vi "Battery_Tester_Main.vi"() -> ()   [LabVIEW 2019]
uses:
  <vilib>/Analysis/baseanly.llb/Mean (DBL).vi
  <vilib>/Analysis/NI_AALBase.lvlib
panel:
  in  "CurrentRefArrayGraph":dbl[](array[numeric])
  in  "Reset Log":bool
  out "Voltage/Current by Time NUI":T1(graph)=[{"TimeGraph"=[0.0, 0.88, 1.924, 3.815, 4.953, 6.09, 7.236, 8.152, 9.288, 10.425, 11.564, 12.704, 13.844, 14.984, 16.032, 17.055, 18.199, 19.341, 20.48, 21.391, 22.528, 23.667, 24.804, 25.944, 27.082, 28.181, 29.167, 30.31, 31.445, 32.587, 33.721, 34.863, 35.997, 37.13, 38.264, 39.403, 40.547, 41.692, 42.838, 43.976, 45.121, 46.267, 47.404, 48.544, 49.684, 50.825, 51.952, 53.087, 54.227, 55.361, 56.502, 57.644, 58.78, 59.928, 61.067, 62.203, 63.348, 64.485, 65.629, 66.772, 67.915, 69.061, 70.022, 71.167, 72.302, 73.444, 74.578, 75.709, 76.845, 77.978, 79.128, 80.272, 81.412, 82.552, 83.693, 84.833, 85.971, 87.106, 88.246, 89.247, 90.387, 91.523, 92.658, 93.8, 94.936, 96.082, 97.22, 98.357, 99.491, 100.625, 101.764, 102.898, 104.035, 105.171, 106.317, 107.453, 108.597, 109.732, 110.872, 112.007, 113.153, 114.287, 115.319, 116.45, 117.588, 118.721, 119.861, 120.999, 122.139, 123.108, 124.248, 125.384, 126.521, 127.655, 128.797, 129.932, 131.067, 132.105, 133.242, 134.386, 135.531, 136.662, 137.795, 138.946, 140.08, 141.219, 142.357, 143.495, 144.633, 145.771, 146.824, 147.806, 148.95, 150.084, 151.22, 152.353, 153.487, 154.625, 155.761, 156.899, 158.045, 159.178, 160.317, 161.481, 162.612, 163.748, 164.881, 166.022, 167.158, 168.295, 169.21, 170.339, 171.473, 172.612, 173.746, 174.884, 176.016, 177.159, 178.11, 179.243, 180.374, 181.505, 182.639, 183.777, 184.914, 186.049, 187.188, 188.326, 189.465, 190.609, 191.74, 201.232, 202.369, 203.395, 204.535, 205.597, 206.735, 207.868, 209.009, 210.148, 211.285, 212.42, 213.563, 214.701, 215.84, 216.981, 218.121, 219.26, 220.402, 221.537, 222.673, 223.812, 224.946, 226.083, 227.221, 228.36, 229.504, 230.637, 231.78, 232.916, 234.051, 235.189, 236.321, 237.457, 238.593, 239.73, 240.871, 242.008, 243.147, 265.521, 266.543, 267.649, 268.599, 269.536], "CurrentArrayGraph"=[844.5, 844.5, 844.0, 837.3, 835.8, 833.5, 835.2, 829.9, 832.5, 828.9, 829.5, 831.6, 832.0, 831.6, 825.7, 830.4, 828.4, 830.0, 825.9, 827.8, 825.2, 825.2, 826.7, 827.8, 827.4, 821.6, 831.1, 822.6, 826.3, 822.9, 824.2, 819.1, 819.5, 824.8, 825.0, 817.7, 821.7, 823.7, 820.6, 820.2, 824.2, 823.3, 820.2, 824.8, 825.4, 821.7, 818.0, 820.0, 822.7, 818.0, 817.1, 822.2, 821.1, 818.6, 816.5, 816.6, 818.1, 818.0, 818.1, 816.6, 816.5, 815.0, 819.0, 814.5, 823.8, 814.0, 816.0, 818.5, 812.5, 821.6, 817.0, 815.6, 818.0, 818.6, 817.6, 815.6, 814.0, 812.0, 813.5, 812.5, 813.0, 812.5, 814.5, 813.0, 815.0, 810.5, 817.0, 815.6, 814.6, 812.0, 816.5, 815.0, 813.0, 816.6, 812.5, 808.5, 812.5, 807.0, 810.5, 814.0, 812.0, 818.5, 810.5, 817.5, 808.0, 820.0, 808.5, 816.0, 813.1, 813.0, 808.0, 814.5, 809.0, 814.0, 806.5, 815.5, 810.0, 806.5, 807.0, 812.5, 811.5, 816.1, 810.5, 813.6, 812.5, 806.0, 809.5, 816.5, 809.0, 806.5, 806.0, 808.5, 804.5, 811.5, 814.5, 816.0, 804.5, 804.5, 803.5, 808.5, 809.0, 804.5, 805.5, 805.5, 804.0, 805.5, 805.0, 803.0, 806.0, 806.5, 810.5, 807.0, 803.5, 803.0, 802.5, 803.0, 802.5, 802.5, 812.0, 811.0, 803.5, 806.1, 809.0, 818.1, 809.5, 804.0, 802.5, 804.5, 803.5, 809.5, 809.5, 81.2, 809.5, 803.5, 812.0, 801.5, 807.5, 804.5, 804.5, 807.0, 805.0, 808.0, 807.0, 802.5, 807.0, 803.5, 803.0, 806.0, 802.5, 805.5, 806.5, 804.0, 806.0, 804.0, 804.5, 807.5, 800.0, 805.0, 807.0, 803.5, 804.0, 802.0, 806.5, 802.0, 804.0, 800.5, 803.0, 803.0, 804.0, 80.2, 723.3, 803.0, 800.5, 798.5]}, {"TimeGraph"=[0.0, 0.88, 1.924, 3.815, 4.953, 6.09, 7.236, 8.152, 9.288, 10.425, 11.564, 12.704, 13.844, 14.984, 16.032, 17.055, 18.199, 19.341, 20.48, 21.391, 22.528, 23.667, 24.804, 25.944, 27.082, 28.181, 29.167, 30.31, 31.445, 32.587, 33.721, 34.863, 35.997, 37.13, 38.264, 39.403, 40.547, 41.692, 42.838, 43.976, 45.121, 46.267, 47.404, 48.544, 49.684, 50.825, 51.952, 53.087, 54.227, 55.361, 56.502, 57.644, 58.78, 59.928, 61.067, 62.203, 63.348, 64.485, 65.629, 66.772, 67.915, 69.061, 70.022, 71.167, 72.302, 73.444, 74.578, 75.709, 76.845, 77.978, 79.128, 80.272, 81.412, 82.552, 83.693, 84.833, 85.971, 87.106, 88.246, 89.247, 90.387, 91.523, 92.658, 93.8, 94.936, 96.082, 97.22, 98.357, 99.491, 100.625, 101.764, 102.898, 104.035, 105.171, 106.317, 107.453, 108.597, 109.732, 110.872, 112.007, 113.153, 114.287, 115.319, 116.45, 117.588, 118.721, 119.861, 120.999, 122.139, 123.108, 124.248, 125.384, 126.521, 127.655, 128.797, 129.932, 131.067, 132.105, 133.242, 134.386, 135.531, 136.662, 137.795, 138.946, 140.08, 141.219, 142.357, 143.495, 144.633, 145.771, 146.824, 147.806, 148.95, 150.084, 151.22, 152.353, 153.487, 154.625, 155.761, 156.899, 158.045, 159.178, 160.317, 161.481, 162.612, 163.748, 164.881, 166.022, 167.158, 168.295, 169.21, 170.339, 171.473, 172.612, 173.746, 174.884, 176.016, 177.159, 178.11, 179.243, 180.374, 181.505, 182.639, 183.777, 184.914, 186.049, 187.188, 188.326, 189.465, 190.609, 191.74, 201.232, 202.369, 203.395, 204.535, 205.597, 206.735, 207.868, 209.009, 210.148, 211.285, 212.42, 213.563, 214.701, 215.84, 216.981, 218.121, 219.26, 220.402, 221.537, 222.673, 223.812, 224.946, 226.083, 227.221, 228.36, 229.504, 230.637, 231.78, 232.916, 234.051, 235.189, 236.321, 237.457, 238.593, 239.73, 240.871, 242.008, 243.147, 265.521, 266.543, 267.649, 268.599, 269.536], "CurrentArrayGraph"=[48.35, 47.1, 48.6, 47.3, 49.35, 49.4, 50.05, 44.95, 51.65, 44.95, 44.7, 50.15, 51.4, 49.9, 49.45, 48.05, 49.1, 49.85, 46.75, 50.1, 50.65, 44.9, 44.7, 43.9, 44.45, 46.25, 45.9, 49.9, 50.1, 46.8, 48.75, 48.6, 49.65, 51.4, 49.6, 43.7, 43.7, 51.15, 49.35, 50.45, 49.9, 50.9, 48.85, 49.05, 51.65, 50.4, 41.35, 50.65, 49.4, 43.9, 50.9, 48.55, 48.85, 47.8, 39.0, 48.9, 47.05, 51.95, 48.8, 51.15, 50.95, 48.6, 46.5, 45.75, 52.6, 43.45, 48.85, 51.6, 50.4, 50.3, 50.45, 44.95, 49.6, 49.8, 50.1, 49.9, 51.25, 44.75, 51.15, 46.0, 45.45, 51.5, 52.0, 48.65, 54.45, 48.85, 46.0, 53.95, 42.1, 51.15, 41.35, 56.1, 46.75, 53.6, 47.3, 50.7, 48.6, 52.75, 35.45, 56.05, 45.25, 54.2, 50.45, 52.65, 48.9, 48.5, 50.4, 48.6, 51.45, 48.85, 45.25, 53.5, 44.0, 52.35, 49.35, 52.95, 56.1, 56.35, 46.8, 52.35, 46.8, 55.0, 56.6, 52.3, 56.9, 46.3, 44.5, 49.75, 50.9, 46.5, 43.75, 45.75, 39.1, 46.75, 47.25, 52.1, 56.35, 49.9, 30.05, 46.0, 55.3, 51.0, 49.8, 39.6, 33.95, 45.5, 40.85, 35.95, 39.1, 39.6, 45.75, 43.25, 30.8, 43.75, 38.6, 43.75, 49.55, 39.85, 45.1, 46.5, 39.1, 49.55, 56.35, 50.25, 45.5, 44.0, 38.6, 39.35, 43.0, 48.5, 43.6, 5.95, 52.2, 48.55, 48.6, 43.5, 52.7, 49.55, 48.05, 49.1, 50.15, 49.6, 52.95, 49.35, 47.85, 50.65, 44.95, 49.1, 47.8, 49.1, 46.2, 48.1, 49.8, 49.65, 49.85, 50.6, 38.8, 46.55, 47.8, 50.05, 51.15, 46.0, 49.1, 48.3, 51.4, 50.2, 33.3, 50.65, 48.1, 5.95, 42.9, 48.3, 40.6, 45.7]}, {"TimeGraph"=[0.0, 0.88, 1.924, 3.815, 4.953, 6.09, 7.236, 8.152, 9.288, 10.425, 11.564, 12.704, 13.844, 14.984, 16.032, 17.055, 18.199, 19.341, 20.48, 21.391, 22.528, 23.667, 24.804, 25.944, 27.082, 28.181, 29.167, 30.31, 31.445, 32.587, 33.721, 34.863, 35.997, 37.13, 38.264, 39.403, 40.547, 41.692, 42.838, 43.976, 45.121, 46.267, 47.404, 48.544, 49.684, 50.825, 51.952, 53.087, 54.227, 55.361, 56.502, 57.644, 58.78, 59.928, 61.067, 62.203, 63.348, 64.485, 65.629, 66.772, 67.915, 69.061, 70.022, 71.167, 72.302, 73.444, 74.578, 75.709, 76.845, 77.978, 79.128, 80.272, 81.412, 82.552, 83.693, 84.833, 85.971, 87.106, 88.246, 89.247, 90.387, 91.523, 92.658, 93.8, 94.936, 96.082, 97.22, 98.357, 99.491, 100.625, 101.764, 102.898, 104.035, 105.171, 106.317, 107.453, 108.597, 109.732, 110.872, 112.007, 113.153, 114.287, 115.319, 116.45, 117.588, 118.721, 119.861, 120.999, 122.139, 123.108, 124.248, 125.384, 126.521, 127.655, 128.797, 129.932, 131.067, 132.105, 133.242, 134.386, 135.531, 136.662, 137.795, 138.946, 140.08, 141.219, 142.357, 143.495, 144.633, 145.771, 146.824, 147.806, 148.95, 150.084, 151.22, 152.353, 153.487, 154.625, 155.761, 156.899, 158.045, 159.178, 160.317, 161.481, 162.612, 163.748, 164.881, 166.022, 167.158, 168.295, 169.21, 170.339, 171.473, 172.612, 173.746, 174.884, 176.016, 177.159, 178.11, 179.243, 180.374, 181.505, 182.639, 183.777, 184.914, 186.049, 187.188, 188.326, 189.465, 190.609, 191.74, 201.232, 202.369, 203.395, 204.535, 205.597, 206.735, 207.868, 209.009, 210.148, 211.285, 212.42, 213.563, 214.701, 215.84, 216.981, 218.121, 219.26, 220.402, 221.537, 222.673, 223.812, 224.946, 226.083, 227.221, 228.36, 229.504, 230.637, 231.78, 232.916, 234.051, 235.189, 236.321, 237.457, 238.593, 239.73, 240.871, 242.008, 243.147, 265.521, 266.543, 267.649, 268.599, 269.536], "CurrentArrayGraph"=[50.0, 50.0, 50.0, 50.0, 50.0, 50.0, 50.0, 50.0, 50.0, 50.0, 50.0, 50.0, 50.0, 50.0, 50.0, 50.0, 50.0, 50.0, 50.0, 50.0, 50.0, 50.0, 50.0, 50.0, 50.0, 50.0, 50.0, 50.0, 50.0, 50.0, 50.0, 50.0, 50.0, 50.0, 50.0, 50.0, 50.0, 50.0, 50.0, 50.0, 50.0, 50.0, 50.0, 50.0, 50.0, 50.0, 50.0, 50.0, 50.0, 50.0, 50.0, 50.0, 50.0, 50.0, 50.0, 50.0, 50.0, 50.0, 50.0, 50.0, 50.0, 50.0, 50.0, 50.0, 50.0, 50.0, 50.0, 50.0, 50.0, 50.0, 50.0, 50.0, 50.0, 50.0, 50.0, 50.0, 50.0, 50.0, 50.0, 50.0, 50.0, 50.0, 50.0, 50.0, 50.0, 50.0, 50.0, 50.0, 50.0, 50.0, 50.0, 50.0, 50.0, 50.0, 50.0, 50.0, 50.0, 50.0, 50.0, 50.0, 50.0, 50.0, 50.0, 50.0, 50.0, 50.0, 50.0, 50.0, 50.0, 50.0, 50.0, 50.0, 50.0, 50.0, 50.0, 50.0, 50.0, 50.0, 50.0, 50.0, 50.0, 50.0, 50.0, 50.0, 50.0, 50.0, 50.0, 50.0, 50.0, 50.0, 50.0, 50.0, 50.0, 50.0, 50.0, 50.0, 50.0, 50.0, 50.0, 50.0, 50.0, 50.0, 50.0, 50.0, 50.0, 50.0, 50.0, 50.0, 50.0, 50.0, 50.0, 50.0, 50.0, 50.0, 50.0, 50.0, 50.0, 50.0, 50.0, 50.0, 50.0, 50.0, 50.0, 50.0, 50.0, 50.0, 50.0, 50.0, 50.0, 50.0, 50.0, 50.0, 50.0, 50.0, 50.0, 50.0, 50.0, 50.0, 50.0, 50.0, 50.0, 50.0, 50.0, 50.0, 50.0, 50.0, 50.0, 50.0, 50.0, 50.0, 50.0, 50.0, 50.0, 50.0, 50.0, 50.0, 50.0, 50.0, 50.0, 50.0, 50.0, 50.0, 50.0, 50.0, 50.0, 50.0, 50.0, 50.0, 50.0, 50.0, 50.0, 50.0, 50.0, 50.0, 0.0]}]
  out "Watt by Time NUI":cluster{"TimeGraph":dbl[], dbl[]}(graph)
  out "Watt by Time":cluster{"TimeGraph":dbl[], dbl[]}(graph)
  out "Voltage/Current by Time":T1(graph)
  in  "RTB Enable":bool
  in  "TimeGraph":dbl[](array[numeric])
  in  "CurrentArrayGraph":dbl[](array[numeric])
  in  "VoltageArrayGraph":dbl[](array[numeric])
  in  "Update XY":bool
  out "CL Status":bool
  out "VL Status":bool
  in  "CL Active":bool
  in  "VL Active":bool
  in  "Current Limit":dbl
  in  "Voltage Limit":dbl
  in  "LogIndex":i32
  in  "RTB":string="26\t312457915\t1404,000000\t498,000000\t500,000000\r\n27\t312459060\t1399,500000\t498,500000\t500,000000\r\n28\t312460197\t1398,500000\t498,000000\t500,000000\r\n29\t312461332\t1400,500000\t497,250000\t500,000000\r\n30\t312462472\t1397,000000\t498,250000\t500,000000\r\n31\t312463608\t1399,000000\t498,250000\t500,000000\r\n32\t312464755\t1395,900000\t498,250000\t500,000000\r\n33\t312465899\t1394,700000\t498,250000\t500,000000\r\n34\t312467032\t1393,300000\t498,750000\t500,000000\r\n35\t312468162\t1395,800000\t497,750000\t500,000000\r\n36\t312469297\t1390,400000\t497,500000\t500,000000\r\n37\t312470436\t1393,100000\t498,750000\t500,000000\r\n38\t312471582\t1390,400000\t498,000000\t500,000000\r\n39\t312472717\t1389,300000\t498,750000\t500,000000\r\n40\t312473855\t1385,500000\t499,250000\t500,000000\r\n41\t312474986\t1386,100000\t498,000000\t500,000000\r\n42\t312476128\t1384,700000\t498,250000\t500,000000\r\n43\t312477264\t1384,000000\t498,250000\t500,000000\r\n44\t312478402\t1384,700000\t498,750000\t500,000000\r\n45\t312479539\t1381,500000\t497,250000\t500,000000\r\n46\t312480679\t1381,500000\t498,750000\t500,000000\r\n47\t312481826\t1381,600000\t498,750000\t500,000000\r\n48\t312482971\t1381,500000\t498,750000\t500,000000\r\n49\t312484111\t1378,500000\t497,750000\t500,000000\r\n50\t312485249\t1377,000000\t498,000000\t500,000000\r\n51\t312486384\t1379,000000\t498,750000\t500,000000\r\n52\t312487529\t1379,100000\t497,250000\t500,000000\r\n53\t312488669\t1375,000000\t498,500000\t500,000000\r\n54\t312489813\t1376,000000\t498,250000\t500,000000\r\n55\t312490955\t1375,500000\t498,250000\t500,000000\r\n56\t312492089\t1375,500000\t498,500000\t500,000000\r\n57\t312493222\t1375,500000\t497,750000\t500,000000\r\n58\t312494349\t1375,000000\t497,750000\t500,000000\r\n59\t312495483\t1373,000000\t498,500000\t500,000000\r\n60\t312496615\t1373,500000\t498,000000\t500,000000\r\n61\t312497754\t1373,000000\t497,750000\t500,000000\r\n62\t312498899\t1372,500000\t498,000000\t500,000000\r\n63\t312500040\t1374,500000\t498,500000\t500,000000\r\n64\t312501176\t1373,500000\t497,250000\t500,000000\r\n65\t312502315\t1374,000000\t496,950000\t500,000000\r\n66\t312503457\t1371,500000\t497,250000\t500,000000\r\n67\t312504594\t1370,500000\t498,250000\t500,000000\r\n68\t312505732\t1370,500000\t498,250000\t500,000000\r\n69\t312506866\t1371,000000\t497,250000\t500,000000\r\n70\t312508008\t1369,500000\t498,250000\t500,000000\r\n71\t312509151\t1369,500000\t498,250000\t500,000000\r\n72\t312510284\t1367,500000\t498,500000\t500,000000\r\n73\t312511422\t1366,500000\t498,000000\t500,000000\r\n74\t312512564\t1370,500000\t497,500000\t500,000000\r\n75\t312513704\t1368,000000\t499,000000\t500,000000\r\n76\t312514846\t1366,000000\t499,000000\t500,000000\r\n77\t312515981\t1365,500000\t497,750000\t500,000000\r\n78\t312517116\t1365,000000\t498,250000\t500,000000\r\n79\t312518260\t1364,500000\t498,500000\t500,000000\r\n80\t312519401\t1364,500000\t498,200000\t500,000000\r\n81\t312520533\t1364,000000\t497,750000\t500,000000\r\n82\t312521670\t1363,000000\t498,250000\t500,000000\r\n83\t312522809\t1364,000000\t498,750000\t500,000000\r\n84\t312523943\t1362,500000\t499,500000\t500,000000\r\n85\t312525082\t1360,000000\t498,000000\t500,000000\r\n86\t312526212\t1358,500000\t498,750000\t500,000000\r\n87\t312527353\t1362,000000\t497,750000\t500,000000\r\n88\t312528493\t1359,000000\t498,250000\t500,000000\r\n89\t312529631\t1358,500000\t497,500000\t500,000000\r\n90\t312530777\t1359,500000\t498,250000\t500,000000\r\n91\t312531911\t1358,000000\t498,250000\t500,000000\r\n92\t312533047\t1358,000000\t498,250000\t500,000000\r\n93\t312534189\t1358,000000\t498,250000\t500,000000\r\n94\t312535334\t1358,000000\t498,000000\t500,000000\r\n95\t312536465\t1355,000000\t498,750000\t500,000000\r\n96\t312537599\t1356,000000\t498,500000\t500,000000\r\n97\t312538738\t1355,000000\t498,250000\t500,000000\r\n98\t312539872\t1355,000000\t498,750000\t500,000000\r\n99\t312541018\t1355,000000\t497,500000\t500,000000\r\n100\t312542160\t1354,000000\t498,250000\t500,000000\r\n101\t312543297\t1354,000000\t497,750000\t500,000000\r\n102\t312544442\t1353,000000\t497,000000\t500,000000\r\n103\t312545578\t1357,000000\t498,500000\t500,000000\r\n104\t312546718\t1353,000000\t498,000000\t500,000000\r\n105\t312547854\t1355,000000\t498,250000\t500,000000\r\n106\t312548993\t1352,500000\t498,250000\t500,000000\r\n107\t312550133\t1354,000000\t497,750000\t500,000000\r\n108\t312551272\t1353,000000\t499,250000\t500,000000\r\n109\t312552415\t1353,000000\t497,750000\t500,000000\r\n110\t312553556\t1351,000000\t498,250000\t500,000000\r\n111\t312554694\t1351,000000\t498,500000\t500,000000\r\n112\t312555836\t1352,000000\t498,250000\t500,000000\r\n113\t312556984\t1352,000000\t499,000000\t500,000000\r\n114\t312558116\t1350,000000\t499,250000\t500,000000\r\n115\t312559256\t1350,000000\t497,500000\t500,000000\r\n116\t312560395\t1348,900000\t498,750000\t500,000000\r\n117\t312561536\t1349,500000\t499,000000\t500,000000\r\n118\t312562677\t1350,500000\t497,750000\t500,000000\r\n119\t312563815\t1348,000000\t498,250000\t500,000000\r\n120\t312564953\t1350,000000\t498,500000\t500,000000\r\n121\t312566091\t1348,500000\t498,500000\t500,000000\r\n122\t312567233\t1346,900000\t498,000000\t500,000000\r\n123\t312568373\t1347,500000\t498,500000\t500,000000\r\n124\t312569512\t1346,500000\t498,750000\t500,000000\r\n125\t312570653\t1344,900000\t498,000000\t500,000000\r\n126\t312571794\t1344,500000\t498,000000\t500,000000\r\n127\t312572934\t1345,500000\t498,000000\t500,000000\r\n128\t312574072\t1347,000000\t498,750000\t500,000000\r\n129\t312575212\t1345,400000\t498,250000\t500,000000\r\n130\t312576346\t1343,200000\t498,750000\t500,000000\r\n131\t312577489\t1343,300000\t498,250000\t500,000000\r\n132\t312578627\t1344,400000\t498,250000\t500,000000\r\n133\t312579768\t1344,500000\t498,750000\t500,000000\r\n134\t312580911\t1341,700000\t497,750000\t500,000000\r\n135\t312582052\t1338,900000\t498,250000\t500,000000\r\n136\t312583191\t1342,700000\t498,750000\t500,000000\r\n137\t312584327\t1341,000000\t498,750000\t500,000000\r\n138\t312585467\t1342,100000\t498,000000\t500,000000\r\n139\t312586607\t1341,300000\t496,700000\t500,000000\r\n140\t312587748\t1341,100000\t498,750000\t500,000000\r\n141\t312588888\t1338,800000\t498,000000\t500,000000\r\n142\t312590024\t1339,400000\t498,750000\t500,000000\r\n143\t312591168\t1344,300000\t498,000000\t500,000000\r\n144\t312592300\t1337,700000\t498,500000\t500,000000\r\n145\t312593437\t1340,500000\t498,000000\t500,000000\r\n146\t312594574\t1338,700000\t498,000000\t500,000000\r\n147\t312595543\t1338,300000\t498,500000\t500,000000\r\n148\t312596684\t1337,300000\t497,750000\t500,000000\r\n149\t312597814\t1337,800000\t498,750000\t500,000000\r\n150\t312598947\t1338,900000\t498,500000\t500,000000\r\n151\t312600084\t1336,200000\t497,500000\t500,000000\r\n152\t312601230\t1337,200000\t497,500000\t500,000000\r\n153\t312602361\t1337,200000\t498,750000\t500,000000\r\n154\t312603499\t1337,300000\t498,000000\t500,000000\r\n155\t312604636\t1334,600000\t498,500000\t500,000000\r\n156\t312605771\t1336,300000\t497,200000\t500,000000\r\n157\t312606906\t1334,100000\t497,750000\t500,000000\r\n158\t312608051\t1333,500000\t497,500000\t500,000000\r\n159\t312609190\t1336,700000\t498,250000\t500,000000\r\n160\t312610331\t1334,600000\t498,750000\t500,000000\r\n161\t312611466\t1336,300000\t497,750000\t500,000000\r\n162\t312612612\t1336,100000\t498,750000\t500,000000\r\n163\t312613744\t1337,200000\t498,000000\t500,000000\r\n164\t312614881\t1333,500000\t498,500000\t500,000000\r\n165\t312616021\t1335,700000\t497,750000\t500,000000\r\n166\t312617153\t1333,000000\t498,250000\t500,000000\r\n167\t312618290\t1332,000000\t498,500000\t500,000000\r\n168\t312619431\t1332,000000\t498,000000\t500,000000\r\n169\t312620571\t1333,600000\t498,250000\t500,000000\r\n170\t312621708\t1335,600000\t498,500000\t500,000000\r\n171\t312622844\t1333,000000\t498,000000\t500,000000\r\n172\t312623981\t1333,500000\t498,750000\t500,000000\r\n173\t312625119\t1331,000000\t498,500000\t500,000000\r\n174\t312626257\t1333,100000\t498,250000\t500,000000\r\n175\t312627391\t1331,000000\t498,500000\t500,000000\r\n176\t312628523\t1330,000000\t497,750000\t500,000000\r\n177\t312629658\t1330,500000\t498,250000\t500,000000\r\n178\t312630789\t1330,000000\t498,500000\t500,000000\r\n179\t312631849\t1327,000000\t498,200000\t500,000000\r\n180\t312632984\t1332,100000\t498,000000\t500,000000\r\n181\t312634121\t1333,200000\t498,250000\t500,000000\r\n182\t312635257\t1332,600000\t499,000000\t500,000000\r\n183\t312636390\t1332,600000\t497,750000\t500,000000\r\n184\t312637535\t1330,500000\t499,000000\t500,000000\r\n185\t312638669\t1329,000000\t498,250000\t500,000000\r\n186\t312639804\t1329,100000\t498,500000\t500,000000\r\n187\t312640943\t1327,500000\t497,250000\t500,000000\r\n188\t312642081\t1331,500000\t499,250000\t500,000000\r\n189\t312643218\t1328,000000\t498,750000\t500,000000\r\n190\t312644355\t1327,000000\t498,750000\t500,000000\r\n191\t312645501\t1328,000000\t499,000000\t500,000000\r\n192\t312646651\t1325,500000\t498,500000\t500,000000\r\n193\t312647792\t1326,000000\t498,000000\t500,000000\r\n194\t312648930\t1327,000000\t498,250000\t500,000000\r\n195\t312650061\t1327,000000\t498,250000\t500,000000\r\n196\t312651205\t1326,000000\t498,250000\t500,000000\r\n197\t312652352\t1325,500000\t498,500000\t500,000000\r\n198\t312653490\t1324,000000\t498,250000\t500,000000\r\n199\t312654626\t1325,000000\t499,000000\t500,000000\r\n200\t312655764\t1325,500000\t498,250000\t500,000000\r\n201\t312656897\t1324,500000\t499,250000\t500,000000\r\n202\t312658036\t1326,000000\t499,750000\t500,000000\r\n203\t312659174\t1326,000000\t497,750000\t500,000000\r\n204\t312660311\t1326,500000\t498,750000\t500,000000\r\n205\t312661453\t1323,500000\t498,000000\t500,000000\r\n206\t312662597\t1323,500000\t497,750000\t500,000000\r\n207\t312663734\t1321,500000\t498,250000\t500,000000\r\n208\t312664877\t1321,000000\t497,750000\t500,000000\r\n209\t312666022\t1324,500000\t498,750000\t500,000000\r\n210\t312667162\t1324,500000\t497,750000\t500,000000\r\n211\t312668302\t1321,500000\t497,500000\t500,000000\r\n212\t312669438\t1321,000000\t498,250000\t500,000000\r\n213\t312670572\t1322,000000\t498,750000\t500,000000\r\n214\t312671709\t1322,500000\t498,000000\t500,000000\r\n215\t312672844\t1320,500000\t497,500000\t500,000000\r\n216\t312673981\t1322,500000\t497,250000\t500,000000\r\n217\t312675118\t1320,500000\t498,500000\t500,000000\r\n218\t312676261\t1321,000000\t498,750000\t500,000000\r\n219\t312677399\t1319,500000\t498,500000\t500,000000\r\n220\t312678534\t1321,500000\t498,250000\t500,000000\r\n221\t312679673\t1322,000000\t497,750000\t500,000000\r\n222\t312680810\t1320,500000\t498,250000\t500,000000\r\n223\t312681944\t1320,000000\t498,750000\t500,000000\r\n224\t312683083\t1318,000000\t498,250000\t500,000000\r\n225\t312684230\t1323,000000\t499,000000\t500,000000\r\n226\t312685373\t1317,500000\t498,750000\t500,000000\r\n227\t312686510\t1319,500000\t499,000000\t500,000000\r\n228\t312687654\t1319,500000\t498,250000\t500,000000\r\n229\t312688795\t1317,000000\t498,750000\t500,000000\r\n230\t312689930\t1317,500000\t498,750000\t500,000000\r\n231\t312691072\t1317,000000\t498,000000\t500,000000\r\n232\t312692219\t1318,500000\t497,500000\t500,000000\r\n233\t312693356\t1317,500000\t498,500000\t500,000000\r\n234\t312694500\t1318,000000\t498,250000\t500,000000\r\n235\t312695636\t1316,000000\t498,750000\t500,000000\r\n236\t312696768\t1318,000000\t498,500000\t500,000000\r\n237\t312697913\t1317,500000\t498,750000\t500,000000\r\n238\t312699048\t1318,000000\t498,500000\t500,000000\r\n239\t312700187\t1317,000000\t498,000000\t500,000000\r\n240\t312701322\t1315,000000\t499,750000\t500,000000\r\n241\t312702469\t1319,000000\t498,750000\t500,000000\r\n242\t312703615\t1317,000000\t498,250000\t500,000000\r\n243\t312704748\t1314,500000\t498,750000\t500,000000\r\n244\t312705885\t1313,500000\t497,750000\t500,000000\r\n245\t312707020\t1314,000000\t498,750000\t500,000000\r\n246\t312708160\t1314,500000\t498,250000\t500,000000\r\n247\t312709304\t1313,500000\t498,500000\t500,000000\r\n248\t312710447\t1313,500000\t498,250000\t500,000000\r\n249\t312711592\t1313,000000\t499,000000\t500,000000\r\n250\t312712747\t1314,000000\t498,000000\t500,000000\r\n251\t312713889\t1312,000000\t498,250000\t500,000000\r\n252\t312715021\t1311,000000\t497,500000\t500,000000\r\n253\t312716159\t1311,500000\t499,250000\t500,000000\r\n254\t312717297\t1314,000000\t498,750000\t500,000000\r\n255\t312718434\t1310,500000\t498,500000\t500,000000\r\n256\t312719566\t1311,500000\t498,750000\t500,000000\r\n257\t312720703\t1313,500000\t499,000000\t500,000000\r\n258\t312721832\t1313,500000\t499,250000\t500,000000\r\n259\t312722971\t1310,000000\t497,750000\t500,000000\r\n260\t312724113\t1312,500000\t498,250000\t500,000000\r\n261\t312725252\t1312,000000\t499,000000\t500,000000\r\n262\t312726386\t1311,500000\t498,500000\t500,000000\r\n263\t312727524\t1309,500000\t499,000000\t500,000000\r\n264\t312728662\t1312,000000\t497,750000\t500,000000\r\n265\t312729798\t1310,500000\t498,750000\t500,000000\r\n266\t312730940\t1312,500000\t498,250000\t500,000000\r\n267\t312732076\t1310,500000\t499,000000\t500,000000\r\n268\t312733211\t1311,500000\t497,750000\t500,000000\r\n269\t312734350\t1311,000000\t497,750000\t500,000000\r\n270\t312735485\t1310,500000\t498,750000\t500,000000\r\n271\t312736619\t1310,000000\t498,500000\t500,000000\r\n272\t312737754\t1308,500000\t498,000000\t500,000000\r\n273\t312738886\t1310,000000\t498,750000\t500,000000\r\n274\t312740021\t1310,500000\t498,250000\t500,000000\r\n275\t312741150\t1308,500000\t498,750000\t500,000000\r\n276\t312742547\t1306,500000\t498,000000\t500,000000\r\n277\t312744254\t1310,500000\t499,000000\t500,000000\r\n278\t312745956\t1310,500000\t497,750000\t500,000000\r\n279\t312747655\t1307,500000\t498,750000\t500,000000\r\n280\t312749356\t1307,500000\t498,250000\t500,000000\r\n281\t312751064\t1307,000000\t498,000000\t500,000000\r\n282\t312752776\t1306,000000\t499,000000\t500,000000\r\n283\t312754482\t1306,500000\t498,250000\t500,000000\r\n284\t312756185\t1306,500000\t497,750000\t500,000000\r\n285\t312757873\t1304,000000\t498,500000\t500,000000\r\n286\t312759574\t1303,500000\t497,500000\t500,000000\r\n287\t312761274\t1306,000000\t499,500000\t500,000000\r\n288\t312762978\t1303,000000\t498,250000\t500,000000\r\n289\t312764676\t1305,000000\t498,250000\t500,000000\r\n290\t312766380\t1303,500000\t498,250000\t500,000000\r\n291\t312768080\t1303,500000\t498,000000\t500,000000\r\n292\t312769773\t1300,500000\t497,750000\t500,000000\r\n293\t312771468\t1302,500000\t498,000000\t500,000000\r\n294\t312773170\t1301,500000\t498,000000\t500,000000\r\n295\t312774864\t1302,000000\t499,250000\t500,000000\r\n296\t312776568\t1301,500000\t498,000000\t500,000000\r\n297\t312778269\t1303,500000\t497,750000\t500,000000\r\n298\t312779966\t1301,000000\t497,250000\t500,000000\r\n299\t312781670\t1302,500000\t497,750000\t500,000000\r\n300\t312783364\t1301,000000\t498,000000\t500,000000\r\n301\t312785065\t1301,500000\t498,500000\t500,000000\r\n302\t312786760\t1301,500000\t499,000000\t500,000000\r\n303\t312788466\t1302,000000\t498,000000\t500,000000\r\n304\t312790164\t1300,000000\t498,750000\t500,000000\r\n305\t312791875\t1299,000000\t498,250000\t500,000000\r\n306\t312793587\t1298,000000\t498,500000\t500,000000\r\n307\t312795294\t1297,500000\t497,750000\t500,000000\r\n308\t312796989\t1298,000000\t498,750000\t500,000000\r\n309\t312798692\t1297,500000\t498,000000\t500,000000\r\n310\t312800399\t1299,500000\t498,250000\t500,000000\r\n311\t312802104\t1297,000000\t498,250000\t500,000000\r\n312\t312803809\t1298,000000\t498,750000\t500,000000\r\n313\t312805513\t1298,500000\t498,250000\t500,000000\r\n314\t312807215\t1297,000000\t498,000000\t500,000000\r\n315\t312808926\t1297,500000\t499,000000\t500,000000\r\n316\t312810628\t1297,000000\t497,500000\t500,000000\r\n317\t312812325\t1295,400000\t499,000000\t500,000000\r\n318\t312814026\t1295,500000\t498,250000\t500,000000\r\n319\t312815735\t1297,000000\t497,500000\t500,000000\r\n320\t312817433\t1295,500000\t499,000000\t500,000000\r\n321\t312819131\t1294,000000\t498,250000\t500,000000\r\n322\t312820831\t1292,900000\t499,000000\t500,000000\r\n323\t312822526\t1296,000000\t499,000000\t500,000000\r\n324\t312824223\t1294,500000\t498,250000\t500,000000\r\n325\t312825923\t1292,400000\t497,950000\t500,000000\r\n326\t312827610\t1292,400000\t497,750000\t500,000000\r\n327\t312829306\t1293,400000\t498,750000\t500,000000\r\n328\t312831006\t1292,500000\t498,000000\t500,000000\r\n329\t312832697\t1292,900000\t498,750000\t500,000000\r\n330\t312834397\t1294,400000\t498,250000\t500,000000\r\n331\t312836100\t1296,500000\t498,750000\t500,000000\r\n332\t312837789\t1291,800000\t498,500000\t500,000000\r\n333\t312839475\t1291,900000\t498,500000\t500,000000\r\n334\t312841175\t1291,800000\t498,750000\t500,000000\r\n335\t312842866\t1293,900000\t497,750000\t500,000000\r\n336\t312844563\t1291,700000\t497,750000\t500,000000\r\n337\t312846256\t1291,700000\t497,750000\t500,000000\r\n338\t312847944\t1292,200000\t499,000000\t500,000000\r\n339\t312849643\t1291,800000\t499,000000\t500,000000\r\n340\t312851337\t1290,500000\t498,750000\t500,000000\r\n341\t312853051\t1290,600000\t499,000000\t500,000000\r\n342\t312854746\t1289,000000\t498,500000\t500,000000\r\n343\t312856164\t1291,300000\t498,500000\t500,000000\r\n344\t312857846\t1291,100000\t498,500000\t500,000000\r\n345\t312859191\t1289,500000\t498,250000\t500,000000\r\n346\t312860323\t1290,000000\t498,750000\t500,000000\r\n347\t312861455\t1290,500000\t497,750000\t500,000000\r\n348\t312862592\t1290,100000\t498,250000\t500,000000\r\n349\t312863726\t1288,600000\t497,000000\t500,000000\r\n350\t312864864\t1287,900000\t498,500000\t500,000000\r\n351\t312865999\t1288,400000\t498,000000\t500,000000\r\n352\t312867141\t1286,800000\t498,250000\t500,000000\r\n353\t312868279\t1287,200000\t496,700000\t500,000000\r\n354\t312869415\t1289,500000\t499,000000\t500,000000\r\n355\t312870549\t1286,200000\t498,500000\t500,000000\r\n356\t312871686\t1286,800000\t498,000000\t500,000000\r\n357\t312872819\t1288,500000\t499,500000\t500,000000\r\n358\t312873953\t1287,800000\t498,500000\t500,000000\r\n359\t312875089\t1286,800000\t498,250000\t500,000000\r\n360\t312876228\t1287,900000\t499,000000\t500,000000\r\n361\t312877364\t1285,800000\t498,500000\t500,000000\r\n362\t312878506\t1286,700000\t498,250000\t500,000000\r\n363\t312879648\t1286,800000\t498,250000\t500,000000\r\n364\t312880785\t1287,300000\t498,000000\t500,000000\r\n365\t312881927\t1284,700000\t498,500000\t500,000000\r\n366\t312883066\t1285,800000\t498,000000\t500,000000\r\n367\t312884202\t1284,600000\t497,250000\t500,000000\r\n368\t312885341\t1285,300000\t499,000000\t500,000000\r\n369\t312886481\t1284,700000\t498,750000\t500,000000\r\n370\t312887614\t1284,700000\t498,500000\t500,000000\r\n371\t312888748\t1284,100000\t497,500000\t500,000000\r\n372\t312889888\t1284,100000\t498,000000\t500,000000\r\n373\t312891023\t1283,600000\t497,500000\t500,000000\r\n374\t312892166\t1284,700000\t498,000000\t500,000000\r\n375\t312893302\t1285,200000\t498,500000\t500,000000\r\n376\t312894441\t1283,600000\t498,000000\t500,000000\r\n377\t312895573\t1282,100000\t496,200000\t500,000000\r\n378\t312896713\t1282,000000\t498,250000\t500,000000\r\n379\t312897851\t1281,500000\t498,500000\t500,000000\r\n380\t312898995\t1284,800000\t498,250000\t500,000000\r\n381\t312900134\t1284,100000\t498,000000\t500,000000\r\n382\t312901274\t1283,100000\t497,500000\t500,000000\r\n383\t312902407\t1282,100000\t498,000000\t500,000000\r\n384\t312903547\t1282,100000\t499,000000\t500,000000\r\n385\t312904686\t1280,600000\t498,750000\t500,000000\r\n386\t312905824\t1283,800000\t498,750000\t500,000000\r\n387\t312906959\t1281,000000\t499,500000\t500,000000\r\n388\t312908103\t1279,000000\t498,250000\t500,000000\r\n389\t312909236\t1282,700000\t498,250000\t500,000000\r\n390\t312910369\t1283,100000\t497,750000\t500,000000\r\n391\t312911501\t1281,700000\t498,250000\t500,000000\r\n392\t312912639\t1280,000000\t499,250000\t500,000000\r\n393\t312913776\t1281,000000\t499,000000\t500,000000\r\n394\t312914917\t1279,000000\t498,500000\t500,000000\r\n395\t312916057\t1280,500000\t498,750000\t500,000000\r\n396\t312917199\t1282,100000\t497,750000\t500,000000\r\n397\t312918337\t1270,500000\t497,250000\t500,000000\r\n398\t312919479\t1279,500000\t498,250000\t500,000000\r\n399\t312920614\t1277,500000\t497,750000\t500,000000\r\n400\t312921745\t1280,700000\t496,750000\t500,000000\r\n401\t312922887\t1282,100000\t498,250000\t500,000000\r\n402\t312924018\t1279,000000\t498,500000\t500,000000\r\n403\t312925165\t1278,000000\t498,000000\t500,000000\r\n404\t312926308\t1277,000000\t498,500000\t500,000000\r\n405\t312927443\t1277,500000\t497,750000\t500,000000\r\n406\t312928582\t1280,000000\t498,250000\t500,000000\r\n407\t312929719\t1277,000000\t498,500000\t500,000000\r\n408\t312930848\t1278,100000\t498,000000\t500,000000\r\n409\t312931983\t1280,600000\t498,250000\t500,000000\r\n410\t312933117\t1278,500000\t497,750000\t500,000000\r\n411\t312934260\t1278,100000\t498,000000\t500,000000\r\n412\t312935395\t1277,500000\t498,750000\t500,000000\r\n413\t312936528\t1278,500000\t498,000000\t500,000000\r\n414\t312937661\t1276,500000\t498,000000\t500,000000\r\n415\t312938798\t1276,500000\t498,000000\t500,000000\r\n416\t312939937\t1276,500000\t498,000000\t500,000000\r\n417\t312941076\t1278,000000\t498,500000\t500,000000\r\n418\t312942209\t1276,500000\t499,000000\t500,000000\r\n419\t312943348\t1276,100000\t498,750000\t500,000000\r\n420\t312944491\t1276,500000\t498,000000\t500,000000\r\n421\t312945629\t1276,000000\t497,500000\t500,000000\r\n422\t312946770\t1275,500000\t498,000000\t500,000000\r\n423\t312947832\t1276,000000\t498,250000\t500,000000\r\n424\t312948976\t1276,500000\t498,250000\t500,000000\r\n425\t312950113\t1275,500000\t498,500000\t500,000000\r\n426\t312951132\t1276,500000\t499,000000\t500,000000\r\n427\t312952267\t1274,500000\t497,750000\t500,000000\r\n428\t312953406\t1276,100000\t497,200000\t500,000000\r\n429\t312954544\t1274,500000\t497,750000\t500,000000\r\n430\t312955686\t1275,500000\t498,000000\t500,000000\r\n431\t312956825\t1276,100000\t498,250000\t500,000000\r\n432\t312957963\t1272,500000\t498,000000\t500,000000\r\n433\t312959105\t1274,500000\t498,000000\t500,000000\r\n434\t312960243\t1273,000000\t498,500000\t500,000000\r\n435\t312961388\t1273,000000\t498,000000\t500,000000\r\n436\t312962527\t1273,500000\t498,250000\t500,000000\r\n437\t312963662\t1272,500000\t499,000000\t500,000000\r\n438\t312964799\t1273,500000\t498,250000\t500,000000\r\n439\t312965937\t1277,500000\t498,250000\t500,000000\r\n440\t312967069\t1271,000000\t499,000000\t500,000000\r\n441\t312968209\t1272,000000\t498,500000\t500,000000\r\n442\t312969340\t1273,500000\t498,750000\t500,000000\r\n443\t312970479\t1273,000000\t497,750000\t500,000000\r\n444\t312971640\t1273,500000\t498,000000\t500,000000\r\n445\t312972780\t1273,000000\t498,500000\t500,000000\r\n446\t312973913\t1272,000000\t498,000000\t500,000000\r\n447\t312975052\t1271,000000\t498,750000\t500,000000\r\n448\t312976190\t1273,500000\t498,000000\t500,000000\r\n449\t312977331\t1272,500000\t498,250000\t500,000000\r\n450\t312978471\t1272,000000\t498,250000\t500,000000\r\n451\t312979613\t1272,500000\t497,750000\t500,000000\r\n452\t312980754\t1271,500000\t497,500000\t500,000000\r\n453\t312981889\t1270,500000\t498,000000\t500,000000\r\n454\t312983027\t1272,500000\t496,950000\t500,000000\r\n455\t312984168\t1269,500000\t499,000000\t500,000000\r\n456\t312985306\t1272,500000\t498,000000\t500,000000\r\n457\t312986448\t1270,500000\t499,000000\t500,000000\r\n458\t312987591\t1271,500000\t498,750000\t500,000000\r\n459\t312988725\t1271,500000\t498,000000\t500,000000\r\n460\t312989861\t1270,000000\t498,250000\t500,000000\r\n461\t312990994\t1270,000000\t497,750000\t500,000000\r\n462\t312992127\t1270,500000\t498,000000\t500,000000\r\n463\t312993257\t1269,500000\t498,500000\t500,000000\r\n464\t312994392\t1269,500000\t498,000000\t500,000000\r\n465\t312995525\t1272,500000\t496,950000\t500,000000\r\n466\t312996659\t1269,000000\t499,000000\t500,000000\r\n467\t312997793\t1268,500000\t498,500000\t500,000000\r\n468\t312998801\t1269,000000\t498,500000\t500,000000\r\n469\t312999935\t1269,000000\t497,750000\t500,000000\r\n470\t313001073\t1270,500000\t498,250000\t500,000000\r\n471\t313002205\t1270,000000\t498,750000\t500,000000\r\n472\t313003352\t1268,000000\t498,750000\t500,000000\r\n473\t313004487\t1265,000000\t498,250000\t500,000000\r\n474\t313005625\t1270,500000\t498,500000\t500,000000\r\n475\t313006757\t1269,500000\t497,750000\t500,000000\r\n476\t313007897\t1267,500000\t498,750000\t500,000000\r\n477\t313009037\t1268,500000\t499,000000\t500,000000\r\n478\t313010172\t1267,000000\t499,250000\t500,000000\r\n479\t313011308\t1269,000000\t498,750000\t500,000000\r\n480\t313012439\t1269,000000\t497,500000\t500,000000\r\n481\t313013578\t1268,000000\t498,250000\t500,000000\r\n482\t313014713\t1267,000000\t498,750000\t500,000000\r\n483\t313015852\t1266,000000\t498,250000\t500,000000\r\n484\t313016990\t1267,500000\t498,500000\t500,000000\r\n485\t313018137\t1267,500000\t498,500000\t500,000000\r\n486\t313019275\t1269,500000\t498,250000\t500,000000\r\n487\t313020409\t1267,000000\t497,750000\t500,000000\r\n488\t313021545\t1267,000000\t498,500000\t500,000000\r\n489\t313022680\t1267,000000\t498,250000\t500,000000\r\n490\t313023814\t1265,500000\t497,500000\t500,000000\r\n491\t313024943\t1266,500000\t497,250000\t500,000000\r\n492\t313026086\t1267,500000\t498,500000\t500,000000\r\n493\t313027217\t1265,000000\t498,250000\t500,000000\r\n494\t313028356\t1266,000000\t498,750000\t500,000000\r\n495\t313029491\t1267,000000\t498,500000\t500,000000\r\n496\t313030623\t1264,500000\t498,000000\t500,000000\r\n497\t313031757\t1266,000000\t497,750000\t500,000000\r\n498\t313032898\t1264,500000\t498,250000\t500,000000\r\n499\t313034034\t1267,000000\t498,000000\t500,000000\r\n500\t313035167\t1266,500000\t498,250000\t500,000000\r\n501\t313036305\t1262,500000\t498,750000\t500,000000\r\n502\t313037443\t1263,500000\t498,000000\t500,000000\r\n503\t313038580\t1262,500000\t498,250000\t500,000000\r\n504\t313039714\t1265,500000\t498,500000\t500,000000\r\n505\t313040850\t1265,000000\t498,250000\t500,000000\r\n506\t313041987\t1262,000000\t497,750000\t500,000000\r\n507\t313043128\t1263,500000\t499,000000\t500,000000\r\n508\t313044268\t1264,500000\t497,750000\t500,000000\r\n509\t313045411\t1264,500000\t498,750000\t500,000000\r\n510\t313046548\t1264,000000\t498,500000\t500,000000\r\n511\t313047683\t1261,000000\t499,250000\t500,000000\r\n512\t313048827\t1263,500000\t498,000000\t500,000000\r\n513\t313049959\t1262,500000\t498,250000\t500,000000\r\n514\t313051092\t1263,500000\t498,000000\t500,000000\r\n515\t313052228\t1263,000000\t497,750000\t500,000000\r\n516\t313053368\t1263,000000\t498,000000\t500,000000\r\n517\t313054503\t1264,500000\t498,500000\t500,000000\r\n518\t313055637\t1261,000000\t497,200000\t500,000000\r\n519\t313056771\t1263,000000\t498,250000\t500,000000\r\n520\t313057899\t1262,000000\t497,750000\t500,000000\r\n521\t313059036\t1262,000000\t498,250000\t500,000000\r\n522\t313060166\t1262,000000\t498,000000\t500,000000\r\n523\t313061304\t1263,500000\t497,200000\t500,000000\r\n524\t313062439\t1262,000000\t497,750000\t500,000000\r\n525\t313063573\t1261,000000\t499,000000\t500,000000\r\n526\t313064720\t1261,500000\t498,500000\t500,000000\r\n527\t313065861\t1262,500000\t497,500000\t500,000000\r\n528\t313066990\t1260,000000\t498,000000\t500,000000\r\n529\t313068124\t1262,000000\t497,750000\t500,000000\r\n530\t313069278\t1261,500000\t498,500000\t500,000000\r\n531\t313070412\t1261,500000\t498,500000\t500,000000\r\n532\t313071548\t1260,000000\t498,500000\t500,000000\r\n533\t313072682\t1261,000000\t498,750000\t500,000000\r\n534\t313073823\t1259,000000\t498,750000\t500,000000\r\n535\t313074961\t1260,000000\t497,450000\t500,000000\r\n536\t313076099\t1261,000000\t497,500000\t500,000000\r\n537\t313077237\t1257,500000\t497,250000\t500,000000\r\n538\t313078373\t1260,000000\t498,250000\t500,000000\r\n539\t313079513\t1263,000000\t498,000000\t500,000000\r\n540\t313080656\t1258,000000\t497,500000\t500,000000\r\n541\t313081793\t1262,000000\t498,500000\t500,000000\r\n542\t313082929\t1259,500000\t498,750000\t500,000000\r\n543\t313084066\t1259,500000\t497,450000\t500,000000\r\n544\t313085205\t1261,000000\t497,750000\t500,000000\r\n545\t313086349\t1259,000000\t498,000000\t500,000000\r\n546\t313087490\t1257,500000\t498,750000\t500,000000\r\n547\t313088623\t1257,000000\t499,000000\t500,000000\r\n548\t313089756\t1257,500000\t498,500000\t500,000000\r\n549\t313090893\t1258,000000\t499,250000\t500,000000\r\n550\t313092028\t1257,000000\t498,750000\t500,000000\r\n551\t313093181\t1260,500000\t498,000000\t500,000000\r\n552\t313094318\t1257,000000\t498,500000\t500,000000\r\n553\t313095458\t1256,000000\t499,000000\t500,000000\r\n554\t313096589\t1257,500000\t498,250000\t500,000000\r\n555\t313097727\t1258,000000\t497,750000\t500,000000\r\n556\t313098865\t1255,500000\t498,250000\t500,000000\r\n557\t313099997\t1259,000000\t497,750000\t500,000000\r\n558\t313101133\t1255,500000\t498,500000\t500,000000\r\n559\t313102275\t1257,000000\t498,500000\t500,000000\r\n560\t313103410\t1256,500000\t498,250000\t500,000000\r\n561\t313104550\t1256,000000\t498,750000\t500,000000\r\n562\t313105681\t1257,500000\t499,250000\t500,000000\r\n563\t313106821\t1256,500000\t498,000000\t500,000000\r\n564\t313107961\t1256,000000\t498,000000\t500,000000\r\n565\t313109095\t1255,000000\t498,500000\t500,000000\r\n566\t313110233\t1255,500000\t498,500000\t500,000000\r\n567\t313111381\t1256,000000\t498,250000\t500,000000\r\n568\t313112520\t1255,500000\t498,750000\t500,000000\r\n569\t313113655\t1254,400000\t498,250000\t500,000000\r\n570\t313114798\t1255,000000\t498,500000\t500,000000\r\n571\t313115928\t1257,000000\t498,000000\t500,000000\r\n572\t313117062\t1253,500000\t499,250000\t500,000000\r\n573\t313118197\t1256,500000\t498,250000\t500,000000\r\n574\t313119334\t1255,500000\t498,500000\t500,000000\r\n575\t313120477\t1254,500000\t497,250000\t500,000000\r\n576\t313121613\t1252,500000\t497,500000\t500,000000\r\n577\t313122746\t1254,000000\t498,750000\t500,000000\r\n578\t313123883\t1254,500000\t498,250000\t500,000000\r\n579\t313125029\t1252,500000\t499,250000\t500,000000\r\n580\t313126171\t1254,000000\t498,500000\t500,000000\r\n581\t313127311\t1252,500000\t498,250000\t500,000000\r\n582\t313128447\t1255,500000\t498,250000\t500,000000\r\n583\t313129581\t1252,500000\t498,250000\t500,000000\r\n584\t313130721\t1249,900000\t498,250000\t500,000000\r\n585\t313131856\t1254,500000\t498,250000\t500,000000\r\n586\t313133001\t1254,000000\t498,750000\t500,000000\r\n587\t313134140\t1253,500000\t497,750000\t500,000000\r\n588\t313135276\t1253,000000\t497,750000\t500,000000\r\n589\t313136413\t1253,500000\t498,500000\t500,000000\r\n590\t313137560\t1251,000000\t498,500000\t500,000000\r\n591\t313138694\t1251,000000\t498,000000\t500,000000\r\n592\t313139836\t1251,500000\t498,250000\t500,000000\r\n593\t313140979\t1251,500000\t498,000000\t500,000000\r\n594\t313142115\t1251,500000\t497,750000\t500,000000\r\n596\t313144239\t1254,000000\t498,250000\t500,000000\r\n597\t313145376\t1251,000000\t498,000000\t500,000000\r\n598\t313146505\t1250,500000\t497,500000\t500,000000\r\n599\t313147637\t1253,500000\t498,250000\t500,000000\r\n600\t313148765\t1251,000000\t498,250000\t500,000000\r\n601\t313149900\t1252,000000\t497,750000\t500,000000\r\n602\t313151037\t1251,000000\t498,500000\t500,000000\r\n603\t313152171\t1250,000000\t498,250000\t500,000000\r\n604\t313153316\t1252,500000\t498,500000\t500,000000\r\n605\t313154456\t1252,500000\t499,000000\t500,000000\r\n606\t313155591\t1252,000000\t497,750000\t500,000000\r\n607\t313156733\t1250,500000\t498,500000\t500,000000\r\n608\t313157872\t1249,500000\t498,250000\t500,000000\r\n609\t313159009\t1249,000000\t498,000000\t500,000000\r\n610\t313160145\t1249,500000\t499,250000\t500,000000\r\n611\t313161285\t1249,500000\t498,750000\t500,000000\r\n612\t313162426\t1252,000000\t498,250000\t500,000000\r\n613\t313163567\t1253,000000\t499,000000\t500,000000\r\n614\t313164709\t1251,500000\t497,750000\t500,000000\r\n615\t313165844\t1250,500000\t498,000000\t500,000000\r\n616\t313166986\t1249,500000\t498,250000\t500,000000\r\n617\t313168118\t1249,500000\t498,500000\t500,000000\r\n618\t313169255\t1249,500000\t497,200000\t500,000000\r\n619\t313170397\t1250,000000\t498,250000\t500,000000\r\n620\t313171526\t1249,000000\t498,500000\t500,000000\r\n621\t313172666\t1248,500000\t499,000000\t500,000000\r\n622\t313173797\t1249,500000\t498,000000\t500,000000\r\n623\t313174934\t1249,000000\t498,500000\t500,000000\r\n624\t313176075\t1249,000000\t497,500000\t500,000000\r\n625\t313177211\t1248,400000\t499,000000\t500,000000\r\n626\t313178348\t1248,000000\t497,500000\t500,000000\r\n627\t313179485\t1247,400000\t498,500000\t500,000000\r\n628\t313180621\t1247,400000\t497,750000\t500,000000\r\n629\t313181767\t1243,900000\t498,000000\t500,000000\r\n630\t313182901\t1247,500000\t498,000000\t500,000000\r\n631\t313184039\t1248,000000\t497,000000\t500,000000\r\n632\t313185173\t1245,400000\t497,750000\t500,000000\r\n633\t313186309\t1245,400000\t498,250000\t500,000000\r\n634\t313187441\t1244,900000\t497,500000\t500,000000\r\n635\t313188571\t1247,500000\t498,200000\t500,000000\r\n636\t313189711\t1246,500000\t498,250000\t500,000000\r\n637\t313190844\t1247,000000\t498,250000\t500,000000\r\n638\t313191976\t1247,500000\t499,000000\t500,000000\r\n639\t313193116\t1248,000000\t498,000000\t500,000000\r\n640\t313194253\t1245,500000\t498,000000\t500,000000\r\n641\t313195385\t1244,000000\t498,250000\t500,000000\r\n642\t313196519\t1245,500000\t498,500000\t500,000000\r\n643\t313197665\t1246,500000\t498,750000\t500,000000\r\n644\t313198803\t1247,500000\t497,250000\t500,000000\r\n645\t313199943\t1244,900000\t498,000000\t500,000000\r\n646\t313201080\t1246,000000\t497,250000\t500,000000\r\n647\t313202218\t1245,500000\t497,750000\t500,000000\r\n648\t313203358\t1244,400000\t498,500000\t500,000000\r\n649\t313204497\t1244,000000\t498,250000\t500,000000\r\n650\t313205638\t1246,000000\t498,750000\t500,000000\r\n651\t313206777\t1244,900000\t498,500000\t500,000000\r\n652\t313207914\t1244,900000\t499,250000\t500,000000\r\n653\t313209052\t1245,000000\t498,250000\t500,000000\r\n654\t313210189\t1242,900000\t498,250000\t500,000000\r\n655\t313211332\t1245,500000\t498,000000\t500,000000\r\n656\t313212470\t1247,000000\t499,250000\t500,000000\r\n657\t313213603\t1243,500000\t497,750000\t500,000000\r\n658\t313214741\t1242,500000\t498,250000\t500,000000\r\n659\t313215891\t1246,500000\t498,750000\t500,000000\r\n660\t313217022\t1242,500000\t497,750000\t500,000000\r\n661\t313218159\t1244,000000\t496,750000\t500,000000\r\n662\t313219299\t1242,400000\t498,250000\t500,000000\r\n663\t313220440\t1242,400000\t498,000000\t500,000000\r\n664\t313221584\t1243,500000\t498,250000\t500,000000\r\n665\t313222725\t1243,400000\t498,000000\t500,000000\r\n666\t313223864\t1242,400000\t498,000000\t500,000000\r\n667\t313225002\t1243,000000\t497,750000\t500,000000\r\n668\t313226143\t1243,000000\t499,000000\t500,000000\r\n669\t313227281\t1242,500000\t497,500000\t500,000000\r\n670\t313228425\t1240,800000\t498,250000\t500,000000\r\n671\t313229558\t1242,500000\t498,500000\t500,000000\r\n672\t313230696\t1244,000000\t498,250000\t500,000000\r\n673\t313231837\t1243,500000\t498,750000\t500,000000\r\n674\t313232981\t1240,900000\t497,500000\t500,000000\r\n675\t313234118\t1240,300000\t498,000000\t500,000000\r\n676\t313235249\t1242,700000\t497,250000\t500,000000\r\n677\t313236392\t1241,300000\t498,250000\t500,000000\r\n678\t313237525\t1243,000000\t497,750000\t500,000000\r\n679\t313238658\t1240,900000\t498,750000\t500,000000\r\n680\t313239806\t1240,200000\t499,000000\t500,000000\r\n681\t313240956\t1240,800000\t498,750000\t500,000000\r\n682\t313242097\t1243,300000\t497,700000\t500,000000\r\n683\t313243235\t1243,300000\t498,500000\t500,000000\r\n684\t313244378\t1238,000000\t498,000000\t500,000000\r\n685\t313245517\t1242,200000\t498,500000\t500,000000\r\n686\t313246650\t1239,100000\t498,250000\t500,000000\r\n687\t313247785\t1242,400000\t498,250000\t500,000000\r\n688\t313248925\t1239,600000\t498,250000\t500,000000\r\n689\t313250063\t1240,400000\t498,250000\t500,000000\r\n690\t313251201\t1239,800000\t498,250000\t500,000000\r\n691\t313252333\t1240,400000\t497,750000\t500,000000\r\n692\t313253470\t1242,800000\t497,500000\t500,000000\r\n693\t313254608\t1239,000000\t498,250000\t500,000000\r\n694\t313255749\t1238,500000\t498,500000\t500,000000\r\n695\t313256887\t1239,500000\t498,750000\t500,000000\r\n696\t313258029\t1238,500000\t498,750000\t500,000000\r\n697\t313259169\t1237,600000\t498,250000\t500,000000\r\n698\t313260305\t1240,700000\t498,250000\t500,000000\r\n699\t313261437\t1236,200000\t498,250000\t500,000000\r\n700\t313262579\t1238,100000\t498,250000\t500,000000\r\n701\t313263714\t1235,200000\t498,500000\t500,000000\r\n702\t313264848\t1236,800000\t498,750000\t500,000000\r\n703\t313265993\t1237,300000\t497,750000\t500,000000\r\n704\t313267125\t1239,500000\t498,500000\t500,000000\r\n705\t313268260\t1236,900000\t498,500000\t500,000000\r\n706\t313269396\t1238,000000\t497,500000\t500,000000\r\n707\t313270530\t1239,500000\t498,500000\t500,000000\r\n708\t313271667\t1236,300000\t498,000000\t500,000000\r\n709\t313272805\t1236,700000\t498,500000\t500,000000\r\n710\t313273946\t1235,800000\t499,250000\t500,000000\r\n711\t313275086\t1235,200000\t498,250000\t500,000000\r\n712\t313276227\t1236,200000\t498,000000\t500,000000\r\n713\t313277367\t1236,400000\t498,750000\t500,000000\r\n714\t313278501\t1237,800000\t497,000000\t500,000000\r\n715\t313279638\t1236,200000\t498,750000\t500,000000\r\n716\t313280774\t1236,300000\t498,500000\t500,000000\r\n717\t313281907\t1236,300000\t498,000000\t500,000000\r\n718\t313283044\t1232,500000\t496,750000\t500,000000\r\n719\t313284181\t1234,100000\t498,000000\t500,000000\r\n720\t313285326\t1233,200000\t497,700000\t500,000000\r\n721\t313286465\t1239,000000\t498,250000\t500,000000\r\n722\t313287594\t1235,700000\t497,750000\t500,000000\r\n723\t313288728\t1234,100000\t497,750000\t500,000000\r\n724\t313289867\t1233,000000\t497,750000\t500,000000\r\n725\t313291002\t1236,300000\t499,000000\t500,000000\r\n726\t313292143\t1233,100000\t498,500000\t500,000000\r\n727\t313293281\t1236,400000\t498,000000\t500,000000\r\n728\t313294418\t1233,500000\t497,000000\t500,000000\r\n729\t313295557\t1233,600000\t498,000000\t500,000000\r\n730\t313296696\t1233,200000\t498,750000\t500,000000\r\n731\t313297832\t1236,300000\t498,000000\t500,000000\r\n732\t313298967\t1234,100000\t498,250000\t500,000000\r\n733\t313300107\t1232,500000\t498,250000\t500,000000\r\n734\t313301249\t1235,100000\t498,750000\t500,000000\r\n735\t313302390\t1232,500000\t498,500000\t500,000000\r\n736\t313303527\t1234,100000\t498,000000\t500,000000\r\n737\t313304668\t1232,500000\t497,750000\t500,000000\r\n738\t313305811\t1233,600000\t498,000000\t500,000000\r\n739\t313306946\t1230,500000\t498,500000\t500,000000\r\n740\t313308086\t1232,100000\t499,000000\t500,000000\r\n741\t313309226\t1234,700000\t499,500000\t500,000000\r\n742\t313310366\t1233,100000\t497,750000\t500,000000\r\n743\t313311503\t1232,600000\t498,000000\t500,000000\r\n744\t313312646\t1231,600000\t498,250000\t500,000000\r\n745\t313313781\t1232,600000\t499,250000\t500,000000\r\n746\t313314920\t1230,500000\t498,000000\t500,000000\r\n747\t313316053\t1232,000000\t498,000000\t500,000000\r\n748\t313317190\t1230,000000\t499,000000\t500,000000\r\n749\t313318329\t1233,700000\t498,000000\t500,000000\r\n750\t313319373\t1232,000000\t498,500000\t500,000000\r\n751\t313320512\t1232,100000\t497,750000\t500,000000\r\n752\t313321649\t1230,500000\t498,250000\t500,000000\r\n753\t313322786\t1229,500000\t498,250000\t500,000000\r\n754\t313323922\t1232,100000\t498,000000\t500,000000\r\n755\t313325061\t1231,100000\t498,250000\t500,000000\r\n756\t313326199\t1231,500000\t499,250000\t500,000000\r\n757\t313327331\t1232,500000\t497,750000\t500,000000\r\n758\t313328296\t1232,000000\t498,250000\t500,000000\r\n759\t313329430\t1230,000000\t498,000000\t500,000000\r\n760\t313330567\t1233,600000\t497,500000\t500,000000\r\n761\t313331710\t1227,500000\t498,750000\t500,000000\r\n762\t313332847\t1231,000000\t497,500000\t500,000000\r\n763\t313333985\t1231,600000\t497,750000\t500,000000\r\n764\t313335129\t1229,500000\t498,500000\t500,000000\r\n765\t313336276\t1230,600000\t498,500000\t500,000000\r\n766\t313337419\t1231,600000\t498,500000\t500,000000\r\n767\t313338552\t1230,000000\t498,000000\t500,000000\r\n768\t313339694\t1231,500000\t498,500000\t500,000000\r\n769\t313340833\t1232,200000\t499,000000\t500,000000\r\n770\t313341974\t1232,700000\t497,750000\t500,000000\r\n771\t313343114\t1229,000000\t497,500000\t500,000000\r\n772\t313344254\t1229,100000\t498,000000\t500,000000\r\n773\t313345396\t1230,700000\t498,000000\t500,000000\r\n774\t313346534\t1230,600000\t497,750000\t500,000000\r\n775\t313347666\t1228,500000\t498,500000\t500,000000\r\n776\t313348808\t1229,000000\t497,750000\t500,000000\r\n777\t313349945\t1230,000000\t497,750000\t500,000000\r\n778\t313351084\t1231,600000\t498,500000\t500,000000\r\n779\t313352216\t1229,000000\t497,750000\t500,000000\r\n780\t313353358\t1231,100000\t499,000000\t500,000000\r\n781\t313354497\t1226,500000\t497,500000\t500,000000\r\n782\t313355637\t1231,100000\t498,000000\t500,000000\r\n783\t313356772\t1227,000000\t498,500000\t500,000000\r\n784\t313357906\t1230,000000\t498,000000\t500,000000\r\n785\t313359049\t1228,000000\t498,000000\t500,000000\r\n786\t313360192\t1228,000000\t498,000000\t500,000000\r\n787\t313361325\t1226,000000\t498,250000\t500,000000\r\n788\t313362460\t1228,600000\t498,000000\t500,000000\r\n789\t313363599\t1227,500000\t498,250000\t500,000000\r\n790\t313364741\t1227,000000\t498,000000\t500,000000\r\n791\t313365882\t1227,500000\t497,750000\t500,000000\r\n792\t313367028\t1227,000000\t498,250000\t500,000000\r\n793\t313368160\t1227,500000\t498,000000\t500,000000\r\n794\t313369292\t1226,000000\t498,750000\t500,000000\r\n795\t313370429\t1227,500000\t497,750000\t500,000000\r\n796\t313371570\t1229,000000\t498,250000\t500,000000\r\n797\t313372714\t1227,000000\t498,500000\t500,000000\r\n798\t313373852\t1226,000000\t498,250000\t500,000000\r\n799\t313374982\t1226,000000\t498,500000\t500,000000\r\n800\t313376115\t1226,500000\t497,200000\t500,000000\r\n801\t313377254\t1227,000000\t498,250000\t500,000000\r\n802\t313378390\t1226,500000\t498,500000\t500,000000\r\n803\t313379529\t1226,500000\t497,750000\t500,000000\r\n804\t313380665\t1224,500000\t498,000000\t500,000000\r\n805\t313381800\t1226,000000\t498,500000\t500,000000\r\n806\t313382935\t1225,500000\t498,000000\t500,000000\r\n807\t313384071\t1227,500000\t498,500000\t500,000000\r\n808\t313385211\t1224,000000\t498,250000\t500,000000\r\n809\t313386346\t1225,500000\t498,000000\t500,000000\r\n810\t313387488\t1225,000000\t498,750000\t500,000000\r\n811\t313388623\t1225,000000\t498,250000\t500,000000\r\n812\t313389753\t1224,500000\t498,500000\t500,000000\r\n813\t313390894\t1226,500000\t498,000000\t500,000000\r\n814\t313392028\t1225,500000\t498,250000\t500,000000\r\n815\t313393164\t1225,000000\t499,500000\t500,000000\r\n816\t313394303\t1224,000000\t498,500000\t500,000000\r\n817\t313395440\t1224,100000\t498,250000\t500,000000\r\n818\t313396578\t1225,500000\t497,750000\t500,000000\r\n819\t313397710\t1225,500000\t499,000000\t500,000000\r\n820\t313398842\t1224,000000\t498,250000\t500,000000\r\n821\t313399981\t1226,000000\t498,500000\t500,000000\r\n822\t313401126\t1222,500000\t498,750000\t500,000000\r\n823\t313402267\t1221,500000\t498,500000\t500,000000\r\n824\t313403406\t1221,500000\t498,500000\t500,000000\r\n825\t313404542\t1223,500000\t498,250000\t500,000000\r\n826\t313405685\t1224,000000\t498,500000\t500,000000\r\n827\t313406825\t1222,500000\t498,250000\t500,000000\r\n828\t313407958\t1223,500000\t498,250000\t500,000000\r\n829\t313409091\t1221,500000\t498,750000\t500,000000\r\n830\t313410225\t1222,000000\t497,500000\t500,000000\r\n831\t313411359\t1224,500000\t498,500000\t500,000000\r\n832\t313412499\t1222,500000\t498,250000\t500,000000\r\n833\t313413641\t1220,500000\t498,250000\t500,000000\r\n834\t313414780\t1222,000000\t498,250000\t500,000000\r\n835\t313415922\t1222,000000\t498,500000\t500,000000\r\n836\t313417057\t1223,000000\t498,750000\t500,000000\r\n837\t313418191\t1222,500000\t497,500000\t500,000000\r\n838\t313419325\t1221,500000\t498,000000\t500,000000\r\n839\t313420457\t1221,000000\t498,000000\t500,000000\r\n840\t313421592\t1220,500000\t499,000000\t500,000000\r\n841\t313422730\t1221,000000\t498,250000\t500,000000\r\n842\t313423866\t1223,500000\t498,250000\t500,000000\r\n843\t313425006\t1222,000000\t497,750000\t500,000000\r\n844\t313426144\t1220,500000\t498,000000\t500,000000\r\n845\t313427276\t1218,000000\t498,000000\t500,000000\r\n846\t313428411\t1221,000000\t497,200000\t500,000000\r\n847\t313429555\t1219,000000\t498,500000\t500,000000\r\n848\t313430697\t1220,500000\t497,750000\t500,000000\r\n849\t313431835\t1221,500000\t497,200000\t500,000000\r\n850\t313432972\t1221,000000\t498,000000\t500,000000\r\n851\t313434115\t1218,500000\t497,250000\t500,000000\r\n852\t313435258\t1218,000000\t498,750000\t500,000000\r\n853\t313436394\t1217,500000\t498,500000\t500,000000\r\n854\t313437535\t1218,000000\t498,000000\t500,000000\r\n855\t313438673\t1217,000000\t497,450000\t500,000000\r\n856\t313439807\t1217,000000\t498,750000\t500,000000\r\n857\t313440937\t1219,000000\t498,500000\t500,000000\r\n859\t313443138\t1217,500000\t497,750000\t500,000000\r\n860\t313444275\t1216,000000\t498,500000\t500,000000\r\n861\t313445411\t1217,500000\t498,000000\t500,000000\r\n862\t313446547\t1217,500000\t498,250000\t500,000000\r\n863\t313447676\t1220,000000\t498,500000\t500,000000\r\n864\t313448810\t1215,500000\t498,000000\t500,000000\r\n865\t313449948\t1220,000000\t497,750000\t500,000000\r\n866\t313451081\t1217,000000\t497,450000\t500,000000\r\n867\t313452212\t1218,500000\t497,750000\t500,000000\r\n868\t313453351\t1219,000000\t499,000000\t500,000000\r\n869\t313454486\t1216,500000\t498,500000\t500,000000\r\n870\t313455618\t1220,000000\t497,500000\t500,000000\r\n871\t313456756\t1218,500000\t498,250000\t500,000000\r\n872\t313457896\t1216,500000\t498,000000\t500,000000\r\n873\t313459039\t1216,500000\t498,500000\t500,000000\r\n874\t313460178\t1217,500000\t498,000000\t500,000000\r\n875\t313461318\t1217,000000\t498,250000\t500,000000\r\n876\t313462458\t1214,500000\t498,500000\t500,000000\r\n877\t313464102\t1216,500000\t499,250000\t500,000000\r\n878\t313465796\t1216,000000\t498,500000\t500,000000\r\n879\t313467495\t1216,500000\t498,500000\t500,000000\r\n880\t313469188\t1214,000000\t498,000000\t500,000000\r\n881\t313470893\t1216,500000\t498,750000\t500,000000\r\n882\t313472591\t1214,500000\t498,250000\t500,000000\r\n883\t313474287\t1216,500000\t498,750000\t500,000000\r\n884\t313475983\t1214,000000\t498,500000\t500,000000\r\n885\t313477687\t1214,500000\t498,250000\t500,000000\r\n886\t313479383\t1213,000000\t497,200000\t500,000000\r\n887\t313481078\t1217,000000\t498,750000\t500,000000\r\n888\t313482778\t1214,000000\t498,000000\t500,000000\r\n889\t313484478\t1213,500000\t498,000000\t500,000000\r\n890\t313486176\t1211,500000\t498,500000\t500,000000\r\n891\t313487874\t1213,500000\t498,250000\t500,000000\r\n892\t313489572\t1215,000000\t498,000000\t500,000000\r\n893\t313491277\t1214,500000\t498,250000\t500,000000\r\n894\t313492983\t1212,500000\t498,500000\t500,000000\r\n895\t313494688\t1213,000000\t497,200000\t500,000000\r\n896\t313496393\t1212,000000\t498,500000\t500,000000\r\n897\t313498090\t1213,000000\t498,750000\t500,000000\r\n898\t313499794\t1215,500000\t498,000000\t500,000000\r\n899\t313501496\t1210,500000\t498,250000\t500,000000\r\n900\t313503205\t1212,500000\t498,250000\t500,000000\r\n901\t313504908\t1210,000000\t498,250000\t500,000000\r\n902\t313506617\t1211,500000\t498,000000\t500,000000\r\n903\t313508326\t1211,500000\t498,000000\t500,000000\r\n904\t313510033\t1212,500000\t497,000000\t500,000000\r\n905\t313511741\t1210,500000\t498,500000\t500,000000\r\n906\t313513442\t1210,500000\t498,500000\t500,000000\r\n907\t313515145\t1212,000000\t497,750000\t500,000000\r\n908\t313516849\t1213,000000\t498,000000\t500,000000\r\n909\t313518559\t1213,000000\t499,250000\t500,000000\r\n910\t313520261\t1211,500000\t498,250000\t500,000000\r\n911\t313521952\t1210,500000\t498,250000\t500,000000\r\n912\t313523649\t1212,000000\t498,000000\t500,000000\r\n913\t313525353\t1213,500000\t498,500000\t500,000000\r\n914\t313527052\t1210,500000\t498,500000\t500,000000\r\n915\t313528753\t1213,500000\t498,250000\t500,000000\r\n916\t313530451\t1213,000000\t497,250000\t500,000000\r\n917\t313532156\t1210,500000\t498,500000\t500,000000\r\n918\t313533853\t1210,500000\t498,500000\t500,000000\r\n919\t313535559\t1209,500000\t498,000000\t500,000000\r\n920\t313537263\t1212,000000\t497,750000\t500,000000\r\n921\t313538951\t1211,500000\t498,250000\t500,000000\r\n922\t313540651\t1209,500000\t498,750000\t500,000000\r\n923\t313542359\t1209,000000\t497,750000\t500,000000\r\n924\t313544067\t1210,000000\t498,250000\t500,000000\r\n925\t313545769\t1210,000000\t498,750000\t500,000000\r\n926\t313547471\t1208,000000\t498,750000\t500,000000\r\n927\t313549178\t1210,000000\t497,750000\t500,000000\r\n928\t313550879\t1209,500000\t497,750000\t500,000000\r\n929\t313552586\t1207,500000\t498,750000\t500,000000\r\n930\t313554287\t1210,000000\t498,000000\t500,000000\r\n931\t313555983\t1209,000000\t498,250000\t500,000000\r\n932\t313557686\t1208,500000\t498,200000\t500,000000\r\n933\t313559387\t1208,000000\t498,000000\t500,000000\r\n934\t313561094\t1207,000000\t498,750000\t500,000000\r\n935\t313562798\t1210,000000\t498,500000\t500,000000\r\n936\t313564501\t1208,500000\t498,750000\t500,000000\r\n937\t313566207\t1208,000000\t498,500000\t500,000000\r\n938\t313567907\t1208,500000\t497,500000\t500,000000\r\n939\t313569612\t1208,000000\t499,000000\t500,000000\r\n940\t313571313\t1207,000000\t498,500000\t500,000000\r\n941\t313573009\t1209,000000\t497,750000\t500,000000\r\n942\t313574717\t1204,900000\t498,250000\t500,000000\r\n943\t313576422\t1206,000000\t499,000000\t500,000000\r\n944\t313578124\t1206,500000\t498,500000\t500,000000\r\n945\t313579828\t1209,000000\t497,750000\t500,000000\r\n946\t313581532\t1207,000000\t498,750000\t500,000000\r\n947\t313583241\t1208,500000\t499,000000\t500,000000\r\n948\t313584952\t1203,000000\t497,250000\t500,000000\r\n949\t313586647\t1206,000000\t498,000000\t500,000000\r\n950\t313588346\t1206,500000\t498,750000\t500,000000\r\n951\t313590047\t1205,000000\t498,250000\t500,000000\r\n952\t313591749\t1206,500000\t497,750000\t500,000000\r\n953\t313593427\t1204,000000\t498,750000\t500,000000\r\n954\t313595126\t1206,500000\t498,250000\t500,000000\r\n955\t313596828\t1206,500000\t498,500000\t500,000000\r\n956\t313598525\t1201,000000\t498,250000\t500,000000\r\n957\t313600224\t1204,500000\t498,250000\t500,000000\r\n958\t313601927\t1204,000000\t498,750000\t500,000000\r\n959\t313603627\t1203,000000\t498,250000\t500,000000\r\n960\t313605328\t1204,000000\t498,500000\t500,000000\r\n961\t313607034\t1204,500000\t497,450000\t500,000000\r\n962\t313608735\t1203,500000\t498,000000\t500,000000\r\n963\t313610429\t1202,500000\t498,250000\t500,000000\r\n964\t313612133\t1203,500000\t498,250000\t500,000000\r\n965\t313613831\t1202,500000\t499,250000\t500,000000\r\n966\t313615532\t1201,500000\t498,250000\t500,000000\r\n967\t313617229\t1204,000000\t498,000000\t500,000000\r\n968\t313618932\t1202,000000\t498,500000\t500,000000\r\n969\t313620069\t1202,500000\t497,750000\t500,000000\r\n970\t313621207\t1202,500000\t498,000000\t500,000000\r\n971\t313622339\t1201,500000\t497,500000\t500,000000\r\n972\t313623475\t1201,500000\t499,000000\t500,000000\r\n973\t313624616\t1201,000000\t498,250000\t500,000000\r\n974\t313625748\t1202,500000\t499,000000\t500,000000\r\n975\t313626883\t1202,000000\t498,500000\t500,000000\r\n976\t313628016\t1202,000000\t498,000000\t500,000000\r\n977\t313629035\t1200,500000\t498,250000\t500,000000\r\n978\t313630062\t1200,000000\t497,750000\t500,000000\r\n979\t313631191\t1202,000000\t498,250000\t500,000000\r\n980\t313632326\t1201,500000\t498,500000\t500,000000\r\n981\t313633463\t1202,000000\t499,000000\t500,000000\r\n982\t313634605\t1200,000000\t498,500000\t500,000000\r\n983\t313635740\t1202,000000\t498,000000\t500,000000\r\n984\t313636879\t1203,000000\t498,000000\t500,000000\r\n985\t313638017\t1201,000000\t498,000000\t500,000000\r\n986\t313639159\t1198,000000\t498,000000\t500,000000\r\n987\t313640296\t1201,500000\t498,000000\t500,000000\r\n988\t313641435\t1202,000000\t498,000000\t500,000000\r\n989\t313642574\t1199,500000\t499,250000\t500,000000\r\n990\t313643720\t1202,000000\t498,000000\t500,000000\r\n991\t313644862\t1200,500000\t499,000000\t500,000000\r\n992\t313645993\t1202,500000\t498,250000\t500,000000\r\n993\t313647136\t1201,500000\t498,750000\t500,000000\r\n994\t313648265\t1199,000000\t498,750000\t500,000000\r\n995\t313649404\t1198,000000\t498,000000\t500,000000\r\n996\t313650549\t1199,000000\t497,750000\t500,000000\r\n997\t313651685\t1199,500000\t499,250000\t500,000000\r\n998\t313652819\t1198,500000\t498,000000\t500,000000\r\n999\t313653956\t1198,500000\t499,000000\t500,000000\r\n1000\t313655087\t1201,500000\t497,450000\t500,000000\r\n1001\t313656226\t1199,000000\t498,500000\t500,000000\r\n1002\t313657356\t1198,500000\t497,250000\t500,000000\r\n1003\t313658487\t1201,000000\t498,250000\t500,000000\r\n1004\t313659619\t1199,000000\t499,000000\t500,000000\r\n1005\t313660757\t1199,500000\t498,250000\t500,000000\r\n1006\t313661897\t1198,500000\t498,000000\t500,000000\r\n1007\t313663031\t1198,000000\t499,000000\t500,000000\r\n1008\t313664174\t1199,000000\t498,250000\t500,000000\r\n1009\t313665324\t1200,000000\t497,500000\t500,000000\r\n1010\t313666463\t1199,500000\t498,500000\t500,000000\r\n1011\t313667595\t1198,000000\t497,750000\t500,000000\r\n1012\t313668729\t1198,000000\t498,250000\t500,000000\r\n1013\t313669867\t1196,500000\t498,000000\t500,000000\r\n1014\t313671007\t1197,000000\t498,250000\t500,000000\r\n1015\t313672148\t1198,500000\t498,250000\t500,000000\r\n1016\t313673293\t1197,000000\t498,750000\t500,000000\r\n1017\t313674436\t1195,000000\t498,500000\t500,000000\r\n1018\t313675574\t1197,500000\t498,250000\t500,000000\r\n1019\t313676708\t1197,000000\t497,750000\t500,000000\r\n1020\t313677840\t1194,500000\t498,500000\t500,000000\r\n1021\t313678980\t1198,000000\t498,500000\t500,000000\r\n1022\t313680118\t1199,000000\t499,000000\t500,000000\r\n1023\t313681254\t1195,500000\t498,500000\t500,000000\r\n1024\t313682393\t1196,500000\t498,000000\t500,000000\r\n1025\t313683537\t1196,500000\t498,500000\t500,000000\r\n1026\t313684670\t1195,000000\t497,250000\t500,000000\r\n1027\t313685802\t1196,000000\t497,500000\t500,000000\r\n1028\t313686937\t1196,000000\t498,750000\t500,000000\r\n1029\t313688075\t1195,500000\t499,000000\t500,000000\r\n1030\t313689209\t1195,500000\t498,250000\t500,000000\r\n1031\t313690347\t1197,000000\t497,750000\t500,000000\r\n1032\t313691478\t1194,500000\t498,250000\t500,000000\r\n1033\t313692617\t1196,000000\t498,000000\t500,000000\r\n1034\t313693755\t1195,500000\t497,750000\t500,000000\r\n1035\t313694897\t1196,500000\t498,250000\t500,000000\r\n1036\t313696034\t1194,500000\t497,750000\t500,000000\r\n1037\t313697175\t1194,000000\t498,000000\t500,000000\r\n1038\t313698311\t1194,500000\t497,750000\t500,000000\r\n1039\t313699453\t1194,500000\t497,750000\t500,000000\r\n1040\t313700593\t1194,500000\t498,250000\t500,000000\r\n1041\t313701723\t1195,000000\t498,000000\t500,000000\r\n1042\t313702863\t1194,000000\t497,500000\t500,000000\r\n1043\t313703995\t1197,000000\t498,000000\t500,000000\r\n1044\t313705136\t1194,500000\t497,750000\t500,000000\r\n1045\t313706274\t1194,500000\t498,250000\t500,000000\r\n1047\t313708445\t1196,000000\t497,500000\t500,000000\r\n1048\t313709580\t1194,000000\t498,750000\t500,000000\r\n1049\t313710711\t1194,500000\t498,250000\t500,000000\r\n1050\t313711847\t1192,500000\t498,000000\t500,000000\r\n1051\t313712991\t1191,500000\t498,500000\t500,000000\r\n1052\t313714125\t1194,000000\t498,500000\t500,000000\r\n1053\t313715253\t1195,000000\t498,250000\t500,000000\r\n1054\t313716406\t1192,000000\t498,000000\t500,000000\r\n1055\t313717542\t1190,900000\t497,500000\t500,000000\r\n1056\t313718677\t1191,900000\t499,250000\t500,000000\r\n1057\t313719815\t1192,500000\t498,500000\t500,000000\r\n1058\t313720955\t1194,000000\t498,500000\t500,000000\r\n1059\t313722095\t1194,500000\t498,500000\t500,000000\r\n1060\t313723238\t1195,500000\t497,250000\t500,000000\r\n1061\t313724368\t1193,000000\t498,250000\t500,000000\r\n1062\t313725501\t1192,500000\t498,250000\t500,000000\r\n1063\t313726641\t1193,500000\t498,250000\t500,000000\r\n1064\t313727780\t1192,500000\t497,500000\t500,000000\r\n1065\t313728910\t1192,400000\t499,000000\t500,000000\r\n1066\t313730047\t1191,500000\t498,000000\t500,000000\r\n1067\t313731185\t1191,400000\t498,500000\t500,000000\r\n1068\t313732317\t1193,500000\t498,250000\t500,000000\r\n1069\t313733473\t1193,500000\t498,250000\t500,000000\r\n1070\t313734625\t1191,500000\t498,000000\t500,000000\r\n1071\t313735757\t1194,000000\t497,500000\t500,000000\r\n1072\t313736892\t1192,500000\t498,000000\t500,000000\r\n1073\t313738032\t1189,800000\t497,250000\t500,000000\r\n1074\t313739167\t1190,400000\t498,000000\t500,000000\r\n1075\t313740267\t1190,400000\t498,000000\t500,000000\r\n1076\t313741409\t1189,200000\t498,250000\t500,000000\r\n1077\t313742547\t1189,800000\t498,250000\t500,000000\r\n1078\t313743690\t1190,300000\t498,250000\t500,000000\r\n1079\t313744831\t1190,900000\t498,250000\t500,000000\r\n1080\t313745970\t1189,900000\t497,250000\t500,000000\r\n1081\t313747106\t1191,000000\t498,250000\t500,000000\r\n1082\t313748239\t1191,900000\t498,750000\t500,000000\r\n1083\t313749380\t1190,900000\t498,250000\t500,000000\r\n1084\t313750516\t1192,500000\t497,750000\t500,000000\r\n1085\t313751657\t1190,900000\t498,000000\t500,000000\r\n1086\t313752794\t1190,200000\t498,750000\t500,000000\r\n1087\t313753938\t1190,300000\t497,750000\t500,000000\r\n1088\t313755077\t1189,200000\t498,250000\t500,000000\r\n1089\t313756210\t1187,300000\t498,500000\t500,000000\r\n1090\t313757347\t1191,500000\t498,500000\t500,000000\r\n1091\t313758487\t1189,100000\t499,500000\t500,000000\r\n1092\t313759627\t1189,200000\t497,750000\t500,000000\r\n1093\t313760760\t1189,300000\t498,000000\t500,000000\r\n1094\t313761899\t1190,200000\t498,500000\t500,000000\r\n1095\t313763042\t1189,800000\t498,500000\t500,000000\r\n1096\t313764183\t1190,900000\t497,500000\t500,000000\r\n1097\t313765316\t1190,300000\t497,750000\t500,000000\r\n1098\t313766450\t1188,700000\t497,500000\t500,000000\r\n1099\t313767592\t1186,500000\t497,950000\t500,000000\r\n1100\t313768739\t1188,100000\t499,000000\t500,000000\r\n1101\t313769873\t1188,600000\t497,250000\t500,000000\r\n1102\t313771009\t1187,600000\t498,250000\t500,000000\r\n1103\t313772149\t1189,100000\t499,250000\t500,000000\r\n1104\t313773283\t1189,100000\t498,000000\t500,000000\r\n1105\t313774425\t1188,200000\t497,750000\t500,000000\r\n1106\t313775563\t1188,700000\t498,000000\t500,000000\r\n1107\t313776697\t1188,700000\t498,250000\t500,000000\r\n1108\t313777842\t1188,700000\t497,500000\t500,000000\r\n1109\t313778995\t1185,200000\t498,000000\t500,000000\r\n1110\t313780133\t1186,400000\t498,000000\t500,000000\r\n1111\t313781274\t1188,100000\t497,750000\t500,000000\r\n1112\t313782412\t1186,400000\t499,000000\t500,000000\r\n1113\t313783548\t1188,600000\t498,000000\t500,000000\r\n1114\t313784688\t1189,100000\t499,250000\t500,000000\r\n1115\t313785820\t1186,800000\t498,250000\t500,000000\r\n1116\t313786957\t1187,500000\t498,000000\t500,000000\r\n1117\t313788088\t1185,800000\t498,250000\t500,000000\r\n1118\t313789225\t1188,000000\t499,250000\t500,000000\r\n1119\t313790360\t1186,300000\t499,750000\t500,000000\r\n1120\t313791506\t1187,500000\t498,000000\t500,000000\r\n1121\t313792644\t1186,400000\t497,250000\t500,000000\r\n1122\t313793777\t1187,000000\t498,500000\t500,000000\r\n1123\t313794911\t1189,100000\t497,750000\t500,000000\r\n1124\t313796051\t1185,400000\t498,000000\t500,000000\r\n1125\t313797184\t1185,800000\t499,000000\t500,000000\r\n1126\t313798321\t1185,700000\t498,750000\t500,000000\r\n1127\t313799460\t1187,000000\t498,750000\t500,000000\r\n1128\t313800602\t1186,000000\t498,500000\t500,000000\r\n1129\t313801742\t1185,900000\t497,750000\t500,000000\r\n1130\t313802875\t1184,800000\t498,500000\t500,000000\r\n1131\t313804011\t1184,200000\t498,750000\t500,000000\r\n1132\t313805142\t1185,200000\t498,250000\t500,000000\r\n1133\t313806281\t1184,700000\t498,250000\t500,000000\r\n1134\t313807412\t1185,800000\t498,000000\t500,000000\r\n1135\t313808552\t1183,700000\t498,500000\t500,000000\r\n1136\t313809697\t1182,700000\t498,000000\t500,000000\r\n1137\t313810842\t1183,100000\t498,250000\t500,000000\r\n1138\t313811978\t1184,300000\t497,500000\t500,000000\r\n1139\t313813120\t1184,100000\t498,000000\t500,000000\r\n1140\t313814259\t1184,300000\t496,950000\t500,000000\r\n1141\t313815391\t1184,100000\t498,500000\t500,000000\r\n1142\t313816525\t1185,300000\t497,950000\t500,000000\r\n1143\t313817657\t1186,300000\t498,500000\t500,000000\r\n1144\t313818789\t1183,100000\t498,750000\t500,000000\r\n1145\t313819921\t1181,000000\t498,000000\t500,000000\r\n1146\t313821054\t1183,700000\t497,500000\t500,000000\r\n1147\t313822195\t1181,000000\t498,500000\t500,000000\r\n1148\t313823335\t1183,700000\t498,000000\t500,000000\r\n1149\t313824466\t1184,200000\t498,500000\t500,000000\r\n1150\t313825602\t1184,800000\t498,250000\t500,000000\r\n1151\t313826738\t1182,000000\t498,500000\t500,000000\r\n1152\t313827881\t1182,100000\t497,750000\t500,000000\r\n1153\t313829015\t1181,500000\t497,500000\t500,000000\r\n1154\t313830152\t1183,700000\t498,000000\t500,000000\r\n1155\t313831291\t1181,500000\t498,000000\t500,000000\r\n1156\t313832426\t1182,600000\t497,500000\t500,000000\r\n1157\t313833565\t1181,500000\t498,250000\t500,000000\r\n1158\t313834697\t1181,000000\t498,750000\t500,000000\r\n1159\t313835831\t1182,100000\t498,250000\t500,000000\r\n1160\t313836969\t1183,700000\t498,250000\t500,000000\r\n1161\t313838108\t1181,500000\t498,500000\t500,000000\r\n1162\t313839245\t1180,000000\t498,250000\t500,000000\r\n1163\t313840387\t1181,000000\t497,500000\t500,000000\r\n1164\t313841526\t1181,700000\t496,950000\t500,000000\r\n1165\t313842667\t1181,100000\t499,250000\t500,000000\r\n1166\t313843800\t1181,100000\t498,000000\t500,000000\r\n1167\t313844940\t1181,100000\t498,250000\t500,000000\r\n1168\t313846080\t1179,000000\t497,750000\t500,000000\r\n1169\t313847216\t1178,000000\t497,750000\t500,000000\r\n1170\t313848347\t1179,000000\t497,750000\t500,000000\r\n1171\t313849486\t1182,700000\t497,750000\t500,000000\r\n1172\t313850627\t1182,200000\t497,750000\t500,000000\r\n1173\t313851765\t1178,500000\t497,450000\t500,000000\r\n1174\t313852899\t1180,500000\t498,500000\t500,000000\r\n1175\t313854044\t1179,500000\t497,000000\t500,000000\r\n1176\t313855180\t1179,600000\t498,250000\t500,000000\r\n1177\t313856316\t1182,300000\t498,750000\t500,000000\r\n1178\t313857459\t1181,600000\t498,000000\t500,000000\r\n1179\t313858605\t1181,200000\t498,000000\t500,000000\r\n1180\t313859741\t1180,100000\t497,000000\t500,000000\r\n1181\t313860875\t1181,600000\t498,250000\t500,000000\r\n1182\t313862008\t1178,000000\t498,750000\t500,000000\r\n1183\t313863145\t1183,200000\t498,750000\t500,000000\r\n1184\t313864283\t1176,000000\t495,950000\t500,000000\r\n1185\t313865415\t1179,000000\t497,750000\t500,000000\r\n1186\t313866553\t1180,600000\t498,250000\t500,000000\r\n1187\t313867685\t1179,500000\t498,500000\t500,000000\r\n1188\t313868822\t1179,600000\t497,750000\t500,000000\r\n1189\t313869960\t1179,000000\t498,750000\t500,000000\r\n1190\t313871094\t1178,000000\t498,750000\t500,000000\r\n1191\t313872230\t1180,600000\t498,750000\t500,000000\r\n1192\t313873376\t1179,600000\t498,750000\t500,000000\r\n1193\t313874522\t1179,100000\t498,250000\t500,000000\r\n1194\t313875656\t1179,600000\t497,700000\t500,000000\r\n1195\t313876784\t1178,000000\t498,250000\t500,000000\r\n1196\t313877926\t1179,600000\t497,750000\t500,000000\r\n1197\t313879060\t1180,200000\t498,500000\t500,000000\r\n1198\t313880202\t1176,500000\t498,250000\t500,000000\r\n1199\t313881342\t1176,500000\t497,700000\t500,000000\r\n1200\t313882478\t1178,000000\t498,750000\t500,000000\r\n1201\t313883616\t1174,500000\t498,750000\t500,000000\r\n1202\t313884750\t1178,600000\t498,000000\t500,000000\r\n1203\t313885890\t1174,500000\t497,000000\t500,000000\r\n1204\t313887028\t1175,500000\t499,250000\t500,000000\r\n1205\t313888174\t1177,000000\t498,250000\t500,000000\r\n1206\t313889316\t1175,500000\t497,750000\t500,000000\r\n1207\t313890456\t1177,000000\t498,500000\t500,000000\r\n1208\t313891595\t1177,500000\t498,500000\t500,000000\r\n1209\t313892730\t1176,000000\t498,000000\t500,000000\r\n1210\t313893859\t1177,100000\t498,750000\t500,000000\r\n1211\t313894997\t1177,000000\t498,250000\t500,000000\r\n1212\t313896140\t1176,000000\t497,750000\t500,000000\r\n1213\t313897280\t1178,500000\t498,500000\t500,000000\r\n1214\t313898422\t1176,600000\t498,000000\t500,000000\r\n1215\t313899553\t1175,500000\t499,000000\t500,000000\r\n1216\t313900692\t1175,000000\t498,000000\t500,000000\r\n1217\t313901831\t1175,500000\t498,250000\t500,000000\r\n1218\t313902975\t1177,600000\t498,250000\t500,000000\r\n1219\t313904109\t1177,000000\t497,000000\t500,000000\r\n1220\t313905250\t1175,000000\t497,000000\t500,000000\r\n1221\t313906393\t1174,500000\t498,250000\t500,000000\r\n1222\t313907534\t1177,000000\t498,500000\t500,000000\r\n1223\t313908668\t1177,100000\t499,250000\t500,000000\r\n1224\t313909810\t1176,000000\t498,250000\t500,000000\r\n1225\t313910949\t1177,100000\t497,750000\t500,000000\r\n1226\t313912087\t1175,000000\t498,500000\t500,000000\r\n1227\t313913220\t1173,500000\t498,750000\t500,000000\r\n1228\t313914352\t1177,500000\t498,750000\t500,000000\r\n1229\t313915494\t1173,000000\t498,250000\t500,000000\r\n1230\t313916632\t1174,000000\t496,500000\t500,000000\r\n1231\t313917767\t1173,500000\t498,500000\t500,000000\r\n1232\t313918906\t1176,000000\t498,250000\t500,000000\r\n1233\t313920048\t1174,000000\t497,750000\t500,000000\r\n1234\t313921184\t1174,000000\t498,000000\t500,000000\r\n1235\t313922316\t1174,500000\t498,250000\t500,000000\r\n1236\t313923451\t1174,000000\t497,750000\t500,000000\r\n1237\t313924593\t1176,000000\t498,750000\t500,000000\r\n1238\t313925736\t1174,000000\t496,950000\t500,000000\r\n1239\t313926871\t1173,000000\t499,000000\t500,000000\r\n1240\t313928013\t1174,500000\t498,000000\t500,000000\r\n1241\t313929150\t1174,500000\t498,750000\t500,000000\r\n1242\t313930280\t1174,000000\t498,500000\t500,000000\r\n1243\t313931419\t1172,000000\t498,250000\t500,000000\r\n1244\t313932557\t1172,500000\t498,500000\t500,000000\r\n1245\t313933695\t1173,000000\t498,750000\t500,000000\r\n1246\t313934836\t1175,000000\t499,000000\t500,000000\r\n1247\t313935969\t1173,000000\t497,250000\t500,000000\r\n1248\t313937100\t1173,500000\t498,500000\t500,000000\r\n1249\t313938245\t1174,000000\t498,500000\t500,000000\r\n1250\t313939376\t1174,500000\t498,250000\t500,000000\r\n1251\t313940518\t1173,500000\t498,000000\t500,000000\r\n1252\t313941652\t1173,000000\t497,750000\t500,000000\r\n1253\t313942790\t1174,000000\t498,000000\t500,000000\r\n1254\t313943935\t1173,000000\t499,000000\t500,000000\r\n1255\t313945075\t1172,500000\t498,250000\t500,000000\r\n1256\t313946210\t1173,500000\t497,750000\t500,000000\r\n1257\t313947350\t1170,000000\t497,750000\t500,000000\r\n1258\t313948485\t1170,500000\t498,500000\t500,000000\r\n1259\t313949621\t1171,000000\t498,750000\t500,000000\r\n1260\t313950759\t1173,000000\t498,000000\t500,000000\r\n1261\t313951899\t1172,000000\t498,250000\t500,000000\r\n1262\t313953039\t1174,000000\t498,750000\t500,000000\r\n1263\t313954180\t1174,000000\t498,250000\t500,000000\r\n1264\t313955315\t1172,000000\t498,500000\t500,000000\r\n1265\t313956454\t1171,500000\t499,000000\t500,000000\r\n1266\t313957588\t1172,500000\t498,000000\t500,000000\r\n1267\t313958732\t1170,500000\t498,500000\t500,000000\r\n1268\t313959871\t1173,600000\t498,250000\t500,000000\r\n1269\t313961011\t1172,500000\t498,250000\t500,000000\r\n1270\t313962155\t1172,500000\t498,000000\t500,000000\r\n1271\t313963293\t1170,500000\t498,500000\t500,000000\r\n1272\t313964433\t1170,500000\t498,500000\t500,000000\r\n1273\t313965579\t1172,000000\t498,750000\t500,000000\r\n1274\t313966722\t1171,000000\t498,250000\t500,000000\r\n1275\t313967861\t1169,500000\t498,250000\t500,000000\r\n1276\t313968993\t1170,500000\t497,750000\t500,000000\r\n1277\t313970136\t1171,500000\t497,500000\t500,000000\r\n1278\t313971277\t1173,000000\t497,500000\t500,000000\r\n1279\t313972413\t1171,500000\t498,250000\t500,000000\r\n1280\t313973548\t1170,500000\t498,500000\t500,000000\r\n1281\t313974685\t1170,500000\t498,750000\t500,000000\r\n1282\t313975824\t1170,500000\t499,000000\t500,000000\r\n1283\t313976957\t1169,500000\t499,000000\t500,000000\r\n1284\t313978095\t1169,500000\t498,500000\t500,000000\r\n1285\t313979232\t1170,000000\t497,250000\t500,000000\r\n1286\t313980369\t1171,500000\t498,500000\t500,000000\r\n1287\t313981507\t1170,500000\t498,250000\t500,000000\r\n1288\t313982645\t1170,500000\t498,250000\t500,000000\r\n1289\t313983776\t1168,500000\t498,500000\t500,000000\r\n1290\t313984917\t1170,000000\t497,750000\t500,000000\r\n1291\t313986064\t1169,500000\t498,000000\t500,000000\r\n1292\t313987202\t1170,500000\t498,250000\t500,000000\r\n1293\t313988336\t1171,500000\t498,500000\t500,000000\r\n1294\t313989470\t1170,500000\t498,500000\t500,000000\r\n1295\t313990618\t1172,000000\t497,750000\t500,000000\r\n1296\t313991752\t1171,000000\t496,450000\t500,000000\r\n1297\t313992897\t1169,000000\t498,250000\t500,000000\r\n1298\t313994031\t1169,500000\t498,500000\t500,000000\r\n1299\t313995175\t1171,000000\t498,000000\t500,000000\r\n1300\t313996314\t1168,500000\t498,250000\t500,000000\r\n1301\t313997450\t1169,000000\t498,500000\t500,000000\r\n1302\t313998590\t1168,500000\t498,500000\t500,000000\r\n1303\t313999729\t1170,500000\t498,750000\t500,000000\r\n1304\t314000869\t1170,000000\t498,750000\t500,000000\r\n1305\t314002006\t1169,500000\t497,250000\t500,000000\r\n1306\t314003144\t1169,000000\t497,750000\t500,000000\r\n1307\t314004280\t1167,500000\t498,500000\t500,000000\r\n1308\t314005414\t1169,500000\t499,000000\t500,000000\r\n1309\t314006552\t1168,000000\t497,750000\t500,000000\r\n1310\t314007686\t1167,000000\t497,500000\t500,000000\r\n1311\t314008827\t1168,500000\t498,750000\t500,000000\r\n1312\t314009959\t1168,000000\t498,000000\t500,000000\r\n1313\t314011096\t1171,000000\t498,250000\t500,000000\r\n1314\t314012233\t1168,000000\t497,750000\t500,000000\r\n1315\t314013197\t1166,500000\t498,500000\t500,000000\r\n1316\t314014333\t1172,000000\t498,750000\t500,000000\r\n1317\t314015466\t1169,000000\t498,750000\t500,000000\r\n1318\t314016604\t1168,000000\t498,750000\t500,000000\r\n1319\t314017736\t1168,000000\t497,750000\t500,000000\r\n1320\t314018878\t1169,000000\t497,750000\t500,000000\r\n1321\t314020518\t1168,000000\t498,500000\t500,000000\r\n1322\t314022220\t1166,500000\t498,500000\t500,000000\r\n1323\t314023919\t1167,000000\t498,000000\t500,000000\r\n1324\t314025621\t1170,500000\t498,500000\t500,000000\r\n1325\t314026993\t1166,500000\t498,500000\t500,000000\r\n1326\t314028131\t1169,000000\t497,750000\t500,000000\r\n1327\t314029267\t1167,500000\t498,250000\t500,000000\r\n1328\t314030401\t1169,500000\t498,250000\t500,000000\r\n1329\t314031530\t1168,500000\t498,000000\t500,000000\r\n1330\t314032660\t1167,000000\t498,500000\t500,000000\r\n1331\t314033792\t1167,000000\t498,250000\t500,000000\r\n1332\t314035241\t1166,500000\t498,750000\t500,000000\r\n1333\t314036941\t1166,500000\t498,250000\t500,000000\r\n1334\t314038635\t1167,000000\t498,750000\t500,000000\r\n1335\t314040336\t1167,500000\t498,000000\t500,000000\r\n1336\t314042034\t1165,500000\t498,250000\t500,000000\r\n1337\t314043728\t1166,000000\t498,750000\t500,000000\r\n1338\t314045431\t1164,000000\t498,000000\t500,000000\r\n1339\t314047126\t1166,500000\t498,500000\t500,000000\r\n1340\t314048818\t1164,500000\t498,000000\t500,000000\r\n1341\t314050511\t1165,000000\t498,000000\t500,000000\r\n1342\t314052201\t1168,000000\t497,500000\t500,000000\r\n1343\t314053896\t1164,000000\t498,500000\t500,000000\r\n1344\t314055593\t1165,000000\t498,250000\t500,000000\r\n1345\t314057291\t1166,500000\t498,500000\t500,000000\r\n1346\t314058981\t1165,000000\t498,250000\t500,000000\r\n1347\t314060680\t1165,000000\t498,000000\t500,000000\r\n1348\t314062370\t1163,000000\t498,250000\t500,000000\r\n1349\t314064066\t1164,500000\t499,250000\t500,000000\r\n1350\t314065759\t1164,000000\t498,250000\t500,000000\r\n1351\t314067443\t1164,500000\t498,500000\t500,000000\r\n1352\t314069142\t1162,500000\t498,500000\t500,000000\r\n1353\t314070835\t1166,500000\t498,250000\t500,000000\r\n1354\t314072528\t1164,500000\t498,750000\t500,000000\r\n1355\t314074228\t1164,500000\t500,000000\t500,000000\r\n1356\t314075924\t1165,500000\t498,500000\t500,000000\r\n1357\t314077617\t1164,500000\t498,750000\t500,000000\r\n1358\t314079308\t1160,500000\t497,750000\t500,000000\r\n1359\t314080999\t1165,500000\t498,000000\t500,000000\r\n1360\t314082689\t1162,000000\t497,500000\t500,000000\r\n1361\t314084386\t1162,500000\t498,000000\t500,000000\r\n1362\t314086089\t1162,500000\t498,000000\t500,000000\r\n1363\t314087781\t1163,000000\t497,500000\t500,000000\r\n1364\t314089475\t1163,000000\t497,500000\t500,000000\r\n1365\t314091172\t1163,000000\t497,500000\t500,000000\r\n1366\t314092861\t1165,500000\t497,750000\t500,000000\r\n1367\t314094564\t1163,500000\t497,750000\t500,000000\r\n1368\t314096266\t1161,500000\t497,500000\t500,000000\r\n1369\t314097668\t1162,000000\t498,750000\t500,000000\r\n1370\t314098807\t1162,000000\t498,000000\t500,000000\r\n1371\t314099936\t1161,500000\t499,500000\t500,000000\r\n1372\t314101069\t1163,000000\t497,500000\t500,000000\r\n1373\t314102204\t1162,000000\t498,250000\t500,000000\r\n1374\t314103348\t1162,500000\t498,500000\t500,000000\r\n1375\t314104485\t1161,000000\t498,000000\t500,000000\r\n1376\t314105621\t1161,000000\t498,750000\t500,000000\r\n1377\t314106758\t1161,500000\t498,500000\t500,000000\r\n1378\t314107890\t1163,500000\t498,750000\t500,000000\r\n1379\t314109035\t1162,000000\t498,250000\t500,000000\r\n1380\t314110171\t1160,000000\t497,500000\t500,000000\r\n1381\t314111312\t1161,500000\t498,500000\t500,000000\r\n1382\t314112449\t1161,500000\t499,250000\t500,000000\r\n1383\t314113592\t1161,000000\t499,250000\t500,000000\r\n1384\t314114725\t1159,500000\t497,750000\t500,000000\r\n1385\t314115866\t1160,000000\t498,500000\t500,000000\r\n1386\t314117001\t1158,500000\t498,250000\t500,000000\r\n1387\t314118136\t1160,500000\t498,250000\t500,000000\r\n1388\t314119271\t1160,500000\t498,500000\t500,000000\r\n1389\t314120406\t1160,000000\t498,750000\t500,000000\r\n1390\t314121540\t1161,500000\t498,000000\t500,000000\r\n1391\t314122675\t1160,500000\t497,250000\t500,000000\r\n1392\t314123811\t1160,500000\t497,750000\t500,000000\r\n1393\t314124949\t1159,000000\t498,250000\t500,000000\r\n1394\t314126086\t1159,500000\t498,000000\t500,000000\r\n1395\t314127218\t1161,500000\t498,500000\t500,000000\r\n1396\t314128354\t1159,000000\t499,000000\t500,000000\r\n1397\t314129488\t1158,000000\t498,000000\t500,000000\r\n1398\t314130630\t1158,000000\t499,000000\t500,000000\r\n1399\t314131766\t1162,000000\t498,000000\t500,000000\r\n1400\t314132897\t1158,500000\t497,750000\t500,000000\r\n1401\t314134036\t1159,500000\t498,250000\t500,000000\r\n1402\t314135171\t1161,500000\t498,500000\t500,000000\r\n1403\t314136305\t1156,500000\t498,500000\t500,000000\r\n1404\t314137444\t1160,000000\t499,000000\t500,000000\r\n1405\t314138583\t1158,500000\t499,000000\t500,000000\r\n1406\t314139726\t1158,000000\t497,750000\t500,000000\r\n1407\t314140866\t1157,000000\t498,500000\t500,000000\r\n1408\t314142010\t1158,500000\t498,250000\t500,000000\r\n1409\t314143155\t1158,000000\t498,500000\t500,000000\r\n1410\t314144288\t1157,500000\t498,250000\t500,000000\r\n1411\t314145435\t1159,500000\t498,750000\t500,000000\r\n1412\t314146573\t1158,000000\t498,000000\t500,000000\r\n1413\t314147703\t1157,500000\t497,500000\t500,000000\r\n1414\t314148834\t1158,000000\t498,000000\t500,000000\r\n1415\t314149973\t1157,500000\t498,000000\t500,000000\r\n1416\t314151111\t1157,000000\t498,750000\t500,000000\r\n1417\t314152118\t1157,000000\t498,250000\t500,000000\r\n1418\t314153144\t1158,000000\t498,250000\t500,000000\r\n1419\t314154279\t1159,500000\t498,250000\t500,000000\r\n1420\t314155421\t1157,500000\t498,000000\t500,000000\r\n1421\t314156563\t1156,000000\t498,750000\t500,000000\r\n1422\t314157692\t1156,000000\t498,000000\t500,000000\r\n1423\t314158828\t1156,500000\t498,250000\t500,000000\r\n1424\t314159959\t1158,500000\t498,500000\t500,000000\r\n1425\t314161101\t1157,000000\t497,750000\t500,000000\r\n1426\t314162243\t1157,000000\t498,250000\t500,000000\r\n1427\t314163384\t1155,500000\t498,250000\t500,000000\r\n1428\t314164523\t1157,000000\t498,000000\t500,000000\r\n1429\t314165660\t1156,500000\t498,000000\t500,000000\r\n1430\t314166796\t1156,000000\t498,000000\t500,000000\r\n1431\t314167934\t1155,000000\t497,750000\t500,000000\r\n1432\t314169075\t1159,500000\t498,250000\t500,000000\r\n1433\t314170210\t1157,500000\t498,500000\t500,000000\r\n1434\t314171348\t1156,000000\t498,500000\t500,000000\r\n1435\t314172490\t1156,000000\t498,000000\t500,000000\r\n1436\t314173624\t1156,500000\t498,000000\t500,000000\r\n1437\t314174768\t1154,500000\t498,500000\t500,000000\r\n1438\t314175911\t1157,000000\t497,750000\t500,000000\r\n1439\t314177051\t1154,500000\t498,700000\t500,000000\r\n1440\t314178186\t1155,500000\t498,250000\t500,000000\r\n1441\t314179321\t1156,500000\t498,000000\t500,000000\r\n1442\t314180458\t1155,000000\t497,500000\t500,000000\r\n1443\t314181594\t1156,500000\t497,950000\t500,000000\r\n1444\t314182732\t1157,000000\t499,250000\t500,000000\r\n1445\t314183862\t1155,000000\t498,500000\t500,000000\r\n1446\t314184999\t1157,000000\t497,750000\t500,000000\r\n1447\t314186132\t1155,000000\t497,750000\t500,000000\r\n1448\t314187276\t1155,500000\t498,250000\t500,000000\r\n1449\t314188410\t1154,500000\t498,000000\t500,000000\r\n1450\t314189546\t1156,000000\t498,500000\t500,000000\r\n1451\t314190685\t1155,000000\t499,000000\t500,000000\r\n1452\t314191819\t1153,500000\t498,000000\t500,000000\r\n1453\t314192952\t1154,500000\t498,000000\t500,000000\r\n1454\t314194088\t1152,000000\t497,500000\t500,000000\r\n1455\t314195221\t1156,000000\t499,000000\t500,000000\r\n1456\t314196278\t1152,500000\t497,750000\t500,000000\r\n1457\t314197417\t1155,000000\t497,750000\t500,000000\r\n1458\t314198551\t1153,500000\t498,750000\t500,000000\r\n1459\t314199690\t1153,000000\t497,500000\t500,000000\r\n1460\t314200829\t1153,500000\t498,000000\t500,000000\r\n1461\t314201966\t1154,500000\t498,250000\t500,000000\r\n1462\t314203108\t1153,000000\t497,500000\t500,000000\r\n1464\t314205255\t1153,000000\t499,000000\t500,000000\r\n1465\t314206389\t1153,500000\t498,250000\t500,000000\r\n1466\t314207538\t1153,500000\t498,750000\t500,000000\r\n1467\t314208676\t1154,000000\t497,750000\t500,000000\r\n1468\t314209808\t1154,500000\t498,250000\t500,000000\r\n1469\t314210947\t1153,000000\t497,750000\t500,000000\r\n1470\t314212083\t1153,500000\t497,500000\t500,000000\r\n1471\t314213219\t1153,500000\t498,250000\t500,000000\r\n1472\t314214349\t1153,500000\t498,750000\t500,000000\r\n1473\t314215484\t1154,000000\t498,250000\t500,000000\r\n1474\t314216618\t1153,000000\t498,250000\t500,000000\r\n1475\t314217755\t1155,000000\t498,250000\t500,000000\r\n1476\t314218889\t1152,500000\t497,500000\t500,000000\r\n1477\t314220026\t1152,500000\t497,500000\t500,000000\r\n1478\t314221155\t1152,500000\t497,500000\t500,000000\r\n1479\t314222288\t1152,500000\t498,500000\t500,000000\r\n1480\t314223431\t1155,500000\t498,250000\t500,000000\r\n1481\t314224570\t1152,000000\t498,250000\t500,000000\r\n1482\t314225709\t1152,000000\t498,500000\t500,000000\r\n1483\t314226851\t1152,500000\t498,750000\t500,000000\r\n1484\t314227984\t1153,000000\t498,000000\t500,000000\r\n1485\t314229121\t1151,500000\t498,750000\t500,000000\r\n1486\t314230257\t1152,000000\t497,500000\t500,000000\r\n1487\t314231391\t1150,000000\t498,000000\t500,000000\r\n1488\t314232521\t1153,000000\t497,500000\t500,000000\r\n1489\t314233662\t1151,500000\t498,500000\t500,000000\r\n1490\t314234801\t1152,000000\t497,750000\t500,000000\r\n1491\t314235938\t1153,000000\t497,250000\t500,000000\r\n1492\t314237083\t1150,500000\t498,750000\t500,000000\r\n1493\t314238223\t1151,000000\t498,250000\t500,000000\r\n1494\t314239361\t1151,000000\t498,500000\t500,000000\r\n1495\t314240494\t1152,500000\t498,750000\t500,000000\r\n1496\t314241628\t1151,500000\t498,500000\t500,000000\r\n1497\t314242768\t1153,000000\t498,500000\t500,000000\r\n1498\t314243907\t1152,000000\t498,500000\t500,000000\r\n1499\t314245041\t1150,500000\t498,000000\t500,000000\r\n1500\t314246180\t1154,000000\t497,750000\t500,000000\r\n1501\t314247339\t1151,500000\t498,750000\t500,000000\r\n1502\t314248475\t1152,000000\t498,750000\t500,000000\r\n1503\t314249609\t1152,000000\t498,250000\t500,000000\r\n1504\t314250737\t1151,500000\t498,000000\t500,000000\r\n1505\t314251871\t1150,500000\t498,500000\t500,000000\r\n1506\t314253016\t1148,400000\t498,750000\t500,000000\r\n1507\t314254163\t1149,500000\t499,000000\t500,000000\r\n1508\t314255307\t1150,500000\t498,250000\t500,000000\r\n1509\t314256443\t1152,000000\t498,500000\t500,000000\r\n1510\t314257581\t1150,000000\t498,250000\t500,000000\r\n1511\t314258717\t1150,000000\t498,500000\t500,000000\r\n1512\t314259851\t1151,000000\t499,750000\t500,000000\r\n1513\t314260991\t1149,500000\t497,750000\t500,000000\r\n1514\t314262131\t1149,500000\t498,250000\t500,000000\r\n1515\t314263272\t1152,000000\t498,500000\t500,000000\r\n1516\t314264409\t1149,500000\t498,750000\t500,000000\r\n1517\t314265549\t1152,000000\t498,750000\t500,000000\r\n1518\t314266681\t1150,500000\t497,750000\t500,000000\r\n1519\t314267821\t1149,500000\t497,750000\t500,000000\r\n1520\t314268959\t1152,500000\t498,000000\t500,000000\r\n1521\t314270102\t1150,000000\t498,750000\t500,000000\r\n1522\t314271239\t1150,500000\t498,250000\t500,000000\r\n1523\t314272381\t1148,500000\t498,250000\t500,000000\r\n1524\t314273514\t1150,000000\t498,250000\t500,000000\r\n1525\t314274650\t1151,000000\t497,750000\t500,000000\r\n1526\t314275788\t1150,000000\t498,000000\t500,000000\r\n1527\t314276934\t1150,000000\t498,000000\t500,000000\r\n1528\t314278068\t1150,000000\t498,750000\t500,000000\r\n1529\t314279205\t1148,500000\t498,000000\t500,000000\r\n1530\t314280341\t1149,000000\t498,250000\t500,000000\r\n1531\t314281475\t1148,500000\t498,250000\t500,000000\r\n1532\t314282619\t1149,000000\t498,000000\t500,000000\r\n1533\t314283755\t1150,500000\t498,000000\t500,000000\r\n1534\t314284896\t1151,000000\t497,700000\t500,000000\r\n1535\t314286031\t1150,000000\t499,250000\t500,000000\r\n1536\t314287169\t1149,000000\t498,750000\t500,000000\r\n1537\t314288309\t1147,500000\t498,750000\t500,000000\r\n1538\t314289440\t1149,000000\t498,750000\t500,000000\r\n1539\t314290579\t1150,500000\t499,250000\t500,000000\r\n1540\t314291712\t1149,000000\t498,250000\t500,000000\r\n1541\t314292848\t1149,000000\t497,500000\t500,000000\r\n1542\t314293982\t1146,500000\t498,000000\t500,000000\r\n1543\t314295119\t1147,500000\t498,000000\t500,000000\r\n1544\t314296256\t1150,000000\t498,250000\t500,000000\r\n1545\t314297398\t1146,500000\t497,750000\t500,000000\r\n1546\t314298529\t1149,000000\t498,500000\t500,000000\r\n1547\t314299668\t1148,500000\t498,000000\t500,000000\r\n1548\t314300807\t1148,000000\t498,500000\t500,000000\r\n1549\t314301944\t1147,500000\t498,000000\t500,000000\r\n1550\t314303085\t1150,000000\t498,250000\t500,000000\r\n1551\t314304222\t1150,500000\t497,750000\t500,000000\r\n1552\t314305354\t1149,000000\t497,750000\t500,000000\r\n1553\t314306483\t1149,500000\t497,000000\t500,000000\r\n1554\t314307627\t1147,500000\t498,250000\t500,000000\r\n1555\t314308768\t1150,000000\t498,000000\t500,000000\r\n1556\t314309907\t1148,500000\t498,250000\t500,000000\r\n1557\t314311044\t1147,500000\t498,750000\t500,000000\r\n1558\t314312179\t1148,000000\t498,250000\t500,000000\r\n1559\t314313316\t1146,000000\t497,750000\t500,000000\r\n1560\t314314455\t1147,000000\t498,000000\t500,000000\r\n1561\t314315587\t1147,500000\t498,250000\t500,000000\r\n1562\t314316728\t1148,000000\t498,000000\t500,000000\r\n1563\t314317859\t1146,500000\t497,750000\t500,000000\r\n1564\t314318995\t1147,500000\t498,000000\t500,000000\r\n1565\t314320128\t1147,500000\t497,750000\t500,000000\r\n1566\t314321261\t1149,500000\t499,000000\t500,000000\r\n1567\t314322399\t1147,500000\t498,500000\t500,000000\r\n1568\t314323530\t1148,000000\t498,000000\t500,000000\r\n1569\t314324658\t1149,000000\t498,750000\t500,000000\r\n1570\t314325789\t1149,000000\t497,750000\t500,000000\r\n1571\t314326926\t1147,000000\t499,500000\t500,000000\r\n1572\t314328062\t1147,000000\t498,500000\t500,000000\r\n1573\t314329194\t1149,000000\t497,750000\t500,000000\r\n1574\t314330330\t1147,000000\t497,750000\t500,000000\r\n1575\t314331472\t1146,500000\t498,250000\t500,000000\r\n1576\t314332605\t1146,500000\t498,000000\t500,000000\r\n1577\t314333744\t1147,000000\t498,500000\t500,000000\r\n1578\t314334883\t1150,000000\t497,750000\t500,000000\r\n1579\t314336020\t1145,500000\t498,750000\t500,000000\r\n1580\t314337158\t1147,500000\t497,750000\t500,000000\r\n1581\t314338299\t1145,500000\t498,750000\t500,000000\r\n1582\t314339433\t1146,500000\t497,500000\t500,000000\r\n1583\t314340579\t1147,500000\t497,750000\t500,000000\r\n1584\t314341720\t1145,000000\t497,750000\t500,000000\r\n1585\t314342862\t1147,000000\t498,250000\t500,000000\r\n1586\t314343999\t1147,500000\t498,250000\t500,000000\r\n1587\t314345135\t1147,000000\t497,750000\t500,000000\r\n1588\t314346275\t1145,000000\t497,500000\t500,000000\r\n1589\t314347419\t1144,500000\t497,750000\t500,000000\r\n1590\t314348563\t1147,500000\t498,500000\t500,000000\r\n1591\t314349702\t1149,000000\t498,000000\t500,000000\r\n1592\t314350835\t1145,500000\t497,750000\t500,000000\r\n1593\t314351972\t1145,500000\t498,500000\t500,000000\r\n1594\t314353108\t1146,500000\t496,200000\t500,000000\r\n1595\t314354249\t1145,500000\t498,250000\t500,000000\r\n1596\t314355393\t1148,500000\t498,500000\t500,000000\r\n1597\t314356529\t1145,000000\t498,250000\t500,000000\r\n1598\t314357667\t1146,500000\t498,500000\t500,000000\r\n1599\t314358808\t1144,500000\t498,000000\t500,000000\r\n1600\t314359948\t1144,000000\t496,950000\t500,000000\r\n1601\t314361085\t1145,000000\t497,500000\t500,000000\r\n1602\t314362216\t1146,000000\t498,500000\t500,000000\r\n1603\t314363349\t1146,500000\t498,250000\t500,000000\r\n1604\t314364506\t1144,000000\t498,000000\t500,000000\r\n1605\t314365650\t1146,500000\t497,700000\t500,000000\r\n1606\t314366788\t1145,500000\t497,750000\t500,000000\r\n1607\t314367920\t1145,500000\t498,250000\t500,000000\r\n1608\t314369059\t1144,900000\t498,250000\t500,000000\r\n1609\t314370195\t1143,400000\t498,250000\t500,000000\r\n1610\t314371333\t1142,500000\t497,750000\t500,000000\r\n1611\t314372474\t1145,000000\t498,500000\t500,000000\r\n1612\t314373609\t1144,000000\t497,250000\t500,000000\r\n1613\t314374756\t1143,000000\t497,500000\t500,000000\r\n1614\t314375891\t1144,500000\t498,500000\t500,000000\r\n1615\t314377032\t1144,500000\t498,750000\t500,000000\r\n1616\t314378165\t1147,000000\t498,750000\t500,000000\r\n1617\t314379300\t1144,000000\t498,250000\t500,000000\r\n1618\t314380436\t1143,000000\t498,250000\t500,000000\r\n1619\t314381578\t1143,000000\t498,500000\t500,000000\r\n1620\t314382713\t1144,500000\t498,500000\t500,000000\r\n1621\t314383849\t1143,500000\t498,000000\t500,000000\r\n1622\t314384994\t1145,000000\t497,200000\t500,000000\r\n1623\t314386132\t1143,500000\t498,000000\t500,000000\r\n1624\t314387281\t1142,500000\t497,500000\t500,000000\r\n1625\t314388420\t1143,500000\t498,500000\t500,000000\r\n1626\t314389560\t1145,000000\t498,250000\t500,000000\r\n1627\t314390700\t1141,000000\t498,250000\t500,000000\r\n1628\t314391838\t1143,400000\t497,200000\t500,000000\r\n1629\t314392977\t1143,500000\t498,500000\t500,000000\r\n1630\t314394112\t1142,900000\t498,500000\t500,000000\r\n1631\t314395253\t1144,500000\t498,000000\t500,000000\r\n1632\t314396386\t1143,500000\t498,250000\t500,000000\r\n1633\t314397522\t1142,800000\t499,500000\t500,000000\r\n1634\t314398658\t1142,000000\t498,000000\t500,000000\r\n1635\t314399794\t1142,500000\t497,750000\t500,000000\r\n1636\t314400932\t1139,500000\t497,500000\t500,000000\r\n1637\t314402067\t1144,400000\t498,250000\t500,000000\r\n1638\t314403200\t1140,900000\t497,750000\t500,000000\r\n1639\t314404338\t1143,000000\t498,000000\t500,000000\r\n1640\t314405471\t1145,000000\t499,000000\t500,000000\r\n1641\t314406606\t1144,000000\t498,250000\t500,000000\r\n1642\t314407590\t1141,500000\t498,500000\t500,000000\r\n1643\t314408725\t1140,400000\t498,500000\t500,000000\r\n1644\t314409859\t1139,500000\t497,750000\t500,000000\r\n1645\t314410994\t1141,400000\t498,250000\t500,000000\r\n1646\t314412131\t1143,000000\t498,000000\t500,000000\r\n1647\t314413274\t1142,500000\t499,250000\t500,000000\r\n1648\t314414408\t1143,500000\t497,200000\t500,000000\r\n1649\t314415547\t1141,000000\t497,750000\t500,000000\r\n1650\t314416679\t1140,500000\t498,000000\t500,000000\r\n1651\t314417818\t1140,500000\t497,750000\t500,000000\r\n1652\t314418956\t1143,000000\t498,250000\t500,000000\r\n1653\t314420100\t1141,900000\t498,750000\t500,000000\r\n1654\t314421228\t1142,000000\t497,500000\t500,000000\r\n1655\t314422368\t1136,700000\t498,000000\t500,000000\r\n1656\t314423507\t1139,400000\t498,250000\t500,000000\r\n1657\t314424647\t1138,900000\t498,250000\t500,000000\r\n1658\t314425783\t1142,500000\t497,200000\t500,000000\r\n1659\t314426915\t1140,900000\t498,250000\t500,000000\r\n1660\t314428046\t1141,000000\t498,250000\t500,000000\r\n1661\t314429179\t1138,900000\t499,250000\t500,000000\r\n1662\t314430316\t1141,400000\t496,700000\t500,000000\r\n1663\t314431455\t1141,000000\t498,000000\t500,000000\r\n1664\t314432586\t1139,500000\t499,250000\t500,000000\r\n1665\t314433729\t1141,500000\t497,500000\t500,000000\r\n1666\t314434864\t1141,400000\t498,000000\t500,000000\r\n1667\t314436002\t1142,300000\t498,250000\t500,000000\r\n1668\t314437142\t1138,300000\t498,750000\t500,000000\r\n1669\t314438278\t1138,700000\t499,000000\t500,000000\r\n1670\t314439412\t1142,400000\t497,250000\t500,000000\r\n1671\t314440554\t1141,300000\t498,500000\t500,000000\r\n1672\t314441695\t1139,400000\t498,250000\t500,000000\r\n1673\t314442836\t1139,500000\t497,250000\t500,000000\r\n1674\t314443973\t1137,200000\t498,750000\t500,000000\r\n1675\t314445108\t1137,700000\t498,000000\t500,000000\r\n1676\t314446241\t1140,400000\t498,250000\t500,000000\r\n1677\t314447375\t1141,400000\t497,500000\t500,000000\r\n1678\t314448515\t1138,200000\t498,500000\t500,000000\r\n1679\t314449651\t1140,400000\t497,750000\t500,000000\r\n1680\t314450788\t1137,100000\t498,250000\t500,000000\r\n1681\t314451922\t1140,500000\t498,250000\t500,000000\r\n1682\t314453057\t1140,500000\t498,500000\t500,000000\r\n1683\t314454192\t1141,900000\t498,000000\t500,000000\r\n1684\t314455321\t1137,200000\t498,250000\t500,000000\r\n1685\t314456463\t1140,200000\t498,500000\t500,000000\r\n1686\t314457603\t1138,700000\t498,250000\t500,000000\r\n1687\t314458742\t1140,400000\t497,500000\t500,000000\r\n1688\t314459882\t1137,600000\t498,500000\t500,000000\r\n1689\t314461016\t1138,700000\t498,250000\t500,000000\r\n1690\t314462166\t1140,000000\t499,000000\t500,000000\r\n1691\t314463308\t1139,300000\t498,500000\t500,000000\r\n1692\t314464440\t1138,200000\t499,500000\t500,000000\r\n1693\t314465580\t1140,300000\t498,000000\t500,000000\r\n1694\t314466717\t1139,300000\t498,250000\t500,000000\r\n1695\t314467857\t1136,100000\t498,250000\t500,000000\r\n1696\t314468988\t1140,300000\t497,750000\t500,000000\r\n1697\t314470134\t1137,200000\t498,500000\t500,000000\r\n1698\t314471277\t1135,900000\t498,500000\t500,000000\r\n1699\t314472419\t1135,400000\t498,000000\t500,000000\r\n1700\t314473553\t1137,100000\t497,500000\t500,000000\r\n1701\t314474696\t1137,800000\t497,250000\t500,000000\r\n1702\t314475828\t1135,300000\t498,250000\t500,000000\r\n1703\t314476972\t1139,200000\t498,500000\t500,000000\r\n1704\t314478109\t1135,500000\t498,250000\t500,000000\r\n1705\t314479247\t1136,600000\t498,000000\t500,000000\r\n1706\t314480384\t1136,100000\t496,700000\t500,000000\r\n1707\t314481521\t1136,000000\t498,000000\t500,000000\r\n1708\t314482661\t1135,900000\t498,750000\t500,000000\r\n1709\t314483795\t1135,500000\t498,000000\t500,000000\r\n1710\t314484928\t1134,800000\t498,000000\t500,000000\r\n1711\t314486063\t1137,000000\t496,950000\t500,000000\r\n1712\t314487207\t1134,300000\t498,250000\t500,000000\r\n1713\t314488344\t1136,000000\t498,500000\t500,000000\r\n1714\t314489474\t1136,000000\t497,750000\t500,000000\r\n1715\t314490605\t1136,500000\t498,000000\t500,000000\r\n1716\t314491741\t1136,400000\t498,500000\t500,000000\r\n1717\t314492875\t1137,100000\t497,200000\t500,000000\r\n1718\t314494017\t1137,100000\t497,750000\t500,000000\r\n1719\t314495152\t1136,400000\t498,500000\t500,000000\r\n1720\t314496291\t1133,700000\t498,500000\t500,000000\r\n1721\t314497429\t1133,200000\t498,000000\t500,000000\r\n1722\t314498564\t1134,300000\t499,250000\t500,000000\r\n1723\t314499708\t1136,400000\t497,750000\t500,000000\r\n1724\t314500847\t1135,900000\t497,750000\t500,000000\r\n1725\t314501987\t1133,700000\t498,250000\t500,000000\r\n1726\t314503128\t1136,500000\t497,750000\t500,000000\r\n1727\t314504263\t1134,900000\t498,000000\t500,000000\r\n1728\t314505405\t1133,300000\t497,500000\t500,000000\r\n1729\t314506544\t1133,900000\t497,750000\t500,000000\r\n1730\t314507681\t1135,900000\t498,500000\t500,000000\r\n1731\t314508817\t1137,000000\t498,250000\t500,000000\r\n1732\t314509953\t1133,200000\t498,750000\t500,000000\r\n1733\t314511085\t1133,700000\t498,750000\t500,000000\r\n1734\t314512228\t1134,700000\t497,750000\t500,000000\r\n1735\t314513361\t1136,000000\t498,000000\t500,000000\r\n1736\t314514494\t1135,400000\t498,000000\t500,000000\r\n1737\t314515635\t1134,800000\t498,000000\t500,000000\r\n1738\t314516767\t1133,300000\t497,750000\t500,000000\r\n1739\t314517902\t1133,800000\t497,500000\t500,000000\r\n1740\t314519037\t1132,700000\t498,250000\t500,000000\r\n1741\t314520177\t1136,900000\t497,750000\t500,000000\r\n1742\t314521318\t1133,700000\t498,000000\t500,000000\r\n1743\t314522457\t1132,300000\t498,000000\t500,000000\r\n1744\t314523598\t1131,100000\t498,250000\t500,000000\r\n1745\t314524733\t1134,900000\t498,250000\t500,000000\r\n1746\t314525871\t1131,200000\t498,250000\t500,000000\r\n1747\t314527013\t1133,200000\t497,500000\t500,000000\r\n1748\t314528149\t1133,800000\t498,000000\t500,000000\r\n1749\t314529287\t1133,700000\t498,250000\t500,000000\r\n1750\t314530421\t1132,600000\t498,500000\t500,000000\r\n1751\t314531559\t1136,500000\t497,750000\t500,000000\r\n1752\t314532699\t1133,200000\t498,750000\t500,000000\r\n1753\t314533835\t1131,200000\t498,000000\t500,000000\r\n1754\t314534974\t1130,000000\t497,750000\t500,000000\r\n1755\t314536111\t1131,500000\t498,250000\t500,000000\r\n1756\t314537254\t1130,500000\t497,250000\t500,000000\r\n1757\t314538398\t1133,300000\t498,250000\t500,000000\r\n1758\t314539529\t1131,000000\t498,000000\t500,000000\r\n1759\t314540677\t1133,700000\t496,700000\t500,000000\r\n1760\t314541810\t1133,100000\t496,700000\t500,000000\r\n1761\t314542950\t1131,700000\t498,500000\t500,000000\r\n1762\t314544086\t1135,200000\t498,250000\t500,000000\r\n1763\t314545232\t1133,400000\t498,250000\t500,000000\r\n1764\t314546365\t1135,900000\t496,950000\t500,000000\r\n1765\t314547503\t1133,200000\t498,500000\t500,000000\r\n1766\t314548639\t1130,600000\t497,250000\t500,000000\r\n1767\t314549779\t1128,700000\t497,500000\t500,000000\r\n1768\t314550915\t1131,100000\t498,250000\t500,000000\r\n1769\t314552059\t1133,800000\t498,500000\t500,000000\r\n1770\t314553196\t1132,200000\t497,750000\t500,000000\r\n1771\t314554333\t1131,700000\t498,000000\t500,000000\r\n1772\t314555466\t1131,000000\t498,500000\t500,000000\r\n1773\t314556595\t1133,300000\t498,000000\t500,000000\r\n1774\t314557733\t1132,600000\t498,500000\t500,000000\r\n1775\t314558873\t1130,000000\t497,750000\t500,000000\r\n1776\t314560011\t1131,000000\t498,250000\t500,000000\r\n1777\t314561142\t1132,700000\t498,250000\t500,000000\r\n1778\t314562279\t1132,200000\t498,000000\t500,000000\r\n1779\t314563415\t1130,100000\t498,250000\t500,000000\r\n1780\t314564546\t1132,100000\t498,000000\t500,000000\r\n1781\t314565678\t1131,700000\t498,750000\t500,000000\r\n1782\t314566819\t1131,100000\t498,000000\t500,000000\r\n1783\t314567957\t1133,200000\t497,750000\t500,000000\r\n1784\t314569092\t1133,100000\t498,000000\t500,000000\r\n1785\t314570226\t1129,600000\t498,000000\t500,000000\r\n1786\t314571366\t1134,100000\t499,000000\t500,000000\r\n1787\t314572503\t1130,500000\t499,000000\t500,000000\r\n1788\t314573640\t1132,200000\t497,750000\t500,000000\r\n1789\t314574723\t1132,800000\t497,750000\t500,000000\r\n1790\t314575859\t1130,600000\t497,500000\t500,000000\r\n1791\t314576992\t1129,000000\t498,000000\t500,000000\r\n1792\t314578131\t1129,600000\t497,750000\t500,000000\r\n1793\t314579265\t1131,600000\t498,250000\t500,000000\r\n1794\t314580410\t1130,600000\t497,500000\t500,000000\r\n1795\t314581544\t1132,200000\t498,250000\t500,000000\r\n1796\t314582685\t1133,100000\t498,250000\t500,000000\r\n1797\t314583824\t1130,500000\t498,250000\t500,000000\r\n1798\t314584971\t1130,500000\t497,500000\t500,000000\r\n1799\t314586114\t1130,200000\t498,000000\t500,000000\r\n1800\t314587259\t1129,100000\t497,250000\t500,000000\r\n1801\t314588393\t1130,600000\t498,000000\t500,000000\r\n1802\t314589536\t1129,700000\t497,750000\t500,000000\r\n1803\t314590669\t1129,000000\t498,500000\t500,000000\r\n1804\t314591805\t1129,100000\t497,750000\t500,000000\r\n1805\t314592946\t1128,000000\t498,000000\t500,000000\r\n1806\t314594083\t1129,000000\t497,500000\t500,000000\r\n1807\t314595217\t1128,000000\t498,250000\t500,000000\r\n1808\t314596360\t1130,100000\t498,000000\t500,000000\r\n1809\t314597499\t1129,100000\t497,500000\t500,000000\r\n1810\t314598637\t1130,600000\t497,500000\t500,000000\r\n1811\t314599772\t1130,100000\t498,250000\t500,000000\r\n1812\t314600914\t1130,500000\t497,750000\t500,000000\r\n1813\t314602056\t1128,500000\t498,000000\t500,000000\r\n1814\t314603191\t1129,000000\t497,500000\t500,000000\r\n1815\t314604323\t1131,600000\t498,500000\t500,000000\r\n1816\t314605459\t1127,500000\t498,250000\t500,000000\r\n1817\t314606595\t1128,100000\t498,500000\t500,000000\r\n1818\t314607730\t1129,500000\t498,250000\t500,000000\r\n1819\t314608871\t1131,600000\t497,750000\t500,000000\r\n1820\t314609937\t1129,000000\t498,250000\t500,000000\r\n1821\t314611074\t1129,500000\t497,250000\t500,000000\r\n1822\t314612211\t1128,500000\t498,250000\t500,000000\r\n1823\t314613352\t1129,000000\t498,750000\t500,000000\r\n1824\t314614489\t1129,000000\t497,500000\t500,000000\r\n1825\t314615630\t1127,500000\t498,000000\t500,000000\r\n1827\t314617706\t1129,000000\t498,000000\t500,000000\r\n1828\t314618845\t1128,500000\t498,750000\t500,000000\r\n1829\t314619980\t1130,100000\t498,250000\t500,000000\r\n1830\t314621113\t1128,000000\t499,000000\t500,000000\r\n1831\t314622254\t1129,200000\t498,500000\t500,000000\r\n1832\t314623387\t1128,500000\t497,750000\t500,000000\r\n1833\t314624525\t1130,700000\t498,000000\t500,000000\r\n1834\t314625659\t1128,000000\t498,250000\t500,000000\r\n1835\t314626788\t1129,500000\t497,500000\t500,000000\r\n1836\t314627926\t1130,500000\t498,000000\t500,000000\r\n1837\t314629062\t1130,100000\t499,250000\t500,000000\r\n1838\t314630202\t1127,500000\t498,000000\t500,000000\r\n1839\t314631342\t1127,600000\t498,000000\t500,000000\r\n1840\t314632479\t1127,000000\t498,500000\t500,000000\r\n1841\t314633616\t1129,100000\t498,750000\t500,000000\r\n1842\t314634763\t1126,000000\t498,500000\t500,000000\r\n1844\t314637004\t1128,600000\t497,250000\t500,000000\r\n1845\t314638151\t1127,500000\t499,000000\t500,000000\r\n1846\t314639289\t1130,200000\t499,250000\t500,000000\r\n1847\t314640430\t1127,500000\t498,500000\t500,000000\r\n1848\t314641565\t1128,600000\t497,500000\t500,000000\r\n1849\t314642708\t1129,700000\t498,250000\t500,000000\r\n1850\t314643845\t1129,100000\t498,750000\t500,000000\r\n1851\t314644985\t1127,000000\t498,000000\t500,000000\r\n1852\t314646120\t1129,100000\t498,000000\t500,000000\r\n1853\t314647250\t1126,000000\t498,500000\t500,000000\r\n1854\t314648385\t1130,100000\t497,750000\t500,000000\r\n1855\t314649540\t1129,100000\t498,500000\t500,000000\r\n1856\t314650680\t1126,500000\t498,000000\t500,000000\r\n1857\t314651818\t1129,700000\t499,250000\t500,000000\r\n1858\t314652961\t1128,200000\t498,500000\t500,000000\r\n1859\t314654093\t1128,100000\t498,000000\t500,000000\r\n1860\t314655237\t1126,500000\t497,250000\t500,000000\r\n1861\t314656376\t1127,000000\t498,250000\t500,000000\r\n1862\t314657516\t1128,100000\t498,250000\t500,000000\r\n1863\t314658670\t1130,200000\t498,000000\t500,000000\r\n1864\t314659798\t1126,000000\t498,500000\t500,000000\r\n1865\t314660934\t1129,200000\t498,250000\t500,000000\r\n1866\t314662065\t1127,500000\t498,000000\t500,000000\r\n1867\t314663205\t1127,000000\t498,250000\t500,000000\r\n1868\t314664339\t1128,700000\t498,000000\t500,000000\r\n1869\t314665478\t1126,500000\t499,000000\t500,000000\r\n1870\t314666619\t1126,500000\t499,000000\t500,000000\r\n1871\t314667753\t1126,000000\t498,750000\t500,000000\r\n1872\t314668896\t1126,600000\t498,500000\t500,000000\r\n1873\t314670033\t1125,500000\t496,700000\t500,000000\r\n1874\t314671169\t1127,600000\t498,250000\t500,000000\r\n1875\t314672304\t1125,000000\t499,000000\t500,000000\r\n1876\t314673434\t1126,100000\t497,200000\t500,000000\r\n1877\t314674572\t1126,600000\t499,000000\t500,000000\r\n1878\t314675709\t1125,000000\t498,000000\t500,000000\r\n1879\t314676845\t1126,600000\t498,000000\t500,000000\r\n1880\t314677982\t1125,500000\t497,750000\t500,000000\r\n1881\t314679117\t1128,700000\t499,000000\t500,000000\r\n1882\t314680252\t1127,500000\t497,500000\t500,000000\r\n1883\t314681382\t1127,500000\t496,950000\t500,000000\r\n1884\t314682519\t1129,700000\t498,000000\t500,000000\r\n1885\t314683656\t1125,500000\t498,250000\t500,000000\r\n1886\t314684796\t1126,100000\t498,750000\t500,000000\r\n1887\t314685932\t1126,000000\t497,250000\t500,000000\r\n1888\t314687066\t1128,600000\t498,250000\t500,000000\r\n1889\t314688201\t1125,600000\t498,000000\t500,000000\r\n1890\t314689343\t1126,000000\t498,250000\t500,000000\r\n1891\t314690477\t1126,500000\t496,950000\t500,000000\r\n1892\t314691609\t1126,000000\t498,000000\t500,000000\r\n1893\t314692743\t1126,100000\t497,750000\t500,000000\r\n1894\t314693882\t1128,100000\t498,000000\t500,000000\r\n1895\t314695017\t1126,500000\t497,750000\t500,000000\r\n1896\t314696147\t1125,000000\t498,500000\t500,000000\r\n1897\t314697428\t1123,500000\t498,000000\t500,000000\r\n1898\t314698951\t1123,000000\t498,500000\t500,000000\r\n1899\t314700637\t1124,600000\t497,750000\t500,000000\r\n1900\t314702334\t1124,000000\t498,000000\t500,000000\r\n1901\t314704041\t1129,100000\t498,500000\t500,000000\r\n1902\t314705744\t1124,100000\t498,500000\t500,000000\r\n1903\t314707443\t1123,000000\t498,500000\t500,000000\r\n1904\t314709138\t1124,000000\t498,250000\t500,000000\r\n1905\t314710638\t1123,500000\t498,250000\t500,000000\r\n1906\t314711776\t1125,000000\t497,500000\t500,000000\r\n1907\t314712911\t1124,600000\t498,250000\t500,000000\r\n1908\t314714052\t1124,500000\t498,500000\t500,000000\r\n1909\t314715192\t1126,000000\t497,500000\t500,000000\r\n1910\t314716606\t1122,000000\t497,750000\t500,000000\r\n1911\t314718300\t1123,500000\t498,250000\t500,000000\r\n1912\t314719996\t1123,500000\t498,250000\t500,000000\r\n1913\t314721437\t1124,500000\t498,000000\t500,000000\r\n1914\t314722584\t1124,000000\t497,500000\t500,000000\r\n1915\t314723718\t1123,000000\t498,500000\t500,000000\r\n1916\t314724859\t1122,100000\t498,250000\t500,000000\r\n1917\t314725998\t1123,500000\t498,000000\t500,000000\r\n1918\t314727135\t1123,500000\t497,500000\t500,000000\r\n1919\t314728269\t1123,000000\t498,750000\t500,000000\r\n1920\t314729409\t1121,000000\t498,250000\t500,000000\r\n1921\t314730543\t1122,500000\t498,500000\t500,000000\r\n1922\t314731686\t1122,000000\t497,500000\t500,000000\r\n1923\t314732832\t1124,100000\t498,250000\t500,000000\r\n1924\t314733965\t1121,500000\t498,000000\t500,000000\r\n1925\t314735106\t1121,500000\t498,500000\t500,000000\r\n1926\t314736241\t1122,500000\t499,250000\t500,000000\r\n1927\t314737382\t1124,100000\t498,250000\t500,000000\r\n1928\t314738531\t1124,000000\t498,750000\t500,000000\r\n1929\t314739666\t1123,500000\t498,500000\t500,000000\r\n1930\t314740803\t1122,000000\t498,000000\t500,000000\r\n1931\t314741946\t1119,000000\t498,750000\t500,000000\r\n1932\t314743084\t1122,500000\t498,750000\t500,000000\r\n1933\t314744220\t1123,000000\t498,250000\t500,000000\r\n1934\t314745359\t1122,100000\t499,000000\t500,000000\r\n1935\t314746505\t1122,500000\t498,000000\t500,000000\r\n1936\t314747639\t1120,500000\t497,500000\t500,000000\r\n1937\t314748781\t1119,500000\t498,500000\t500,000000\r\n1938\t314749916\t1121,500000\t499,000000\t500,000000\r\n1939\t314751055\t1120,500000\t497,750000\t500,000000\r\n1940\t314752189\t1121,500000\t498,000000\t500,000000\r\n1941\t314753320\t1120,000000\t498,000000\t500,000000\r\n1942\t314754464\t1122,600000\t498,250000\t500,000000\r\n1943\t314755611\t1120,000000\t498,000000\t500,000000\r\n1944\t314756749\t1121,500000\t498,750000\t500,000000\r\n1945\t314757889\t1122,500000\t498,250000\t500,000000\r\n1946\t314759029\t1121,000000\t498,250000\t500,000000\r\n1947\t314760171\t1122,000000\t497,750000\t500,000000\r\n1948\t314761310\t1122,000000\t497,750000\t500,000000\r\n1949\t314762450\t1120,000000\t498,000000\t500,000000\r\n1950\t314763596\t1121,500000\t498,000000\t500,000000\r\n1951\t314764734\t1119,500000\t498,250000\t500,000000\r\n1952\t314765878\t1121,500000\t498,250000\t500,000000\r\n1953\t314767016\t1120,500000\t498,750000\t500,000000\r\n1954\t314768148\t1120,500000\t498,000000\t500,000000\r\n1955\t314769289\t1121,000000\t499,000000\t500,000000\r\n1956\t314770425\t1122,600000\t498,500000\t500,000000\r\n1957\t314771560\t1120,500000\t498,750000\t500,000000\r\n1958\t314772695\t1123,000000\t498,500000\t500,000000\r\n1959\t314773830\t1121,000000\t498,750000\t500,000000\r\n1960\t314774962\t1122,000000\t498,000000\t500,000000\r\n1961\t314776096\t1119,500000\t497,750000\t500,000000\r\n1962\t314777234\t1119,600000\t498,500000\t500,000000\r\n1963\t314778376\t1121,000000\t498,000000\t500,000000\r\n1964\t314779513\t1118,500000\t498,250000\t500,000000\r\n1965\t314780650\t1120,000000\t498,000000\t500,000000\r\n1966\t314781782\t1120,000000\t498,750000\t500,000000\r\n1967\t314782920\t1119,000000\t498,250000\t500,000000\r\n1968\t314784058\t1120,000000\t498,500000\t500,000000\r\n1969\t314785192\t1118,000000\t498,250000\t500,000000\r\n1970\t314786333\t1120,500000\t497,500000\t500,000000\r\n1971\t314787470\t1119,000000\t498,000000\t500,000000\r\n1972\t314788602\t1119,500000\t498,250000\t500,000000\r\n1973\t314789740\t1117,500000\t498,750000\t500,000000\r\n1974\t314790879\t1116,500000\t498,000000\t500,000000\r\n1975\t314792019\t1117,500000\t498,250000\t500,000000\r\n1976\t314793156\t1118,500000\t497,750000\t500,000000\r\n1977\t314794297\t1117,500000\t497,750000\t500,000000\r\n1978\t314795437\t1119,000000\t497,500000\t500,000000\r\n1979\t314796574\t1118,500000\t497,750000\t500,000000\r\n1980\t314797715\t1117,500000\t497,750000\t500,000000\r\n1981\t314798847\t1120,000000\t498,750000\t500,000000\r\n1982\t314799987\t1119,000000\t498,250000\t500,000000\r\n1983\t314801124\t1118,500000\t497,750000\t500,000000\r\n1984\t314802265\t1118,500000\t498,000000\t500,000000\r\n1985\t314803405\t1119,600000\t498,000000\t500,000000\r\n1986\t314804539\t1117,500000\t498,250000\t500,000000\r\n1987\t314805671\t1118,500000\t497,500000\t500,000000\r\n1988\t314806811\t1116,000000\t498,000000\t500,000000\r\n1989\t314807946\t1116,500000\t498,000000\t500,000000\r\n1990\t314809086\t1118,500000\t497,200000\t500,000000\r\n1991\t314810226\t1119,000000\t498,250000\t500,000000\r\n1992\t314811370\t1116,500000\t498,250000\t500,000000\r\n1993\t314812503\t1118,000000\t498,000000\t500,000000\r\n1994\t314813637\t1118,000000\t498,250000\t500,000000\r\n1995\t314814771\t1117,500000\t498,250000\t500,000000\r\n1996\t314815906\t1117,500000\t498,000000\t500,000000\r\n1997\t314817040\t1117,500000\t498,250000\t500,000000\r\n1998\t314818181\t1117,000000\t498,500000\t500,000000\r\n1999\t314819324\t1117,500000\t498,250000\t500,000000\r\n2000\t314820458\t1118,500000\t498,000000\t500,000000\r\n2001\t314821596\t1118,500000\t498,500000\t500,000000\r\n2002\t314822735\t1116,500000\t498,500000\t500,000000\r\n2003\t314823879\t1116,500000\t498,000000\t500,000000\r\n2004\t314825017\t1115,500000\t497,750000\t500,000000\r\n2005\t314826158\t1116,000000\t498,000000\t500,000000\r\n2006\t314827292\t1115,000000\t498,750000\t500,000000\r\n2007\t314828431\t1116,500000\t498,000000\t500,000000\r\n2008\t314829566\t1115,500000\t498,750000\t500,000000\r\n2009\t314830709\t1116,000000\t498,000000\t500,000000\r\n2010\t314831852\t1116,000000\t497,500000\t500,000000\r\n2011\t314832995\t1116,000000\t498,250000\t500,000000\r\n2012\t314834137\t1117,500000\t498,250000\t500,000000\r\n2013\t314835274\t1116,000000\t498,750000\t500,000000\r\n2014\t314836415\t1114,000000\t498,250000\t500,000000\r\n2015\t314837552\t1115,500000\t498,500000\t500,000000\r\n2016\t314838698\t1115,000000\t498,500000\t500,000000\r\n2017\t314839839\t1115,500000\t498,750000\t500,000000\r\n2018\t314840973\t1116,000000\t498,250000\t500,000000\r\n2019\t314842112\t1114,500000\t498,500000\t500,000000\r\n2020\t314843244\t1114,500000\t498,750000\t500,000000\r\n2021\t314844387\t1114,000000\t498,000000\t500,000000\r\n2022\t314845526\t1114,500000\t498,000000\t500,000000\r\n2023\t314846665\t1115,000000\t499,250000\t500,000000\r\n2024\t314847798\t1117,000000\t499,000000\t500,000000\r\n2025\t314848933\t1116,500000\t498,750000\t500,000000\r\n2026\t314850075\t1117,000000\t496,500000\t500,000000\r\n2027\t314851213\t1114,500000\t499,000000\t500,000000\r\n2028\t314852350\t1113,500000\t498,000000\t500,000000\r\n2029\t314853487\t1116,000000\t498,250000\t500,000000\r\n2030\t314854623\t1115,000000\t498,500000\t500,000000\r\n2031\t314855763\t1115,000000\t498,500000\t500,000000\r\n2032\t314856908\t1115,000000\t497,750000\t500,000000\r\n2033\t314858044\t1116,500000\t498,750000\t500,000000\r\n2034\t314859185\t1113,500000\t498,000000\t500,000000\r\n2035\t314860326\t1112,500000\t497,250000\t500,000000\r\n2036\t314861465\t1115,500000\t498,250000\t500,000000\r\n2037\t314862604\t1115,500000\t498,000000\t500,000000\r\n2038\t314863738\t1113,500000\t498,250000\t500,000000\r\n2039\t314864881\t1116,000000\t499,000000\t500,000000\r\n2040\t314866020\t1115,000000\t498,000000\t500,000000\r\n2041\t314867160\t1116,500000\t498,000000\t500,000000\r\n2042\t314868295\t1114,500000\t498,000000\t500,000000\r\n2043\t314869434\t1113,500000\t497,750000\t500,000000\r\n2044\t314870577\t1113,000000\t497,750000\t500,000000\r\n2045\t314871712\t1113,000000\t497,500000\t500,000000\r\n2046\t314872843\t1113,500000\t498,250000\t500,000000\r\n2047\t314873984\t1113,000000\t497,500000\t500,000000\r\n2048\t314875123\t1113,000000\t497,750000\t500,000000\r\n2049\t314876256\t1112,500000\t498,000000\t500,000000\r\n2050\t314877388\t1112,500000\t498,500000\t500,000000\r\n2051\t314878515\t1114,000000\t498,750000\t500,000000\r\n2052\t314879650\t1114,000000\t497,750000\t500,000000\r\n2053\t314880788\t1112,000000\t498,500000\t500,000000\r\n2054\t314881924\t1115,000000\t497,750000\t500,000000\r\n2055\t314883061\t1112,500000\t498,000000\t500,000000\r\n2056\t314884197\t1113,000000\t498,500000\t500,000000\r\n2057\t314885334\t1112,500000\t498,500000\t500,000000\r\n2058\t314886468\t1113,000000\t498,250000\t500,000000\r\n2059\t314887609\t1111,500000\t497,500000\t500,000000\r\n2060\t314888750\t1112,500000\t497,250000\t500,000000\r\n2061\t314889892\t1113,000000\t497,500000\t500,000000\r\n2062\t314891032\t1113,000000\t499,000000\t500,000000\r\n2063\t314892172\t1112,500000\t498,250000\t500,000000\r\n2064\t314893323\t1112,000000\t498,250000\t500,000000\r\n2065\t314894462\t1112,500000\t498,750000\t500,000000\r\n2066\t314895604\t1113,000000\t498,500000\t500,000000\r\n2067\t314896750\t1112,500000\t495,700000\t500,000000\r\n2068\t314897887\t1110,500000\t497,750000\t500,000000\r\n2069\t314899024\t1109,500000\t498,000000\t500,000000\r\n2070\t314900159\t1113,000000\t498,750000\t500,000000\r\n2071\t314901293\t1113,000000\t498,500000\t500,000000\r\n2072\t314902433\t1111,000000\t498,250000\t500,000000\r\n2073\t314903570\t1112,500000\t498,500000\t500,000000\r\n2074\t314904704\t1109,500000\t498,000000\t500,000000\r\n2075\t314905843\t1113,000000\t497,750000\t500,000000\r\n2076\t314906981\t1112,500000\t498,000000\t500,000000\r\n2077\t314908119\t1110,500000\t498,250000\t500,000000\r\n2078\t314909258\t1112,500000\t498,250000\t500,000000\r\n2079\t314910401\t1111,500000\t499,000000\t500,000000\r\n2080\t314911541\t1109,500000\t498,500000\t500,000000\r\n2081\t314912679\t1113,500000\t498,500000\t500,000000\r\n2082\t314913821\t1113,000000\t497,750000\t500,000000\r\n2083\t314914960\t1111,000000\t497,500000\t500,000000\r\n2084\t314916094\t1110,000000\t498,000000\t500,000000\r\n2085\t314917228\t1112,500000\t498,250000\t500,000000\r\n2086\t314918361\t1111,500000\t498,000000\t500,000000\r\n2087\t314919494\t1110,500000\t498,750000\t500,000000\r\n2088\t314920625\t1111,500000\t498,250000\t500,000000\r\n2089\t314921758\t1111,000000\t497,500000\t500,000000\r\n2090\t314922894\t1109,500000\t498,750000\t500,000000\r\n2091\t314924036\t1110,500000\t497,500000\t500,000000\r\n2092\t314925177\t1110,000000\t498,250000\t500,000000\r\n2093\t314926305\t1109,500000\t498,500000\t500,000000\r\n2094\t314927446\t1112,000000\t498,000000\t500,000000\r\n2095\t314928587\t1110,500000\t498,000000\t500,000000\r\n2096\t314929728\t1112,500000\t498,250000\t500,000000\r\n2097\t314930865\t1111,500000\t498,750000\t500,000000\r\n2098\t314931999\t1112,500000\t498,000000\t500,000000\r\n2099\t314933146\t1110,500000\t497,750000\t500,000000\r\n2100\t314934285\t1111,500000\t498,250000\t500,000000\r\n2101\t314935417\t1110,500000\t498,250000\t500,000000\r\n2102\t314936554\t1111,000000\t497,500000\t500,000000\r\n2103\t314937691\t1111,000000\t498,750000\t500,000000\r\n2104\t314938823\t1107,500000\t498,250000\t500,000000\r\n2105\t314939957\t1112,000000\t497,500000\t500,000000\r\n2106\t314941098\t1109,500000\t497,750000\t500,000000\r\n2107\t314942244\t1109,000000\t498,750000\t500,000000\r\n2108\t314943387\t1109,000000\t498,750000\t500,000000\r\n2109\t314944518\t1109,500000\t497,750000\t500,000000\r\n2110\t314945658\t1109,500000\t498,000000\t500,000000\r\n2111\t314946796\t1106,500000\t498,500000\t500,000000\r\n2112\t314947929\t1110,500000\t498,250000\t500,000000\r\n2113\t314949066\t1109,500000\t499,000000\t500,000000\r\n2114\t314950205\t1109,500000\t498,000000\t500,000000\r\n2115\t314951339\t1109,000000\t497,750000\t500,000000\r\n2116\t314952478\t1110,000000\t497,750000\t500,000000\r\n2117\t314953617\t1109,000000\t498,000000\t500,000000\r\n2118\t314954756\t1110,000000\t498,500000\t500,000000\r\n2119\t314955897\t1110,000000\t499,500000\t500,000000\r\n2120\t314957037\t1107,000000\t498,750000\t500,000000\r\n2121\t314958177\t1108,000000\t499,250000\t500,000000\r\n2122\t314959319\t1108,500000\t498,000000\t500,000000\r\n2123\t314960457\t1108,500000\t498,250000\t500,000000\r\n2124\t314961600\t1110,000000\t498,500000\t500,000000\r\n2125\t314962740\t1107,500000\t497,250000\t500,000000\r\n2126\t314963880\t1107,500000\t498,000000\t500,000000\r\n2127\t314965020\t1109,500000\t498,750000\t500,000000\r\n2128\t314966157\t1109,500000\t498,000000\t500,000000\r\n2129\t314967301\t1110,500000\t499,000000\t500,000000\r\n2130\t314968445\t1109,000000\t498,250000\t500,000000\r\n2131\t314969585\t1110,000000\t498,500000\t500,000000\r\n2132\t314970720\t1109,000000\t498,250000\t500,000000\r\n2133\t314971858\t1109,500000\t498,250000\t500,000000\r\n2134\t314972997\t1110,000000\t498,500000\t500,000000\r\n2135\t314974132\t1108,000000\t498,000000\t500,000000\r\n2136\t314975268\t1107,500000\t497,750000\t500,000000\r\n2137\t314976402\t1106,500000\t499,000000\t500,000000\r\n2138\t314977542\t1110,500000\t498,500000\t500,000000\r\n2139\t314978683\t1108,500000\t498,250000\t500,000000\r\n2140\t314979817\t1108,500000\t498,500000\t500,000000\r\n2141\t314980951\t1106,000000\t497,750000\t500,000000\r\n2142\t314982097\t1108,000000\t498,500000\t500,000000\r\n2143\t314983241\t1108,500000\t498,750000\t500,000000\r\n2144\t314984384\t1109,000000\t497,250000\t500,000000\r\n2145\t314985530\t1111,500000\t498,000000\t500,000000\r\n2146\t314986674\t1108,500000\t497,750000\t500,000000\r\n2147\t314987826\t1107,500000\t497,250000\t500,000000\r\n2148\t314988963\t1109,000000\t499,750000\t500,000000\r\n2149\t314990099\t1108,500000\t498,750000\t500,000000\r\n2150\t314991238\t1107,500000\t498,000000\t500,000000\r\n2151\t314992368\t1106,500000\t497,750000\t500,000000\r\n2152\t314993507\t1108,000000\t499,000000\t500,000000\r\n2153\t314994650\t1108,500000\t498,000000\t500,000000\r\n2154\t314995789\t1105,500000\t499,000000\t500,000000\r\n2155\t314996925\t1109,000000\t498,250000\t500,000000\r\n2156\t314998054\t1106,500000\t498,000000\t500,000000\r\n2157\t314999195\t1106,500000\t498,250000\t500,000000\r\n2158\t315000331\t1106,500000\t498,000000\t500,000000\r\n2159\t315001471\t1106,500000\t498,250000\t500,000000\r\n2160\t315002610\t1107,000000\t498,250000\t500,000000\r\n2161\t315003749\t1106,500000\t498,500000\t500,000000\r\n2162\t315004889\t1107,000000\t498,500000\t500,000000\r\n2163\t315006033\t1106,500000\t498,000000\t500,000000\r\n2164\t315007171\t1104,500000\t498,750000\t500,000000\r\n2165\t315008310\t1108,000000\t498,000000\t500,000000\r\n2166\t315009449\t1105,000000\t496,700000\t500,000000\r\n2167\t315010589\t1107,500000\t498,250000\t500,000000\r\n2168\t315011725\t1105,000000\t498,000000\t500,000000\r\n2169\t315012862\t1106,500000\t497,750000\t500,000000\r\n2170\t315013999\t1106,500000\t498,250000\t500,000000\r\n2171\t315015143\t1106,500000\t497,750000\t500,000000\r\n2172\t315016277\t1108,500000\t498,750000\t500,000000\r\n2173\t315017414\t1108,000000\t498,000000\t500,000000\r\n2174\t315018552\t1104,500000\t497,500000\t500,000000\r\n2175\t315019688\t1105,500000\t496,700000\t500,000000\r\n2176\t315020825\t1104,500000\t498,500000\t500,000000\r\n2177\t315021966\t1105,500000\t498,000000\t500,000000\r\n2178\t315023105\t1106,500000\t498,000000\t500,000000\r\n2179\t315024240\t1105,000000\t498,750000\t500,000000\r\n2180\t315025378\t1106,000000\t498,250000\t500,000000\r\n2181\t315026514\t1107,500000\t497,450000\t500,000000\r\n2182\t315027651\t1107,500000\t498,250000\t500,000000\r\n2183\t315028793\t1107,000000\t498,250000\t500,000000\r\n2184\t315029925\t1104,500000\t497,250000\t500,000000\r\n2185\t315031062\t1106,000000\t498,250000\t500,000000\r\n2186\t315032197\t1104,000000\t497,750000\t500,000000\r\n2187\t315033334\t1103,500000\t497,500000\t500,000000\r\n2188\t315034468\t1107,000000\t498,250000\t500,000000\r\n2189\t315035603\t1105,000000\t497,500000\t500,000000\r\n2190\t315036742\t1105,000000\t498,500000\t500,000000\r\n2191\t315037879\t1105,500000\t498,000000\t500,000000\r\n2192\t315039015\t1104,500000\t498,500000\t500,000000\r\n2193\t315040155\t1106,000000\t498,250000\t500,000000\r\n2194\t315041286\t1104,000000\t499,000000\t500,000000\r\n2195\t315042426\t1104,000000\t498,000000\t500,000000\r\n2196\t315043567\t1104,500000\t498,500000\t500,000000\r\n2197\t315044702\t1106,000000\t498,500000\t500,000000\r\n2198\t315045843\t1103,000000\t498,500000\t500,000000\r\n2199\t315046978\t1104,000000\t498,250000\t500,000000\r\n2200\t315048112\t1105,000000\t498,500000\t500,000000\r\n2201\t315049251\t1100,900000\t498,500000\t500,000000\r\n2202\t315050392\t1103,500000\t499,000000\t500,000000\r\n2203\t315051535\t1104,500000\t498,000000\t500,000000\r\n2204\t315052671\t1103,500000\t497,750000\t500,000000\r\n2205\t315053812\t1102,500000\t498,250000\t500,000000\r\n2206\t315054946\t1104,000000\t497,750000\t500,000000\r\n2207\t315056085\t1105,500000\t498,250000\t500,000000\r\n2208\t315057222\t1103,500000\t498,000000\t500,000000\r\n2209\t315058364\t1104,500000\t498,750000\t500,000000\r\n2210\t315059504\t1103,500000\t499,000000\t500,000000\r\n2211\t315060641\t1104,500000\t499,000000\t500,000000\r\n2212\t315061777\t1103,000000\t498,250000\t500,000000\r\n2213\t315062911\t1103,000000\t497,750000\t500,000000\r\n2214\t315064042\t1103,500000\t497,750000\t500,000000\r\n2215\t315065178\t1102,500000\t496,950000\t500,000000\r\n2216\t315066324\t1103,500000\t498,250000\t500,000000\r\n2217\t315067457\t1102,500000\t499,250000\t500,000000\r\n2218\t315068599\t1103,000000\t498,500000\t500,000000\r\n2219\t315069738\t1102,000000\t497,750000\t500,000000\r\n2220\t315070872\t1103,500000\t497,750000\t500,000000\r\n2221\t315072011\t1103,500000\t498,500000\t500,000000\r\n2222\t315073152\t1101,000000\t498,000000\t500,000000\r\n2223\t315074289\t1102,000000\t499,250000\t500,000000\r\n2224\t315075425\t1102,500000\t498,250000\t500,000000\r\n2225\t315076564\t1102,000000\t498,000000\t500,000000\r\n2226\t315077701\t1101,500000\t498,000000\t500,000000\r\n2227\t315078838\t1103,500000\t498,500000\t500,000000\r\n2228\t315079978\t1104,500000\t498,750000\t500,000000\r\n2229\t315081112\t1103,500000\t497,750000\t500,000000\r\n2230\t315082251\t1100,000000\t498,750000\t500,000000\r\n2231\t315083388\t1101,000000\t498,000000\t500,000000\r\n2233\t315085630\t1102,500000\t498,250000\t500,000000\r\n2234\t315086768\t1101,000000\t498,000000\t500,000000\r\n2235\t315087905\t1102,500000\t498,250000\t500,000000\r\n2236\t315089039\t1101,500000\t498,500000\t500,000000\r\n2237\t315090176\t1101,000000\t497,750000\t500,000000\r\n2238\t315091317\t1101,000000\t498,500000\t500,000000\r\n2239\t315092457\t1103,000000\t498,500000\t500,000000\r\n2240\t315093600\t1100,500000\t498,750000\t500,000000\r\n2241\t315094742\t1101,000000\t497,750000\t500,000000\r\n2242\t315095879\t1101,500000\t499,250000\t500,000000\r\n2243\t315097008\t1099,500000\t498,250000\t500,000000\r\n2244\t315098146\t1101,000000\t497,250000\t500,000000\r\n2245\t315099280\t1099,500000\t498,250000\t500,000000\r\n2246\t315100426\t1101,000000\t498,250000\t500,000000\r\n2247\t315101564\t1102,000000\t498,750000\t500,000000\r\n2248\t315102704\t1101,000000\t499,000000\t500,000000\r\n2249\t315103841\t1101,500000\t498,000000\t500,000000\r\n2250\t315104982\t1101,500000\t498,750000\t500,000000\r\n2251\t315106116\t1102,000000\t498,250000\t500,000000\r\n2252\t315107258\t1102,000000\t497,250000\t500,000000\r\n2253\t315108394\t1100,000000\t498,250000\t500,000000\r\n2254\t315109533\t1101,500000\t497,500000\t500,000000\r\n2255\t315110671\t1099,000000\t498,000000\t500,000000\r\n2256\t315111814\t1100,000000\t498,500000\t500,000000\r\n2257\t315112954\t1100,500000\t497,750000\t500,000000\r\n2258\t315114092\t1099,000000\t498,750000\t500,000000\r\n2259\t315115232\t1100,000000\t497,750000\t500,000000\r\n2260\t315116369\t1100,000000\t498,000000\t500,000000\r\n2261\t315117509\t1100,000000\t499,250000\t500,000000\r\n2262\t315118642\t1100,500000\t498,500000\t500,000000\r\n2263\t315119775\t1099,000000\t498,500000\t500,000000\r\n2264\t315120919\t1099,000000\t498,250000\t500,000000\r\n2265\t315122054\t1099,500000\t498,000000\t500,000000\r\n2266\t315123194\t1099,500000\t498,500000\t500,000000\r\n2267\t315124334\t1099,500000\t498,000000\t500,000000\r\n2268\t315125472\t1101,500000\t497,250000\t500,000000\r\n2269\t315126613\t1102,000000\t498,250000\t500,000000\r\n2270\t315127752\t1097,400000\t497,500000\t500,000000\r\n2271\t315128890\t1100,500000\t498,250000\t500,000000\r\n2272\t315130030\t1099,000000\t499,000000\t500,000000\r\n2273\t315131171\t1099,000000\t498,250000\t500,000000\r\n2274\t315132304\t1100,000000\t498,250000\t500,000000\r\n2275\t315133441\t1097,000000\t498,750000\t500,000000\r\n2276\t315134577\t1100,500000\t497,500000\t500,000000\r\n2277\t315135712\t1097,500000\t498,750000\t500,000000\r\n2278\t315136849\t1096,900000\t497,500000\t500,000000\r\n2279\t315137994\t1099,500000\t498,500000\t500,000000\r\n2280\t315139131\t1098,500000\t498,250000\t500,000000\r\n2281\t315140274\t1098,000000\t497,750000\t500,000000\r\n2282\t315141410\t1100,000000\t497,500000\t500,000000\r\n2283\t315142548\t1096,400000\t499,000000\t500,000000\r\n2284\t315143683\t1094,900000\t498,250000\t500,000000\r\n2285\t315144831\t1099,500000\t498,250000\t500,000000\r\n2286\t315145967\t1097,500000\t498,500000\t500,000000\r\n2287\t315147107\t1098,000000\t498,000000\t500,000000\r\n2288\t315148234\t1099,000000\t498,000000\t500,000000\r\n2289\t315149374\t1099,000000\t497,750000\t500,000000\r\n2290\t315150513\t1097,000000\t497,750000\t500,000000\r\n2291\t315151651\t1097,500000\t497,750000\t500,000000\r\n2292\t315152791\t1099,000000\t498,250000\t500,000000\r\n2293\t315153929\t1097,500000\t497,750000\t500,000000\r\n2294\t315155069\t1096,500000\t498,500000\t500,000000\r\n2295\t315156215\t1096,000000\t498,750000\t500,000000\r\n2296\t315157358\t1098,500000\t498,250000\t500,000000\r\n2297\t315158498\t1097,000000\t498,000000\t500,000000\r\n2298\t315159638\t1098,500000\t498,250000\t500,000000\r\n2299\t315160778\t1101,000000\t498,000000\t500,000000\r\n2300\t315161919\t1097,000000\t498,500000\t500,000000\r\n2301\t315163058\t1098,000000\t498,250000\t500,000000\r\n2302\t315164196\t1095,000000\t497,250000\t500,000000\r\n2303\t315165330\t1098,000000\t499,000000\t500,000000\r\n2304\t315166459\t1100,000000\t498,750000\t500,000000\r\n2305\t315167597\t1098,000000\t498,250000\t500,000000\r\n2306\t315168730\t1095,900000\t498,000000\t500,000000\r\n2307\t315170263\t1099,000000\t498,250000\t500,000000\r\n2308\t315171958\t1098,000000\t497,000000\t500,000000\r\n2309\t315173655\t1097,000000\t498,500000\t500,000000\r\n2310\t315175356\t1097,500000\t497,750000\t500,000000\r\n2311\t315177034\t1097,500000\t497,750000\t500,000000\r\n2312\t315178726\t1097,000000\t498,750000\t500,000000\r\n2313\t315180424\t1095,000000\t499,500000\t500,000000\r\n2314\t315182126\t1096,000000\t498,750000\t500,000000\r\n2315\t315183827\t1095,500000\t498,250000\t500,000000\r\n2316\t315185527\t1096,000000\t497,750000\t500,000000\r\n2317\t315187220\t1095,500000\t497,500000\t500,000000\r\n2318\t315188911\t1097,500000\t498,500000\t500,000000\r\n2319\t315190608\t1096,000000\t498,750000\t500,000000\r\n2320\t315192296\t1095,500000\t498,250000\t500,000000\r\n2321\t315193998\t1095,000000\t498,250000\t500,000000\r\n2322\t315195694\t1093,500000\t498,250000\t500,000000\r\n2323\t315197393\t1094,500000\t498,000000\t500,000000\r\n2324\t315199081\t1096,500000\t498,500000\t500,000000\r\n2325\t315200785\t1093,000000\t497,500000\t500,000000\r\n2326\t315202477\t1095,000000\t498,250000\t500,000000\r\n2327\t315204174\t1094,000000\t497,750000\t500,000000\r\n2328\t315205877\t1096,500000\t498,500000\t500,000000\r\n2329\t315207577\t1095,000000\t498,500000\t500,000000\r\n2330\t315209258\t1094,000000\t498,250000\t500,000000\r\n2331\t315210941\t1095,500000\t497,750000\t500,000000\r\n2332\t315212644\t1094,500000\t498,250000\t500,000000\r\n2333\t315214340\t1094,000000\t498,750000\t500,000000\r\n2334\t315216016\t1098,000000\t498,250000\t500,000000\r\n2335\t315217713\t1096,000000\t497,250000\t500,000000\r\n2336\t315219392\t1089,400000\t496,200000\t500,000000\r\n2337\t315221070\t1094,500000\t498,500000\t500,000000\r\n2338\t315222770\t1094,000000\t498,000000\t500,000000\r\n2339\t315224464\t1092,000000\t498,250000\t500,000000\r\n2340\t315226165\t1091,500000\t497,250000\t500,000000\r\n2341\t315227869\t1093,000000\t498,250000\t500,000000\r\n2342\t315229558\t1094,000000\t498,250000\t500,000000\r\n2343\t315231254\t1095,500000\t498,750000\t500,000000\r\n2344\t315232954\t1093,500000\t498,000000\t500,000000\r\n2345\t315234646\t1093,500000\t498,250000\t500,000000\r\n2346\t315236351\t1094,000000\t497,750000\t500,000000\r\n2347\t315238044\t1093,500000\t498,750000\t500,000000\r\n2348\t315239743\t1094,500000\t498,750000\t500,000000\r\n2349\t315241447\t1092,500000\t498,500000\t500,000000\r\n2350\t315243139\t1094,000000\t497,500000\t500,000000\r\n2351\t315244850\t1094,500000\t498,500000\t500,000000\r\n2352\t315246561\t1094,500000\t498,250000\t500,000000\r\n2353\t315248265\t1093,000000\t498,500000\t500,000000\r\n2354\t315249977\t1094,500000\t498,250000\t500,000000\r\n2355\t315251679\t1091,900000\t498,750000\t500,000000\r\n2356\t315253384\t1093,000000\t498,500000\t500,000000\r\n2357\t315255088\t1093,000000\t498,250000\t500,000000\r\n2358\t315256789\t1092,000000\t498,500000\t500,000000\r\n2359\t315258492\t1092,500000\t498,500000\t500,000000\r\n2360\t315260196\t1091,500000\t498,250000\t500,000000\r\n2361\t315261884\t1093,500000\t498,000000\t500,000000\r\n2362\t315263596\t1091,500000\t497,450000\t500,000000\r\n2363\t315265298\t1092,500000\t498,250000\t500,000000\r\n2364\t315267000\t1092,000000\t498,500000\t500,000000\r\n2365\t315268701\t1091,500000\t498,000000\t500,000000\r\n2366\t315270388\t1092,500000\t498,500000\t500,000000\r\n2367\t315272095\t1091,000000\t499,000000\t500,000000\r\n2368\t315273798\t1093,000000\t498,500000\t500,000000\r\n2369\t315275503\t1092,000000\t498,250000\t500,000000\r\n2370\t315277204\t1090,000000\t497,750000\t500,000000\r\n2371\t315278908\t1091,500000\t498,750000\t500,000000\r\n2372\t315280600\t1091,500000\t497,750000\t500,000000\r\n2373\t315282303\t1087,900000\t499,000000\t500,000000\r\n2374\t315284007\t1090,500000\t497,250000\t500,000000\r\n2375\t315285707\t1093,000000\t498,250000\t500,000000\r\n2376\t315287391\t1092,000000\t498,750000\t500,000000\r\n2377\t315289084\t1090,400000\t498,000000\t500,000000\r\n2378\t315290776\t1090,500000\t499,250000\t500,000000\r\n2379\t315292476\t1088,300000\t497,750000\t500,000000\r\n2380\t315294173\t1090,900000\t498,000000\t500,000000\r\n2381\t315295869\t1090,800000\t499,000000\t500,000000\r\n2382\t315297569\t1089,500000\t498,250000\t500,000000\r\n2383\t315299260\t1094,500000\t498,250000\t500,000000\r\n2384\t315300938\t1090,500000\t499,000000\t500,000000\r\n2385\t315302636\t1087,900000\t498,750000\t500,000000\r\n2386\t315304344\t1089,000000\t498,500000\t500,000000\r\n2387\t315306048\t1091,500000\t498,750000\t500,000000\r\n2388\t315307749\t1089,400000\t498,000000\t500,000000\r\n2389\t315309452\t1088,900000\t498,500000\t500,000000\r\n2390\t315311156\t1091,500000\t498,500000\t500,000000\r\n2391\t315312859\t1087,800000\t498,500000\t500,000000\r\n2392\t315314560\t1089,900000\t498,750000\t500,000000\r\n2393\t315316257\t1088,800000\t497,750000\t500,000000\r\n2394\t315317968\t1090,800000\t499,250000\t500,000000\r\n2395\t315319666\t1088,400000\t498,000000\t500,000000\r\n2396\t315321367\t1090,500000\t498,250000\t500,000000\r\n2397\t315323066\t1087,900000\t499,000000\t500,000000\r\n2398\t315324772\t1088,400000\t498,000000\t500,000000\r\n2399\t315326472\t1086,700000\t497,500000\t500,000000\r\n2400\t315328161\t1088,200000\t497,750000\t500,000000\r\n2401\t315329865\t1088,700000\t498,250000\t500,000000\r\n2402\t315331553\t1086,700000\t498,000000\t500,000000\r\n2403\t315333259\t1088,700000\t498,500000\t500,000000\r\n2404\t315334961\t1089,400000\t498,000000\t500,000000\r\n2405\t315336660\t1088,700000\t498,500000\t500,000000\r\n2406\t315338360\t1088,900000\t498,000000\t500,000000\r\n2407\t315340058\t1087,900000\t498,250000\t500,000000\r\n2408\t315341766\t1088,200000\t498,750000\t500,000000\r\n2409\t315343451\t1085,600000\t498,250000\t500,000000\r\n2410\t315345157\t1086,000000\t498,500000\t500,000000\r\n2411\t315346858\t1089,300000\t497,250000\t500,000000\r\n2412\t315348564\t1089,000000\t498,250000\t500,000000\r\n2413\t315350264\t1087,200000\t498,500000\t500,000000\r\n2414\t315351970\t1088,700000\t497,750000\t500,000000\r\n2415\t315353681\t1085,100000\t499,250000\t500,000000\r\n2416\t315355363\t1084,400000\t498,000000\t500,000000\r\n2417\t315357063\t1086,600000\t498,000000\t500,000000\r\n2418\t315358758\t1086,600000\t498,500000\t500,000000\r\n2419\t315360451\t1087,100000\t498,500000\t500,000000\r\n2420\t315362153\t1087,200000\t498,750000\t500,000000\r\n2421\t315363847\t1086,000000\t498,250000\t500,000000\r\n2422\t315365547\t1085,500000\t498,000000\t500,000000\r\n2423\t315367246\t1084,900000\t498,750000\t500,000000\r\n2424\t315368938\t1085,500000\t498,250000\t500,000000\r\n2425\t315370639\t1085,100000\t497,200000\t500,000000\r\n2426\t315372331\t1087,600000\t498,500000\t500,000000\r\n2427\t315374016\t1083,900000\t498,250000\t500,000000\r\n2428\t315375694\t1086,000000\t498,000000\t500,000000\r\n2429\t315377398\t1083,900000\t498,000000\t500,000000\r\n2430\t315379087\t1085,600000\t498,500000\t500,000000\r\n2431\t315380789\t1085,400000\t498,000000\t500,000000\r\n2432\t315382493\t1084,800000\t496,700000\t500,000000\r\n2433\t315384190\t1083,900000\t498,250000\t500,000000\r\n2434\t315385892\t1083,900000\t499,000000\t500,000000\r\n2435\t315387584\t1083,200000\t498,250000\t500,000000\r\n2436\t315389279\t1084,400000\t497,750000\t500,000000\r\n2437\t315390978\t1084,700000\t497,750000\t500,000000\r\n2438\t315392674\t1087,700000\t498,000000\t500,000000\r\n2439\t315394375\t1083,800000\t498,250000\t500,000000\r\n2440\t315396069\t1086,500000\t498,000000\t500,000000\r\n2441\t315397760\t1079,500000\t497,450000\t500,000000\r\n2442\t315399457\t1083,300000\t499,000000\t500,000000\r\n2443\t315401163\t1082,700000\t497,500000\t500,000000\r\n2444\t315402859\t1081,100000\t498,250000\t500,000000\r\n2445\t315404558\t1083,800000\t498,000000\t500,000000\r\n2446\t315406252\t1082,800000\t497,750000\t500,000000\r\n2447\t315407944\t1081,300000\t498,750000\t500,000000\r\n2448\t315409643\t1082,300000\t498,250000\t500,000000\r\n2449\t315411341\t1079,500000\t497,500000\t500,000000\r\n2450\t315413044\t1083,200000\t498,250000\t500,000000\r\n2451\t315414736\t1081,100000\t497,500000\t500,000000\r\n2452\t315416437\t1082,200000\t499,000000\t500,000000\r\n2453\t315418142\t1082,700000\t498,250000\t500,000000\r\n2454\t315419844\t1082,700000\t498,000000\t500,000000\r\n2455\t315421539\t1081,000000\t498,750000\t500,000000\r\n2456\t315423221\t1081,000000\t497,500000\t500,000000\r\n2457\t315424917\t1084,400000\t498,000000\t500,000000\r\n2458\t315426614\t1085,000000\t498,500000\t500,000000\r\n2459\t315428309\t1082,700000\t497,500000\t500,000000\r\n2460\t315430007\t1082,700000\t497,750000\t500,000000\r\n2461\t315431706\t1083,300000\t498,250000\t500,000000\r\n2462\t315433404\t1082,700000\t498,750000\t500,000000\r\n2463\t315435085\t1083,700000\t497,500000\t500,000000\r\n2464\t315436783\t1081,800000\t497,500000\t500,000000\r\n2465\t315438479\t1080,100000\t497,500000\t500,000000\r\n2466\t315440177\t1082,200000\t497,750000\t500,000000\r\n2467\t315441878\t1082,800000\t497,200000\t500,000000\r\n2468\t315443573\t1083,800000\t497,500000\t500,000000\r\n2469\t315445272\t1082,700000\t498,000000\t500,000000\r\n2470\t315446974\t1083,300000\t498,750000\t500,000000\r\n2471\t315448671\t1081,200000\t498,000000\t500,000000\r\n2472\t315450364\t1081,000000\t498,000000\t500,000000\r\n2473\t315452059\t1080,500000\t497,750000\t500,000000\r\n2474\t315453756\t1084,400000\t498,250000\t500,000000\r\n2475\t315455451\t1080,000000\t498,000000\t500,000000\r\n2476\t315457149\t1083,800000\t498,250000\t500,000000\r\n2477\t315458845\t1082,600000\t499,000000\t500,000000\r\n2478\t315460544\t1081,700000\t498,250000\t500,000000\r\n2479\t315462255\t1081,700000\t497,750000\t500,000000\r\n2480\t315463959\t1080,000000\t498,000000\t500,000000\r\n2481\t315465646\t1079,500000\t498,500000\t500,000000\r\n2482\t315467325\t1081,700000\t498,500000\t500,000000\r\n2483\t315469022\t1079,500000\t497,500000\t500,000000\r\n2484\t315470727\t1083,400000\t497,500000\t500,000000\r\n2485\t315472436\t1082,300000\t498,000000\t500,000000\r\n2486\t315474134\t1079,700000\t497,750000\t500,000000\r\n2487\t315475837\t1080,100000\t498,750000\t500,000000\r\n2488\t315477530\t1081,200000\t498,500000\t500,000000\r\n2489\t315479236\t1079,000000\t498,250000\t500,000000\r\n2490\t315480939\t1081,800000\t498,750000\t500,000000\r\n2491\t315482637\t1079,000000\t498,000000\t500,000000\r\n2492\t315484336\t1081,800000\t498,500000\t500,000000\r\n2493\t315486039\t1078,500000\t497,500000\t500,000000\r\n2494\t315487736\t1079,100000\t498,500000\t500,000000\r\n2495\t315489440\t1080,200000\t498,500000\t500,000000\r\n2496\t315491144\t1079,100000\t498,250000\t500,000000\r\n2497\t315492850\t1080,600000\t498,250000\t500,000000\r\n2498\t315494564\t1078,600000\t498,250000\t500,000000\r\n2499\t315496263\t1080,600000\t497,500000\t500,000000\r\n2500\t315497966\t1079,000000\t498,500000\t500,000000\r\n2501\t315499670\t1079,600000\t498,500000\t500,000000\r\n2502\t315501372\t1077,600000\t498,250000\t500,000000\r\n2503\t315503072\t1081,200000\t498,500000\t500,000000\r\n2504\t315504781\t1080,200000\t498,250000\t500,000000\r\n2505\t315506484\t1077,000000\t498,000000\t500,000000\r\n2506\t315508194\t1078,000000\t498,000000\t500,000000\r\n2507\t315509898\t1078,000000\t496,950000\t500,000000\r\n2508\t315511602\t1079,500000\t498,000000\t500,000000\r\n2509\t315513304\t1079,600000\t498,000000\t500,000000\r\n2510\t315515012\t1079,200000\t497,750000\t500,000000\r\n2511\t315516716\t1077,600000\t498,000000\t500,000000\r\n2512\t315518408\t1078,500000\t497,500000\t500,000000\r\n2513\t315520093\t1078,600000\t498,250000\t500,000000\r\n2514\t315521787\t1076,500000\t498,250000\t500,000000\r\n2515\t315523489\t1079,700000\t498,500000\t500,000000\r\n2516\t315525191\t1077,500000\t498,250000\t500,000000\r\n2517\t315526885\t1078,500000\t498,000000\t500,000000\r\n2518\t315528580\t1076,500000\t497,750000\t500,000000\r\n2519\t315530268\t1078,200000\t498,500000\t500,000000\r\n2520\t315531971\t1077,600000\t498,500000\t500,000000\r\n2521\t315533673\t1076,000000\t498,000000\t500,000000\r\n2522\t315535377\t1076,600000\t498,250000\t500,000000\r\n2523\t315537079\t1074,500000\t498,750000\t500,000000\r\n2524\t315538778\t1077,600000\t498,250000\t500,000000\r\n2525\t315540476\t1078,100000\t497,750000\t500,000000\r\n2526\t315542170\t1077,000000\t498,000000\t500,000000\r\n2527\t315543863\t1075,500000\t498,000000\t500,000000\r\n2528\t315545566\t1075,500000\t498,000000\t500,000000\r\n2529\t315547268\t1076,500000\t497,700000\t500,000000\r\n2530\t315548964\t1077,700000\t498,500000\t500,000000\r\n2531\t315550663\t1076,000000\t498,000000\t500,000000\r\n2532\t315552366\t1078,100000\t498,250000\t500,000000\r\n2533\t315554066\t1078,700000\t497,250000\t500,000000\r\n2534\t315555773\t1078,200000\t498,500000\t500,000000\r\n2535\t315557477\t1073,600000\t498,000000\t500,000000\r\n2536\t315559176\t1077,600000\t498,750000\t500,000000\r\n2537\t315560879\t1078,100000\t498,250000\t500,000000\r\n2538\t315562582\t1075,500000\t498,500000\t500,000000\r\n2539\t315564287\t1074,000000\t498,000000\t500,000000\r\n2540\t315565984\t1076,600000\t497,750000\t500,000000\r\n2541\t315567688\t1076,600000\t498,750000\t500,000000\r\n2542\t315569388\t1075,500000\t498,250000\t500,000000\r\n2543\t315571090\t1076,000000\t498,250000\t500,000000\r\n2544\t315572789\t1078,000000\t498,000000\t500,000000\r\n2545\t315574493\t1075,000000\t498,250000\t500,000000\r\n2546\t315576195\t1075,600000\t497,500000\t500,000000\r\n2547\t315577901\t1076,700000\t498,250000\t500,000000\r\n2548\t315579597\t1077,100000\t497,500000\t500,000000\r\n2549\t315581303\t1075,500000\t498,250000\t500,000000\r\n2550\t315583002\t1073,500000\t498,000000\t500,000000\r\n2551\t315584705\t1077,600000\t498,250000\t500,000000\r\n2552\t315586411\t1076,100000\t498,000000\t500,000000\r\n2553\t315588119\t1076,600000\t498,000000\t500,000000\r\n2554\t315589824\t1072,000000\t498,000000\t500,000000\r\n2555\t315591526\t1073,500000\t498,500000\t500,000000\r\n2556\t315593232\t1076,100000\t497,750000\t500,000000\r\n2557\t315594937\t1071,000000\t498,500000\t500,000000\r\n2558\t315596644\t1076,100000\t499,000000\t500,000000\r\n2559\t315598345\t1074,600000\t498,000000\t500,000000\r\n2560\t315600030\t1073,000000\t498,750000\t500,000000\r\n2561\t315601734\t1075,000000\t498,250000\t500,000000\r\n2562\t315603445\t1072,500000\t497,500000\t500,000000\r\n2563\t315605141\t1073,500000\t498,750000\t500,000000\r\n2564\t315606827\t1074,500000\t498,000000\t500,000000\r\n2565\t315608528\t1075,000000\t498,250000\t500,000000\r\n2566\t315610233\t1071,500000\t498,750000\t500,000000\r\n2567\t315611939\t1072,500000\t498,500000\t500,000000\r\n2568\t315613646\t1072,000000\t498,000000\t500,000000\r\n2569\t315615346\t1074,000000\t498,250000\t500,000000\r\n2570\t315617026\t1074,500000\t498,000000\t500,000000\r\n2571\t315618730\t1073,500000\t498,250000\t500,000000\r\n2572\t315620431\t1073,500000\t499,250000\t500,000000\r\n2573\t315622135\t1072,000000\t498,750000\t500,000000\r\n2574\t315623836\t1072,500000\t497,500000\t500,000000\r\n2575\t315625544\t1076,100000\t497,750000\t500,000000\r\n2576\t315627245\t1073,000000\t497,250000\t500,000000\r\n2577\t315628946\t1071,500000\t497,500000\t500,000000\r\n2578\t315630646\t1074,600000\t498,750000\t500,000000\r\n2579\t315632353\t1075,600000\t498,250000\t500,000000\r\n2580\t315634059\t1072,000000\t498,000000\t500,000000\r\n2581\t315635760\t1073,000000\t497,250000\t500,000000\r\n2582\t315637467\t1073,000000\t498,500000\t500,000000\r\n2583\t315639167\t1073,000000\t499,250000\t500,000000\r\n2584\t315640864\t1074,500000\t499,250000\t500,000000\r\n2585\t315642559\t1071,000000\t498,250000\t500,000000\r\n2586\t315644261\t1072,500000\t498,250000\t500,000000\r\n2587\t315645964\t1074,100000\t498,000000\t500,000000\r\n2588\t315647661\t1072,500000\t497,500000\t500,000000\r\n2589\t315649364\t1072,500000\t497,750000\t500,000000\r\n2590\t315651073\t1072,000000\t497,000000\t500,000000\r\n2591\t315652773\t1072,000000\t497,750000\t500,000000\r\n2592\t315654475\t1073,100000\t498,000000\t500,000000\r\n2593\t315656177\t1072,500000\t498,750000\t500,000000\r\n2594\t315657875\t1070,500000\t497,750000\t500,000000\r\n2595\t315659578\t1069,000000\t498,000000\t500,000000\r\n2596\t315661286\t1072,000000\t498,500000\t500,000000\r\n2597\t315662987\t1070,500000\t498,250000\t500,000000\r\n2598\t315664688\t1070,500000\t499,000000\t500,000000\r\n2599\t315666389\t1072,000000\t498,500000\t500,000000\r\n2600\t315668087\t1069,000000\t497,750000\t500,000000\r\n2601\t315669774\t1073,000000\t497,750000\t500,000000\r\n2602\t315671451\t1070,000000\t498,500000\t500,000000\r\n2603\t315673138\t1071,500000\t498,000000\t500,000000\r\n2604\t315674840\t1070,000000\t497,250000\t500,000000\r\n2605\t315676549\t1072,500000\t498,000000\t500,000000\r\n2606\t315678253\t1070,500000\t498,750000\t500,000000\r\n2607\t315679954\t1071,000000\t497,500000\t500,000000\r\n2608\t315681650\t1071,500000\t497,750000\t500,000000\r\n2609\t315683346\t1071,100000\t497,750000\t500,000000\r\n2610\t315685047\t1073,600000\t497,500000\t500,000000\r\n2611\t315686747\t1070,000000\t498,000000\t500,000000\r\n2612\t315688444\t1069,500000\t497,750000\t500,000000\r\n2613\t315690137\t1071,500000\t498,000000\t500,000000\r\n2614\t315691823\t1070,000000\t498,000000\t500,000000\r\n2615\t315693523\t1071,000000\t497,750000\t500,000000\r\n2616\t315695223\t1070,500000\t498,500000\t500,000000\r\n2617\t315696915\t1070,500000\t497,750000\t500,000000\r\n2618\t315698612\t1069,000000\t498,250000\t500,000000\r\n2619\t315700309\t1070,000000\t499,000000\t500,000000\r\n2620\t315702009\t1070,500000\t498,000000\t500,000000\r\n2621\t315703708\t1069,500000\t498,250000\t500,000000\r\n2622\t315705404\t1069,500000\t498,250000\t500,000000\r\n2623\t315707111\t1068,000000\t498,250000\t500,000000\r\n2624\t315708806\t1067,000000\t498,000000\t500,000000\r\n2625\t315710503\t1070,000000\t497,750000\t500,000000\r\n2626\t315712186\t1069,000000\t497,500000\t500,000000\r\n2627\t315713864\t1068,000000\t497,500000\t500,000000\r\n2628\t315715559\t1069,500000\t498,000000\t500,000000\r\n2629\t315717258\t1070,500000\t498,000000\t500,000000\r\n2630\t315718953\t1069,500000\t498,250000\t500,000000\r\n2631\t315720650\t1068,500000\t498,750000\t500,000000\r\n2632\t315722326\t1069,500000\t499,000000\t500,000000\r\n2633\t315724019\t1070,500000\t498,000000\t500,000000\r\n2634\t315725723\t1073,500000\t498,500000\t500,000000\r\n2635\t315727416\t1068,500000\t497,000000\t500,000000\r\n2636\t315729117\t1068,000000\t497,500000\t500,000000\r\n2637\t315730814\t1069,500000\t497,500000\t500,000000\r\n2638\t315732511\t1068,000000\t497,750000\t500,000000\r\n2639\t315734208\t1067,500000\t499,250000\t500,000000\r\n2640\t315735891\t1068,000000\t498,500000\t500,000000\r\n2641\t315737594\t1069,000000\t498,750000\t500,000000\r\n2642\t315739288\t1069,500000\t497,750000\t500,000000\r\n2643\t315740993\t1066,500000\t497,750000\t500,000000\r\n2644\t315742691\t1070,500000\t498,250000\t500,000000\r\n2645\t315744391\t1067,000000\t497,500000\t500,000000\r\n2646\t315746099\t1068,500000\t497,450000\t500,000000\r\n2647\t315747806\t1067,500000\t497,750000\t500,000000\r\n2648\t315749509\t1068,500000\t498,000000\t500,000000\r\n2649\t315751212\t1070,000000\t498,250000\t500,000000\r\n2650\t315752895\t1068,000000\t498,500000\t500,000000\r\n2651\t315754599\t1067,500000\t496,450000\t500,000000\r\n2652\t315756284\t1066,500000\t497,750000\t500,000000\r\n2653\t315757986\t1067,500000\t497,750000\t500,000000\r\n2654\t315759689\t1068,000000\t498,500000\t500,000000\r\n2655\t315761396\t1066,000000\t496,700000\t500,000000\r\n2656\t315763103\t1067,000000\t497,500000\t500,000000\r\n2657\t315764806\t1067,000000\t497,500000\t500,000000\r\n2658\t315766516\t1065,500000\t498,750000\t500,000000\r\n2659\t315768214\t1064,500000\t498,250000\t500,000000\r\n2660\t315769914\t1065,500000\t498,250000\t500,000000\r\n2661\t315771619\t1066,500000\t498,000000\t500,000000\r\n2662\t315773317\t1068,000000\t497,750000\t500,000000\r\n2663\t315775019\t1069,000000\t497,750000\t500,000000\r\n2664\t315776724\t1069,000000\t498,000000\t500,000000\r\n2665\t315778427\t1066,500000\t498,250000\t500,000000\r\n2666\t315780126\t1066,500000\t497,750000\t500,000000\r\n2667\t315781814\t1068,000000\t498,500000\t500,000000\r\n2668\t315783521\t1066,500000\t498,500000\t500,000000\r\n2669\t315785219\t1067,500000\t498,000000\t500,000000\r\n2670\t315786914\t1067,000000\t498,500000\t500,000000\r\n2671\t315788622\t1066,000000\t497,750000\t500,000000\r\n2672\t315790322\t1066,500000\t498,000000\t500,000000\r\n2673\t315792023\t1067,000000\t497,750000\t500,000000\r\n2674\t315793727\t1066,500000\t498,000000\t500,000000\r\n2675\t315795429\t1063,500000\t498,750000\t500,000000\r\n2676\t315797134\t1063,500000\t497,750000\t500,000000\r\n2677\t315798840\t1065,000000\t498,000000\t500,000000\r\n2678\t315800546\t1066,500000\t498,750000\t500,000000\r\n2679\t315802254\t1066,500000\t498,250000\t500,000000\r\n2680\t315803953\t1065,000000\t498,250000\t500,000000\r\n2681\t315805659\t1067,000000\t497,750000\t500,000000\r\n2682\t315807370\t1066,500000\t498,000000\t500,000000\r\n2683\t315809077\t1065,000000\t498,250000\t500,000000\r\n2684\t315810771\t1064,500000\t497,200000\t500,000000\r\n2685\t315812469\t1066,000000\t497,750000\t500,000000\r\n2686\t315814161\t1065,500000\t498,250000\t500,000000\r\n2687\t315815853\t1064,000000\t499,000000\t500,000000\r\n2688\t315817551\t1066,500000\t498,500000\t500,000000\r\n2689\t315819254\t1066,500000\t497,750000\t500,000000\r\n2690\t315820954\t1068,000000\t497,700000\t500,000000\r\n2691\t315822653\t1065,000000\t497,250000\t500,000000\r\n2692\t315824349\t1064,500000\t497,750000\t500,000000\r\n2693\t315826043\t1065,000000\t498,250000\t500,000000\r\n2694\t315827742\t1065,000000\t497,750000\t500,000000\r\n2695\t315829439\t1064,000000\t498,500000\t500,000000\r\n2696\t315831135\t1064,500000\t498,750000\t500,000000\r\n2697\t315832840\t1066,000000\t498,000000\t500,000000\r\n2698\t315834534\t1064,500000\t498,750000\t500,000000\r\n2699\t315836241\t1064,500000\t498,000000\t500,000000\r\n2700\t315837923\t1065,500000\t498,500000\t500,000000\r\n2701\t315839611\t1064,500000\t498,500000\t500,000000\r\n2702\t315841303\t1066,000000\t498,750000\t500,000000\r\n2703\t315842989\t1065,000000\t498,500000\t500,000000\r\n2704\t315844687\t1066,000000\t498,000000\t500,000000\r\n2705\t315846383\t1067,000000\t499,000000\t500,000000\r\n2706\t315848088\t1065,500000\t498,000000\t500,000000\r\n2707\t315849764\t1065,500000\t498,500000\t500,000000\r\n2708\t315851463\t1063,000000\t498,750000\t500,000000\r\n2709\t315853164\t1063,500000\t499,250000\t500,000000\r\n2710\t315854864\t1064,000000\t498,750000\t500,000000\r\n2711\t315856571\t1064,000000\t498,000000\t500,000000\r\n2712\t315858269\t1063,000000\t498,000000\t500,000000\r\n2713\t315859964\t1064,000000\t497,750000\t500,000000\r\n2714\t315861664\t1065,500000\t499,250000\t500,000000\r\n2715\t315863366\t1063,500000\t497,750000\t500,000000\r\n2716\t315865058\t1067,000000\t498,250000\t500,000000\r\n2717\t315866753\t1062,500000\t498,250000\t500,000000\r\n2718\t315868453\t1064,500000\t498,250000\t500,000000\r\n2719\t315870154\t1060,000000\t498,000000\t500,000000\r\n2720\t315871843\t1063,000000\t498,000000\t500,000000\r\n2721\t315873541\t1062,000000\t497,750000\t500,000000\r\n2722\t315875237\t1065,000000\t498,500000\t500,000000\r\n2723\t315876929\t1063,500000\t499,250000\t500,000000\r\n2724\t315878631\t1061,500000\t498,750000\t500,000000\r\n2725\t315880338\t1063,000000\t498,000000\t500,000000\r\n2726\t315882038\t1064,000000\t498,000000\t500,000000\r\n2727\t315883743\t1063,000000\t497,750000\t500,000000\r\n2728\t315885453\t1062,000000\t498,250000\t500,000000\r\n2729\t315887159\t1061,000000\t497,500000\t500,000000\r\n2730\t315888858\t1062,500000\t498,750000\t500,000000\r\n2731\t315890563\t1061,000000\t498,500000\t500,000000\r\n2732\t315892267\t1065,000000\t498,250000\t500,000000\r\n2733\t315893968\t1061,000000\t498,500000\t500,000000\r\n2734\t315895672\t1061,500000\t498,500000\t500,000000\r\n2735\t315897377\t1062,500000\t498,250000\t500,000000\r\n2736\t315899076\t1061,500000\t498,500000\t500,000000\r\n2737\t315900763\t1061,500000\t498,000000\t500,000000\r\n2738\t315902464\t1060,500000\t498,750000\t500,000000\r\n2739\t315904168\t1063,000000\t498,750000\t500,000000\r\n2740\t315905869\t1060,500000\t498,500000\t500,000000\r\n2741\t315907578\t1061,000000\t498,750000\t500,000000\r\n2742\t315909278\t1061,500000\t498,500000\t500,000000\r\n2743\t315910966\t1060,000000\t498,250000\t500,000000\r\n2744\t315912673\t1059,000000\t498,000000\t500,000000\r\n2745\t315914376\t1061,500000\t497,500000\t500,000000\r\n2746\t315916084\t1060,000000\t498,750000\t500,000000\r\n2747\t315917785\t1064,100000\t498,250000\t500,000000\r\n2748\t315919491\t1062,500000\t497,250000\t500,000000\r\n2749\t315921194\t1061,500000\t499,500000\t500,000000\r\n2750\t315922891\t1062,500000\t497,000000\t500,000000\r\n2751\t315924592\t1061,000000\t498,250000\t500,000000\r\n2752\t315926295\t1062,500000\t497,500000\t500,000000\r\n2753\t315928004\t1061,000000\t498,250000\t500,000000\r\n2754\t315929687\t1058,000000\t497,250000\t500,000000\r\n2755\t315931386\t1061,000000\t497,750000\t500,000000\r\n2756\t315933088\t1062,500000\t498,500000\t500,000000\r\n2757\t315934788\t1061,000000\t497,750000\t500,000000\r\n2758\t315936492\t1061,500000\t498,500000\t500,000000\r\n2759\t315938197\t1061,000000\t497,750000\t500,000000\r\n2760\t315939899\t1059,500000\t498,000000\t500,000000\r\n2761\t315941591\t1058,000000\t498,750000\t500,000000\r\n2762\t315943284\t1059,500000\t497,500000\t500,000000\r\n2763\t315944981\t1057,000000\t498,000000\t500,000000\r\n2764\t315946674\t1059,000000\t499,500000\t500,000000\r\n2765\t315948372\t1058,500000\t498,250000\t500,000000\r\n2766\t315950069\t1059,500000\t497,500000\t500,000000\r\n2767\t315951770\t1060,000000\t498,500000\t500,000000\r\n2768\t315953471\t1058,500000\t498,000000\t500,000000\r\n2769\t315955168\t1056,500000\t498,000000\t500,000000\r\n2770\t315956864\t1058,500000\t498,250000\t500,000000\r\n2771\t315958561\t1057,000000\t498,000000\t500,000000\r\n2772\t315960263\t1058,500000\t498,750000\t500,000000\r\n2773\t315961961\t1061,000000\t497,750000\t500,000000\r\n2774\t315963664\t1061,000000\t498,500000\t500,000000\r\n2775\t315965363\t1061,000000\t498,250000\t500,000000\r\n2776\t315967053\t1059,500000\t498,000000\t500,000000\r\n2777\t315968735\t1056,000000\t498,750000\t500,000000\r\n2778\t315970428\t1057,500000\t497,700000\t500,000000\r\n2779\t315972129\t1059,000000\t498,250000\t500,000000\r\n2780\t315973806\t1057,000000\t498,000000\t500,000000\r\n2781\t315975502\t1058,000000\t498,000000\t500,000000\r\n2782\t315977206\t1059,000000\t497,000000\t500,000000\r\n2783\t315978906\t1057,000000\t497,750000\t500,000000\r\n2784\t315980597\t1056,500000\t499,250000\t500,000000\r\n2785\t315982292\t1058,000000\t498,250000\t500,000000\r\n2786\t315983984\t1057,500000\t498,250000\t500,000000\r\n2787\t315985691\t1059,500000\t497,750000\t500,000000\r\n2788\t315987388\t1057,500000\t497,750000\t500,000000\r\n2789\t315989083\t1056,000000\t498,000000\t500,000000\r\n2790\t315990783\t1058,500000\t498,250000\t500,000000\r\n2791\t315992481\t1056,000000\t497,750000\t500,000000\r\n2792\t315994178\t1056,500000\t498,250000\t500,000000\r\n2793\t315995874\t1057,000000\t496,700000\t500,000000\r\n2794\t315997572\t1056,500000\t498,750000\t500,000000\r\n2795\t315999264\t1057,500000\t498,750000\t500,000000\r\n2796\t316000951\t1054,500000\t498,250000\t500,000000\r\n2797\t316002651\t1056,500000\t497,500000\t500,000000\r\n2798\t316004354\t1056,000000\t498,750000\t500,000000\r\n2799\t316006048\t1056,500000\t498,500000\t500,000000\r\n2800\t316007754\t1059,000000\t498,750000\t500,000000\r\n2801\t316009459\t1058,500000\t498,250000\t500,000000\r\n2802\t316011166\t1055,000000\t497,750000\t500,000000\r\n2803\t316012868\t1058,000000\t498,500000\t500,000000\r\n2804\t316014570\t1058,000000\t498,250000\t500,000000\r\n2805\t316016279\t1055,500000\t498,000000\t500,000000\r\n2806\t316017975\t1054,500000\t498,250000\t500,000000\r\n2807\t316019680\t1057,500000\t497,500000\t500,000000\r\n2808\t316021381\t1058,500000\t498,000000\t500,000000\r\n2809\t316023084\t1055,000000\t498,500000\t500,000000\r\n2810\t316024792\t1053,500000\t498,000000\t500,000000\r\n2811\t316026496\t1055,000000\t497,750000\t500,000000\r\n2812\t316028201\t1056,500000\t498,000000\t500,000000\r\n2813\t316029898\t1056,500000\t498,750000\t500,000000\r\n2814\t316031604\t1054,000000\t498,500000\t500,000000\r\n2815\t316033315\t1056,000000\t498,250000\t500,000000\r\n2816\t316035015\t1054,500000\t498,250000\t500,000000\r\n2817\t316036721\t1057,000000\t498,250000\t500,000000\r\n2818\t316038420\t1053,500000\t498,250000\t500,000000\r\n2819\t316040126\t1053,000000\t498,500000\t500,000000\r\n2820\t316041829\t1055,500000\t498,000000\t500,000000\r\n2821\t316043529\t1054,000000\t499,000000\t500,000000\r\n2822\t316045230\t1053,500000\t498,750000\t500,000000\r\n2823\t316046927\t1055,500000\t498,000000\t500,000000\r\n2824\t316048630\t1050,000000\t498,750000\t500,000000\r\n2825\t316050333\t1057,500000\t497,750000\t500,000000\r\n2826\t316052031\t1053,000000\t497,000000\t500,000000\r\n2827\t316053737\t1052,500000\t498,500000\t500,000000\r\n2828\t316055449\t1055,500000\t499,000000\t500,000000\r\n2829\t316057158\t1052,500000\t499,750000\t500,000000\r\n2830\t316058843\t1054,500000\t498,250000\t500,000000\r\n2831\t316060544\t1053,500000\t498,000000\t500,000000\r\n2832\t316062246\t1055,500000\t498,500000\t500,000000\r\n2833\t316063946\t1054,000000\t498,500000\t500,000000\r\n2834\t316065644\t1053,500000\t498,500000\t500,000000\r\n2835\t316067341\t1053,500000\t498,000000\t500,000000\r\n2836\t316069035\t1053,500000\t498,250000\t500,000000\r\n2837\t316070736\t1054,000000\t498,000000\t500,000000\r\n2838\t316072433\t1055,000000\t498,250000\t500,000000\r\n2839\t316074127\t1054,000000\t498,000000\t500,000000\r\n2840\t316075829\t1054,500000\t498,500000\t500,000000\r\n2841\t316077529\t1055,500000\t498,250000\t500,000000\r\n2842\t316079220\t1053,500000\t497,750000\t500,000000\r\n2843\t316080912\t1051,400000\t498,500000\t500,000000\r\n2844\t316082616\t1050,000000\t498,000000\t500,000000\r\n2845\t316084314\t1051,500000\t498,500000\t500,000000\r\n2846\t316086014\t1053,500000\t498,500000\t500,000000\r\n2847\t316087715\t1053,000000\t498,250000\t500,000000\r\n2848\t316089409\t1050,000000\t497,750000\t500,000000\r\n2849\t316091105\t1052,500000\t499,000000\t500,000000\r\n2850\t316092808\t1052,500000\t498,250000\t500,000000\r\n2851\t316094507\t1051,500000\t498,000000\t500,000000\r\n2852\t316096191\t1052,000000\t498,000000\t500,000000\r\n2853\t316097896\t1051,500000\t498,250000\t500,000000\r\n2854\t316099578\t1053,000000\t498,250000\t500,000000\r\n2855\t316101283\t1051,000000\t497,000000\t500,000000\r\n2856\t316102969\t1052,000000\t498,500000\t500,000000\r\n2857\t316104664\t1050,500000\t497,450000\t500,000000\r\n2858\t316106364\t1050,000000\t498,500000\t500,000000\r\n2859\t316108061\t1050,500000\t499,500000\t500,000000\r\n2860\t316109759\t1050,500000\t498,500000\t500,000000\r\n2861\t316111454\t1051,500000\t498,500000\t500,000000\r\n2862\t316113150\t1054,500000\t497,500000\t500,000000\r\n2863\t316114846\t1053,000000\t497,750000\t500,000000\r\n2864\t316116538\t1051,500000\t497,750000\t500,000000\r\n2865\t316118238\t1051,000000\t497,750000\t500,000000\r\n2866\t316119935\t1052,000000\t498,750000\t500,000000\r\n2867\t316121638\t1052,000000\t498,750000\t500,000000\r\n2868\t316123331\t1051,500000\t497,750000\t500,000000\r\n2869\t316125029\t1050,500000\t498,250000\t500,000000\r\n2870\t316126731\t1051,000000\t498,250000\t500,000000\r\n2871\t316128427\t1053,000000\t498,250000\t500,000000\r\n2872\t316130122\t1052,000000\t498,750000\t500,000000\r\n2873\t316131825\t1049,000000\t498,000000\t500,000000\r\n2874\t316133523\t1050,500000\t498,750000\t500,000000\r\n2875\t316135220\t1050,000000\t498,500000\t500,000000\r\n2876\t316136921\t1051,000000\t497,750000\t500,000000\r\n2877\t316138616\t1049,000000\t499,000000\t500,000000\r\n2878\t316140320\t1048,500000\t498,250000\t500,000000\r\n2879\t316142021\t1050,500000\t497,500000\t500,000000\r\n2880\t316143733\t1052,000000\t498,000000\t500,000000\r\n2881\t316145439\t1048,000000\t497,500000\t500,000000\r\n2882\t316147142\t1052,000000\t498,500000\t500,000000\r\n2883\t316148851\t1050,500000\t498,250000\t500,000000\r\n2884\t316150551\t1052,000000\t498,250000\t500,000000\r\n2885\t316152257\t1049,500000\t499,750000\t500,000000\r\n2886\t316153966\t1050,500000\t499,250000\t500,000000\r\n2887\t316155673\t1049,000000\t497,500000\t500,000000\r\n2888\t316157376\t1051,000000\t499,000000\t500,000000\r\n2889\t316159080\t1050,000000\t498,250000\t500,000000\r\n2890\t316160781\t1050,500000\t497,250000\t500,000000\r\n2891\t316162490\t1048,500000\t497,500000\t500,000000\r\n2892\t316164179\t1050,500000\t497,750000\t500,000000\r\n2893\t316165885\t1048,500000\t498,000000\t500,000000\r\n2894\t316167589\t1049,000000\t499,250000\t500,000000\r\n2895\t316169288\t1049,500000\t497,250000\t500,000000\r\n2896\t316170982\t1049,000000\t498,250000\t500,000000\r\n2897\t316172690\t1049,500000\t499,500000\t500,000000\r\n2898\t316174391\t1049,500000\t497,750000\t500,000000\r\n2899\t316176089\t1050,000000\t498,250000\t500,000000\r\n2900\t316177799\t1048,500000\t499,250000\t500,000000\r\n2901\t316179498\t1048,500000\t499,000000\t500,000000\r\n2902\t316181199\t1048,500000\t498,250000\t500,000000\r\n2903\t316182904\t1050,000000\t498,000000\t500,000000\r\n2904\t316184609\t1050,500000\t498,500000\t500,000000\r\n2905\t316186311\t1047,500000\t498,000000\t500,000000\r\n2906\t316187996\t1049,000000\t498,750000\t500,000000\r\n2907\t316189706\t1050,000000\t498,250000\t500,000000\r\n2908\t316191408\t1048,500000\t497,750000\t500,000000\r\n2909\t316193113\t1047,000000\t498,500000\t500,000000\r\n2910\t316194815\t1049,500000\t498,250000\t500,000000\r\n2911\t316196516\t1047,500000\t498,250000\t500,000000\r\n2912\t316198215\t1047,500000\t497,500000\t500,000000\r\n2913\t316199914\t1049,000000\t498,250000\t500,000000\r\n2914\t316201614\t1048,500000\t498,750000\t500,000000\r\n2915\t316203316\t1049,000000\t496,700000\t500,000000\r\n2916\t316205017\t1048,500000\t497,750000\t500,000000\r\n2917\t316206719\t1047,500000\t498,500000\t500,000000\r\n2918\t316208414\t1046,500000\t497,750000\t500,000000\r\n2919\t316210115\t1049,500000\t498,250000\t500,000000\r\n2920\t316211829\t1050,500000\t498,250000\t500,000000\r\n2921\t316213534\t1048,500000\t498,250000\t500,000000\r\n2922\t316215237\t1049,500000\t498,750000\t500,000000\r\n2923\t316216943\t1049,000000\t498,000000\t500,000000\r\n2924\t316218648\t1048,000000\t498,250000\t500,000000\r\n2925\t316220343\t1049,000000\t498,500000\t500,000000\r\n2926\t316222043\t1048,000000\t498,250000\t500,000000\r\n2927\t316223742\t1047,000000\t498,750000\t500,000000\r\n2928\t316225445\t1047,000000\t497,750000\t500,000000\r\n2929\t316227152\t1048,500000\t499,250000\t500,000000\r\n2930\t316228856\t1049,500000\t498,750000\t500,000000\r\n2931\t316230556\t1046,500000\t498,750000\t500,000000\r\n2932\t316232267\t1046,500000\t499,000000\t500,000000\r\n2933\t316233945\t1048,000000\t498,250000\t500,000000\r\n2934\t316235652\t1048,000000\t497,750000\t500,000000\r\n2935\t316237351\t1049,500000\t497,250000\t500,000000\r\n2936\t316239053\t1047,500000\t497,750000\t500,000000\r\n2937\t316240740\t1047,500000\t498,000000\t500,000000\r\n2938\t316242429\t1046,000000\t497,250000\t500,000000\r\n2939\t316244128\t1042,900000\t498,250000\t500,000000\r\n2940\t316245821\t1049,500000\t497,750000\t500,000000\r\n2941\t316247521\t1047,000000\t499,250000\t500,000000\r\n2942\t316249221\t1048,500000\t498,750000\t500,000000\r\n2943\t316250916\t1046,000000\t499,250000\t500,000000\r\n2944\t316252614\t1048,000000\t499,000000\t500,000000\r\n2945\t316254314\t1049,500000\t497,250000\t500,000000\r\n2946\t316256016\t1050,000000\t498,000000\t500,000000\r\n2947\t316257722\t1046,500000\t498,500000\t500,000000\r\n2948\t316259423\t1047,500000\t498,000000\t500,000000\r\n2949\t316261134\t1047,500000\t498,250000\t500,000000\r\n2950\t316262841\t1046,500000\t498,500000\t500,000000\r\n2951\t316264543\t1046,000000\t498,750000\t500,000000\r\n2952\t316266234\t1045,500000\t497,500000\t500,000000\r\n2953\t316267936\t1045,000000\t498,250000\t500,000000\r\n2954\t316269638\t1047,000000\t497,750000\t500,000000\r\n2955\t316271338\t1047,000000\t497,200000\t500,000000\r\n2956\t316273038\t1046,500000\t498,000000\t500,000000\r\n2957\t316274744\t1047,000000\t498,750000\t500,000000\r\n2958\t316276448\t1045,500000\t498,200000\t500,000000\r\n2959\t316278141\t1047,000000\t498,250000\t500,000000\r\n2960\t316279841\t1045,000000\t498,750000\t500,000000\r\n2961\t316281532\t1048,000000\t498,500000\t500,000000\r\n2962\t316283227\t1043,500000\t497,500000\t500,000000\r\n2963\t316284920\t1047,000000\t498,250000\t500,000000\r\n2964\t316286618\t1044,500000\t499,000000\t500,000000\r\n2965\t316288316\t1045,000000\t497,750000\t500,000000\r\n2966\t316289994\t1045,000000\t499,000000\t500,000000\r\n2967\t316291696\t1044,900000\t499,000000\t500,000000\r\n2968\t316293395\t1046,000000\t498,750000\t500,000000\r\n2969\t316295081\t1046,000000\t499,000000\t500,000000\r\n2970\t316296777\t1047,000000\t498,750000\t500,000000\r\n2971\t316298478\t1045,000000\t499,750000\t500,000000\r\n2972\t316300174\t1047,000000\t498,250000\t500,000000\r\n2973\t316301876\t1042,500000\t497,750000\t500,000000\r\n2974\t316303583\t1046,500000\t498,250000\t500,000000\r\n2975\t316305293\t1043,500000\t497,750000\t500,000000\r\n2976\t316306993\t1044,500000\t498,750000\t500,000000\r\n2977\t316308696\t1045,500000\t499,000000\t500,000000\r\n2978\t316310383\t1045,000000\t498,750000\t500,000000\r\n2979\t316312089\t1044,500000\t497,750000\t500,000000\r\n2980\t316313792\t1043,500000\t498,500000\t500,000000\r\n2981\t316315494\t1045,500000\t498,500000\t500,000000\r\n2982\t316317193\t1047,000000\t497,750000\t500,000000\r\n2983\t316318896\t1047,000000\t498,500000\t500,000000\r\n2984\t316320596\t1043,000000\t498,000000\t500,000000\r\n2985\t316322291\t1043,400000\t498,750000\t500,000000\r\n2986\t316323998\t1044,500000\t498,250000\t500,000000\r\n2987\t316325700\t1044,500000\t498,000000\t500,000000\r\n2988\t316327402\t1043,500000\t497,750000\t500,000000\r\n2989\t316329105\t1043,000000\t498,000000\t500,000000\r\n2990\t316330805\t1044,000000\t498,500000\t500,000000\r\n2991\t316332499\t1045,000000\t497,500000\t500,000000\r\n2992\t316334194\t1044,500000\t498,000000\t500,000000\r\n2993\t316335896\t1043,500000\t498,250000\t500,000000\r\n2994\t316337592\t1045,000000\t498,000000\t500,000000\r\n2995\t316339295\t1047,000000\t498,000000\t500,000000\r\n2996\t316340992\t1045,500000\t498,750000\t500,000000\r\n2997\t316342693\t1042,500000\t498,000000\t500,000000\r\n2998\t316344392\t1044,000000\t498,250000\t500,000000\r\n2999\t316346082\t1045,000000\t498,000000\t500,000000\r\n3000\t316347785\t1043,000000\t498,750000\t500,000000\r\n3001\t316349480\t1043,500000\t497,750000\t500,000000\r\n3002\t316351185\t1044,000000\t498,500000\t500,000000\r\n3003\t316352889\t1046,000000\t497,200000\t500,000000\r\n3004\t316354596\t1042,000000\t497,200000\t500,000000\r\n3005\t316356299\t1043,000000\t498,500000\t500,000000\r\n3006\t316358007\t1046,000000\t498,250000\t500,000000\r\n3007\t316359706\t1044,000000\t498,250000\t500,000000\r\n3008\t316361631\t1045,000000\t498,250000\t500,000000\r\n3009\t316363331\t1044,400000\t498,250000\t500,000000\r\n3010\t316365034\t1041,000000\t498,000000\t500,000000\r\n3011\t316366735\t1045,000000\t498,000000\t500,000000\r\n3012\t316368427\t1043,000000\t498,000000\t500,000000\r\n3013\t316370125\t1044,000000\t498,000000\t500,000000\r\n3014\t316371825\t1043,000000\t498,750000\t500,000000\r\n3015\t316373526\t1041,500000\t498,250000\t500,000000\r\n3016\t316375225\t1041,500000\t497,750000\t500,000000\r\n3017\t316376921\t1039,500000\t497,500000\t500,000000\r\n3018\t316378626\t1043,500000\t499,000000\t500,000000\r\n3019\t316380330\t1043,000000\t497,750000\t500,000000\r\n3020\t316382039\t1040,900000\t496,450000\t500,000000\r\n3021\t316383744\t1043,000000\t497,750000\t500,000000\r\n3022\t316385449\t1041,500000\t498,750000\t500,000000\r\n3023\t316387153\t1043,000000\t498,000000\t500,000000\r\n3024\t316388855\t1043,500000\t498,250000\t500,000000\r\n3025\t316391071\t1039,500000\t498,000000\t500,000000\r\n3026\t316392767\t1043,500000\t498,500000\t500,000000\r\n3027\t316394460\t1043,500000\t498,500000\t500,000000\r\n3028\t316396119\t1045,000000\t499,750000\t500,000000\r\n3029\t316397660\t1041,500000\t498,750000\t500,000000\r\n3030\t316399353\t1041,000000\t497,250000\t500,000000\r\n3031\t316400620\t1043,000000\t496,950000\t500,000000\r\n3032\t316401751\t1041,500000\t498,000000\t500,000000\r\n3033\t316402888\t1039,400000\t497,500000\t500,000000\r\n3034\t316404030\t1039,400000\t498,000000\t500,000000\r\n3035\t316405168\t1038,500000\t496,950000\t500,000000\r\n3036\t316406303\t1040,500000\t498,000000\t500,000000\r\n3037\t316407435\t1042,000000\t497,750000\t500,000000\r\n3038\t316408575\t1043,000000\t498,750000\t500,000000\r\n3039\t316409715\t1039,000000\t498,500000\t500,000000\r\n3040\t316410854\t1042,000000\t498,000000\t500,000000\r\n3041\t316411995\t1038,900000\t497,250000\t500,000000\r\n3042\t316413135\t1042,000000\t497,500000\t500,000000\r\n3043\t316414271\t1041,500000\t498,750000\t500,000000\r\n3044\t316415402\t1040,000000\t497,750000\t500,000000\r\n3045\t316416539\t1040,500000\t497,750000\t500,000000\r\n3046\t316417679\t1039,500000\t498,750000\t500,000000\r\n3047\t316418815\t1042,900000\t498,750000\t500,000000\r\n3048\t316419947\t1039,900000\t498,250000\t500,000000\r\n3049\t316421086\t1039,400000\t498,750000\t500,000000\r\n3050\t316422226\t1040,500000\t498,000000\t500,000000\r\n3051\t316423360\t1038,500000\t499,000000\t500,000000\r\n3052\t316424499\t1040,000000\t497,250000\t500,000000\r\n3053\t316425636\t1039,300000\t498,250000\t500,000000\r\n3054\t316426768\t1040,000000\t498,500000\t500,000000\r\n3055\t316427902\t1036,400000\t498,000000\t500,000000\r\n3056\t316429038\t1039,400000\t498,250000\t500,000000\r\n3057\t316430173\t1040,500000\t498,750000\t500,000000\r\n3058\t316431315\t1037,900000\t497,500000\t500,000000\r\n3059\t316432453\t1040,000000\t498,000000\t500,000000\r\n3060\t316433591\t1040,900000\t498,250000\t500,000000\r\n3061\t316434734\t1038,900000\t498,000000\t500,000000\r\n3062\t316435875\t1039,000000\t498,750000\t500,000000\r\n3063\t316437015\t1038,500000\t498,250000\t500,000000\r\n3064\t316438149\t1038,900000\t498,250000\t500,000000\r\n3065\t316439289\t1037,900000\t498,000000\t500,000000\r\n3066\t316440425\t1040,900000\t498,500000\t500,000000\r\n3067\t316441565\t1039,000000\t498,000000\t500,000000\r\n3068\t316442708\t1040,000000\t498,750000\t500,000000\r\n3069\t316443844\t1039,500000\t498,500000\t500,000000\r\n3070\t316444976\t1039,000000\t498,250000\t500,000000\r\n3071\t316446116\t1040,000000\t498,250000\t500,000000\r\n3072\t316447261\t1041,500000\t498,000000\t500,000000\r\n3073\t316448400\t1036,200000\t498,000000\t500,000000\r\n3074\t316449535\t1038,400000\t498,750000\t500,000000\r\n3075\t316450679\t1038,400000\t498,250000\t500,000000\r\n3076\t316451818\t1040,500000\t497,750000\t500,000000\r\n3077\t316452958\t1039,000000\t498,000000\t500,000000\r\n3078\t316454089\t1039,000000\t498,500000\t500,000000\r\n3079\t316455226\t1038,500000\t497,750000\t500,000000\r\n3080\t316456368\t1040,500000\t498,500000\t500,000000\r\n3081\t316457507\t1038,300000\t498,500000\t500,000000\r\n3082\t316458648\t1038,900000\t498,750000\t500,000000\r\n3083\t316459781\t1036,900000\t498,500000\t500,000000\r\n3084\t316460919\t1033,600000\t498,500000\t500,000000\r\n3085\t316462061\t1036,300000\t498,250000\t500,000000\r\n3086\t316463194\t1039,500000\t497,000000\t500,000000\r\n3087\t316464330\t1038,900000\t498,250000\t500,000000\r\n3088\t316465475\t1038,400000\t497,750000\t500,000000\r\n3089\t316466610\t1038,000000\t498,750000\t500,000000\r\n3090\t316467744\t1041,000000\t497,000000\t500,000000\r\n3091\t316468880\t1037,900000\t498,000000\t500,000000\r\n3092\t316470014\t1038,900000\t499,000000\t500,000000\r\n3093\t316471150\t1040,400000\t497,000000\t500,000000\r\n3094\t316472287\t1038,400000\t498,500000\t500,000000\r\n3095\t316473434\t1037,800000\t498,500000\t500,000000\r\n3096\t316474568\t1036,200000\t497,750000\t500,000000\r\n3097\t316475704\t1036,200000\t498,250000\t500,000000\r\n3098\t316476836\t1039,000000\t498,250000\t500,000000\r\n3099\t316477972\t1036,900000\t498,250000\t500,000000\r\n3100\t316479113\t1037,300000\t498,000000\t500,000000\r\n3101\t316480253\t1038,400000\t497,500000\t500,000000\r\n3102\t316481389\t1037,400000\t498,000000\t500,000000\r\n3103\t316482533\t1035,800000\t499,000000\t500,000000\r\n3104\t316483677\t1039,400000\t497,500000\t500,000000\r\n3105\t316484818\t1037,800000\t497,250000\t500,000000\r\n3106\t316485954\t1036,800000\t497,750000\t500,000000\r\n3107\t316487089\t1038,300000\t499,000000\t500,000000\r\n3108\t316488223\t1036,800000\t498,000000\t500,000000\r\n3109\t316489358\t1037,800000\t498,000000\t500,000000\r\n3110\t316490505\t1037,400000\t498,000000\t500,000000\r\n3111\t316491639\t1037,900000\t498,250000\t500,000000\r\n3112\t316492772\t1040,000000\t498,000000\t500,000000\r\n3113\t316493917\t1038,500000\t498,500000\t500,000000\r\n3114\t316495058\t1038,900000\t498,250000\t500,000000\r\n3115\t316496199\t1039,500000\t498,000000\t500,000000\r\n3116\t316497329\t1037,400000\t498,750000\t500,000000\r\n3117\t316498468\t1037,900000\t498,500000\t500,000000\r\n3118\t316499602\t1037,800000\t498,250000\t500,000000\r\n3119\t316500744\t1037,800000\t498,000000\t500,000000\r\n3120\t316501880\t1036,700000\t498,000000\t500,000000\r\n3121\t316503019\t1037,400000\t497,500000\t500,000000\r\n3122\t316504159\t1036,700000\t498,000000\t500,000000\r\n3123\t316505296\t1037,200000\t498,500000\t500,000000\r\n3124\t316506437\t1034,500000\t497,500000\t500,000000\r\n3125\t316507575\t1035,600000\t497,750000\t500,000000\r\n3126\t316508712\t1037,300000\t498,500000\t500,000000\r\n3127\t316509848\t1037,800000\t498,750000\t500,000000\r\n3128\t316510995\t1036,200000\t498,000000\t500,000000\r\n3129\t316512136\t1036,200000\t498,000000\t500,000000\r\n3130\t316513278\t1035,900000\t498,250000\t500,000000\r\n3131\t316514416\t1037,900000\t498,750000\t500,000000\r\n3132\t316515547\t1034,600000\t497,450000\t500,000000\r\n3133\t316516687\t1036,800000\t497,750000\t500,000000\r\n3134\t316517825\t1035,700000\t498,000000\t500,000000\r\n3135\t316518959\t1036,800000\t498,500000\t500,000000\r\n3136\t316520103\t1035,700000\t497,750000\t500,000000\r\n3137\t316521243\t1033,900000\t496,950000\t500,000000\r\n3138\t316522382\t1036,200000\t498,000000\t500,000000\r\n3139\t316523525\t1037,800000\t497,500000\t500,000000\r\n3140\t316524665\t1034,700000\t498,000000\t500,000000\r\n3141\t316525800\t1036,300000\t497,750000\t500,000000\r\n3142\t316526939\t1034,600000\t498,000000\t500,000000\r\n3143\t316528076\t1037,900000\t499,250000\t500,000000\r\n3144\t316529214\t1038,900000\t498,500000\t500,000000\r\n3145\t316530350\t1035,700000\t498,000000\t500,000000\r\n3146\t316531495\t1036,200000\t498,250000\t500,000000\r\n3147\t316532635\t1034,000000\t497,750000\t500,000000\r\n3148\t316533770\t1034,500000\t498,250000\t500,000000\r\n3149\t316534916\t1035,700000\t498,500000\t500,000000\r\n3150\t316536059\t1036,300000\t498,500000\t500,000000\r\n3151\t316537193\t1036,800000\t497,750000\t500,000000\r\n3152\t316538328\t1036,700000\t498,000000\t500,000000\r\n3153\t316539464\t1034,100000\t497,250000\t500,000000\r\n3154\t316540603\t1035,600000\t498,000000\t500,000000\r\n3155\t316541739\t1035,400000\t498,250000\t500,000000\r\n3156\t316542883\t1036,200000\t498,000000\t500,000000\r\n3157\t316544017\t1035,700000\t498,750000\t500,000000\r\n3158\t316545153\t1036,000000\t498,250000\t500,000000\r\n3159\t316546294\t1034,000000\t498,250000\t500,000000\r\n3160\t316547435\t1034,800000\t498,500000\t500,000000\r\n3161\t316548572\t1035,600000\t498,250000\t500,000000\r\n3162\t316549705\t1034,500000\t498,250000\t500,000000\r\n3163\t316550844\t1036,000000\t497,750000\t500,000000\r\n3164\t316551984\t1036,200000\t498,250000\t500,000000\r\n3165\t316553120\t1034,000000\t498,250000\t500,000000\r\n3166\t316554263\t1035,700000\t498,000000\t500,000000\r\n3167\t316555405\t1036,100000\t498,500000\t500,000000\r\n3168\t316556542\t1036,700000\t497,500000\t500,000000\r\n3169\t316557674\t1036,700000\t498,250000\t500,000000\r\n3170\t316558820\t1033,400000\t498,250000\t500,000000\r\n3171\t316559952\t1035,100000\t497,750000\t500,000000\r\n3172\t316561096\t1033,100000\t497,500000\t500,000000\r\n3173\t316562231\t1036,200000\t497,500000\t500,000000\r\n3174\t316563364\t1031,200000\t498,750000\t500,000000\r\n3175\t316564504\t1033,400000\t498,500000\t500,000000\r\n3176\t316565643\t1034,500000\t498,250000\t500,000000\r\n3177\t316566787\t1033,200000\t497,750000\t500,000000\r\n3178\t316567925\t1034,500000\t498,250000\t500,000000\r\n3179\t316569063\t1033,900000\t498,250000\t500,000000\r\n3180\t316570208\t1034,900000\t499,250000\t500,000000\r\n3181\t316571356\t1035,100000\t497,750000\t500,000000\r\n3182\t316572494\t1037,400000\t498,250000\t500,000000\r\n3183\t316573639\t1034,800000\t497,500000\t500,000000\r\n3184\t316574777\t1034,500000\t498,250000\t500,000000\r\n3185\t316575914\t1031,900000\t496,750000\t500,000000\r\n3186\t316577056\t1031,700000\t498,500000\t500,000000\r\n3187\t316578197\t1031,200000\t497,250000\t500,000000\r\n3188\t316579331\t1033,500000\t497,750000\t500,000000\r\n3189\t316580472\t1034,500000\t497,750000\t500,000000\r\n3190\t316581604\t1032,900000\t498,250000\t500,000000\r\n3191\t316582742\t1034,400000\t498,250000\t500,000000\r\n3192\t316583880\t1032,900000\t498,250000\t500,000000\r\n3193\t316585018\t1033,300000\t497,750000\t500,000000\r\n3194\t316586153\t1035,400000\t498,250000\t500,000000\r\n3195\t316587294\t1035,000000\t498,750000\t500,000000\r\n3196\t316588431\t1031,200000\t498,000000\t500,000000\r\n3197\t316589565\t1032,900000\t498,500000\t500,000000\r\n3198\t316590705\t1034,600000\t498,750000\t500,000000\r\n3199\t316591845\t1032,900000\t498,250000\t500,000000\r\n3200\t316592979\t1031,300000\t498,500000\t500,000000\r\n3201\t316594113\t1032,900000\t498,000000\t500,000000\r\n3202\t316595246\t1032,300000\t498,250000\t500,000000\r\n3203\t316596388\t1032,800000\t498,250000\t500,000000\r\n3204\t316597527\t1033,300000\t498,500000\t500,000000\r\n3205\t316598625\t1029,700000\t498,500000\t500,000000\r\n3206\t316599763\t1031,300000\t499,000000\t500,000000\r\n3207\t316600897\t1032,200000\t498,750000\t500,000000\r\n3208\t316602022\t1033,500000\t498,000000\t500,000000\r\n3209\t316603155\t1033,300000\t497,500000\t500,000000\r\n3210\t316604293\t1033,400000\t498,250000\t500,000000\r\n3211\t316605428\t1033,900000\t498,000000\t500,000000\r\n3212\t316606559\t1034,300000\t498,250000\t500,000000\r\n3213\t316607688\t1032,800000\t499,000000\t500,000000\r\n3214\t316608821\t1031,700000\t498,250000\t500,000000\r\n3215\t316609959\t1035,000000\t498,000000\t500,000000\r\n3216\t316611094\t1031,100000\t498,000000\t500,000000\r\n3217\t316612235\t1031,900000\t498,000000\t500,000000\r\n3218\t316613370\t1033,900000\t498,000000\t500,000000\r\n3219\t316614512\t1032,300000\t498,250000\t500,000000\r\n3220\t316615651\t1031,300000\t499,000000\t500,000000\r\n3221\t316616780\t1033,900000\t498,250000\t500,000000\r\n3222\t316617918\t1032,700000\t497,500000\t500,000000\r\n3223\t316619059\t1034,600000\t498,500000\t500,000000\r\n3224\t316620190\t1029,600000\t498,000000\t500,000000\r\n3225\t316621328\t1031,200000\t497,750000\t500,000000\r\n3226\t316622467\t1032,300000\t498,250000\t500,000000\r\n3227\t316623606\t1030,000000\t499,000000\t500,000000\r\n3228\t316624751\t1033,800000\t497,750000\t500,000000\r\n3229\t316625883\t1033,400000\t497,750000\t500,000000\r\n3230\t316627018\t1031,800000\t498,000000\t500,000000\r\n3231\t316628159\t1031,800000\t499,250000\t500,000000\r\n3232\t316629299\t1029,800000\t498,000000\t500,000000\r\n3233\t316630440\t1031,200000\t497,000000\t500,000000\r\n3234\t316631579\t1030,600000\t498,000000\t500,000000\r\n3235\t316632720\t1030,900000\t497,500000\t500,000000\r\n3236\t316633851\t1030,600000\t497,500000\t500,000000\r\n3237\t316634990\t1031,700000\t497,750000\t500,000000\r\n3238\t316636132\t1033,800000\t498,750000\t500,000000\r\n3239\t316637269\t1030,300000\t498,000000\t500,000000\r\n3240\t316638406\t1033,200000\t498,250000\t500,000000\r\n3241\t316639543\t1030,800000\t497,750000\t500,000000\r\n3242\t316640684\t1033,800000\t498,250000\t500,000000\r\n3243\t316641820\t1030,100000\t498,000000\t500,000000\r\n3244\t316642953\t1029,600000\t498,000000\t500,000000\r\n3245\t316644098\t1031,300000\t498,000000\t500,000000\r\n3246\t316645232\t1033,400000\t498,000000\t500,000000\r\n3247\t316646370\t1032,800000\t498,000000\t500,000000\r\n3248\t316647505\t1031,200000\t499,250000\t500,000000\r\n3249\t316648639\t1033,400000\t498,000000\t500,000000\r\n3250\t316649776\t1030,300000\t498,500000\t500,000000\r\n3251\t316650909\t1031,800000\t496,950000\t500,000000\r\n3252\t316652051\t1030,700000\t498,500000\t500,000000\r\n3253\t316653194\t1031,800000\t498,500000\t500,000000\r\n3254\t316654338\t1032,200000\t498,500000\t500,000000\r\n3255\t316655473\t1031,200000\t498,750000\t500,000000\r\n3256\t316656614\t1029,700000\t498,000000\t500,000000\r\n3257\t316657749\t1030,300000\t498,750000\t500,000000\r\n3258\t316658894\t1030,700000\t497,750000\t500,000000\r\n3259\t316660024\t1032,200000\t497,500000\t500,000000\r\n3260\t316661156\t1029,600000\t497,250000\t500,000000\r\n3261\t316662301\t1032,900000\t498,750000\t500,000000\r\n3262\t316663441\t1030,200000\t498,000000\t500,000000\r\n3263\t316664578\t1030,000000\t499,000000\t500,000000\r\n3264\t316665726\t1031,700000\t498,250000\t500,000000\r\n3265\t316666863\t1030,700000\t498,250000\t500,000000\r\n3266\t316668000\t1031,100000\t498,500000\t500,000000\r\n3267\t316669135\t1032,400000\t499,000000\t500,000000\r\n3268\t316670274\t1030,600000\t498,000000\t500,000000\r\n3269\t316671408\t1033,300000\t498,250000\t500,000000\r\n3270\t316672544\t1030,800000\t498,250000\t500,000000\r\n3271\t316673683\t1031,100000\t498,500000\t500,000000\r\n3272\t316674823\t1031,200000\t498,000000\t500,000000\r\n3273\t316675963\t1029,600000\t498,750000\t500,000000\r\n3274\t316677099\t1032,800000\t497,750000\t500,000000\r\n3275\t316678246\t1035,800000\t497,500000\t500,000000\r\n3276\t316679379\t1029,000000\t498,500000\t500,000000\r\n3277\t316680513\t1029,600000\t498,000000\t500,000000\r\n3278\t316681657\t1030,700000\t497,750000\t500,000000\r\n3279\t316682800\t1030,200000\t498,000000\t500,000000\r\n3280\t316683941\t1030,800000\t498,000000\t500,000000\r\n3281\t316685075\t1029,600000\t497,250000\t500,000000\r\n3282\t316686218\t1031,800000\t498,250000\t500,000000\r\n3283\t316687357\t1029,000000\t497,000000\t500,000000\r\n3284\t316688490\t1030,700000\t498,250000\t500,000000\r\n3285\t316689621\t1030,700000\t497,500000\t500,000000\r\n3286\t316690758\t1029,100000\t498,000000\t500,000000\r\n3287\t316691893\t1031,200000\t498,250000\t500,000000\r\n3288\t316693033\t1030,000000\t498,250000\t500,000000\r\n3289\t316694171\t1030,100000\t498,000000\t500,000000\r\n3290\t316695313\t1031,700000\t498,000000\t500,000000\r\n3291\t316696452\t1028,600000\t499,000000\t500,000000\r\n3292\t316697589\t1029,200000\t497,250000\t500,000000\r\n3293\t316698723\t1029,000000\t497,500000\t500,000000\r\n3294\t316699863\t1029,300000\t498,500000\t500,000000\r\n3295\t316700995\t1028,000000\t498,250000\t500,000000\r\n3296\t316702133\t1030,200000\t498,000000\t500,000000\r\n3297\t316703279\t1028,600000\t498,250000\t500,000000\r\n3298\t316704417\t1029,700000\t498,250000\t500,000000\r\n3299\t316705553\t1029,600000\t498,500000\t500,000000\r\n3300\t316706687\t1030,200000\t498,000000\t500,000000\r\n3301\t316707823\t1029,600000\t498,500000\t500,000000\r\n3302\t316708960\t1029,100000\t498,250000\t500,000000\r\n3303\t316710097\t1029,000000\t498,500000\t500,000000\r\n3304\t316711232\t1030,700000\t497,500000\t500,000000\r\n3305\t316712372\t1029,600000\t498,250000\t500,000000\r\n3306\t316713512\t1031,300000\t498,000000\t500,000000\r\n3307\t316714653\t1029,000000\t498,250000\t500,000000\r\n3308\t316715793\t1027,500000\t498,250000\t500,000000\r\n3309\t316716927\t1031,300000\t497,750000\t500,000000\r\n3310\t316718067\t1029,200000\t498,500000\t500,000000\r\n3311\t316719212\t1030,700000\t498,000000\t500,000000\r\n3312\t316720348\t1031,300000\t497,750000\t500,000000\r\n3313\t316721481\t1029,600000\t498,250000\t500,000000\r\n3314\t316722619\t1031,800000\t498,250000\t500,000000\r\n3315\t316723755\t1030,600000\t497,750000\t500,000000\r\n3316\t316724886\t1029,100000\t498,750000\t500,000000\r\n3317\t316726026\t1031,200000\t498,250000\t500,000000\r\n3318\t316727166\t1026,000000\t497,750000\t500,000000\r\n3319\t316728311\t1031,200000\t499,000000\t500,000000\r\n3320\t316729450\t1028,100000\t498,000000\t500,000000\r\n3321\t316730584\t1027,000000\t499,000000\t500,000000\r\n3322\t316731719\t1028,600000\t497,500000\t500,000000\r\n3323\t316732862\t1029,700000\t499,500000\t500,000000\r\n3324\t316734003\t1027,000000\t498,250000\t500,000000\r\n3325\t316735137\t1027,600000\t498,500000\t500,000000\r\n3326\t316736279\t1027,000000\t497,750000\t500,000000\r\n3327\t316737412\t1028,700000\t498,250000\t500,000000\r\n3328\t316738551\t1028,600000\t498,750000\t500,000000\r\n3329\t316739691\t1028,500000\t498,000000\t500,000000\r\n3330\t316740821\t1028,700000\t498,500000\t500,000000\r\n3331\t316741955\t1027,500000\t498,750000\t500,000000\r\n3332\t316743092\t1028,500000\t498,250000\t500,000000\r\n3333\t316744229\t1028,200000\t498,500000\t500,000000\r\n3334\t316745369\t1029,200000\t498,500000\t500,000000\r\n3335\t316746508\t1029,200000\t497,750000\t500,000000\r\n3336\t316747642\t1028,100000\t498,750000\t500,000000\r\n3337\t316748779\t1028,100000\t499,000000\t500,000000\r\n3338\t316749907\t1028,700000\t498,000000\t500,000000\r\n3339\t316751046\t1029,200000\t497,750000\t500,000000\r\n3340\t316752182\t1028,000000\t498,500000\t500,000000\r\n3341\t316753327\t1025,000000\t497,500000\t500,000000\r\n3342\t316754463\t1029,600000\t498,250000\t500,000000\r\n3343\t316755601\t1028,000000\t497,750000\t500,000000\r\n3344\t316756740\t1029,100000\t498,500000\t500,000000\r\n3345\t316757880\t1027,100000\t498,250000\t500,000000\r\n3346\t316759015\t1027,600000\t498,750000\t500,000000\r\n3347\t316760150\t1027,000000\t498,750000\t500,000000\r\n3348\t316761287\t1027,000000\t496,700000\t500,000000\r\n3349\t316762422\t1028,100000\t498,500000\t500,000000\r\n3350\t316763556\t1026,500000\t498,750000\t500,000000\r\n3351\t316764697\t1028,100000\t498,250000\t500,000000\r\n3352\t316765836\t1027,000000\t498,250000\t500,000000\r\n3353\t316766982\t1026,500000\t498,500000\t500,000000\r\n3354\t316768119\t1028,100000\t498,250000\t500,000000\r\n3355\t316769254\t1027,600000\t497,000000\t500,000000\r\n3356\t316770389\t1028,100000\t497,750000\t500,000000\r\n3357\t316771530\t1027,100000\t498,000000\t500,000000\r\n3358\t316772664\t1027,600000\t497,750000\t500,000000\r\n3359\t316773803\t1027,700000\t498,500000\t500,000000\r\n3360\t316774942\t1028,100000\t499,250000\t500,000000\r\n3361\t316776076\t1028,600000\t498,750000\t500,000000\r\n3362\t316777212\t1030,200000\t498,000000\t500,000000\r\n3363\t316778354\t1026,500000\t499,000000\t500,000000\r\n3364\t316779490\t1029,200000\t498,250000\t500,000000\r\n3365\t316780630\t1026,500000\t499,000000\t500,000000\r\n3366\t316781768\t1029,100000\t497,750000\t500,000000\r\n3367\t316782910\t1027,700000\t498,000000\t500,000000\r\n3368\t316784043\t1025,600000\t498,000000\t500,000000\r\n3369\t316785176\t1026,500000\t498,500000\t500,000000\r\n3370\t316786313\t1026,500000\t498,500000\t500,000000\r\n3371\t316787454\t1028,100000\t498,250000\t500,000000\r\n3372\t316788592\t1028,600000\t498,000000\t500,000000\r\n3373\t316789734\t1025,500000\t498,500000\t500,000000\r\n3374\t316790875\t1026,600000\t498,500000\t500,000000\r\n3375\t316792012\t1025,000000\t497,750000\t500,000000\r\n3376\t316793148\t1028,200000\t498,000000\t500,000000\r\n3377\t316794286\t1028,600000\t498,250000\t500,000000\r\n3378\t316795424\t1026,600000\t498,000000\t500,000000\r\n3379\t316796566\t1027,600000\t497,250000\t500,000000\r\n3380\t316797707\t1027,600000\t497,500000\t500,000000\r\n3381\t316798858\t1028,200000\t499,000000\t500,000000\r\n3382\t316799994\t1024,000000\t498,250000\t500,000000\r\n3383\t316801133\t1027,000000\t498,250000\t500,000000\r\n3384\t316802269\t1027,100000\t497,750000\t500,000000\r\n3385\t316803419\t1029,200000\t497,250000\t500,000000\r\n3386\t316804554\t1027,100000\t497,750000\t500,000000\r\n3387\t316805692\t1027,600000\t497,450000\t500,000000\r\n3388\t316806831\t1026,100000\t498,000000\t500,000000\r\n3389\t316807968\t1027,700000\t497,750000\t500,000000\r\n3390\t316809104\t1026,500000\t499,000000\t500,000000\r\n3391\t316810246\t1027,000000\t498,250000\t500,000000\r\n3392\t316811377\t1030,200000\t498,250000\t500,000000\r\n3393\t316812520\t1026,100000\t498,000000\t500,000000\r\n3394\t316813659\t1028,100000\t498,750000\t500,000000\r\n3395\t316814787\t1025,500000\t498,000000\t500,000000\r\n3396\t316815925\t1025,500000\t497,750000\t500,000000\r\n3397\t316817064\t1027,100000\t498,250000\t500,000000\r\n3398\t316818203\t1027,000000\t498,500000\t500,000000\r\n3399\t316819341\t1023,600000\t499,250000\t500,000000\r\n3400\t316820480\t1025,000000\t498,500000\t500,000000\r\n3401\t316821612\t1025,000000\t498,500000\t500,000000\r\n3402\t316822745\t1024,500000\t498,750000\t500,000000\r\n3403\t316823879\t1026,600000\t497,750000\t500,000000\r\n3404\t316825018\t1025,500000\t499,750000\t500,000000\r\n3405\t316826153\t1028,200000\t498,750000\t500,000000\r\n3406\t316827290\t1026,000000\t497,500000\t500,000000\r\n3407\t316828422\t1023,000000\t498,250000\t500,000000\r\n3408\t316829562\t1024,500000\t498,250000\t500,000000\r\n3409\t316830703\t1025,500000\t498,500000\t500,000000\r\n3410\t316831840\t1025,500000\t498,250000\t500,000000\r\n3411\t316832980\t1025,500000\t498,000000\t500,000000\r\n3412\t316834121\t1025,500000\t498,000000\t500,000000\r\n3413\t316835262\t1027,100000\t498,500000\t500,000000\r\n3414\t316836393\t1024,000000\t498,250000\t500,000000\r\n3415\t316837535\t1029,200000\t498,000000\t500,000000\r\n3416\t316838669\t1024,600000\t498,250000\t500,000000\r\n3417\t316839805\t1024,600000\t497,750000\t500,000000\r\n3418\t316840945\t1025,000000\t497,750000\t500,000000\r\n3419\t316842080\t1025,000000\t498,500000\t500,000000\r\n3420\t316843224\t1023,600000\t498,000000\t500,000000\r\n3421\t316844358\t1026,500000\t497,750000\t500,000000\r\n3422\t316845500\t1025,000000\t497,250000\t500,000000\r\n3423\t316846641\t1026,500000\t497,500000\t500,000000\r\n3424\t316847779\t1024,500000\t498,000000\t500,000000\r\n3425\t316848911\t1023,500000\t498,000000\t500,000000\r\n3426\t316850046\t1023,000000\t498,750000\t500,000000\r\n3427\t316851181\t1027,200000\t497,750000\t500,000000\r\n3428\t316852319\t1023,500000\t499,750000\t500,000000\r\n3429\t316853459\t1024,500000\t497,250000\t500,000000\r\n3430\t316854593\t1024,000000\t498,250000\t500,000000\r\n3431\t316855731\t1026,500000\t497,500000\t500,000000\r\n3432\t316856867\t1024,600000\t498,250000\t500,000000\r\n3433\t316858004\t1024,500000\t499,000000\t500,000000\r\n3434\t316859139\t1028,700000\t498,500000\t500,000000\r\n3435\t316860278\t1025,000000\t498,500000\t500,000000\r\n3436\t316861415\t1025,500000\t497,250000\t500,000000\r\n3437\t316862553\t1025,000000\t497,500000\t500,000000\r\n3438\t316863693\t1025,500000\t497,750000\t500,000000\r\n3439\t316864842\t1025,500000\t497,250000\t500,000000\r\n3440\t316865976\t1026,600000\t498,250000\t500,000000\r\n3441\t316867115\t1023,000000\t498,750000\t500,000000\r\n3442\t316868254\t1025,000000\t498,000000\t500,000000\r\n3443\t316869390\t1026,100000\t498,000000\t500,000000\r\n3444\t316870513\t1024,500000\t497,500000\t500,000000\r\n3445\t316871638\t1023,500000\t497,500000\t500,000000\r\n3446\t316872773\t1024,500000\t497,500000\t500,000000\r\n3447\t316873909\t1025,000000\t498,750000\t500,000000\r\n3448\t316875050\t1024,000000\t498,250000\t500,000000\r\n3449\t316876188\t1025,100000\t499,000000\t500,000000\r\n3450\t316877334\t1022,000000\t497,750000\t500,000000\r\n3451\t316878473\t1025,100000\t497,750000\t500,000000\r\n3452\t316879611\t1022,000000\t498,500000\t500,000000\r\n3453\t316880753\t1024,000000\t497,500000\t500,000000\r\n3454\t316881891\t1022,500000\t497,750000\t500,000000\r\n3455\t316883035\t1025,100000\t498,500000\t500,000000\r\n3456\t316884173\t1024,100000\t498,000000\t500,000000\r\n3457\t316885312\t1023,100000\t498,750000\t500,000000\r\n3458\t316886450\t1023,500000\t498,750000\t500,000000\r\n3459\t316887592\t1026,100000\t498,500000\t500,000000\r\n3460\t316888727\t1023,600000\t498,500000\t500,000000\r\n3461\t316889867\t1023,000000\t497,500000\t500,000000\r\n3462\t316891006\t1023,600000\t498,750000\t500,000000\r\n3463\t316892137\t1024,000000\t498,000000\t500,000000\r\n3464\t316893269\t1023,000000\t498,000000\t500,000000\r\n3465\t316894406\t1022,500000\t497,750000\t500,000000\r\n3466\t316895545\t1026,100000\t497,500000\t500,000000\r\n3467\t316896680\t1022,500000\t497,250000\t500,000000\r\n3468\t316897820\t1023,000000\t498,500000\t500,000000\r\n3469\t316898952\t1023,000000\t496,950000\t500,000000\r\n3470\t316900085\t1024,000000\t499,500000\t500,000000\r\n3471\t316901219\t1024,500000\t498,000000\t500,000000\r\n3472\t316902356\t1022,000000\t498,500000\t500,000000\r\n3473\t316903497\t1023,500000\t497,750000\t500,000000\r\n3474\t316904632\t1023,500000\t498,000000\t500,000000\r\n3475\t316905767\t1025,600000\t497,500000\t500,000000\r\n3476\t316906902\t1024,500000\t498,250000\t500,000000\r\n3477\t316908037\t1025,500000\t497,750000\t500,000000\r\n3478\t316909169\t1021,500000\t498,750000\t500,000000\r\n3479\t316910298\t1024,000000\t497,750000\t500,000000\r\n3480\t316911429\t1022,500000\t498,750000\t500,000000\r\n3481\t316912666\t1022,500000\t498,000000\t500,000000\r\n3482\t316914355\t1020,500000\t498,250000\t500,000000\r\n3483\t316916049\t1023,500000\t498,500000\t500,000000\r\n3484\t316917745\t1021,500000\t498,250000\t500,000000\r\n3485\t316919441\t1022,500000\t497,500000\t500,000000\r\n3486\t316921067\t1020,000000\t498,500000\t500,000000\r\n3487\t316922615\t1023,100000\t499,250000\t500,000000\r\n3488\t316924152\t1024,000000\t498,250000\t500,000000\r\n3489\t316925639\t1021,500000\t498,750000\t500,000000\r\n3490\t316927201\t1023,000000\t498,250000\t500,000000\r\n3491\t316928764\t1023,000000\t497,500000\t500,000000\r\n3492\t316930302\t1022,000000\t498,500000\t500,000000\r\n3493\t316931867\t1022,000000\t498,500000\t500,000000\r\n3494\t316933337\t1023,600000\t498,500000\t500,000000\r\n3495\t316934889\t1022,500000\t498,000000\t500,000000\r\n3496\t316936435\t1024,100000\t498,000000\t500,000000\r\n3497\t316937922\t1022,000000\t498,500000\t500,000000\r\n3498\t316939462\t1020,500000\t498,750000\t500,000000\r\n3499\t316940982\t1021,000000\t498,000000\t500,000000\r\n3500\t316942478\t1019,500000\t498,250000\t500,000000\r\n3501\t316944036\t1021,000000\t498,000000\t500,000000\r\n3502\t316945504\t1025,000000\t498,250000\t500,000000\r\n3503\t316947049\t1023,500000\t497,750000\t500,000000\r\n3504\t316948533\t1021,500000\t497,750000\t500,000000\r\n3505\t316950056\t1023,600000\t498,250000\t500,000000\r\n3506\t316951607\t1021,500000\t498,250000\t500,000000\r\n3507\t316953120\t1023,000000\t497,750000\t500,000000\r\n3508\t316954607\t1021,500000\t498,500000\t500,000000\r\n3509\t316956095\t1021,500000\t497,750000\t500,000000\r\n3510\t316957597\t1021,000000\t498,250000\t500,000000\r\n3511\t316959149\t1023,600000\t498,250000\t500,000000\r\n3512\t316960733\t1022,500000\t498,000000\t500,000000\r\n3513\t316962255\t1019,000000\t498,250000\t500,000000\r\n3514\t316963743\t1022,600000\t498,000000\t500,000000\r\n3515\t316965307\t1019,000000\t498,250000\t500,000000\r\n3516\t316966816\t1019,000000\t498,750000\t500,000000\r\n3517\t316968296\t1019,500000\t498,250000\t500,000000\r\n3518\t316969858\t1020,500000\t498,750000\t500,000000\r\n3519\t316971392\t1022,000000\t497,500000\t500,000000\r\n3520\t316972879\t1020,500000\t498,250000\t500,000000\r\n3521\t316974402\t1018,500000\t498,250000\t500,000000\r\n3522\t316975952\t1019,500000\t498,000000\t500,000000\r\n3523\t316977440\t1021,500000\t498,500000\t500,000000\r\n3524\t316978983\t1019,500000\t497,500000\t500,000000\r\n3525\t316980546\t1019,500000\t497,750000\t500,000000\r\n3526\t316982034\t1021,000000\t498,750000\t500,000000\r\n3527\t316983545\t1021,000000\t497,500000\t500,000000\r\n3528\t316985119\t1020,500000\t497,250000\t500,000000\r\n3529\t316986681\t1018,500000\t498,500000\t500,000000\r\n3530\t316988213\t1021,600000\t498,000000\t500,000000\r\n3531\t316989679\t1021,000000\t498,250000\t500,000000\r\n3532\t316991213\t1019,000000\t497,750000\t500,000000\r\n3533\t316992775\t1019,500000\t498,250000\t500,000000\r\n3534\t316994327\t1020,000000\t498,250000\t500,000000\r\n3535\t316995867\t1021,000000\t498,250000\t500,000000\r\n3536\t316997338\t1019,000000\t497,500000\t500,000000\r\n3537\t316998879\t1020,000000\t497,750000\t500,000000\r\n3538\t317000473\t1020,500000\t499,000000\t500,000000\r\n3539\t317002035\t1021,000000\t498,000000\t500,000000\r\n3540\t317003576\t1019,500000\t498,000000\t500,000000\r\n3541\t317005047\t1020,500000\t497,750000\t500,000000\r\n3542\t317006588\t1019,500000\t499,250000\t500,000000\r\n3543\t317008161\t1020,000000\t498,250000\t500,000000\r\n3544\t317009683\t1019,000000\t498,250000\t500,000000\r\n3545\t317011171\t1018,500000\t497,200000\t500,000000\r\n3546\t317012692\t1020,000000\t498,000000\t500,000000\r\n3547\t317014160\t1020,000000\t498,750000\t500,000000\r\n3548\t317015692\t1019,000000\t498,250000\t500,000000\r\n3549\t317017265\t1019,000000\t498,500000\t500,000000\r\n3550\t317018838\t1019,000000\t498,250000\t500,000000\r\n3551\t317020401\t1015,500000\t497,750000\t500,000000\r\n3552\t317021918\t1019,500000\t497,500000\t500,000000\r\n3553\t317023414\t1019,500000\t499,000000\t500,000000\r\n3554\t317024973\t1017,500000\t498,250000\t500,000000\r\n3555\t317026557\t1017,500000\t497,750000\t500,000000\r\n3556\t317028109\t1017,500000\t498,000000\t500,000000\r\n3557\t317029666\t1020,500000\t498,000000\t500,000000\r\n3558\t317031191\t1020,000000\t497,500000\t500,000000\r\n3559\t317032713\t1019,500000\t497,750000\t500,000000\r\n3560\t317034297\t1020,000000\t498,250000\t500,000000\r\n3561\t317035827\t1018,500000\t498,500000\t500,000000\r\n3562\t317037373\t1019,000000\t498,000000\t500,000000\r\n3563\t317038847\t1018,500000\t497,750000\t500,000000\r\n3564\t317040401\t1019,000000\t497,250000\t500,000000\r\n3565\t317041879\t1018,000000\t497,750000\t500,000000\r\n3566\t317043411\t1018,000000\t498,500000\t500,000000\r\n3567\t317044973\t1017,500000\t498,500000\t500,000000\r\n3568\t317046474\t1016,500000\t498,500000\t500,000000\r\n3569\t317047978\t1018,500000\t497,750000\t500,000000\r\n3570\t317049546\t1018,000000\t498,000000\t500,000000\r\n3571\t317051117\t1017,500000\t498,000000\t500,000000\r\n3572\t317052692\t1017,500000\t499,250000\t500,000000\r\n3573\t317054243\t1016,500000\t497,450000\t500,000000\r\n3574\t317055789\t1016,000000\t499,000000\t500,000000\r\n3575\t317057305\t1018,000000\t498,000000\t500,000000\r\n3576\t317058810\t1020,000000\t498,250000\t500,000000\r\n3577\t317060296\t1015,000000\t498,250000\t500,000000\r\n3578\t317061847\t1017,000000\t498,500000\t500,000000\r\n3579\t317063395\t1017,500000\t498,250000\t500,000000\r\n3580\t317064900\t1015,500000\t497,500000\t500,000000\r\n3581\t317066437\t1016,000000\t497,750000\t500,000000\r\n3582\t317067910\t1019,500000\t498,000000\t500,000000\r\n3583\t317069412\t1017,000000\t498,250000\t500,000000\r\n3584\t317070931\t1017,000000\t497,750000\t500,000000\r\n3585\t317072441\t1016,000000\t499,000000\t500,000000\r\n3586\t317074004\t1015,000000\t498,500000\t500,000000\r\n3587\t317075512\t1016,000000\t498,750000\t500,000000\r\n3588\t317077015\t1015,500000\t497,450000\t500,000000\r\n3589\t317078535\t1018,000000\t497,000000\t500,000000\r\n3590\t317080036\t1015,500000\t498,000000\t500,000000\r\n3591\t317081598\t1017,000000\t498,000000\t500,000000\r\n3592\t317083150\t1017,000000\t498,250000\t500,000000\r\n3593\t317084703\t1014,000000\t498,250000\t500,000000\r\n3594\t317086286\t1017,000000\t498,250000\t500,000000\r\n3595\t317087810\t1016,000000\t498,000000\t500,000000\r\n3596\t317089316\t1015,500000\t498,250000\t500,000000\r\n3597\t317090880\t1016,500000\t498,000000\t500,000000\r\n3598\t317092452\t1014,000000\t498,750000\t500,000000\r\n3599\t317094025\t1015,000000\t497,750000\t500,000000\r\n3600\t317095538\t1016,500000\t497,750000\t500,000000\r\n3601\t317097025\t1014,000000\t499,000000\t500,000000\r\n3602\t317098557\t1015,000000\t498,500000\t500,000000\r\n3603\t317100056\t1017,500000\t498,500000\t500,000000\r\n3604\t317101630\t1012,500000\t498,250000\t500,000000\r\n3605\t317103107\t1015,500000\t498,750000\t500,000000\r\n3606\t317104639\t1016,500000\t498,750000\t500,000000\r\n3607\t317106118\t1016,500000\t497,200000\t500,000000\r\n3608\t317107586\t1013,500000\t498,500000\t500,000000\r\n3609\t317109046\t1014,500000\t497,750000\t500,000000\r\n3610\t317110604\t1016,000000\t497,750000\t500,000000\r\n3611\t317112166\t1016,000000\t499,250000\t500,000000\r\n3612\t317113683\t1015,500000\t498,500000\t500,000000\r\n3613\t317115170\t1015,500000\t497,500000\t500,000000\r\n3614\t317116703\t1014,500000\t497,500000\t500,000000\r\n3615\t317118245\t1016,000000\t498,000000\t500,000000\r\n3616\t317119722\t1013,500000\t498,250000\t500,000000\r\n3617\t317121276\t1013,500000\t497,500000\t500,000000\r\n3618\t317122783\t1013,500000\t498,250000\t500,000000\r\n3619\t317124297\t1014,500000\t498,000000\t500,000000\r\n3620\t317125849\t1015,500000\t498,500000\t500,000000\r\n3621\t317127369\t1017,000000\t498,000000\t500,000000\r\n3622\t317128869\t1016,500000\t498,000000\t500,000000\r\n3623\t317130399\t1014,500000\t497,500000\t500,000000\r\n3624\t317131869\t1014,000000\t497,750000\t500,000000\r\n3625\t317133400\t1015,500000\t499,000000\t500,000000\r\n3626\t317134949\t1014,000000\t498,250000\t500,000000\r\n3627\t317136420\t1012,500000\t498,000000\t500,000000\r\n3628\t317137922\t1015,000000\t497,750000\t500,000000\r\n3629\t317139399\t1015,500000\t498,250000\t500,000000\r\n3630\t317140921\t1014,500000\t498,000000\t500,000000\r\n3631\t317142474\t1015,000000\t498,250000\t500,000000\r\n3632\t317143971\t1012,500000\t498,750000\t500,000000\r\n3633\t317145442\t1014,000000\t497,750000\t500,000000\r\n3634\t317146966\t1013,500000\t498,750000\t500,000000\r\n3635\t317148452\t1014,500000\t498,250000\t500,000000\r\n3636\t317149940\t1014,500000\t498,000000\t500,000000\r\n3637\t317151453\t1012,500000\t498,000000\t500,000000\r\n3638\t317152941\t1011,000000\t498,500000\t500,000000\r\n3639\t317154431\t1012,500000\t498,750000\t500,000000\r\n3640\t317156005\t1015,500000\t497,700000\t500,000000\r\n3641\t317157587\t1012,500000\t499,250000\t500,000000\r\n3642\t317159097\t1013,500000\t497,250000\t500,000000\r\n3643\t317160587\t1010,500000\t499,750000\t500,000000\r\n3644\t317162140\t1014,500000\t499,250000\t500,000000\r\n3645\t317163702\t1012,500000\t497,750000\t500,000000\r\n3646\t317165286\t1012,000000\t498,250000\t500,000000\r\n3647\t317166767\t1014,500000\t498,500000\t500,000000\r\n3648\t317167902\t1013,000000\t497,750000\t500,000000\r\n3649\t317169039\t1011,500000\t497,500000\t500,000000\r\n3650\t317170176\t1012,500000\t498,000000\t500,000000\r\n3651\t317171316\t1014,000000\t497,750000\t500,000000\r\n3652\t317172744\t1011,500000\t498,500000\t500,000000\r\n3653\t317174232\t1011,000000\t498,500000\t500,000000\r\n3654\t317175766\t1012,500000\t498,250000\t500,000000\r\n3655\t317177245\t1009,000000\t498,000000\t500,000000\r\n3656\t317178796\t1013,000000\t497,750000\t500,000000\r\n3657\t317180349\t1013,500000\t498,500000\t500,000000\r\n3658\t317181866\t1010,500000\t498,500000\t500,000000\r\n3659\t317183380\t1013,000000\t498,000000\t500,000000\r\n3660\t317184943\t1013,000000\t497,750000\t500,000000\r\n3661\t317186520\t1013,000000\t497,500000\t500,000000\r\n3662\t317188109\t1010,500000\t498,750000\t500,000000\r\n3663\t317189669\t1012,500000\t497,250000\t500,000000\r\n3664\t317191255\t1010,500000\t498,000000\t500,000000\r\n3665\t317192816\t1010,000000\t497,750000\t500,000000\r\n3666\t317194391\t1010,000000\t497,500000\t500,000000\r\n3667\t317195984\t1011,500000\t498,500000\t500,000000\r\n3668\t317197547\t1010,000000\t497,750000\t500,000000\r\n3669\t317199130\t1009,000000\t495,950000\t500,000000\r\n3670\t317200608\t1011,500000\t496,950000\t500,000000\r\n3671\t317202110\t1008,500000\t498,250000\t500,000000\r\n3672\t317203622\t1011,500000\t497,700000\t500,000000\r\n3673\t317205087\t1012,500000\t498,500000\t500,000000\r\n3674\t317206660\t1013,000000\t498,750000\t500,000000\r\n3675\t317208204\t1012,000000\t498,500000\t500,000000\r\n3676\t317209680\t1010,500000\t497,250000\t500,000000\r\n3677\t317211213\t1015,000000\t498,500000\t500,000000\r\n3678\t317212742\t1010,000000\t497,750000\t500,000000\r\n3679\t317214222\t1011,000000\t497,750000\t500,000000\r\n3680\t317215734\t1010,500000\t497,750000\t500,000000\r\n3681\t317217277\t1010,000000\t498,500000\t500,000000\r\n3682\t317218785\t1009,500000\t497,500000\t500,000000\r\n3683\t317220285\t1010,500000\t497,500000\t500,000000\r\n3684\t317221839\t1010,500000\t497,500000\t500,000000\r\n3685\t317223400\t1012,500000\t497,450000\t500,000000\r\n3686\t317224879\t1009,000000\t498,250000\t500,000000\r\n3687\t317226441\t1008,000000\t498,000000\t500,000000\r\n3688\t317228003\t1009,000000\t498,500000\t500,000000\r\n3689\t317229538\t1009,500000\t498,000000\t500,000000\r\n3690\t317231025\t1011,500000\t497,750000\t500,000000\r\n3691\t317232579\t1010,000000\t497,750000\t500,000000\r\n3692\t317234046\t1012,000000\t498,500000\t500,000000\r\n3693\t317235603\t1011,000000\t498,750000\t500,000000\r\n3694\t317237182\t1011,000000\t497,750000\t500,000000\r\n3695\t317238695\t1010,500000\t497,500000\t500,000000\r\n3696\t317240202\t1010,000000\t498,000000\t500,000000\r\n3697\t317241745\t1011,000000\t497,750000\t500,000000\r\n3698\t317243327\t1008,000000\t496,700000\t500,000000\r\n3699\t317244840\t1009,500000\t497,750000\t500,000000\r\n3700\t317246328\t1009,000000\t498,250000\t500,000000\r\n3701\t317247890\t1011,500000\t499,000000\t500,000000\r\n3702\t317249369\t1008,500000\t498,250000\t500,000000\r\n3703\t317250911\t1010,500000\t499,250000\t500,000000\r\n3704\t317252453\t1011,000000\t498,500000\t500,000000\r\n3705\t317254036\t1010,000000\t498,250000\t500,000000\r\n3706\t317255576\t1008,500000\t497,000000\t500,000000\r\n3707\t317257047\t1006,500000\t497,500000\t500,000000\r\n3708\t317258578\t1008,500000\t498,750000\t500,000000\r\n3709\t317260097\t1009,000000\t498,500000\t500,000000\r\n3710\t317261599\t1008,000000\t498,250000\t500,000000\r\n3711\t317263129\t1010,000000\t498,500000\t500,000000\r\n3712\t317264693\t1009,000000\t498,500000\t500,000000\r\n3713\t317266203\t1009,000000\t498,250000\t500,000000\r\n3714\t317267691\t1011,000000\t498,000000\t500,000000\r\n3715\t317269244\t1009,500000\t497,750000\t500,000000\r\n3716\t317270797\t1009,000000\t498,500000\t500,000000\r\n3717\t317272306\t1009,000000\t498,750000\t500,000000\r\n3718\t317273807\t1007,500000\t497,750000\t500,000000\r\n3719\t317275370\t1006,500000\t499,000000\t500,000000\r\n3720\t317276931\t1011,000000\t498,500000\t500,000000\r\n3721\t317278494\t1009,500000\t498,500000\t500,000000\r\n3722\t317280057\t1010,000000\t498,750000\t500,000000\r\n3723\t317281609\t1011,000000\t497,750000\t500,000000\r\n3724\t317283181\t1008,000000\t499,000000\t500,000000\r\n3725\t317284670\t1007,500000\t498,250000\t500,000000\r\n3726\t317286212\t1008,000000\t497,750000\t500,000000\r\n3727\t317287786\t1009,000000\t498,250000\t500,000000\r\n3728\t317289339\t1008,000000\t498,750000\t500,000000\r\n3729\t317290921\t1008,000000\t498,500000\t500,000000\r\n3730\t317292494\t1009,000000\t497,750000\t500,000000\r\n3731\t317294077\t1008,500000\t498,250000\t500,000000\r\n3732\t317295546\t1008,500000\t497,500000\t500,000000\r\n3733\t317297066\t1012,000000\t497,750000\t500,000000\r\n3734\t317298641\t1007,000000\t498,250000\t500,000000\r\n3735\t317300203\t1006,500000\t498,750000\t500,000000\r\n3736\t317301776\t1007,000000\t497,750000\t500,000000\r\n3737\t317303323\t1007,000000\t498,250000\t500,000000\r\n3738\t317304795\t1009,000000\t498,250000\t500,000000\r\n3739\t317306337\t1006,500000\t497,750000\t500,000000\r\n3740\t317307890\t1008,500000\t497,750000\t500,000000\r\n3741\t317309483\t1007,500000\t497,250000\t500,000000\r\n3742\t317311057\t1010,500000\t498,250000\t500,000000\r\n3743\t317312588\t1008,500000\t497,750000\t500,000000\r\n3744\t317314056\t1007,000000\t497,950000\t500,000000\r\n3745\t317315618\t1009,000000\t498,250000\t500,000000\r\n3746\t317317165\t1008,000000\t498,750000\t500,000000\r\n3747\t317318641\t1010,000000\t497,750000\t500,000000\r\n3748\t317320181\t1007,500000\t497,750000\t500,000000\r\n3749\t317321735\t1007,000000\t497,500000\t500,000000\r\n3750\t317323236\t1010,000000\t498,750000\t500,000000\r\n3751\t317324713\t1006,500000\t498,500000\t500,000000\r\n3752\t317326201\t1007,500000\t498,250000\t500,000000\r\n3753\t317327713\t1006,500000\t497,750000\t500,000000\r\n3754\t317329276\t1006,000000\t497,750000\t500,000000\r\n3755\t317330849\t1009,000000\t498,250000\t500,000000\r\n3756\t317332412\t1005,000000\t498,000000\t500,000000\r\n3757\t317333953\t1006,000000\t498,250000\t500,000000\r\n3758\t317335450\t1004,500000\t498,000000\t500,000000\r\n3759\t317336951\t1009,000000\t498,500000\t500,000000\r\n3760\t317338505\t1007,000000\t498,250000\t500,000000\r\n3761\t317340047\t1006,500000\t498,250000\t500,000000\r\n3762\t317341566\t1007,500000\t498,000000\t500,000000\r\n3763\t317343057\t1005,500000\t498,500000\t500,000000\r\n3764\t317344619\t1007,500000\t498,250000\t500,000000\r\n3765\t317346171\t1005,500000\t498,500000\t500,000000\r\n3766\t317347735\t1009,500000\t498,250000\t500,000000\r\n3767\t317349244\t1008,000000\t498,500000\t500,000000\r\n3768\t317350757\t1005,000000\t498,250000\t500,000000\r\n3769\t317352318\t1005,500000\t498,250000\t500,000000\r\n3770\t317353800\t1008,000000\t498,500000\t500,000000\r\n3771\t317355319\t1008,500000\t498,250000\t500,000000\r\n3772\t317356816\t1007,000000\t497,750000\t500,000000\r\n3773\t317358329\t1005,000000\t498,500000\t500,000000\r\n3774\t317359855\t1008,500000\t498,500000\t500,000000\r\n3775\t317361339\t1006,500000\t497,200000\t500,000000\r\n3776\t317362916\t1006,500000\t498,000000\t500,000000\r\n3777\t317364464\t1004,500000\t498,000000\t500,000000\r\n3778\t317365942\t1005,000000\t499,000000\t500,000000\r\n3779\t317367485\t1007,500000\t497,750000\t500,000000\r\n3780\t317369019\t1006,000000\t496,950000\t500,000000\r\n3781\t317370536\t1003,500000\t497,500000\t500,000000\r\n3782\t317372088\t1005,500000\t498,000000\t500,000000\r\n3783\t317373568\t1005,000000\t497,250000\t500,000000\r\n3784\t317375078\t1005,500000\t497,450000\t500,000000\r\n3785\t317376661\t1004,500000\t497,750000\t500,000000\r\n3786\t317378159\t1005,000000\t498,250000\t500,000000\r\n3787\t317379671\t1002,500000\t497,750000\t500,000000\r\n3788\t317381244\t1007,000000\t498,750000\t500,000000\r\n3789\t317382744\t1004,500000\t497,750000\t500,000000\r\n3790\t317384223\t1007,000000\t498,250000\t500,000000\r\n3791\t317385785\t1006,500000\t497,200000\t500,000000\r\n3792\t317387308\t1003,500000\t497,750000\t500,000000\r\n3793\t317388776\t1004,500000\t498,000000\t500,000000\r\n3794\t317390339\t1004,500000\t497,250000\t500,000000\r\n3795\t317391849\t1004,000000\t498,250000\t500,000000\r\n3796\t317393370\t1006,500000\t498,000000\t500,000000\r\n3797\t317394921\t1006,500000\t497,750000\t500,000000\r\n3798\t317396494\t1005,500000\t498,750000\t500,000000\r\n3799\t317398004\t1005,500000\t497,500000\t500,000000\r\n3800\t317399494\t1005,000000\t498,500000\t500,000000\r\n3801\t317401046\t1004,000000\t499,750000\t500,000000\r\n3802\t317402629\t1003,500000\t498,250000\t500,000000\r\n3803\t317404182\t1005,000000\t497,750000\t500,000000\r\n3804\t317405671\t1006,000000\t498,000000\t500,000000\r\n3805\t317407229\t1006,000000\t497,250000\t500,000000\r\n3806\t317408796\t1004,500000\t497,500000\t500,000000\r\n3807\t317410316\t1005,500000\t498,500000\t500,000000\r\n3808\t317411828\t1006,000000\t498,250000\t500,000000\r\n3809\t317413420\t1004,000000\t498,000000\t500,000000\r\n3810\t317414979\t1003,000000\t497,750000\t500,000000\r\n3811\t317416558\t1006,000000\t498,000000\t500,000000\r\n3812\t317418056\t1003,000000\t498,000000\t500,000000\r\n3813\t317419568\t1003,000000\t498,500000\t500,000000\r\n3814\t317421107\t1003,500000\t498,000000\t500,000000\r\n3815\t317422577\t1003,000000\t497,750000\t500,000000\r\n3816\t317424098\t1003,000000\t498,500000\t500,000000\r\n3817\t317425638\t1005,500000\t498,250000\t500,000000\r\n3818\t317427109\t1005,500000\t498,500000\t500,000000\r\n3819\t317428632\t1004,000000\t498,750000\t500,000000\r\n3820\t317430187\t1002,500000\t498,250000\t500,000000\r\n3821\t317431702\t1004,500000\t498,000000\t500,000000\r\n3822\t317433234\t1004,000000\t498,500000\t500,000000\r\n3823\t317434818\t1003,500000\t498,000000\t500,000000\r\n3824\t317436295\t1001,500000\t498,750000\t500,000000\r\n3825\t317437833\t1003,000000\t498,250000\t500,000000\r\n3826\t317439400\t1002,500000\t497,250000\t500,000000\r\n3827\t317440959\t1002,500000\t500,250000\t500,000000\r\n3828\t317442380\t1004,000000\t498,500000\t500,000000\r\n3829\t317443775\t1002,000000\t498,500000\t500,000000\r\n3830\t317445128\t1002,500000\t497,750000\t500,000000\r\n3831\t317446266\t1002,500000\t498,000000\t500,000000\r\n3832\t317447401\t1004,000000\t497,250000\t500,000000\r\n3833\t317448542\t1004,000000\t498,000000\t500,000000\r\n3834\t317449676\t1004,000000\t498,250000\t500,000000\r\n3835\t317450812\t1002,000000\t498,750000\t500,000000\r\n3836\t317451945\t1000,500000\t497,500000\t500,000000\r\n3837\t317453080\t1003,000000\t497,500000\t500,000000\r\n3838\t317454210\t1004,500000\t497,500000\t500,000000\r\n3839\t317455350\t1002,500000\t496,750000\t500,000000\r\n3840\t317456488\t1001,000000\t498,250000\t500,000000\r\n3841\t317457628\t1002,500000\t497,750000\t500,000000\r\n3842\t317458765\t1006,000000\t498,250000\t500,000000\r\n3843\t317459903\t1002,500000\t498,250000\t500,000000\r\n3844\t317461040\t1002,500000\t497,750000\t500,000000\r\n3845\t317462172\t1002,000000\t498,500000\t500,000000\r\n3846\t317463308\t1001,500000\t498,000000\t500,000000\r\n3847\t317464441\t1001,500000\t498,250000\t500,000000\r\n3848\t317465573\t1000,000000\t498,250000\t500,000000\r\n3849\t317466705\t1003,000000\t498,000000\t500,000000\r\n3850\t317467837\t1002,500000\t498,250000\t500,000000\r\n3851\t317469411\t1001,000000\t498,500000\t500,000000\r\n3852\t317470964\t1001,500000\t497,250000\t500,000000\r\n3853\t317472527\t1000,000000\t498,500000\t500,000000\r\n3854\t317473995\t1004,500000\t498,000000\t500,000000\r\n3855\t317475627\t1001,000000\t497,700000\t500,000000\r\n3856\t317477325\t1001,000000\t498,000000\t500,000000\r\n3857\t317479014\t1002,500000\t499,000000\t500,000000\r\n3858\t317480705\t1001,500000\t498,000000\t500,000000\r\n3859\t317482403\t1000,500000\t497,750000\t500,000000\r\n3860\t317484094\t1002,000000\t498,750000\t500,000000\r\n3861\t317485787\t1000,000000\t497,500000\t500,000000\r\n3862\t317487484\t999,500000\t497,750000\t500,000000\r\n3863\t317489186\t1000,500000\t498,000000\t500,000000\r\n3864\t317490891\t1001,000000\t498,250000\t500,000000\r\n3865\t317492587\t1000,500000\t498,000000\t500,000000\r\n3866\t317494283\t1000,000000\t497,250000\t500,000000\r\n3867\t317495978\t999,000000\t497,750000\t500,000000\r\n3868\t317497674\t1001,500000\t497,750000\t500,000000\r\n3869\t317499295\t1001,000000\t499,000000\t500,000000\r\n3870\t317500839\t1000,500000\t497,500000\t500,000000\r\n3871\t317502403\t1001,000000\t498,250000\t500,000000\r\n3872\t317503901\t1002,000000\t498,250000\t500,000000\r\n3873\t317505422\t998,500000\t497,200000\t500,000000\r\n3874\t317506984\t999,500000\t497,500000\t500,000000\r\n3875\t317508536\t1003,500000\t499,500000\t500,000000\r\n3876\t317510005\t999,500000\t497,750000\t500,000000\r\n3877\t317511561\t999,500000\t497,250000\t500,000000\r\n3878\t317513088\t999,000000\t498,250000\t500,000000\r\n3879\t317514583\t999,500000\t497,750000\t500,000000\r\n3880\t317516161\t1000,000000\t497,750000\t500,000000\r\n3881\t317517801\t997,500000\t497,500000\t500,000000\r\n3882\t317519507\t999,500000\t498,750000\t500,000000\r\n3883\t317521210\t1000,500000\t498,750000\t500,000000\r\n3884\t317522913\t998,500000\t498,500000\t500,000000\r\n3885\t317524622\t1000,000000\t499,000000\t500,000000\r\n3886\t317526328\t997,000000\t498,750000\t500,000000\r\n3887\t317528033\t997,500000\t497,500000\t500,000000\r\n3888\t317529731\t998,500000\t497,250000\t500,000000\r\n3889\t317531437\t999,500000\t498,500000\t500,000000\r\n3890\t317533139\t999,500000\t498,250000\t500,000000\r\n3891\t317534838\t999,500000\t498,250000\t500,000000\r\n3892\t317536539\t1001,500000\t499,250000\t500,000000\r\n3893\t317538246\t995,900000\t498,250000\t500,000000\r\n3894\t317539947\t998,500000\t498,000000\t500,000000\r\n3895\t317541649\t999,000000\t498,000000\t500,000000\r\n3896\t317543353\t997,500000\t498,250000\t500,000000\r\n3897\t317545055\t996,500000\t497,750000\t500,000000\r\n3898\t317546759\t998,500000\t497,750000\t500,000000\r\n3899\t317548458\t998,000000\t497,250000\t500,000000\r\n3900\t317550150\t997,500000\t498,250000\t500,000000\r\n3901\t317551847\t1000,000000\t497,250000\t500,000000\r\n3902\t317553543\t998,500000\t498,500000\t500,000000\r\n3903\t317555241\t995,000000\t498,000000\t500,000000\r\n3904\t317556943\t997,000000\t498,250000\t500,000000\r\n3905\t317558642\t997,500000\t497,250000\t500,000000\r\n3906\t317560341\t997,500000\t497,750000\t500,000000\r\n3907\t317562038\t997,500000\t497,750000\t500,000000\r\n3908\t317563734\t995,900000\t497,250000\t500,000000\r\n3909\t317565349\t996,500000\t497,750000\t500,000000\r\n3910\t317566893\t998,000000\t498,250000\t500,000000\r\n3911\t317568359\t998,500000\t498,250000\t500,000000\r\n3912\t317569912\t997,000000\t497,750000\t500,000000\r\n3913\t317571420\t998,000000\t497,750000\t500,000000\r\n3914\t317572926\t996,500000\t498,250000\t500,000000\r\n3915\t317574524\t997,500000\t498,000000\t500,000000\r\n3916\t317576090\t997,500000\t497,500000\t500,000000\r\n3917\t317577641\t996,500000\t499,250000\t500,000000\r\n3918\t317579204\t996,000000\t497,250000\t500,000000\r\n3919\t317580721\t997,000000\t498,250000\t500,000000\r\n3920\t317582223\t994,500000\t497,250000\t500,000000\r\n3921\t317583787\t996,500000\t498,250000\t500,000000\r\n3922\t317585391\t995,500000\t498,000000\t500,000000\r\n3923\t317586963\t996,500000\t498,500000\t500,000000\r\n3924\t317588546\t996,500000\t499,000000\t500,000000\r\n3925\t317590253\t995,500000\t498,500000\t500,000000\r\n3926\t317591962\t997,500000\t498,500000\t500,000000\r\n3927\t317593663\t998,500000\t497,250000\t500,000000\r\n3928\t317595366\t994,500000\t498,000000\t500,000000\r\n3929\t317597066\t994,500000\t498,000000\t500,000000\r\n3930\t317598760\t996,500000\t498,750000\t500,000000\r\n3931\t317600370\t997,000000\t497,250000\t500,000000\r\n3932\t317601908\t992,900000\t498,500000\t500,000000\r\n3933\t317603381\t995,000000\t497,250000\t500,000000\r\n3934\t317604942\t995,000000\t498,750000\t500,000000\r\n3935\t317606504\t997,000000\t497,500000\t500,000000\r\n3936\t317608073\t997,500000\t498,000000\t500,000000\r\n3937\t317609768\t994,900000\t497,500000\t500,000000\r\n3938\t317611466\t995,000000\t498,000000\t500,000000\r\n3939\t317613160\t996,000000\t497,500000\t500,000000\r\n3940\t317614843\t1000,500000\t498,000000\t500,000000\r\n3941\t317616535\t996,500000\t498,500000\t500,000000\r\n3942\t317618224\t997,500000\t497,500000\t500,000000\r\n3943\t317619914\t997,500000\t497,000000\t500,000000\r\n3944\t317621608\t997,500000\t498,250000\t500,000000\r\n3945\t317623295\t995,000000\t497,750000\t500,000000\r\n3946\t317624991\t995,500000\t497,750000\t500,000000\r\n3947\t317626684\t994,000000\t498,250000\t500,000000\r\n3948\t317628374\t994,500000\t499,000000\t500,000000\r\n3949\t317630066\t994,400000\t498,750000\t500,000000\r\n3950\t317631766\t994,500000\t498,000000\t500,000000\r\n3951\t317633465\t991,500000\t497,750000\t500,000000\r\n3952\t317635162\t994,500000\t498,500000\t500,000000\r\n3953\t317636862\t996,500000\t497,500000\t500,000000\r\n3954\t317638563\t995,000000\t498,250000\t500,000000\r\n3955\t317640263\t1000,000000\t497,750000\t500,000000\r\n3956\t317641960\t992,000000\t497,750000\t500,000000\r\n3957\t317643657\t992,500000\t497,500000\t500,000000\r\n3958\t317645357\t994,500000\t498,500000\t500,000000\r\n3959\t317647064\t995,000000\t498,250000\t500,000000\r\n3960\t317648759\t993,000000\t497,750000\t500,000000\r\n3961\t317650463\t993,400000\t499,250000\t500,000000\r\n3962\t317652166\t991,500000\t497,750000\t500,000000\r\n3963\t317653866\t993,000000\t498,250000\t500,000000\r\n3964\t317655569\t994,000000\t498,500000\t500,000000\r\n3965\t317657262\t992,000000\t498,750000\t500,000000\r\n3966\t317658963\t994,500000\t497,500000\t500,000000\r\n3967\t317660672\t995,000000\t498,250000\t500,000000\r\n3968\t317662371\t995,500000\t498,750000\t500,000000\r\n3969\t317664072\t993,000000\t499,000000\t500,000000\r\n3970\t317665770\t998,000000\t499,000000\t500,000000\r\n3971\t317667478\t992,500000\t497,250000\t500,000000\r\n3972\t317669177\t991,900000\t497,750000\t500,000000\r\n3973\t317670864\t992,500000\t498,250000\t500,000000\r\n3974\t317672561\t995,000000\t497,750000\t500,000000\r\n3975\t317674263\t993,000000\t498,500000\t500,000000\r\n3976\t317675967\t993,000000\t498,250000\t500,000000\r\n3977\t317677664\t994,000000\t497,750000\t500,000000\r\n3978\t317679363\t992,000000\t498,000000\t500,000000\r\n3979\t317681057\t991,400000\t498,000000\t500,000000\r\n3980\t317682758\t992,000000\t498,500000\t500,000000\r\n3981\t317684455\t991,500000\t497,750000\t500,000000\r\n3982\t317686153\t991,000000\t498,500000\t500,000000\r\n3983\t317687848\t991,000000\t498,500000\t500,000000\r\n3984\t317689546\t991,500000\t498,250000\t500,000000\r\n3985\t317691237\t993,500000\t497,000000\t500,000000\r\n3986\t317692930\t991,000000\t498,250000\t500,000000\r\n3987\t317694631\t989,000000\t497,950000\t500,000000\r\n3988\t317696336\t992,000000\t498,250000\t500,000000\r\n3989\t317698031\t991,500000\t498,250000\t500,000000\r\n3990\t317699733\t994,000000\t498,250000\t500,000000\r\n3991\t317701435\t992,000000\t497,500000\t500,000000\r\n3992\t317703141\t991,500000\t498,250000\t500,000000\r\n3993\t317704841\t991,500000\t498,750000\t500,000000\r\n3994\t317706544\t991,500000\t497,500000\t500,000000\r\n3995\t317708243\t990,500000\t497,000000\t500,000000\r\n3996\t317709701\t992,500000\t497,250000\t500,000000\r\n3997\t317711287\t991,000000\t497,500000\t500,000000\r\n3998\t317712745\t993,500000\t498,500000\t500,000000\r\n3999\t317713879\t990,000000\t498,250000\t500,000000\r\n4000\t317715018\t990,500000\t498,500000\t500,000000\r\n4001\t317716151\t990,900000\t497,450000\t500,000000\r\n4002\t317717286\t988,500000\t498,000000\t500,000000\r\n4003\t317718422\t991,000000\t498,500000\t500,000000\r\n4004\t317719565\t991,000000\t498,750000\t500,000000\r\n4005\t317720702\t990,500000\t498,500000\t500,000000\r\n4006\t317721841\t990,500000\t497,750000\t500,000000\r\n4007\t317722977\t991,000000\t497,750000\t500,000000\r\n4008\t317724116\t990,500000\t498,250000\t500,000000\r\n4009\t317725258\t991,000000\t498,000000\t500,000000\r\n4010\t317726402\t989,000000\t497,750000\t500,000000\r\n4011\t317727539\t990,400000\t498,500000\t500,000000\r\n4012\t317728680\t990,500000\t498,000000\t500,000000\r\n4013\t317730120\t990,500000\t497,750000\t500,000000\r\n4014\t317731645\t990,000000\t497,750000\t500,000000\r\n4015\t317733131\t990,000000\t499,750000\t500,000000\r\n4016\t317734675\t987,400000\t498,750000\t500,000000\r\n4017\t317736151\t989,000000\t497,250000\t500,000000\r\n4018\t317737705\t991,500000\t498,250000\t500,000000\r\n4019\t317739277\t989,000000\t497,750000\t500,000000\r\n4020\t317740785\t989,400000\t498,500000\t500,000000\r\n4021\t317742109\t987,900000\t498,750000\t500,000000\r\n4022\t317743242\t990,400000\t498,000000\t500,000000\r\n4023\t317744375\t988,000000\t497,250000\t500,000000\r\n4024\t317745506\t989,400000\t498,250000\t500,000000\r\n4025\t317746642\t989,000000\t498,000000\t500,000000\r\n4026\t317747774\t988,900000\t497,750000\t500,000000\r\n4027\t317748907\t988,500000\t498,250000\t500,000000\r\n4028\t317750044\t990,000000\t497,500000\t500,000000\r\n4029\t317751176\t989,500000\t498,250000\t500,000000\r\n4030\t317752314\t987,500000\t498,250000\t500,000000\r\n4031\t317753570\t989,500000\t497,750000\t500,000000\r\n4032\t317755038\t991,500000\t498,500000\t500,000000\r\n4033\t317756549\t990,000000\t498,500000\t500,000000\r\n4034\t317758089\t992,000000\t499,000000\t500,000000\r\n4035\t317759622\t988,500000\t497,500000\t500,000000\r\n4036\t317761183\t992,500000\t498,250000\t500,000000\r\n4037\t317762846\t990,500000\t498,000000\t500,000000\r\n4038\t317764545\t988,500000\t498,750000\t500,000000\r\n4039\t317766241\t988,900000\t497,750000\t500,000000\r\n4040\t317767940\t991,000000\t498,250000\t500,000000\r\n4041\t317769640\t987,500000\t498,000000\t500,000000\r\n4042\t317771339\t990,000000\t497,250000\t500,000000\r\n4043\t317773040\t988,000000\t498,000000\t500,000000\r\n4044\t317774750\t989,000000\t497,000000\t500,000000\r\n4045\t317776452\t988,000000\t498,250000\t500,000000\r\n4046\t317778145\t989,500000\t498,250000\t500,000000\r\n4047\t317779839\t986,800000\t498,250000\t500,000000\r\n4048\t317781536\t989,900000\t497,750000\t500,000000\r\n4049\t317783233\t988,500000\t497,250000\t500,000000\r\n4050\t317784927\t989,000000\t498,750000\t500,000000\r\n4051\t317786622\t988,000000\t498,250000\t500,000000\r\n4052\t317788321\t989,500000\t497,500000\t500,000000\r\n4053\t317790015\t989,900000\t499,250000\t500,000000\r\n4054\t317791695\t989,000000\t497,750000\t500,000000\r\n4055\t317793393\t988,900000\t497,250000\t500,000000\r\n4056\t317795099\t988,000000\t498,500000\t500,000000\r\n4057\t317796791\t985,100000\t498,000000\t500,000000\r\n4058\t317798480\t988,500000\t498,250000\t500,000000\r\n4059\t317800176\t986,500000\t498,500000\t500,000000\r\n4060\t317801877\t989,400000\t498,500000\t500,000000\r\n4061\t317803561\t988,000000\t497,500000\t500,000000\r\n4062\t317805259\t984,700000\t498,000000\t500,000000\r\n4063\t317806953\t986,800000\t498,750000\t500,000000\r\n4064\t317808651\t987,800000\t497,750000\t500,000000\r\n4065\t317810340\t987,000000\t498,250000\t500,000000\r\n4066\t317812036\t987,400000\t498,250000\t500,000000\r\n4067\t317813724\t988,000000\t498,750000\t500,000000\r\n4068\t317815421\t986,300000\t498,250000\t500,000000\r\n4069\t317817114\t985,400000\t498,750000\t500,000000\r\n4070\t317818812\t986,500000\t498,500000\t500,000000\r\n4071\t317820505\t984,700000\t497,750000\t500,000000\r\n4072\t317822193\t986,900000\t497,750000\t500,000000\r\n4073\t317823886\t985,900000\t498,500000\t500,000000\r\n4074\t317825585\t987,300000\t498,250000\t500,000000\r\n4075\t317827276\t986,800000\t497,500000\t500,000000\r\n4076\t317828971\t986,300000\t498,500000\t500,000000\r\n4077\t317830667\t986,400000\t497,500000\t500,000000\r\n4078\t317832373\t986,300000\t497,750000\t500,000000\r\n4079\t317834071\t989,400000\t498,000000\t500,000000\r\n4080\t317835214\t985,800000\t497,500000\t500,000000\r\n4081\t317836353\t984,100000\t497,750000\t500,000000\r\n4082\t317837485\t985,200000\t497,500000\t500,000000\r\n4083\t317838622\t988,300000\t498,750000\t500,000000\r\n4084\t317839754\t986,800000\t497,500000\t500,000000\r\n4085\t317840890\t985,900000\t497,750000\t500,000000\r\n4086\t317842026\t988,500000\t498,250000\t500,000000\r\n4087\t317843160\t986,300000\t498,000000\t500,000000\r\n4088\t317844299\t985,900000\t497,500000\t500,000000\r\n4089\t317845432\t989,000000\t497,000000\t500,000000\r\n4090\t317846568\t986,300000\t497,450000\t500,000000\r\n4091\t317847700\t984,700000\t497,500000\t500,000000\r\n4092\t317848844\t986,200000\t498,000000\t500,000000\r\n4093\t317849981\t985,800000\t497,750000\t500,000000\r\n4094\t317851119\t988,400000\t497,500000\t500,000000\r\n4095\t317852254\t986,200000\t497,250000\t500,000000\r\n4096\t317853399\t985,700000\t497,250000\t500,000000\r\n4097\t317854531\t986,300000\t498,250000\t500,000000\r\n4098\t317855670\t984,700000\t498,250000\t500,000000\r\n4099\t317856813\t986,200000\t497,250000\t500,000000\r\n4100\t317857952\t986,300000\t498,250000\t500,000000\r\n4101\t317859083\t985,800000\t498,000000\t500,000000\r\n4102\t317860213\t985,800000\t497,750000\t500,000000\r\n4103\t317861351\t985,700000\t498,500000\t500,000000\r\n4104\t317862485\t985,200000\t498,500000\t500,000000\r\n4105\t317863622\t985,800000\t498,250000\t500,000000\r\n4106\t317864760\t986,200000\t498,500000\t500,000000\r\n4107\t317865896\t985,300000\t498,250000\t500,000000\r\n4108\t317867037\t986,200000\t498,500000\t500,000000\r\n4109\t317868173\t982,900000\t497,250000\t500,000000\r\n4110\t317869308\t985,200000\t498,750000\t500,000000\r\n4111\t317870445\t985,700000\t498,000000\t500,000000\r\n4112\t317871582\t985,200000\t498,500000\t500,000000\r\n4113\t317872728\t983,500000\t498,000000\t500,000000\r\n4114\t317873870\t985,400000\t498,500000\t500,000000\r\n4115\t317875005\t985,300000\t498,500000\t500,000000\r\n4116\t317876140\t983,600000\t497,700000\t500,000000\r\n4117\t317877274\t984,200000\t497,750000\t500,000000\r\n4118\t317878408\t986,800000\t498,000000\t500,000000\r\n4119\t317879544\t984,100000\t497,750000\t500,000000\r\n4120\t317880676\t983,600000\t497,500000\t500,000000\r\n4121\t317881816\t984,000000\t497,750000\t500,000000\r\n4122\t317882945\t985,000000\t498,250000\t500,000000\r\n4123\t317884082\t984,700000\t497,450000\t500,000000\r\n4124\t317885217\t985,100000\t497,500000\t500,000000\r\n4125\t317886353\t983,400000\t497,750000\t500,000000\r\n4126\t317887493\t983,500000\t498,250000\t500,000000\r\n4127\t317888628\t985,200000\t497,750000\t500,000000\r\n4128\t317889764\t983,600000\t497,250000\t500,000000\r\n4129\t317890903\t984,000000\t497,750000\t500,000000\r\n4130\t317892042\t985,300000\t498,000000\t500,000000\r\n4131\t317893182\t986,400000\t497,250000\t500,000000\r\n4132\t317894315\t984,000000\t498,500000\t500,000000\r\n4133\t317895449\t982,300000\t498,250000\t500,000000\r\n4134\t317896587\t984,600000\t497,250000\t500,000000\r\n4135\t317897722\t982,400000\t497,250000\t500,000000\r\n4136\t317898856\t982,300000\t497,500000\t500,000000\r\n4137\t317899987\t983,400000\t498,000000\t500,000000\r\n4138\t317901126\t984,600000\t498,500000\t500,000000\r\n4139\t317902265\t984,100000\t498,250000\t500,000000\r\n4140\t317903405\t979,800000\t497,750000\t500,000000\r\n4141\t317904537\t984,000000\t498,500000\t500,000000\r\n4142\t317905672\t984,500000\t498,250000\t500,000000\r\n4143\t317906807\t983,500000\t498,750000\t500,000000\r\n4144\t317907947\t980,800000\t497,500000\t500,000000\r\n4145\t317909084\t983,000000\t498,750000\t500,000000\r\n4146\t317910220\t983,900000\t498,000000\t500,000000\r\n4147\t317911361\t980,600000\t497,500000\t500,000000\r\n4148\t317912500\t982,900000\t497,500000\t500,000000\r\n4149\t317913640\t984,100000\t498,000000\t500,000000\r\n4150\t317914773\t982,800000\t498,250000\t500,000000\r\n4151\t317915909\t983,000000\t497,500000\t500,000000\r\n4152\t317917333\t982,900000\t498,500000\t500,000000\r\n4153\t317919034\t983,700000\t497,500000\t500,000000\r\n4154\t317920731\t985,200000\t499,000000\t500,000000\r\n4155\t317922436\t982,500000\t497,500000\t500,000000\r\n4156\t317924119\t985,700000\t498,200000\t500,000000\r\n4157\t317925827\t982,300000\t498,000000\t500,000000\r\n4158\t317927531\t983,000000\t497,750000\t500,000000\r\n4159\t317929222\t982,000000\t498,500000\t500,000000\r\n4160\t317930923\t982,400000\t497,500000\t500,000000\r\n4161\t317932623\t980,800000\t497,500000\t500,000000\r\n4162\t317934322\t983,600000\t497,500000\t500,000000\r\n4163\t317936021\t981,800000\t498,500000\t500,000000\r\n4164\t317937713\t984,600000\t498,250000\t500,000000\r\n4165\t317939406\t981,300000\t497,700000\t500,000000\r\n4166\t317941106\t979,700000\t497,500000\t500,000000\r\n4167\t317942801\t982,800000\t498,000000\t500,000000\r\n4168\t317944505\t980,100000\t498,000000\t500,000000\r\n4169\t317946203\t981,800000\t497,250000\t500,000000\r\n4170\t317947904\t981,300000\t497,750000\t500,000000\r\n4171\t317949608\t980,200000\t498,500000\t500,000000\r\n4172\t317951304\t979,700000\t498,250000\t500,000000\r\n4173\t317952999\t980,800000\t497,250000\t500,000000\r\n4174\t317954697\t982,400000\t498,000000\t500,000000\r\n4175\t317956398\t980,300000\t498,500000\t500,000000\r\n4176\t317958103\t980,800000\t498,000000\t500,000000\r\n4177\t317959802\t980,800000\t497,200000\t500,000000\r\n4178\t317961508\t982,000000\t498,000000\t500,000000\r\n4179\t317963214\t981,900000\t498,000000\t500,000000\r\n4180\t317964914\t979,200000\t498,250000\t500,000000\r\n4181\t317966621\t978,600000\t498,250000\t500,000000\r\n4182\t317967769\t980,700000\t497,750000\t500,000000\r\n4183\t317968899\t979,600000\t498,250000\t500,000000\r\n4184\t317970032\t981,200000\t498,500000\t500,000000\r\n4185\t317971175\t980,300000\t498,000000\t500,000000\r\n4186\t317972533\t979,700000\t497,500000\t500,000000\r\n4187\t317974239\t980,300000\t498,500000\t500,000000\r\n4188\t317975940\t981,400000\t497,750000\t500,000000\r\n4189\t317977637\t978,100000\t498,250000\t500,000000\r\n4190\t317979340\t978,500000\t498,750000\t500,000000\r\n4191\t317981038\t979,600000\t497,200000\t500,000000\r\n4192\t317982736\t978,200000\t497,250000\t500,000000\r\n4193\t317984432\t980,200000\t498,000000\t500,000000\r\n4194\t317986139\t980,800000\t498,000000\t500,000000\r\n4195\t317987842\t982,000000\t498,000000\t500,000000\r\n4196\t317989543\t979,200000\t497,750000\t500,000000\r\n4197\t317991239\t979,700000\t497,500000\t500,000000\r\n4198\t317992939\t978,500000\t497,750000\t500,000000\r\n4199\t317994639\t978,700000\t496,200000\t500,000000\r\n4200\t317996339\t976,000000\t497,750000\t500,000000\r\n4201\t317998038\t980,300000\t496,950000\t500,000000\r\n4202\t317999738\t979,200000\t497,750000\t500,000000\r\n4203\t318001436\t978,000000\t498,250000\t500,000000\r\n4204\t318003134\t977,600000\t497,750000\t500,000000\r\n4205\t318004835\t977,100000\t498,000000\t500,000000\r\n4206\t318006524\t976,500000\t498,500000\t500,000000\r\n4207\t318008219\t978,200000\t498,000000\t500,000000\r\n4208\t318009913\t980,200000\t497,750000\t500,000000\r\n4209\t318011608\t977,200000\t498,250000\t500,000000\r\n4210\t318013313\t977,500000\t497,250000\t500,000000\r\n4211\t318015009\t979,700000\t498,500000\t500,000000\r\n4212\t318016704\t977,500000\t498,250000\t500,000000\r\n4213\t318018405\t978,700000\t498,250000\t500,000000\r\n4214\t318020106\t976,600000\t496,950000\t500,000000\r\n4215\t318021802\t977,100000\t498,000000\t500,000000\r\n4216\t318023510\t977,100000\t498,750000\t500,000000\r\n4217\t318025213\t978,800000\t498,250000\t500,000000\r\n4218\t318026917\t977,000000\t498,500000\t500,000000\r\n4219\t318028616\t977,100000\t498,000000\t500,000000\r\n4220\t318030315\t974,000000\t498,000000\t500,000000\r\n4221\t318032016\t978,600000\t497,750000\t500,000000\r\n4222\t318033718\t978,700000\t498,750000\t500,000000\r\n4223\t318035424\t975,000000\t498,250000\t500,000000\r\n4224\t318037124\t975,500000\t499,250000\t500,000000\r\n4225\t318038824\t977,600000\t498,500000\t500,000000\r\n4226\t318040522\t977,600000\t498,250000\t500,000000\r\n4227\t318042211\t979,200000\t498,250000\t500,000000\r\n4228\t318043915\t976,500000\t496,450000\t500,000000\r\n4229\t318045617\t976,100000\t498,000000\t500,000000\r\n4230\t318047319\t977,700000\t497,500000\t500,000000\r\n4231\t318049020\t976,500000\t498,500000\t500,000000\r\n4232\t318050727\t975,100000\t497,700000\t500,000000\r\n4233\t318052429\t978,700000\t497,500000\t500,000000\r\n4234\t318054114\t973,500000\t498,000000\t500,000000\r\n4235\t318055816\t976,000000\t497,750000\t500,000000\r\n4236\t318057523\t975,600000\t498,250000\t500,000000\r\n4237\t318059224\t976,100000\t497,250000\t500,000000\r\n4238\t318060924\t977,200000\t497,750000\t500,000000\r\n4239\t318062622\t977,700000\t497,200000\t500,000000\r\n4240\t318064323\t976,000000\t497,750000\t500,000000\r\n4241\t318066028\t977,700000\t498,250000\t500,000000\r\n4242\t318067725\t973,500000\t498,000000\t500,000000\r\n4243\t318069417\t976,000000\t498,000000\t500,000000\r\n4244\t318071116\t974,000000\t499,250000\t500,000000\r\n4245\t318072821\t971,000000\t497,500000\t500,000000\r\n4246\t318074528\t974,500000\t498,750000\t500,000000\r\n4247\t318076233\t975,000000\t497,750000\t500,000000\r\n4248\t318077929\t974,500000\t497,500000\t500,000000\r\n4249\t318079635\t974,000000\t498,000000\t500,000000\r\n4250\t318081336\t974,100000\t497,750000\t500,000000\r\n4251\t318083040\t973,500000\t498,000000\t500,000000\r\n4252\t318084740\t973,000000\t498,250000\t500,000000\r\n4253\t318086442\t976,600000\t497,500000\t500,000000\r\n4254\t318088147\t974,500000\t498,000000\t500,000000\r\n4255\t318089844\t973,000000\t498,750000\t500,000000\r\n4256\t318091553\t972,000000\t497,500000\t500,000000\r\n4257\t318093254\t974,500000\t498,250000\t500,000000\r\n4258\t318094956\t974,000000\t497,500000\t500,000000\r\n4259\t318096660\t973,500000\t498,000000\t500,000000\r\n4260\t318098364\t973,600000\t496,700000\t500,000000\r\n4261\t318100072\t973,500000\t498,250000\t500,000000\r\n4262\t318101777\t973,100000\t498,750000\t500,000000\r\n4263\t318103481\t972,500000\t498,250000\t500,000000\r\n4264\t318105176\t974,000000\t498,500000\t500,000000\r\n4265\t318106882\t974,000000\t498,250000\t500,000000\r\n4266\t318108584\t975,100000\t497,500000\t500,000000\r\n4267\t318110292\t973,000000\t498,000000\t500,000000\r\n4268\t318111996\t971,000000\t498,000000\t500,000000\r\n4269\t318113700\t972,000000\t498,000000\t500,000000\r\n4270\t318115399\t974,000000\t498,250000\t500,000000\r\n4271\t318117099\t971,500000\t497,500000\t500,000000\r\n4272\t318118804\t970,500000\t497,000000\t500,000000\r\n4273\t318120500\t973,500000\t498,250000\t500,000000\r\n4274\t318121673\t970,500000\t498,000000\t500,000000\r\n4275\t318122811\t971,000000\t498,250000\t500,000000\r\n4276\t318123953\t971,500000\t497,750000\t500,000000\r\n4277\t318125098\t971,500000\t498,500000\t500,000000\r\n4278\t318126229\t972,000000\t497,750000\t500,000000\r\n4279\t318127368\t973,000000\t498,000000\t500,000000\r\n4280\t318128509\t971,500000\t497,500000\t500,000000\r\n4281\t318129647\t972,500000\t498,000000\t500,000000\r\n4282\t318130786\t969,500000\t498,250000\t500,000000\r\n4283\t318131925\t970,000000\t497,250000\t500,000000\r\n4284\t318133064\t971,500000\t498,000000\t500,000000\r\n4285\t318134203\t970,000000\t498,250000\t500,000000\r\n4286\t318135338\t971,000000\t498,000000\t500,000000\r\n4287\t318136645\t969,500000\t498,250000\t500,000000\r\n4288\t318138344\t970,500000\t498,250000\t500,000000\r\n4289\t318140050\t974,600000\t497,250000\t500,000000\r\n4290\t318141746\t972,000000\t497,500000\t500,000000\r\n4291\t318143433\t973,000000\t498,500000\t500,000000\r\n4292\t318145136\t971,100000\t498,250000\t500,000000\r\n4293\t318146835\t970,500000\t497,250000\t500,000000\r\n4294\t318148332\t968,000000\t498,500000\t500,000000\r\n4295\t318149461\t971,000000\t499,000000\t500,000000\r\n4296\t318150606\t971,500000\t498,750000\t500,000000\r\n4297\t318151747\t971,500000\t498,500000\t500,000000\r\n4298\t318152876\t971,000000\t497,250000\t500,000000\r\n4299\t318154006\t971,600000\t498,250000\t500,000000\r\n4300\t318155135\t968,500000\t497,750000\t500,000000\r\n4301\t318156272\t969,500000\t497,000000\t500,000000\r\n4302\t318157407\t969,500000\t497,250000\t500,000000\r\n4303\t318158561\t970,000000\t497,750000\t500,000000\r\n4304\t318159700\t969,000000\t498,750000\t500,000000\r\n4305\t318160835\t969,000000\t498,000000\t500,000000\r\n4306\t318161973\t971,000000\t498,250000\t500,000000\r\n4307\t318163065\t970,000000\t498,750000\t500,000000\r\n4308\t318164206\t970,500000\t498,250000\t500,000000\r\n4309\t318165341\t968,500000\t498,000000\t500,000000\r\n4310\t318166475\t969,000000\t498,000000\t500,000000\r\n4311\t318167608\t970,000000\t497,750000\t500,000000\r\n4312\t318168746\t968,500000\t498,750000\t500,000000\r\n4313\t318169887\t967,000000\t497,750000\t500,000000\r\n4314\t318171020\t969,000000\t498,000000\t500,000000\r\n4315\t318172153\t970,000000\t497,500000\t500,000000\r\n4316\t318173295\t969,000000\t497,750000\t500,000000\r\n4317\t318174428\t969,000000\t498,250000\t500,000000\r\n4318\t318175562\t969,500000\t497,000000\t500,000000\r\n4319\t318176698\t969,500000\t498,250000\t500,000000\r\n4320\t318177838\t971,500000\t498,500000\t500,000000\r\n4321\t318178976\t969,500000\t497,750000\t500,000000\r\n4322\t318180107\t966,000000\t498,000000\t500,000000\r\n4323\t318181247\t969,000000\t498,000000\t500,000000\r\n4324\t318182384\t969,500000\t497,500000\t500,000000\r\n4325\t318183515\t969,000000\t498,250000\t500,000000\r\n4326\t318184648\t972,000000\t497,500000\t500,000000\r\n4327\t318185782\t971,600000\t498,250000\t500,000000\r\n4328\t318186920\t967,500000\t498,500000\t500,000000\r\n4329\t318188056\t969,000000\t497,750000\t500,000000\r\n4330\t318189189\t968,500000\t498,750000\t500,000000\r\n4331\t318190326\t969,500000\t498,000000\t500,000000\r\n4332\t318191462\t968,000000\t498,750000\t500,000000\r\n4333\t318192600\t969,100000\t499,000000\t500,000000\r\n4334\t318193740\t970,000000\t498,000000\t500,000000\r\n4335\t318194876\t967,000000\t497,000000\t500,000000\r\n4336\t318196016\t968,600000\t498,500000\t500,000000\r\n4337\t318197152\t968,500000\t498,250000\t500,000000\r\n4338\t318198281\t969,000000\t498,250000\t500,000000\r\n4339\t318199415\t969,000000\t497,500000\t500,000000\r\n4340\t318200555\t971,000000\t498,500000\t500,000000\r\n4341\t318201686\t969,500000\t498,500000\t500,000000\r\n4342\t318202817\t969,500000\t498,000000\t500,000000\r\n4343\t318203956\t967,000000\t498,750000\t500,000000\r\n4344\t318205091\t969,500000\t498,000000\t500,000000\r\n4345\t318206233\t969,000000\t497,750000\t500,000000\r\n4346\t318207371\t968,500000\t498,250000\t500,000000\r\n4347\t318208513\t967,500000\t498,000000\t500,000000\r\n4348\t318209652\t970,100000\t498,000000\t500,000000\r\n4349\t318210788\t967,500000\t498,750000\t500,000000\r\n4350\t318211935\t970,100000\t498,750000\t500,000000\r\n4351\t318213080\t970,000000\t498,000000\t500,000000\r\n4352\t318214224\t966,500000\t497,250000\t500,000000\r\n4353\t318215363\t967,500000\t498,000000\t500,000000\r\n4354\t318216504\t968,500000\t498,000000\t500,000000\r\n4355\t318217642\t968,500000\t497,750000\t500,000000\r\n4356\t318218777\t968,500000\t497,500000\t500,000000\r\n4357\t318219915\t970,000000\t497,750000\t500,000000\r\n4358\t318221049\t965,500000\t497,750000\t500,000000\r\n4359\t318222187\t967,500000\t498,500000\t500,000000\r\n4360\t318223320\t969,100000\t498,750000\t500,000000\r\n4361\t318224465\t969,000000\t498,750000\t500,000000\r\n4362\t318225605\t967,500000\t498,000000\t500,000000\r\n4363\t318226745\t968,000000\t498,250000\t500,000000\r\n4364\t318227884\t969,500000\t497,750000\t500,000000\r\n4365\t318229019\t969,600000\t498,000000\t500,000000\r\n4366\t318230151\t967,500000\t498,250000\t500,000000\r\n4367\t318231278\t968,000000\t498,500000\t500,000000\r\n4368\t318232414\t968,000000\t498,000000\t500,000000\r\n4369\t318233542\t966,500000\t497,500000\t500,000000\r\n4370\t318234684\t966,000000\t498,250000\t500,000000\r\n4371\t318235824\t967,500000\t498,250000\t500,000000\r\n4372\t318236965\t968,500000\t498,500000\t500,000000\r\n4373\t318238108\t966,000000\t498,750000\t500,000000\r\n4374\t318239241\t966,000000\t498,250000\t500,000000\r\n4375\t318240374\t967,000000\t498,000000\t500,000000\r\n4376\t318241507\t966,000000\t498,500000\t500,000000\r\n4377\t318242641\t966,500000\t498,250000\t500,000000\r\n4378\t318243782\t966,000000\t498,750000\t500,000000\r\n4379\t318244926\t968,000000\t498,500000\t500,000000\r\n4380\t318246071\t968,500000\t498,750000\t500,000000\r\n4381\t318247211\t966,000000\t498,500000\t500,000000\r\n4382\t318248353\t968,500000\t498,500000\t500,000000\r\n4383\t318249497\t966,500000\t497,500000\t500,000000\r\n4384\t318250630\t968,500000\t498,250000\t500,000000\r\n4385\t318251768\t968,000000\t498,500000\t500,000000\r\n4386\t318252912\t966,500000\t498,500000\t500,000000\r\n4387\t318254050\t964,500000\t497,200000\t500,000000\r\n4388\t318255211\t967,500000\t497,250000\t500,000000\r\n4390\t318257402\t966,500000\t498,000000\t500,000000\r\n4391\t318258556\t968,000000\t497,750000\t500,000000\r\n4392\t318259686\t966,000000\t497,750000\t500,000000\r\n4393\t318260822\t968,000000\t499,000000\t500,000000\r\n4394\t318261960\t966,500000\t498,250000\t500,000000\r\n4395\t318263101\t967,000000\t498,000000\t500,000000\r\n4396\t318264245\t965,000000\t497,750000\t500,000000\r\n4397\t318265383\t965,000000\t498,250000\t500,000000\r\n4398\t318266521\t966,500000\t498,250000\t500,000000\r\n4399\t318267658\t966,000000\t498,000000\t500,000000\r\n4400\t318268793\t968,000000\t497,750000\t500,000000\r\n4401\t318269929\t966,000000\t497,750000\t500,000000\r\n4402\t318271068\t966,500000\t497,500000\t500,000000\r\n4403\t318272201\t965,500000\t498,000000\t500,000000\r\n4404\t318273340\t966,500000\t497,750000\t500,000000\r\n4405\t318274477\t967,500000\t497,750000\t500,000000\r\n4406\t318275614\t966,000000\t498,250000\t500,000000\r\n4407\t318276748\t965,000000\t497,500000\t500,000000\r\n4408\t318277892\t964,000000\t497,950000\t500,000000\r\n4409\t318279032\t966,500000\t498,250000\t500,000000\r\n4410\t318280168\t967,500000\t498,250000\t500,000000\r\n4411\t318281304\t964,500000\t498,750000\t500,000000\r\n4412\t318282439\t967,000000\t497,500000\t500,000000\r\n4413\t318283570\t967,100000\t497,750000\t500,000000\r\n4414\t318284703\t966,500000\t497,750000\t500,000000\r\n4415\t318285839\t966,000000\t498,000000\t500,000000\r\n4416\t318286981\t964,500000\t498,500000\t500,000000\r\n4417\t318288119\t964,500000\t498,500000\t500,000000\r\n4418\t318289257\t965,500000\t498,500000\t500,000000\r\n4419\t318290388\t964,000000\t497,750000\t500,000000\r\n4420\t318291520\t964,500000\t498,500000\t500,000000\r\n4421\t318292660\t966,500000\t498,500000\t500,000000\r\n4422\t318293796\t967,100000\t497,750000\t500,000000\r\n4423\t318294949\t965,500000\t498,250000\t500,000000\r\n4424\t318296089\t965,500000\t497,500000\t500,000000\r\n4425\t318297219\t963,500000\t498,000000\t500,000000\r\n4426\t318298353\t964,000000\t499,000000\t500,000000\r\n4427\t318299506\t963,500000\t498,000000\t500,000000\r\n4428\t318300641\t962,500000\t498,000000\t500,000000\r\n4429\t318301779\t963,000000\t498,250000\t500,000000\r\n4430\t318302910\t962,500000\t497,500000\t500,000000\r\n4431\t318304055\t962,000000\t497,750000\t500,000000\r\n4432\t318305195\t966,000000\t497,750000\t500,000000\r\n4433\t318306331\t962,000000\t498,750000\t500,000000\r\n4434\t318307467\t966,000000\t498,250000\t500,000000\r\n4435\t318308606\t963,500000\t497,500000\t500,000000\r\n4436\t318309738\t964,000000\t497,750000\t500,000000\r\n4437\t318310872\t964,000000\t498,750000\t500,000000\r\n4438\t318312007\t963,500000\t498,750000\t500,000000\r\n4439\t318313150\t965,500000\t498,750000\t500,000000\r\n4440\t318314286\t965,000000\t498,500000\t500,000000\r\n4441\t318315420\t964,000000\t498,000000\t500,000000\r\n4442\t318316555\t964,000000\t498,500000\t500,000000\r\n4443\t318317698\t964,000000\t497,700000\t500,000000\r\n4444\t318318838\t964,000000\t498,500000\t500,000000\r\n4445\t318319971\t965,000000\t498,500000\t500,000000\r\n4446\t318321109\t965,500000\t497,750000\t500,000000\r\n4447\t318322248\t964,000000\t498,250000\t500,000000\r\n4448\t318323387\t962,000000\t498,250000\t500,000000\r\n4449\t318324524\t963,000000\t498,250000\t500,000000\r\n4450\t318325665\t964,000000\t497,500000\t500,000000\r\n4451\t318326802\t963,500000\t498,500000\t500,000000\r\n4452\t318327938\t964,000000\t498,500000\t500,000000\r\n4453\t318329074\t962,000000\t498,500000\t500,000000\r\n4454\t318330214\t966,000000\t497,750000\t500,000000\r\n4455\t318331356\t964,000000\t497,750000\t500,000000\r\n4456\t318332491\t966,000000\t498,250000\t500,000000\r\n4457\t318333625\t965,000000\t498,000000\t500,000000\r\n4458\t318334765\t966,000000\t498,500000\t500,000000\r\n4459\t318335906\t964,500000\t497,750000\t500,000000\r\n4460\t318337049\t962,500000\t498,500000\t500,000000\r\n4461\t318338195\t963,000000\t498,000000\t500,000000\r\n4462\t318339338\t963,500000\t497,750000\t500,000000\r\n4463\t318340477\t962,500000\t498,250000\t500,000000\r\n4464\t318341613\t963,500000\t497,500000\t500,000000\r\n4465\t318342750\t964,500000\t497,750000\t500,000000\r\n4466\t318343879\t963,500000\t498,000000\t500,000000\r\n4467\t318345016\t960,000000\t498,000000\t500,000000\r\n4468\t318346151\t963,500000\t498,000000\t500,000000\r\n4469\t318347287\t962,500000\t498,500000\t500,000000\r\n4470\t318348424\t962,000000\t498,000000\t500,000000\r\n4471\t318349558\t962,000000\t498,000000\t500,000000\r\n4472\t318350692\t962,000000\t496,750000\t500,000000\r\n4473\t318351827\t962,000000\t498,000000\t500,000000\r\n4474\t318352966\t961,500000\t498,000000\t500,000000\r\n4475\t318354100\t962,500000\t498,000000\t500,000000\r\n4476\t318355236\t960,000000\t497,000000\t500,000000\r\n4477\t318356379\t958,500000\t498,750000\t500,000000\r\n4478\t318357518\t961,500000\t497,750000\t500,000000\r\n4479\t318358655\t962,000000\t497,500000\t500,000000\r\n4480\t318359789\t961,500000\t498,250000\t500,000000\r\n4481\t318360930\t963,500000\t499,000000\t500,000000\r\n4482\t318362065\t961,000000\t498,500000\t500,000000\r\n4483\t318363205\t963,500000\t498,250000\t500,000000\r\n4484\t318364342\t963,000000\t498,500000\t500,000000\r\n4485\t318365475\t961,500000\t498,500000\t500,000000\r\n4486\t318366619\t965,500000\t498,250000\t500,000000\r\n4487\t318367747\t961,000000\t497,750000\t500,000000\r\n4488\t318368886\t961,500000\t498,000000\t500,000000\r\n4489\t318370027\t964,500000\t498,000000\t500,000000\r\n4490\t318371170\t962,500000\t498,000000\t500,000000\r\n4491\t318372307\t961,500000\t498,250000\t500,000000\r\n4492\t318373444\t961,500000\t497,750000\t500,000000\r\n4493\t318374579\t963,500000\t497,500000\t500,000000\r\n4494\t318375724\t963,000000\t498,000000\t500,000000\r\n4495\t318376871\t962,000000\t498,750000\t500,000000\r\n4496\t318378007\t960,500000\t498,000000\t500,000000\r\n4497\t318379146\t961,000000\t498,500000\t500,000000\r\n4498\t318380277\t963,000000\t497,750000\t500,000000\r\n4499\t318381412\t961,000000\t497,750000\t500,000000\r\n4500\t318382554\t960,500000\t499,000000\t500,000000\r\n4501\t318383697\t960,000000\t497,750000\t500,000000\r\n4502\t318384842\t959,000000\t497,750000\t500,000000\r\n4503\t318385977\t960,500000\t498,750000\t500,000000\r\n4504\t318387112\t961,500000\t498,500000\t500,000000\r\n4505\t318388247\t959,500000\t497,750000\t500,000000\r\n4506\t318389394\t961,500000\t497,000000\t500,000000\r\n4507\t318390530\t961,500000\t497,750000\t500,000000\r\n4508\t318391666\t963,100000\t497,500000\t500,000000\r\n4509\t318392794\t960,000000\t498,250000\t500,000000\r\n4510\t318393938\t961,000000\t498,500000\t500,000000\r\n4511\t318395077\t960,000000\t497,500000\t500,000000\r\n4512\t318396213\t962,000000\t497,750000\t500,000000\r\n4513\t318397349\t962,000000\t498,250000\t500,000000\r\n4514\t318398489\t960,500000\t497,750000\t500,000000\r\n4515\t318399630\t959,500000\t498,000000\t500,000000\r\n4516\t318400767\t962,500000\t497,500000\t500,000000\r\n4517\t318401902\t959,500000\t497,950000\t500,000000\r\n4518\t318403041\t959,500000\t499,000000\t500,000000\r\n4519\t318404177\t961,000000\t497,500000\t500,000000\r\n4520\t318405318\t957,000000\t497,500000\t500,000000\r\n4521\t318406454\t958,500000\t498,250000\t500,000000\r\n4522\t318407587\t962,000000\t498,500000\t500,000000\r\n4523\t318408721\t961,500000\t498,750000\t500,000000\r\n4524\t318409853\t959,500000\t497,750000\t500,000000\r\n4525\t318410989\t955,000000\t497,750000\t500,000000\r\n4526\t318412125\t961,000000\t497,500000\t500,000000\r\n4527\t318413263\t960,500000\t498,000000\t500,000000\r\n4528\t318414391\t957,000000\t499,000000\t500,000000\r\n4529\t318415520\t959,000000\t498,750000\t500,000000\r\n4530\t318416665\t960,500000\t497,500000\t500,000000\r\n4531\t318417798\t959,500000\t498,250000\t500,000000\r\n4532\t318418935\t957,500000\t497,250000\t500,000000\r\n4533\t318420065\t959,500000\t498,250000\t500,000000\r\n4534\t318421200\t960,500000\t498,250000\t500,000000\r\n4535\t318422341\t960,500000\t498,000000\t500,000000\r\n4536\t318423481\t959,500000\t498,000000\t500,000000\r\n4537\t318424619\t960,500000\t498,750000\t500,000000\r\n4538\t318425755\t957,000000\t497,750000\t500,000000\r\n4539\t318426891\t958,000000\t498,000000\t500,000000\r\n4540\t318428026\t959,500000\t498,250000\t500,000000\r\n4541\t318429168\t959,500000\t498,250000\t500,000000\r\n4542\t318430305\t956,500000\t499,000000\t500,000000\r\n4543\t318431443\t957,500000\t498,500000\t500,000000\r\n4544\t318432578\t960,000000\t498,750000\t500,000000\r\n4545\t318433717\t957,000000\t497,750000\t500,000000\r\n4546\t318434856\t959,000000\t498,750000\t500,000000\r\n4547\t318435990\t958,000000\t498,000000\t500,000000\r\n4548\t318437135\t957,500000\t498,500000\t500,000000\r\n4549\t318438277\t958,000000\t498,000000\t500,000000\r\n4550\t318439415\t956,500000\t497,750000\t500,000000\r\n4551\t318440546\t958,000000\t498,750000\t500,000000\r\n4552\t318441679\t959,000000\t498,500000\t500,000000\r\n4553\t318442813\t957,000000\t498,000000\t500,000000\r\n4554\t318443953\t956,500000\t498,250000\t500,000000\r\n4555\t318445085\t959,000000\t497,750000\t500,000000\r\n4556\t318446226\t956,500000\t498,750000\t500,000000\r\n4557\t318447361\t958,000000\t498,000000\t500,000000\r\n4558\t318448507\t957,000000\t498,750000\t500,000000\r\n4559\t318449652\t957,500000\t497,750000\t500,000000\r\n4560\t318450792\t957,500000\t497,500000\t500,000000\r\n4561\t318451926\t957,500000\t497,750000\t500,000000\r\n4562\t318453063\t955,000000\t498,000000\t500,000000\r\n4563\t318454206\t957,000000\t498,000000\t500,000000\r\n4564\t318455352\t955,500000\t499,000000\t500,000000\r\n4565\t318456488\t957,500000\t497,750000\t500,000000\r\n4566\t318457625\t957,000000\t498,000000\t500,000000\r\n4567\t318458761\t956,000000\t498,250000\t500,000000\r\n4568\t318459900\t957,500000\t497,750000\t500,000000\r\n4569\t318461034\t955,500000\t498,500000\t500,000000\r\n4570\t318462172\t955,500000\t498,250000\t500,000000\r\n4571\t318463301\t955,000000\t499,250000\t500,000000\r\n4572\t318464436\t955,000000\t498,000000\t500,000000\r\n4573\t318465569\t957,000000\t497,750000\t500,000000\r\n4574\t318466708\t954,500000\t498,500000\t500,000000\r\n4575\t318467838\t956,500000\t498,000000\t500,000000\r\n4576\t318468980\t955,000000\t497,750000\t500,000000\r\n4577\t318470114\t957,000000\t498,500000\t500,000000\r\n4578\t318471249\t957,500000\t497,750000\t500,000000\r\n4579\t318472390\t958,500000\t498,000000\t500,000000\r\n4580\t318473530\t954,500000\t497,500000\t500,000000\r\n4581\t318474665\t955,500000\t498,250000\t500,000000\r\n4582\t318475808\t956,000000\t497,750000\t500,000000\r\n4583\t318476942\t956,000000\t497,750000\t500,000000\r\n4584\t318478086\t955,000000\t497,250000\t500,000000\r\n4585\t318479230\t956,000000\t497,750000\t500,000000\r\n4586\t318480368\t957,000000\t498,000000\t500,000000\r\n4587\t318481499\t955,000000\t497,750000\t500,000000\r\n4588\t318482638\t957,500000\t498,000000\t500,000000\r\n4589\t318483769\t954,500000\t498,000000\t500,000000\r\n4590\t318484900\t955,000000\t498,250000\t500,000000\r\n4591\t318486037\t956,500000\t497,750000\t500,000000\r\n4592\t318487173\t957,000000\t498,250000\t500,000000\r\n4593\t318488312\t956,500000\t498,000000\t500,000000\r\n4594\t318489454\t955,500000\t499,000000\t500,000000\r\n4595\t318490592\t956,000000\t498,250000\t500,000000\r\n4596\t318491727\t953,500000\t496,950000\t500,000000\r\n4597\t318492871\t955,000000\t498,000000\t500,000000\r\n4598\t318494013\t955,000000\t498,250000\t500,000000\r\n4599\t318495147\t954,500000\t498,000000\t500,000000\r\n4600\t318496288\t955,500000\t498,000000\t500,000000\r\n4601\t318497430\t953,500000\t498,500000\t500,000000\r\n4602\t318498570\t955,000000\t498,500000\t500,000000\r\n4603\t318499708\t954,500000\t497,500000\t500,000000\r\n4604\t318500845\t954,000000\t497,750000\t500,000000\r\n4605\t318501995\t954,500000\t497,250000\t500,000000\r\n4606\t318503138\t956,000000\t497,750000\t500,000000\r\n4607\t318504272\t956,000000\t497,750000\t500,000000\r\n4608\t318505412\t953,000000\t498,750000\t500,000000\r\n4609\t318506546\t953,000000\t497,750000\t500,000000\r\n4610\t318507966\t955,000000\t497,750000\t500,000000\r\n4611\t318509663\t954,000000\t497,250000\t500,000000\r\n4612\t318511361\t955,500000\t499,250000\t500,000000\r\n4613\t318513053\t953,000000\t498,500000\t500,000000\r\n4614\t318514757\t955,500000\t497,750000\t500,000000\r\n4615\t318516452\t952,500000\t498,000000\t500,000000\r\n4616\t318518152\t953,500000\t497,000000\t500,000000\r\n4617\t318519856\t952,000000\t497,200000\t500,000000\r\n4618\t318521555\t952,000000\t498,500000\t500,000000\r\n4619\t318523252\t953,000000\t498,500000\t500,000000\r\n4620\t318524943\t955,500000\t498,000000\t500,000000\r\n4621\t318526633\t956,000000\t498,000000\t500,000000\r\n4622\t318528325\t951,500000\t498,500000\t500,000000\r\n4623\t318530018\t951,500000\t498,250000\t500,000000\r\n4624\t318531713\t951,500000\t497,500000\t500,000000\r\n4625\t318533411\t955,000000\t498,000000\t500,000000\r\n4626\t318535113\t953,000000\t498,250000\t500,000000\r\n4627\t318536811\t952,500000\t497,750000\t500,000000\r\n4628\t318538505\t952,000000\t497,250000\t500,000000\r\n4629\t318540206\t950,500000\t497,500000\t500,000000\r\n4630\t318541903\t954,000000\t498,250000\t500,000000\r\n4631\t318543596\t951,500000\t498,250000\t500,000000\r\n4632\t318545294\t951,000000\t498,250000\t500,000000\r\n4633\t318546998\t950,500000\t498,500000\t500,000000\r\n4634\t318548693\t952,500000\t498,500000\t500,000000\r\n4635\t318550368\t952,000000\t498,750000\t500,000000\r\n4636\t318552055\t952,000000\t497,750000\t500,000000\r\n4637\t318553743\t954,000000\t498,250000\t500,000000\r\n4638\t318555438\t950,500000\t497,500000\t500,000000\r\n4639\t318557129\t951,500000\t497,750000\t500,000000\r\n4640\t318558818\t951,000000\t498,250000\t500,000000\r\n4641\t318560506\t954,000000\t498,250000\t500,000000\r\n4642\t318562204\t953,500000\t498,250000\t500,000000\r\n4643\t318563893\t953,000000\t497,750000\t500,000000\r\n4644\t318565591\t953,000000\t498,250000\t500,000000\r\n4645\t318567293\t950,500000\t497,000000\t500,000000\r\n4646\t318568985\t949,000000\t498,000000\t500,000000\r\n4647\t318570676\t954,000000\t498,500000\t500,000000\r\n4648\t318572364\t950,500000\t498,000000\t500,000000\r\n4649\t318574060\t951,000000\t498,000000\t500,000000\r\n4650\t318575758\t949,500000\t498,250000\t500,000000\r\n4651\t318577444\t950,500000\t498,750000\t500,000000\r\n4652\t318579136\t950,000000\t496,950000\t500,000000\r\n4653\t318580834\t951,000000\t497,250000\t500,000000\r\n4654\t318582525\t950,500000\t497,750000\t500,000000\r\n4655\t318584220\t950,500000\t498,750000\t500,000000\r\n4656\t318585928\t950,500000\t498,250000\t500,000000\r\n4657\t318587620\t950,000000\t498,250000\t500,000000\r\n4658\t318589315\t951,000000\t498,500000\t500,000000\r\n4659\t318591010\t950,000000\t496,700000\t500,000000\r\n4660\t318592711\t949,000000\t498,000000\t500,000000\r\n4661\t318594412\t950,500000\t498,750000\t500,000000\r\n4662\t318596114\t948,500000\t497,250000\t500,000000\r\n4663\t318597804\t948,000000\t498,500000\t500,000000\r\n4664\t318599502\t950,500000\t498,750000\t500,000000\r\n4665\t318601203\t950,500000\t497,500000\t500,000000\r\n4666\t318602897\t948,000000\t498,750000\t500,000000\r\n4667\t318604598\t946,000000\t498,250000\t500,000000\r\n4668\t318606293\t951,500000\t497,750000\t500,000000\r\n4669\t318607993\t949,500000\t498,250000\t500,000000\r\n4670\t318609682\t950,500000\t497,000000\t500,000000\r\n4671\t318611383\t950,000000\t498,500000\t500,000000\r\n4672\t318613084\t948,000000\t498,250000\t500,000000\r\n4673\t318614779\t949,000000\t498,000000\t500,000000\r\n4674\t318616463\t947,000000\t498,250000\t500,000000\r\n4675\t318618169\t948,500000\t497,750000\t500,000000\r\n4676\t318619876\t947,500000\t497,000000\t500,000000\r\n4677\t318621578\t947,900000\t498,000000\t500,000000\r\n4678\t318623267\t948,000000\t499,000000\t500,000000\r\n4679\t318624969\t947,000000\t497,750000\t500,000000\r\n4680\t318626674\t946,500000\t497,500000\t500,000000\r\n4681\t318628375\t948,500000\t498,250000\t500,000000\r\n4682\t318630077\t947,000000\t498,000000\t500,000000\r\n4683\t318631783\t944,400000\t498,750000\t500,000000\r\n4684\t318633468\t946,000000\t497,750000\t500,000000\r\n4685\t318635162\t948,500000\t498,500000\t500,000000\r\n4686\t318636874\t947,500000\t498,000000\t500,000000\r\n4687\t318638577\t947,500000\t498,000000\t500,000000\r\n4688\t318640281\t948,000000\t498,000000\t500,000000\r\n4689\t318641984\t947,500000\t498,250000\t500,000000\r\n4690\t318643683\t947,000000\t498,000000\t500,000000\r\n4691\t318645393\t948,000000\t498,000000\t500,000000\r\n4692\t318647090\t950,500000\t498,250000\t500,000000\r\n4693\t318648784\t948,000000\t497,250000\t500,000000\r\n4694\t318650487\t946,000000\t498,250000\t500,000000\r\n4695\t318652185\t945,500000\t498,500000\t500,000000\r\n4696\t318653878\t947,500000\t497,750000\t500,000000\r\n4697\t318655580\t945,000000\t498,250000\t500,000000\r\n4698\t318657276\t947,000000\t498,250000\t500,000000\r\n4699\t318658982\t946,500000\t498,500000\t500,000000\r\n4700\t318660625\t947,000000\t498,250000\t500,000000\r\n4701\t318662134\t946,000000\t498,250000\t500,000000\r\n4702\t318663728\t947,000000\t497,500000\t500,000000\r\n4703\t318665334\t946,000000\t498,500000\t500,000000\r\n4704\t318666831\t946,000000\t495,950000\t500,000000\r\n4705\t318668351\t947,500000\t497,250000\t500,000000\r\n4706\t318669946\t945,000000\t498,500000\t500,000000\r\n4707\t318671562\t945,000000\t498,750000\t500,000000\r\n4708\t318673152\t945,000000\t498,000000\t500,000000\r\n4709\t318674726\t945,000000\t497,750000\t500,000000\r\n4710\t318676311\t944,500000\t498,000000\t500,000000\r\n4711\t318677873\t947,500000\t498,500000\t500,000000\r\n4712\t318679438\t947,000000\t498,250000\t500,000000\r\n4713\t318680915\t943,500000\t497,500000\t500,000000\r\n4714\t318682489\t946,000000\t497,750000\t500,000000\r\n4715\t318684066\t946,000000\t498,000000\t500,000000\r\n4716\t318685561\t943,000000\t497,500000\t500,000000\r\n4717\t318687091\t946,000000\t497,500000\t500,000000\r\n4718\t318688675\t943,500000\t497,750000\t500,000000\r\n4719\t318690279\t948,500000\t497,500000\t500,000000\r\n4720\t318691767\t947,500000\t498,500000\t500,000000\r\n4721\t318693290\t947,000000\t498,250000\t500,000000\r\n4722\t318694793\t945,500000\t498,750000\t500,000000\r\n4723\t318696352\t944,500000\t498,250000\t500,000000\r\n4724\t318697915\t943,900000\t498,750000\t500,000000\r\n4725\t318699459\t943,000000\t498,250000\t500,000000\r\n4726\t318700955\t945,500000\t497,750000\t500,000000\r\n4727\t318702538\t944,000000\t498,750000\t500,000000\r\n4728\t318704092\t944,500000\t497,750000\t500,000000\r\n4729\t318705675\t942,000000\t497,750000\t500,000000\r\n4730\t318707238\t942,500000\t497,950000\t500,000000\r\n4731\t318708768\t946,000000\t498,750000\t500,000000\r\n4732\t318710258\t943,000000\t498,250000\t500,000000\r\n4733\t318711842\t944,000000\t498,000000\t500,000000\r\n4734\t318713412\t944,000000\t498,000000\t500,000000\r\n4735\t318715018\t946,500000\t497,750000\t500,000000\r\n4736\t318716592\t944,000000\t498,000000\t500,000000\r\n4737\t318718186\t943,500000\t497,500000\t500,000000\r\n4738\t318719753\t944,000000\t497,750000\t500,000000\r\n4739\t318721341\t945,500000\t498,250000\t500,000000\r\n4740\t318722915\t943,900000\t496,950000\t500,000000\r\n4741\t318724511\t943,500000\t498,750000\t500,000000\r\n4742\t318726061\t943,500000\t498,500000\t500,000000\r\n4743\t318727550\t940,000000\t498,750000\t500,000000\r\n4744\t318729081\t943,000000\t497,500000\t500,000000\r\n4745\t318730684\t941,000000\t499,500000\t500,000000\r\n4746\t318732269\t944,500000\t498,250000\t500,000000\r\n4747\t318733852\t941,500000\t498,500000\t500,000000\r\n4748\t318735411\t941,500000\t498,750000\t500,000000\r\n4749\t318737019\t943,500000\t497,750000\t500,000000\r\n4750\t318738602\t945,000000\t498,000000\t500,000000\r\n4751\t318740185\t942,000000\t497,750000\t500,000000\r\n4752\t318741758\t941,000000\t499,000000\t500,000000\r\n4753\t318743352\t941,500000\t500,000000\t500,000000\r\n4754\t318744878\t941,500000\t498,250000\t500,000000\r\n4755\t318746383\t944,000000\t498,500000\t500,000000\r\n4756\t318747953\t941,500000\t498,250000\t500,000000\r\n4757\t318749455\t941,500000\t498,250000\t500,000000\r\n4758\t318750978\t942,500000\t498,250000\t500,000000\r\n4759\t318752581\t942,500000\t497,750000\t500,000000\r\n4760\t318754038\t940,500000\t498,000000\t500,000000\r\n4761\t318755570\t939,500000\t498,500000\t500,000000\r\n4762\t318757143\t942,000000\t498,250000\t500,000000\r\n4763\t318758695\t943,500000\t498,500000\t500,000000\r\n4764\t318760279\t942,500000\t498,500000\t500,000000\r\n4765\t318761839\t941,500000\t498,000000\t500,000000\r\n4766\t318763418\t941,000000\t498,000000\t500,000000\r\n4767\t318764934\t939,500000\t498,250000\t500,000000\r\n4768\t318766467\t942,000000\t498,000000\t500,000000\r\n4769\t318768019\t940,000000\t497,750000\t500,000000\r\n4770\t318769588\t940,000000\t498,000000\t500,000000\r\n4771\t318771100\t940,000000\t498,000000\t500,000000\r\n4772\t318772623\t942,000000\t498,250000\t500,000000\r\n4773\t318774197\t940,500000\t498,000000\t500,000000\r\n4774\t318775685\t940,000000\t498,250000\t500,000000\r\n4775\t318777232\t939,500000\t498,000000\t500,000000\r\n4776\t318778816\t940,000000\t498,500000\t500,000000\r\n4777\t318780395\t941,000000\t498,000000\t500,000000\r\n4778\t318781957\t941,500000\t497,750000\t500,000000\r\n4779\t318783496\t943,000000\t496,950000\t500,000000\r\n4780\t318784999\t939,500000\t499,250000\t500,000000\r\n4781\t318786536\t942,500000\t498,500000\t500,000000\r\n4782\t318788024\t937,400000\t498,250000\t500,000000\r\n4783\t318789571\t940,000000\t498,250000\t500,000000\r\n4784\t318791144\t941,000000\t497,500000\t500,000000\r\n4785\t318792724\t942,500000\t498,250000\t500,000000\r\n4786\t318794342\t939,500000\t498,250000\t500,000000\r\n4787\t318795914\t939,000000\t498,750000\t500,000000\r\n4788\t318797477\t938,500000\t498,750000\t500,000000\r\n4789\t318798983\t937,000000\t498,000000\t500,000000\r\n4790\t318800519\t941,000000\t498,000000\t500,000000\r\n4791\t318802081\t939,500000\t498,250000\t500,000000\r\n4792\t318803644\t936,400000\t497,500000\t500,000000\r\n4793\t318805165\t938,000000\t497,500000\t500,000000\r\n4794\t318806664\t939,000000\t497,750000\t500,000000\r\n4795\t318808247\t939,500000\t499,500000\t500,000000\r\n4796\t318809794\t935,900000\t498,500000\t500,000000\r\n4797\t318811289\t940,500000\t498,250000\t500,000000\r\n4798\t318812875\t939,500000\t498,500000\t500,000000\r\n4799\t318814466\t938,000000\t497,500000\t500,000000\r\n4800\t318815998\t936,900000\t499,000000\t500,000000\r\n4801\t318817517\t939,000000\t497,750000\t500,000000\r\n4802\t318818998\t935,900000\t498,250000\t500,000000\r\n4803\t318820561\t934,900000\t498,250000\t500,000000\r\n4804\t318822093\t936,400000\t498,000000\t500,000000\r\n4805\t318823591\t938,000000\t498,000000\t500,000000\r\n4806\t318825155\t936,500000\t498,000000\t500,000000\r\n4807\t318826717\t935,500000\t496,950000\t500,000000\r\n4808\t318828290\t936,400000\t497,000000\t500,000000\r\n4809\t318829788\t937,000000\t497,750000\t500,000000\r\n4810\t318831321\t936,500000\t497,500000\t500,000000\r\n4811\t318832884\t936,300000\t497,500000\t500,000000\r\n4812\t318834428\t938,500000\t498,250000\t500,000000\r\n4813\t318835935\t940,000000\t497,500000\t500,000000\r\n4814\t318837509\t935,500000\t498,000000\t500,000000\r\n4815\t318839071\t936,800000\t497,500000\t500,000000\r\n4816\t318840643\t935,800000\t498,000000\t500,000000\r\n4817\t318842143\t936,400000\t498,500000\t500,000000\r\n4818\t318843695\t935,400000\t498,250000\t500,000000\r\n4819\t318845281\t935,300000\t498,500000\t500,000000\r\n4820\t318846862\t935,200000\t499,000000\t500,000000\r\n4821\t318848428\t934,300000\t498,500000\t500,000000\r\n4822\t318849915\t935,900000\t497,750000\t500,000000\r\n4823\t318851478\t937,500000\t497,750000\t500,000000\r\n4824\t318853017\t934,800000\t498,250000\t500,000000\r\n4825\t318854613\t934,800000\t498,000000\t500,000000\r\n4826\t318856113\t934,900000\t498,250000\t500,000000\r\n4827\t318857633\t935,900000\t498,250000\t500,000000\r\n4828\t318859171\t936,400000\t498,500000\t500,000000\r\n4829\t318860675\t938,000000\t498,000000\t500,000000\r\n4830\t318862269\t936,900000\t498,000000\t500,000000\r\n4831\t318863832\t934,700000\t498,250000\t500,000000\r\n4832\t318865426\t935,400000\t497,450000\t500,000000\r\n4833\t318867030\t934,200000\t498,750000\t500,000000\r\n4834\t318868579\t933,200000\t497,750000\t500,000000\r\n4835\t318870073\t934,900000\t497,250000\t500,000000\r\n4836\t318871593\t935,900000\t497,750000\t500,000000\r\n4837\t318873156\t934,800000\t499,000000\t500,000000\r\n4838\t318874760\t933,700000\t497,750000\t500,000000\r\n4839\t318876375\t933,700000\t497,750000\t500,000000\r\n4840\t318877958\t932,000000\t497,500000\t500,000000\r\n4841\t318879502\t934,700000\t498,000000\t500,000000\r\n4842\t318881102\t931,500000\t498,000000\t500,000000\r\n4843\t318882709\t932,500000\t498,500000\t500,000000\r\n4844\t318884289\t934,700000\t497,750000\t500,000000\r\n4845\t318885840\t932,500000\t497,500000\t500,000000\r\n4846\t318887467\t932,500000\t498,250000\t500,000000\r\n4847\t318889049\t930,300000\t498,000000\t500,000000\r\n4848\t318890668\t930,300000\t498,250000\t500,000000\r\n4849\t318892299\t929,700000\t498,500000\t500,000000\r\n4850\t318893894\t930,900000\t499,000000\t500,000000\r\n4851\t318895509\t934,000000\t498,500000\t500,000000\r\n4852\t318897123\t929,600000\t497,500000\t500,000000\r\n4853\t318898676\t933,100000\t497,750000\t500,000000\r\n4854\t318900248\t933,700000\t497,250000\t500,000000\r\n4855\t318901884\t930,900000\t497,750000\t500,000000\r\n4856\t318903404\t931,900000\t498,000000\t500,000000\r\n4857\t318904963\t930,400000\t498,750000\t500,000000\r\n4858\t318906572\t930,900000\t498,750000\t500,000000\r\n4859\t318908113\t931,000000\t498,250000\t500,000000\r\n4860\t318909645\t931,900000\t498,250000\t500,000000\r\n4861\t318911128\t934,600000\t498,000000\t500,000000\r\n4862\t318912696\t928,600000\t498,500000\t500,000000\r\n4863\t318914268\t930,200000\t497,750000\t500,000000\r\n4864\t318915878\t929,300000\t498,250000\t500,000000\r\n4865\t318917575\t930,800000\t497,750000\t500,000000\r\n4866\t318919278\t930,400000\t498,000000\t500,000000\r\n4867\t318920974\t928,800000\t498,250000\t500,000000\r\n4868\t318922676\t933,000000\t499,000000\t500,000000\r\n4869\t318924374\t928,200000\t498,000000\t500,000000\r\n4870\t318926072\t929,800000\t497,750000\t500,000000\r\n4871\t318927766\t930,300000\t498,000000\t500,000000\r\n4872\t318929473\t929,300000\t498,000000\t500,000000\r\n4873\t318931166\t927,700000\t498,000000\t500,000000\r\n4874\t318932866\t928,800000\t498,250000\t500,000000\r\n4875\t318934496\t928,700000\t497,750000\t500,000000\r\n4876\t318935961\t932,900000\t499,000000\t500,000000\r\n4877\t318937508\t928,100000\t497,750000\t500,000000\r\n4878\t318939063\t927,600000\t497,500000\t500,000000\r\n4879\t318940540\t926,600000\t498,250000\t500,000000\r\n4880\t318942092\t929,700000\t497,750000\t500,000000\r\n4881\t318943655\t927,600000\t497,750000\t500,000000\r\n4882\t318945186\t928,200000\t497,500000\t500,000000\r\n4883\t318946711\t930,300000\t498,750000\t500,000000\r\n4884\t318948290\t928,200000\t498,250000\t500,000000\r\n4885\t318949834\t927,100000\t497,750000\t500,000000\r\n4886\t318951350\t927,600000\t498,250000\t500,000000\r\n4887\t318952915\t928,300000\t498,250000\t500,000000\r\n4888\t318954499\t926,100000\t498,000000\t500,000000\r\n4889\t318956061\t928,700000\t498,500000\t500,000000\r\n4890\t318957655\t926,100000\t497,750000\t500,000000\r\n4891\t318959133\t925,000000\t497,500000\t500,000000\r\n4892\t318960656\t927,300000\t498,250000\t500,000000\r\n4893\t318962186\t926,500000\t497,250000\t500,000000\r\n4894\t318963705\t924,500000\t498,250000\t500,000000\r\n4895\t318965258\t925,000000\t498,750000\t500,000000\r\n4896\t318966803\t927,700000\t498,250000\t500,000000\r\n4897\t318968319\t929,200000\t498,000000\t500,000000\r\n4898\t318969842\t925,000000\t498,500000\t500,000000\r\n4899\t318971417\t927,600000\t498,000000\t500,000000\r\n4900\t318972984\t928,200000\t497,750000\t500,000000\r\n4901\t318974558\t926,600000\t498,750000\t500,000000\r\n4902\t318976051\t926,600000\t498,250000\t500,000000\r\n4903\t318977613\t926,500000\t498,500000\t500,000000\r\n4904\t318979157\t927,200000\t497,750000\t500,000000\r\n4905\t318980655\t927,200000\t498,000000\t500,000000\r\n4906\t318982217\t926,600000\t497,500000\t500,000000\r\n4907\t318983776\t926,100000\t498,000000\t500,000000\r\n4908\t318985358\t927,600000\t497,450000\t500,000000\r\n4909\t318986920\t926,100000\t497,500000\t500,000000\r\n4910\t318988488\t925,600000\t497,750000\t500,000000\r\n4911\t318990018\t923,500000\t498,500000\t500,000000\r\n4912\t318991571\t928,100000\t498,000000\t500,000000\r\n4913\t318993144\t924,200000\t498,250000\t500,000000\r\n4914\t318994697\t925,500000\t497,750000\t500,000000\r\n4915\t318996252\t924,100000\t497,750000\t500,000000\r\n4916\t318997748\t924,100000\t498,750000\t500,000000\r\n4917\t318999322\t923,500000\t497,750000\t500,000000\r\n4918\t319000894\t924,600000\t498,500000\t500,000000\r\n4919\t319002404\t925,000000\t498,250000\t500,000000\r\n4920\t319003925\t924,500000\t498,250000\t500,000000\r\n4921\t319005478\t925,100000\t497,250000\t500,000000\r\n4922\t319006987\t924,500000\t496,700000\t500,000000\r\n4923\t319008563\t927,800000\t498,250000\t500,000000\r\n4924\t319010042\t924,500000\t497,750000\t500,000000\r\n4925\t319011624\t925,200000\t498,500000\t500,000000\r\n4926\t319013150\t925,600000\t498,250000\t500,000000\r\n4927\t319014685\t924,500000\t497,500000\t500,000000\r\n4928\t319016186\t924,000000\t497,250000\t500,000000\r\n4929\t319017746\t923,000000\t498,000000\t500,000000\r\n4930\t319019343\t926,200000\t498,250000\t500,000000\r\n4931\t319020872\t922,500000\t498,500000\t500,000000\r\n4932\t319022390\t925,100000\t498,250000\t500,000000\r\n4933\t319023968\t924,500000\t498,500000\t500,000000\r\n4934\t319025540\t924,600000\t498,250000\t500,000000\r\n4935\t319027050\t921,500000\t497,500000\t500,000000\r\n4936\t319028566\t922,000000\t498,500000\t500,000000\r\n4937\t319030144\t924,100000\t498,750000\t500,000000\r\n4938\t319031718\t922,500000\t497,750000\t500,000000\r\n4939\t319033215\t923,000000\t498,000000\t500,000000\r\n4940\t319034758\t922,500000\t498,000000\t500,000000\r\n4941\t319036332\t923,100000\t497,500000\t500,000000\r\n4942\t319037905\t922,600000\t498,250000\t500,000000\r\n4943\t319039529\t921,600000\t497,750000\t500,000000\r\n4944\t319041113\t923,500000\t496,450000\t500,000000\r\n4945\t319042697\t921,100000\t497,250000\t500,000000\r\n4946\t319044273\t920,500000\t497,500000\t500,000000\r\n4947\t319045820\t923,000000\t498,250000\t500,000000\r\n4948\t319047404\t921,000000\t498,500000\t500,000000\r\n4949\t319048978\t922,600000\t497,500000\t500,000000\r\n4950\t319050476\t923,100000\t497,750000\t500,000000\r\n4951\t319051998\t918,500000\t498,000000\t500,000000\r\n4952\t319053546\t922,600000\t497,750000\t500,000000\r\n4953\t319055108\t921,000000\t497,000000\t500,000000\r\n4954\t319056707\t921,000000\t498,750000\t500,000000\r\n4955\t319058300\t921,500000\t498,250000\t500,000000\r\n4956\t319059874\t919,500000\t498,750000\t500,000000\r\n4957\t319061437\t918,500000\t498,000000\t500,000000\r\n4958\t319063041\t922,000000\t498,250000\t500,000000\r\n4959\t319064604\t916,500000\t497,750000\t500,000000\r\n4960\t319066128\t918,100000\t498,750000\t500,000000\r\n4961\t319067643\t921,000000\t497,750000\t500,000000\r\n4962\t319069218\t918,500000\t498,250000\t500,000000\r\n4963\t319070799\t920,500000\t499,000000\t500,000000\r\n4964\t319072351\t920,000000\t498,250000\t500,000000\r\n4965\t319073881\t918,500000\t498,250000\t500,000000\r\n4966\t319075425\t920,000000\t497,750000\t500,000000\r\n4967\t319076999\t921,500000\t497,750000\t500,000000\r\n4968\t319078573\t919,500000\t498,000000\t500,000000\r\n4969\t319080142\t920,500000\t497,750000\t500,000000\r\n4970\t319081718\t921,000000\t498,000000\t500,000000\r\n4971\t319083249\t919,000000\t497,750000\t500,000000\r\n4972\t319084874\t919,500000\t497,000000\t500,000000\r\n4973\t319086463\t919,000000\t498,500000\t500,000000\r\n4974\t319088108\t920,000000\t498,750000\t500,000000\r\n4975\t319089717\t919,000000\t498,500000\t500,000000\r\n4976\t319091307\t920,500000\t497,200000\t500,000000\r\n4977\t319092887\t918,500000\t497,750000\t500,000000\r\n4978\t319094489\t917,500000\t498,000000\t500,000000\r\n4979\t319096082\t918,500000\t498,000000\t500,000000\r\n4980\t319097656\t918,000000\t498,250000\t500,000000\r\n4981\t319099254\t918,500000\t497,500000\t500,000000\r\n4982\t319100819\t917,500000\t498,000000\t500,000000\r\n4983\t319102374\t918,000000\t497,750000\t500,000000\r\n4984\t319104021\t916,500000\t497,750000\t500,000000\r\n4985\t319105588\t918,500000\t498,000000\t500,000000\r\n4986\t319107136\t920,000000\t499,000000\t500,000000\r\n4987\t319108760\t917,000000\t498,000000\t500,000000\r\n4988\t319110376\t915,500000\t498,000000\t500,000000\r\n4989\t319111996\t915,500000\t497,200000\t500,000000\r\n4990\t319113623\t915,000000\t497,750000\t500,000000\r\n4991\t319115219\t915,500000\t498,500000\t500,000000\r\n4992\t319116836\t918,000000\t497,750000\t500,000000\r\n4993\t319118395\t917,500000\t499,000000\t500,000000\r\n4994\t319119947\t916,000000\t498,250000\t500,000000\r\n4995\t319121550\t915,500000\t498,250000\t500,000000\r\n4996\t319123156\t915,000000\t498,250000\t500,000000\r\n4997\t319124746\t916,000000\t498,250000\t500,000000\r\n4998\t319126396\t914,000000\t498,500000\t500,000000\r\n4999\t319127977\t917,000000\t498,250000\t500,000000\r\n5000\t319129578\t916,500000\t498,000000\t500,000000\r\n5001\t319131156\t917,500000\t498,250000\t500,000000\r\n5002\t319132760\t914,500000\t498,250000\t500,000000\r\n5003\t319134338\t914,500000\t498,250000\t500,000000\r\n5004\t319135920\t914,500000\t498,250000\t500,000000\r\n5005\t319137497\t917,000000\t498,250000\t500,000000\r\n5006\t319139135\t913,500000\t498,500000\t500,000000\r\n5007\t319140731\t914,500000\t497,500000\t500,000000\r\n5008\t319142270\t915,000000\t498,000000\t500,000000\r\n5009\t319143830\t913,000000\t499,500000\t500,000000\r\n5010\t319145429\t913,500000\t497,500000\t500,000000\r\n5011\t319147000\t915,000000\t497,750000\t500,000000\r\n5012\t319148585\t915,000000\t497,750000\t500,000000\r\n5013\t319150127\t914,500000\t497,250000\t500,000000\r\n5014\t319151683\t912,000000\t497,750000\t500,000000\r\n5015\t319153223\t913,500000\t497,750000\t500,000000\r\n5016\t319154748\t912,500000\t497,750000\t500,000000\r\n5017\t319156265\t914,500000\t498,000000\t500,000000\r\n5018\t319157784\t914,500000\t498,000000\t500,000000\r\n5019\t319159350\t915,000000\t498,500000\t500,000000\r\n5020\t319160879\t912,000000\t498,250000\t500,000000\r\n5021\t319162419\t914,000000\t498,250000\t500,000000\r\n5022\t319163982\t913,000000\t498,250000\t500,000000\r\n5023\t319165534\t912,000000\t499,000000\t500,000000\r\n5024\t319167118\t912,500000\t497,250000\t500,000000\r\n5025\t319168725\t914,000000\t498,500000\t500,000000\r\n5026\t319170295\t912,000000\t496,450000\t500,000000\r\n5027\t319171879\t914,000000\t498,250000\t500,000000\r\n5028\t319173431\t913,500000\t498,000000\t500,000000\r\n5029\t319175043\t912,500000\t498,000000\t500,000000\r\n5030\t319176582\t914,000000\t498,000000\t500,000000\r\n5031\t319178176\t912,500000\t498,750000\t500,000000\r\n5032\t319179741\t911,000000\t497,250000\t500,000000\r\n5033\t319181316\t914,000000\t498,000000\t500,000000\r\n5034\t319182894\t909,000000\t498,250000\t500,000000\r\n5035\t319184481\t911,000000\t498,000000\t500,000000\r\n5036\t319186022\t911,000000\t497,750000\t500,000000\r\n5037\t319187651\t910,500000\t498,500000\t500,000000\r\n5038\t319189252\t908,000000\t497,750000\t500,000000\r\n5039\t319190858\t911,500000\t498,000000\t500,000000\r\n5040\t319192481\t908,500000\t498,250000\t500,000000\r\n5041\t319194036\t912,500000\t497,450000\t500,000000\r\n5042\t319195617\t908,500000\t497,750000\t500,000000\r\n5043\t319197190\t908,000000\t497,500000\t500,000000\r\n5044\t319198797\t912,500000\t498,250000\t500,000000\r\n5045\t319200342\t908,000000\t496,700000\t500,000000\r\n5046\t319201931\t909,500000\t498,750000\t500,000000\r\n5047\t319203547\t909,500000\t498,000000\t500,000000\r\n5048\t319205110\t906,500000\t498,000000\t500,000000\r\n5049\t319206725\t909,000000\t498,500000\t500,000000\r\n5050\t319208271\t907,000000\t496,950000\t500,000000\r\n5051\t319209856\t907,500000\t498,250000\t500,000000\r\n5052\t319211439\t907,000000\t497,750000\t500,000000\r\n5053\t319212995\t909,000000\t498,250000\t500,000000\r\n5054\t319214598\t908,500000\t498,250000\t500,000000\r\n5055\t319216157\t907,000000\t497,250000\t500,000000\r\n5056\t319217744\t909,500000\t498,250000\t500,000000\r\n5057\t319219421\t907,000000\t498,000000\t500,000000\r\n5058\t319221096\t907,000000\t498,500000\t500,000000\r\n5059\t319222794\t907,000000\t498,000000\t500,000000\r\n5060\t319224426\t907,500000\t497,500000\t500,000000\r\n5061\t319226020\t905,000000\t497,500000\t500,000000\r\n5062\t319227593\t907,500000\t498,750000\t500,000000\r\n5063\t319229126\t907,500000\t498,500000\t500,000000\r\n5064\t319230603\t908,000000\t497,500000\t500,000000\r\n5065\t319232187\t908,000000\t498,750000\t500,000000\r\n5066\t319233750\t906,500000\t498,000000\t500,000000\r\n5067\t319235343\t908,000000\t498,500000\t500,000000\r\n5068\t319236922\t907,000000\t497,500000\t500,000000\r\n5069\t319238483\t910,100000\t497,500000\t500,000000\r\n5070\t319239979\t905,500000\t497,750000\t500,000000\r\n5071\t319241509\t906,500000\t498,500000\t500,000000\r\n5072\t319243022\t905,000000\t497,950000\t500,000000\r\n5073\t319244531\t908,500000\t498,000000\t500,000000\r\n5074\t319246114\t907,000000\t497,500000\t500,000000\r\n5075\t319247638\t904,000000\t499,000000\t500,000000\r\n5076\t319249156\t908,000000\t498,000000\t500,000000\r\n5077\t319250733\t906,500000\t498,250000\t500,000000\r\n5078\t319252333\t908,500000\t498,250000\t500,000000\r\n5079\t319253832\t904,500000\t497,750000\t500,000000\r\n5080\t319255364\t906,500000\t497,250000\t500,000000\r\n5081\t319256872\t906,000000\t498,250000\t500,000000\r\n5082\t319258372\t906,500000\t498,250000\t500,000000\r\n5083\t319259929\t905,500000\t496,500000\t500,000000\r\n5084\t319261425\t903,500000\t497,500000\t500,000000\r\n5085\t319262999\t904,000000\t498,250000\t500,000000\r\n5086\t319264561\t906,000000\t497,750000\t500,000000\r\n5087\t319266096\t905,500000\t498,750000\t500,000000\r\n5088\t319267583\t904,500000\t498,250000\t500,000000\r\n5089\t319269124\t905,000000\t498,250000\t500,000000\r\n5090\t319270728\t904,000000\t499,000000\t500,000000\r\n5091\t319272228\t904,500000\t498,000000\t500,000000\r\n5092\t319273756\t905,000000\t499,000000\t500,000000\r\n5093\t319275309\t905,500000\t498,250000\t500,000000\r\n5094\t319276790\t907,000000\t498,000000\t500,000000\r\n5095\t319278322\t903,000000\t498,500000\t500,000000\r\n5096\t319279927\t904,500000\t497,750000\t500,000000\r\n5097\t319281510\t905,000000\t497,500000\t500,000000\r\n5098\t319283073\t905,000000\t498,500000\t500,000000\r\n5099\t319284642\t903,000000\t498,750000\t500,000000\r\n5100\t319286123\t905,000000\t498,250000\t500,000000\r\n5101\t319287677\t902,500000\t498,000000\t500,000000\r\n5102\t319289260\t904,000000\t497,700000\t500,000000\r\n5103\t319290854\t901,500000\t499,000000\t500,000000\r\n5104\t319292416\t905,500000\t496,950000\t500,000000\r\n5105\t319293971\t902,500000\t497,500000\t500,000000\r\n5106\t319295553\t903,000000\t497,750000\t500,000000\r\n5107\t319297045\t902,000000\t498,500000\t500,000000\r\n5108\t319298478\t900,500000\t498,000000\t500,000000\r\n5109\t319299912\t902,000000\t497,750000\t500,000000\r\n5110\t319301379\t903,500000\t498,000000\t500,000000\r\n5111\t319303080\t903,000000\t498,000000\t500,000000\r\n5112\t319304783\t901,500000\t498,250000\t500,000000\r\n5113\t319306477\t901,500000\t497,500000\t500,000000\r\n5114\t319308171\t899,500000\t497,500000\t500,000000\r\n5115\t319309864\t901,500000\t497,750000\t500,000000\r\n5116\t319311554\t901,500000\t497,750000\t500,000000\r\n5117\t319313255\t904,000000\t498,000000\t500,000000\r\n5118\t319314957\t901,000000\t498,000000\t500,000000\r\n5119\t319316649\t902,000000\t497,750000\t500,000000\r\n5120\t319318354\t904,000000\t497,750000\t500,000000\r\n5121\t319320054\t900,000000\t497,250000\t500,000000\r\n5122\t319321758\t902,500000\t497,450000\t500,000000\r\n5123\t319323451\t902,000000\t498,250000\t500,000000\r\n5124\t319325154\t900,500000\t496,950000\t500,000000\r\n5125\t319326860\t901,000000\t498,500000\t500,000000\r\n5126\t319328565\t901,500000\t499,250000\t500,000000\r\n5127\t319330270\t899,500000\t497,500000\t500,000000\r\n5128\t319331968\t899,000000\t498,250000\t500,000000\r\n5129\t319333662\t899,500000\t498,000000\t500,000000\r\n5130\t319335358\t897,500000\t497,750000\t500,000000\r\n5131\t319337053\t899,000000\t498,750000\t500,000000\r\n5132\t319338753\t899,000000\t498,750000\t500,000000\r\n5133\t319340454\t897,500000\t498,500000\t500,000000\r\n5134\t319342146\t899,500000\t498,000000\t500,000000\r\n5135\t319343846\t902,000000\t498,750000\t500,000000\r\n5136\t319345546\t898,000000\t498,500000\t500,000000\r\n5137\t319347248\t899,000000\t498,250000\t500,000000\r\n5138\t319348940\t898,500000\t498,500000\t500,000000\r\n5139\t319350640\t896,500000\t497,750000\t500,000000\r\n5140\t319352336\t900,000000\t497,750000\t500,000000\r\n5141\t319354037\t896,500000\t498,000000\t500,000000\r\n5142\t319355739\t897,000000\t497,250000\t500,000000\r\n5143\t319357439\t896,500000\t498,000000\t500,000000\r\n5144\t319359133\t898,500000\t498,000000\t500,000000\r\n5145\t319360831\t897,000000\t498,750000\t500,000000\r\n5146\t319362528\t897,000000\t498,250000\t500,000000\r\n5147\t319364238\t895,000000\t497,000000\t500,000000\r\n5148\t319365940\t896,500000\t498,000000\t500,000000\r\n5149\t319367646\t896,500000\t499,250000\t500,000000\r\n5150\t319369341\t896,000000\t498,500000\t500,000000\r\n5151\t319371042\t897,000000\t497,500000\t500,000000\r\n5152\t319372747\t894,500000\t498,000000\t500,000000\r\n5153\t319374446\t895,000000\t498,500000\t500,000000\r\n5154\t319376142\t894,500000\t499,250000\t500,000000\r\n5155\t319377832\t895,000000\t497,750000\t500,000000\r\n5156\t319379532\t895,000000\t497,750000\t500,000000\r\n5157\t319381222\t896,000000\t498,000000\t500,000000\r\n5158\t319382922\t895,500000\t497,750000\t500,000000\r\n5159\t319384615\t893,500000\t498,750000\t500,000000\r\n5160\t319386317\t899,000000\t497,750000\t500,000000\r\n5161\t319388020\t894,500000\t497,500000\t500,000000\r\n5162\t319389716\t895,500000\t498,000000\t500,000000\r\n5163\t319391421\t897,500000\t498,500000\t500,000000\r\n5164\t319393123\t895,500000\t498,500000\t500,000000\r\n5165\t319394823\t894,000000\t498,000000\t500,000000\r\n5166\t319396524\t895,000000\t497,750000\t500,000000\r\n5167\t319398218\t895,500000\t498,250000\t500,000000\r\n5168\t319399914\t892,000000\t498,000000\t500,000000\r\n5169\t319401615\t893,000000\t498,750000\t500,000000\r\n5170\t319403303\t894,000000\t499,000000\t500,000000\r\n5171\t319405006\t894,500000\t498,250000\t500,000000\r\n5172\t319406697\t893,500000\t498,500000\t500,000000\r\n5173\t319408396\t890,500000\t499,000000\t500,000000\r\n5174\t319410091\t891,000000\t497,750000\t500,000000\r\n5175\t319411787\t890,500000\t498,000000\t500,000000\r\n5176\t319413489\t893,000000\t497,750000\t500,000000\r\n5177\t319415189\t891,000000\t498,250000\t500,000000\r\n5178\t319416889\t889,500000\t497,500000\t500,000000\r\n5179\t319418578\t891,000000\t497,500000\t500,000000\r\n5180\t319420274\t890,500000\t498,250000\t500,000000\r\n5181\t319421968\t891,500000\t499,000000\t500,000000\r\n5182\t319423662\t890,500000\t498,750000\t500,000000\r\n5183\t319425362\t888,500000\t497,500000\t500,000000\r\n5184\t319427069\t888,400000\t498,500000\t500,000000\r\n5185\t319428772\t887,500000\t498,750000\t500,000000\r\n5186\t319430477\t891,500000\t497,200000\t500,000000\r\n5187\t319432168\t888,000000\t497,250000\t500,000000\r\n5188\t319433867\t887,500000\t497,500000\t500,000000\r\n5189\t319435553\t888,000000\t498,500000\t500,000000\r\n5190\t319437078\t888,500000\t498,000000\t500,000000\r\n5191\t319438563\t888,000000\t497,750000\t500,000000\r\n5192\t319440078\t887,500000\t497,750000\t500,000000\r\n5193\t319441582\t888,500000\t498,500000\t500,000000\r\n5194\t319443088\t890,000000\t497,750000\t500,000000\r\n5195\t319444595\t889,000000\t498,750000\t500,000000\r\n5196\t319446093\t887,000000\t498,250000\t500,000000\r\n5197\t319447574\t889,000000\t498,000000\t500,000000\r\n5198\t319449062\t888,500000\t498,750000\t500,000000\r\n5199\t319450634\t887,500000\t498,250000\t500,000000\r\n5200\t319452125\t886,000000\t497,750000\t500,000000\r\n5201\t319453655\t887,000000\t497,500000\t500,000000\r\n5202\t319455266\t886,500000\t498,250000\t500,000000\r\n5203\t319456951\t888,500000\t497,500000\t500,000000\r\n5204\t319458655\t884,500000\t497,500000\t500,000000\r\n5205\t319460365\t887,000000\t498,000000\t500,000000\r\n5206\t319461944\t886,000000\t498,000000\t500,000000\r\n5207\t319463457\t886,400000\t499,000000\t500,000000\r\n5208\t319465027\t887,400000\t499,000000\t500,000000\r\n5209\t319466604\t887,400000\t498,250000\t500,000000\r\n5210\t319468125\t886,000000\t498,500000\t500,000000\r\n5211\t319469614\t886,500000\t497,500000\t500,000000\r\n5212\t319471146\t887,000000\t498,000000\t500,000000\r\n5213\t319472644\t884,900000\t497,750000\t500,000000\r\n5214\t319474156\t884,900000\t498,000000\t500,000000\r\n5215\t319475645\t885,900000\t497,500000\t500,000000\r\n5216\t319477134\t887,500000\t498,500000\t500,000000\r\n5217\t319478688\t885,500000\t498,250000\t500,000000\r\n5218\t319480260\t885,000000\t497,500000\t500,000000\r\n5219\t319481810\t886,400000\t498,000000\t500,000000\r\n5220\t319483280\t885,300000\t497,250000\t500,000000\r\n5221\t319484944\t885,400000\t498,500000\t500,000000\r\n5222\t319486512\t885,400000\t497,750000\t500,000000\r\n5223\t319488074\t884,900000\t498,500000\t500,000000\r\n5224\t319489654\t883,700000\t498,750000\t500,000000\r\n5225\t319491225\t884,300000\t496,950000\t500,000000\r\n5226\t319492706\t883,800000\t497,750000\t500,000000\r\n5227\t319494263\t883,900000\t498,250000\t500,000000\r\n5228\t319495814\t885,900000\t498,250000\t500,000000\r\n5229\t319497291\t884,800000\t498,500000\t500,000000\r\n5230\t319498823\t882,100000\t497,250000\t500,000000\r\n5231\t319500394\t883,800000\t498,500000\t500,000000\r\n5232\t319501963\t885,800000\t498,000000\t500,000000\r\n5233\t319503540\t883,700000\t498,250000\t500,000000\r\n5234\t319505073\t884,300000\t498,250000\t500,000000\r\n5235\t319506555\t881,600000\t497,750000\t500,000000\r\n5236\t319508144\t882,100000\t498,750000\t500,000000\r\n5237\t319509683\t883,800000\t498,000000\t500,000000\r\n5238\t319511168\t882,100000\t498,250000\t500,000000\r\n5239\t319512740\t882,100000\t498,250000\t500,000000\r\n5240\t319514442\t884,400000\t498,250000\t500,000000\r\n5241\t319516148\t884,900000\t498,250000\t500,000000\r\n5242\t319517849\t879,900000\t497,500000\t500,000000\r\n5243\t319519404\t881,500000\t498,250000\t500,000000\r\n5244\t319520958\t881,000000\t497,750000\t500,000000\r\n5245\t319522548\t881,500000\t498,250000\t500,000000\r\n5246\t319524154\t880,900000\t498,250000\t500,000000\r\n5247\t319525707\t880,500000\t497,500000\t500,000000\r\n5248\t319527260\t879,800000\t497,500000\t500,000000\r\n5249\t319528821\t880,800000\t497,750000\t500,000000\r\n5250\t319530385\t879,900000\t498,000000\t500,000000\r\n5251\t319531832\t879,400000\t498,000000\t500,000000\r\n5252\t319533401\t878,800000\t498,250000\t500,000000\r\n5253\t319535054\t880,500000\t498,250000\t500,000000\r\n5254\t319536765\t879,200000\t498,000000\t500,000000\r\n5255\t319538475\t876,500000\t499,500000\t500,000000\r\n5256\t319540189\t880,300000\t498,500000\t500,000000\r\n5257\t319541904\t880,500000\t498,750000\t500,000000\r\n5258\t319543612\t882,000000\t498,250000\t500,000000\r\n5259\t319545324\t880,300000\t498,750000\t500,000000\r\n5260\t319547026\t877,100000\t499,500000\t500,000000\r\n5261\t319548735\t877,600000\t498,250000\t500,000000\r\n5262\t319550425\t877,100000\t498,500000\t500,000000\r\n5263\t319552119\t877,700000\t497,750000\t500,000000\r\n5264\t319553815\t877,700000\t497,500000\t500,000000\r\n5265\t319555512\t876,100000\t498,500000\t500,000000\r\n5266\t319557209\t875,100000\t497,500000\t500,000000\r\n5267\t319558909\t875,700000\t498,250000\t500,000000\r\n5268\t319560609\t876,100000\t497,500000\t500,000000\r\n5269\t319562308\t874,600000\t498,250000\t500,000000\r\n5270\t319564006\t875,700000\t498,250000\t500,000000\r\n5271\t319565701\t873,600000\t498,500000\t500,000000\r\n5272\t319567400\t874,600000\t498,000000\t500,000000\r\n5273\t319569096\t873,500000\t497,500000\t500,000000\r\n5274\t319570794\t874,500000\t498,000000\t500,000000\r\n5275\t319572493\t874,600000\t498,500000\t500,000000\r\n5276\t319574189\t873,500000\t497,750000\t500,000000\r\n5277\t319575880\t874,000000\t498,750000\t500,000000\r\n5278\t319577579\t873,100000\t498,000000\t500,000000\r\n5279\t319579277\t874,200000\t498,000000\t500,000000\r\n5280\t319580977\t872,100000\t498,000000\t500,000000\r\n5281\t319582683\t872,600000\t498,000000\t500,000000\r\n5282\t319584382\t871,600000\t498,000000\t500,000000\r\n5283\t319586091\t871,500000\t497,500000\t500,000000\r\n5284\t319587801\t870,500000\t498,000000\t500,000000\r\n5285\t319589363\t872,000000\t497,500000\t500,000000\r\n5286\t319590895\t871,000000\t497,250000\t500,000000\r\n5287\t319592352\t872,100000\t499,250000\t500,000000\r\n5288\t319593885\t872,500000\t498,000000\t500,000000\r\n5289\t319595545\t871,000000\t498,000000\t500,000000\r\n5290\t319597252\t872,100000\t498,250000\t500,000000\r\n5291\t319598953\t871,500000\t498,000000\t500,000000\r\n5292\t319600651\t872,000000\t497,750000\t500,000000\r\n5293\t319602355\t868,500000\t498,000000\t500,000000\r\n5294\t319604057\t872,100000\t497,750000\t500,000000\r\n5295\t319605761\t869,500000\t498,500000\t500,000000\r\n5296\t319607393\t872,000000\t497,750000\t500,000000\r\n5297\t319608904\t871,100000\t496,950000\t500,000000\r\n5298\t319610454\t871,100000\t498,500000\t500,000000\r\n5299\t319611938\t866,500000\t498,750000\t500,000000\r\n5300\t319613364\t867,000000\t498,250000\t500,000000\r\n5301\t319614778\t867,500000\t497,200000\t500,000000\r\n5302\t319616314\t866,500000\t497,250000\t500,000000\r\n5303\t319617833\t869,500000\t498,750000\t500,000000\r\n5304\t319619343\t868,500000\t498,500000\t500,000000\r\n5305\t319620803\t869,000000\t498,000000\t500,000000\r\n5306\t319622344\t867,500000\t498,750000\t500,000000\r\n5307\t319623859\t864,500000\t498,000000\t500,000000\r\n5308\t319625311\t868,500000\t497,750000\t500,000000\r\n5309\t319626815\t868,000000\t498,500000\t500,000000\r\n5310\t319628300\t865,600000\t498,000000\t500,000000\r\n5311\t319629821\t863,000000\t497,000000\t500,000000\r\n5312\t319631316\t868,500000\t497,500000\t500,000000\r\n5313\t319632858\t866,000000\t498,250000\t500,000000\r\n5314\t319634344\t864,000000\t497,750000\t500,000000\r\n5315\t319635789\t864,500000\t497,750000\t500,000000\r\n5316\t319637220\t865,500000\t499,500000\t500,000000\r\n5317\t319638667\t865,500000\t498,000000\t500,000000\r\n5318\t319640197\t864,500000\t498,500000\t500,000000\r\n5319\t319641731\t867,500000\t498,500000\t500,000000\r\n5320\t319643298\t865,000000\t498,250000\t500,000000\r\n5321\t319644847\t864,000000\t498,250000\t500,000000\r\n5322\t319646398\t863,500000\t498,750000\t500,000000\r\n5323\t319647959\t863,500000\t498,250000\t500,000000\r\n5324\t319649562\t862,000000\t498,500000\t500,000000\r\n5325\t319651110\t865,000000\t498,750000\t500,000000\r\n5326\t319652677\t862,500000\t498,250000\t500,000000\r\n5327\t319654294\t863,500000\t497,000000\t500,000000\r\n5328\t319655874\t864,500000\t498,250000\t500,000000\r\n5329\t319657477\t862,000000\t498,250000\t500,000000\r\n5330\t319659020\t862,000000\t499,250000\t500,000000\r\n5331\t319660625\t862,000000\t498,000000\t500,000000\r\n5332\t319662198\t862,500000\t497,750000\t500,000000\r\n5333\t319663750\t864,500000\t497,750000\t500,000000\r\n5334\t319665442\t858,500000\t498,000000\t500,000000\r\n5335\t319667143\t860,000000\t497,500000\t500,000000\r\n5336\t319668865\t859,500000\t496,200000\t500,000000\r\n5337\t319670560\t858,500000\t497,500000\t500,000000\r\n5338\t319672269\t859,500000\t497,750000\t500,000000\r\n5339\t319673978\t861,000000\t497,750000\t500,000000\r\n5340\t319675690\t858,500000\t498,750000\t500,000000\r\n5341\t319677388\t860,500000\t498,250000\t500,000000\r\n5342\t319679076\t860,500000\t499,000000\t500,000000\r\n5343\t319680663\t860,000000\t498,500000\t500,000000\r\n5344\t319682214\t859,500000\t498,000000\t500,000000\r\n5345\t319683792\t857,500000\t498,500000\t500,000000\r\n5346\t319685391\t855,500000\t498,000000\t500,000000\r\n5347\t319686938\t856,000000\t498,750000\t500,000000\r\n5348\t319688542\t857,500000\t497,750000\t500,000000\r\n5349\t319690115\t856,500000\t498,500000\t500,000000\r\n5350\t319691685\t858,000000\t497,250000\t500,000000\r\n5351\t319693258\t856,500000\t497,000000\t500,000000\r\n5352\t319694834\t857,500000\t498,750000\t500,000000\r\n5353\t319696395\t854,000000\t498,500000\t500,000000\r\n5354\t319697942\t854,000000\t498,000000\t500,000000\r\n5355\t319699405\t854,000000\t498,000000\t500,000000\r\n5356\t319701012\t858,000000\t498,500000\t500,000000\r\n5357\t319702707\t853,000000\t497,750000\t500,000000\r\n5358\t319704411\t854,500000\t496,450000\t500,000000\r\n5359\t319706108\t853,000000\t498,500000\t500,000000\r\n5360\t319707805\t854,000000\t497,750000\t500,000000\r\n5361\t319709507\t851,500000\t498,250000\t500,000000\r\n5362\t319711207\t855,500000\t498,250000\t500,000000\r\n5363\t319712914\t853,500000\t497,750000\t500,000000\r\n5364\t319714601\t851,500000\t497,500000\t500,000000\r\n5365\t319716302\t852,000000\t498,000000\t500,000000\r\n5366\t319718003\t848,000000\t497,750000\t500,000000\r\n5367\t319719709\t850,500000\t497,250000\t500,000000\r\n5368\t319721418\t849,500000\t498,750000\t500,000000\r\n5369\t319723120\t849,000000\t497,750000\t500,000000\r\n5370\t319724808\t848,000000\t498,000000\t500,000000\r\n5371\t319726506\t847,000000\t498,000000\t500,000000\r\n5372\t319728215\t848,000000\t498,000000\t500,000000\r\n5373\t319729911\t849,000000\t497,750000\t500,000000\r\n5374\t319731609\t848,000000\t498,000000\t500,000000\r\n5375\t319733322\t848,000000\t498,000000\t500,000000\r\n5376\t319735025\t849,500000\t497,250000\t500,000000\r\n5377\t319736735\t846,500000\t498,250000\t500,000000\r\n5378\t319738436\t845,000000\t498,200000\t500,000000\r\n5379\t319740139\t845,500000\t497,750000\t500,000000\r\n5380\t319741838\t847,000000\t497,500000\t500,000000\r\n5381\t319743537\t847,500000\t497,750000\t500,000000\r\n5382\t319745235\t845,000000\t498,000000\t500,000000\r\n5383\t319746943\t843,500000\t498,250000\t500,000000\r\n5384\t319748643\t844,000000\t497,250000\t500,000000\r\n5385\t319750344\t845,500000\t497,750000\t500,000000\r\n5386\t319752039\t845,000000\t498,500000\t500,000000\r\n5387\t319753743\t843,500000\t497,500000\t500,000000\r\n5388\t319755441\t844,000000\t498,250000\t500,000000\r\n5389\t319757145\t843,500000\t498,500000\t500,000000\r\n5390\t319758851\t840,500000\t498,250000\t500,000000\r\n5391\t319760556\t841,000000\t498,000000\t500,000000\r\n5392\t319762263\t841,500000\t497,500000\t500,000000\r\n5393\t319763965\t838,900000\t497,250000\t500,000000\r\n5394\t319765672\t840,900000\t498,000000\t500,000000\r\n5395\t319767356\t837,400000\t497,750000\t500,000000\r\n5396\t319768955\t836,800000\t497,750000\t500,000000\r\n5397\t319770588\t839,500000\t498,250000\t500,000000\r\n5398\t319772230\t839,000000\t498,500000\t500,000000\r\n5399\t319773887\t840,500000\t498,500000\t500,000000\r\n5400\t319775401\t837,000000\t498,250000\t500,000000\r\n5401\t319777001\t836,000000\t497,750000\t500,000000\r\n5402\t319778577\t837,000000\t498,250000\t500,000000\r\n5403\t319780083\t836,900000\t498,500000\t500,000000\r\n5404\t319781669\t833,800000\t498,750000\t500,000000\r\n5405\t319783272\t833,700000\t499,250000\t500,000000\r\n5406\t319784836\t834,300000\t497,750000\t500,000000\r\n5407\t319786323\t832,700000\t498,500000\t500,000000\r\n5408\t319787855\t832,800000\t498,000000\t500,000000\r\n5409\t319789407\t833,800000\t499,250000\t500,000000\r\n5410\t319790895\t832,100000\t498,250000\t500,000000\r\n5411\t319792447\t832,100000\t498,750000\t500,000000\r\n5412\t319794011\t831,600000\t497,250000\t500,000000\r\n5413\t319795594\t830,000000\t497,500000\t500,000000\r\n5414\t319797173\t828,400000\t497,500000\t500,000000\r\n5415\t319798774\t828,300000\t498,250000\t500,000000\r\n5416\t319800250\t827,800000\t497,000000\t500,000000\r\n5417\t319801813\t831,100000\t498,000000\t500,000000\r\n5418\t319803416\t826,000000\t497,750000\t500,000000\r\n5419\t319805000\t827,800000\t498,250000\t500,000000\r\n5420\t319806553\t828,300000\t498,000000\t500,000000\r\n5421\t319808127\t823,000000\t497,500000\t500,000000\r\n5422\t319809645\t828,300000\t498,250000\t500,000000\r\n5423\t319811168\t822,600000\t497,500000\t500,000000\r\n5424\t319812730\t823,600000\t498,250000\t500,000000\r\n5425\t319814296\t825,200000\t498,500000\t500,000000\r\n5426\t319815901\t821,500000\t498,000000\t500,000000\r\n5427\t319817470\t822,100000\t498,000000\t500,000000\r\n5428\t319819052\t820,600000\t498,250000\t500,000000\r\n5429\t319820606\t824,100000\t497,750000\t500,000000\r\n5430\t319822185\t824,600000\t498,000000\t500,000000\r\n5431\t319823785\t820,000000\t497,250000\t500,000000\r\n5432\t319825301\t823,600000\t497,500000\t500,000000\r\n5433\t319826855\t816,000000\t498,000000\t500,000000\r\n5434\t319828416\t819,000000\t497,750000\t500,000000\r\n5435\t319829927\t818,500000\t498,000000\t500,000000\r\n5436\t319831481\t818,000000\t497,750000\t500,000000\r\n5437\t319832955\t817,000000\t498,250000\t500,000000\r\n5438\t319834479\t814,500000\t498,250000\t500,000000\r\n5439\t319836042\t816,500000\t498,250000\t500,000000\r\n5440\t319837540\t815,500000\t497,500000\t500,000000\r\n5441\t319839083\t813,500000\t498,000000\t500,000000\r\n5442\t319840657\t813,500000\t498,750000\t500,000000\r\n5443\t319842251\t810,500000\t497,750000\t500,000000\r\n5444\t319843800\t810,000000\t497,250000\t500,000000\r\n5445\t319845381\t810,000000\t498,250000\t500,000000\r\n5446\t319846939\t813,000000\t497,750000\t500,000000\r\n5447\t319848480\t805,500000\t498,750000\t500,000000\r\n5448\t319849990\t808,000000\t497,250000\t500,000000\r\n5449\t319851532\t807,500000\t497,750000\t500,000000\r\n5450\t319853041\t806,500000\t497,750000\t500,000000\r\n5451\t319854573\t805,500000\t498,000000\t500,000000\r\n5452\t319856082\t803,500000\t498,500000\t500,000000\r\n5453\t319857605\t804,500000\t498,000000\t500,000000\r\n5454\t319859168\t802,500000\t499,000000\t500,000000\r\n5455\t319860730\t803,500000\t497,750000\t500,000000\r\n5456\t319862355\t802,500000\t497,000000\t500,000000\r\n5457\t319863938\t803,000000\t499,000000\t500,000000\r\n5458\t319865521\t800,500000\t499,000000\t500,000000\r\n5459\t319867095\t798,000000\t496,750000\t500,000000\r\n5460\t319868688\t798,000000\t497,750000\t500,000000\r\n5461\t319870256\t797,000000\t497,750000\t500,000000\r\n5462\t319871839\t794,500000\t497,200000\t500,000000\r\n5463\t319873407\t794,500000\t498,750000\t500,000000\r\n5464\t319875000\t792,900000\t497,750000\t500,000000\r\n5465\t319876596\t793,000000\t498,750000\t500,000000\r\n5466\t319878178\t790,000000\t498,000000\t500,000000\r\n5467\t319879756\t791,500000\t498,500000\t500,000000\r\n5468\t319881309\t789,500000\t498,250000\t500,000000\r\n5469\t319882886\t787,000000\t498,000000\t500,000000\r\n5470\t319884464\t786,500000\t497,750000\t500,000000\r\n5471\t319886019\t783,500000\t498,000000\t500,000000\r\n5472\t319887616\t782,400000\t497,500000\t500,000000\r\n5473\t319889218\t782,200000\t497,750000\t500,000000\r\n5474\t319890791\t780,200000\t498,750000\t500,000000\r\n5475\t319892375\t778,900000\t498,500000\t500,000000\r\n5476\t319893970\t776,700000\t498,250000\t500,000000\r\n5477\t319895541\t775,900000\t496,950000\t500,000000\r\n5478\t319897114\t774,700000\t497,500000\t500,000000\r\n5479\t319898710\t774,600000\t497,750000\t500,000000\r\n5480\t319900281\t771,000000\t497,750000\t500,000000\r\n5481\t319901865\t770,600000\t497,750000\t500,000000\r\n5482\t319903451\t769,500000\t497,750000\t500,000000\r\n5483\t319905044\t766,000000\t498,250000\t500,000000\r\n5484\t319906653\t765,000000\t498,250000\t500,000000\r\n5485\t319908292\t763,500000\t497,000000\t500,000000\r\n5486\t319909886\t760,500000\t498,000000\t500,000000\r\n5487\t319911485\t757,000000\t498,250000\t500,000000\r\n5488\t319913063\t755,000000\t497,750000\t500,000000\r\n5489\t319914660\t756,000000\t498,500000\t500,000000\r\n5490\t319916216\t752,000000\t498,500000\t500,000000\r\n5491\t319917804\t749,500000\t497,500000\t500,000000\r\n5492\t319919374\t747,000000\t497,750000\t500,000000\r\n5493\t319920953\t746,000000\t498,250000\t500,000000\r\n5494\t319922531\t741,500000\t497,750000\t500,000000\r\n5495\t319924096\t741,500000\t497,250000\t500,000000\r\n5496\t319925706\t742,500000\t497,500000\t500,000000\r\n5497\t319927243\t734,500000\t498,750000\t500,000000\r\n5498\t319928829\t731,200000\t497,250000\t500,000000\r\n5499\t319930399\t726,800000\t497,750000\t500,000000\r\n5500\t319931936\t723,700000\t497,750000\t500,000000\r\n5501\t319933524\t721,000000\t497,500000\t500,000000\r\n5502\t319935114\t721,200000\t498,750000\t500,000000\r\n5503\t319936691\t712,000000\t498,250000\t500,000000\r\n5504\t319938278\t709,500000\t497,500000\t500,000000\r\n5505\t319939870\t705,000000\t497,750000\t500,000000\r\n5506\t319941460\t704,000000\t497,000000\t500,000000\r\n5507\t319943028\t698,500000\t498,500000\t500,000000\r\n5508\t319944628\t692,500000\t498,750000\t500,000000\r\n5509\t319946213\t688,000000\t497,250000\t500,000000\r\n5510\t319947780\t684,000000\t497,500000\t500,000000\r\n5511\t319949364\t677,000000\t498,000000\t500,000000\r\n5512\t319950956\t671,100000\t497,750000\t500,000000\r\n5513\t319952479\t666,100000\t497,250000\t500,000000\r\n5514\t319954027\t657,500000\t496,500000\t500,000000\r\n5515\t319955627\t651,500000\t497,250000\t500,000000\r\n5516\t319957219\t642,500000\t497,250000\t500,000000\r\n5517\t319958730\t636,500000\t496,500000\t500,000000\r\n5518\t319960308\t626,400000\t496,000000\t500,000000\r\n5519\t319961864\t618,200000\t495,250000\t500,000000\r\n5520\t319963418\t610,000000\t494,250000\t500,000000\r\n5521\t319964960\t599,500000\t492,350000\t500,000000\r\n5522\t319966449\t589,500000\t486,000000\t500,000000\r\n5523\t319967987\t580,500000\t479,000000\t500,000000\r\n5524\t319969589\t574,200000\t471,750000\t500,000000\r\n5525\t319971124\t565,600000\t463,350000\t500,000000\r\n5526\t319972702\t552,000000\t455,000000\t500,000000\r\n5527\t319974263\t543,500000\t445,750000\t500,000000\r\n5528\t319975855\t534,000000\t435,250000\t500,000000\r\n5529\t319977362\t521,100000\t425,250000\t500,000000\r\n5530\t319978896\t508,500000\t416,550000\t500,000000\r\n5531\t319980459\t495,500000\t405,750000\t500,000000\r\n5532\t319982042\t488,000000\t396,500000\t500,000000\r\n5533\t319983526\t476,900000\t387,150000\t500,000000\r\n5534\t319985085\t462,100000\t378,250000\t500,000000\r\n5535\t319986657\t454,500000\t369,500000\t500,000000\r\n5536\t319988219\t446,000000\t360,550000\t500,000000\r\n5537\t319989803\t437,000000\t353,250000\t500,000000\r\n5538\t319991375\t425,900000\t345,750000\t500,000000\r\n5539\t319992944\t419,200000\t338,800000\t500,000000\r\n5540\t319994482\t413,700000\t332,000000\t500,000000\r\n5541\t319995980\t402,500000\t326,000000\t500,000000\r\n5542\t319997553\t397,000000\t320,000000\t500,000000\r\n5543\t319999125\t388,000000\t313,150000\t500,000000\r\n5544\t320000664\t382,000000\t307,000000\t500,000000\r\n5545\t320002147\t376,500000\t301,250000\t500,000000\r\n5546\t320003734\t370,800000\t294,750000\t500,000000\r\n5547\t320005303\t360,600000\t289,750000\t500,000000\r\n5548\t320006866\t354,500000\t283,050000\t500,000000\r\n5549\t320008449\t346,500000\t277,250000\t500,000000\r\n5550\t320010042\t343,000000\t271,500000\t500,000000\r\n5551\t320011614\t334,500000\t266,500000\t500,000000\r\n5552\t320013199\t330,000000\t260,600000\t500,000000\r\n5553\t320014782\t323,900000\t255,250000\t500,000000\r\n5554\t320016366\t314,500000\t250,750000\t500,000000\r\n5555\t320017857\t311,100000\t246,000000\t500,000000\r\n5556\t320019407\t309,600000\t242,000000\t500,000000\r\n5557\t320020897\t301,500000\t237,500000\t500,000000\r\n5558\t320022449\t295,500000\t233,500000\t500,000000\r\n5559\t320024001\t295,500000\t229,500000\t500,000000\r\n5560\t320025595\t289,000000\t225,750000\t500,000000\r\n5561\t320027063\t284,500000\t222,000000\t500,000000\r\n5562\t320028615\t279,000000\t218,500000\t500,000000\r\n5563\t320030164\t275,500000\t214,500000\t500,000000\r\n5564\t320031676\t271,500000\t211,250000\t500,000000\r\n5565\t320033209\t266,300000\t206,800000\t500,000000\r\n5566\t320034733\t264,700000\t203,250000\t500,000000\r\n5567\t320036311\t259,200000\t200,000000\t500,000000\r\n5568\t320037908\t255,500000\t197,000000\t500,000000\r\n5569\t320039376\t252,500000\t194,500000\t500,000000\r\n5570\t320040928\t248,000000\t191,750000\t500,000000\r\n5571\t320042523\t245,000000\t187,500000\t500,000000\r\n5572\t320044147\t240,500000\t184,850000\t500,000000\r\n5573\t320045707\t237,000000\t181,350000\t500,000000\r\n5574\t320047304\t232,500000\t175,500000\t500,000000\r\n5575\t320048909\t232,500000\t174,250000\t500,000000\r\n5576\t320050460\t225,500000\t170,500000\t500,000000\r\n5577\t320052063\t218,500000\t165,500000\t500,000000\r\n5578\t320053668\t214,700000\t160,700000\t500,000000\r\n5579\t320055242\t211,400000\t157,500000\t500,000000\r\n5580\t320056835\t208,100000\t154,750000\t500,000000\r\n5581\t320058367\t204,600000\t152,000000\t500,000000\r\n5582\t320059834\t201,500000\t149,500000\t500,000000\r\n5583\t320061382\t202,100000\t148,250000\t500,000000\r\n5584\t320062959\t405,200000\t43,800000\t0,000000\r\n5585\t320064506\t561,800000\t0,000000\t0,000000\r\n5586\t320066043\t600,000000\t0,000000\t0,000000\r\n5587\t320067596\t627,700000\t0,000000\t0,000000\r\n5588\t320069241\t651,000000\t0,000000\t0,000000\r\n5589\t320070814\t674,300000\t0,000000\t0,000000\r\n5590\t320072440\t691,500000\t0,000000\t0,000000\r\n5591\t320074022\t706,500000\t0,000000\t0,000000\r\n5592\t320075586\t720,000000\t0,000000\t0,000000\r\n5593\t320077221\t733,200000\t0,000000\t0,000000\r\n5594\t320078825\t744,500000\t0,000000\t0,000000\r\n5595\t320080419\t753,000000\t0,000000\t0,000000\r\n5596\t320082033\t764,500000\t0,000000\t0,000000\r\n5597\t320083648\t774,100000\t0,000000\t0,000000\r\n5598\t320085232\t780,700000\t0,000000\t0,000000\r\n5599\t320086784\t790,000000\t0,000000\t0,000000\r\n5600\t320088368\t798,000000\t0,000000\t0,000000\r\n5601\t320089983\t804,500000\t0,000000\t0,000000\r\n5602\t320091543\t814,000000\t0,000000\t0,000000\r\n5603\t320093089\t822,500000\t0,000000\t0,000000\r\n5604\t320094628\t825,600000\t0,000000\t0,000000\r\n5605\t320096166\t834,400000\t0,000000\t0,000000\r\n5606\t320097730\t841,000000\t0,000000\t0,000000\r\n5607\t320099330\t848,000000\t0,000000\t0,000000\r\n5608\t320100956\t862,500000\t0,000000\t0,000000\r\n5609\t320102573\t895,500000\t0,000000\t0,000000\r\n5610\t320104133\t931,400000\t0,000000\t0,000000\r\n5611\t320105715\t974,900000\t0,000000\t0,000000\r\n5612\t320107327\t1029,900000\t0,000000\t0,000000\r\n5613\t320108901\t1081,900000\t0,000000\t0,000000\r\n5614\t320110478\t1108,500000\t0,000000\t0,000000\r\n5615\t320112109\t1128,500000\t0,000000\t0,000000\r\n5616\t320113702\t1143,000000\t0,000000\t0,000000\r\n5617\t320115269\t1150,500000\t0,000000\t0,000000\r\n5618\t320116826\t1160,500000\t0,000000\t0,000000\r\n5619\t320118376\t1164,000000\t0,000000\t0,000000\r\n5620\t320119916\t1166,500000\t0,000000\t0,000000\r\n5621\t320121545\t1168,500000\t0,000000\t0,000000\r\n5622\t320123075\t1171,500000\t0,000000\t0,000000\r\n5623\t320124596\t1173,500000\t0,000000\t0,000000\r\n5624\t320126171\t1176,000000\t0,000000\t0,000000\r\n5625\t320127678\t1176,000000\t0,000000\t0,000000\r\n5626\t320129212\t1182,100000\t0,000000\t0,000000\r\n5627\t320130780\t1181,100000\t0,000000\t0,000000\r\n5628\t320132340\t1183,600000\t0,000000\t0,000000\r\n5629\t320133945\t1184,800000\t0,000000\t0,000000\r\n5630\t320135483\t1188,000000\t0,000000\t0,000000\r\n5631\t320137007\t1188,600000\t0,000000\t0,000000\r\n5632\t320138601\t1187,600000\t0,000000\t0,000000\r\n5633\t320140172\t1189,400000\t0,000000\t0,000000\r\n5634\t320141741\t1188,200000\t0,000000\t0,000000\r\n5635\t320143268\t1190,900000\t0,000000\t0,000000\r\n5636\t320144825\t1191,000000\t0,000000\t0,000000\r\n5637\t320146356\t1192,500000\t0,000000\t0,000000\r\n5638\t320147950\t1192,000000\t0,000000\t0,000000\r\n5639\t320149511\t1192,000000\t0,000000\t0,000000\r\n5640\t320151105\t1194,000000\t0,000000\t0,000000\r\n5641\t320152691\t1196,000000\t0,000000\t0,000000\r\n5642\t320154283\t1196,500000\t0,000000\t0,000000\r\n5643\t320155838\t1197,000000\t0,000000\t0,000000\r\n5644\t320157365\t1197,000000\t0,000000\t0,000000\r\n5645\t320158943\t1200,500000\t0,000000\t0,000000\r\n5646\t320160522\t1199,400000\t0,000000\t0,000000\r\n5647\t320162116\t1201,000000\t0,000000\t0,000000\r\n5648\t320163686\t1200,500000\t0,000000\t0,000000\r\n5649\t320165251\t1203,500000\t0,000000\t0,000000\r\n5650\t320166824\t1202,500000\t0,000000\t0,000000\r\n5651\t320168331\t1204,000000\t0,000000\t0,000000\r\n5652\t320169919\t1206,500000\t0,000000\t0,000000\r\n5653\t320171491\t1207,000000\t0,000000\t0,000000\r\n5654\t320173011\t1206,000000\t0,000000\t0,000000\r\n5655\t320174541\t1208,500000\t0,000000\t0,000000\r\n5656\t320176086\t1208,000000\t0,000000\t0,000000\r\n5657\t320177690\t1209,500000\t0,000000\t0,000000\r\n5658\t320179267\t1210,000000\t0,000000\t0,000000\r\n5659\t320180755\t1208,500000\t0,000000\t0,000000\r\n5660\t320182330\t1209,500000\t0,000000\t0,000000\r\n5661\t320183921\t1209,500000\t0,000000\t0,000000\r\n5662\t320185471\t1209,500000\t0,000000\t0,000000\r\n5663\t320187042\t1211,500000\t0,000000\t0,000000\r\n5664\t320188615\t1209,500000\t0,000000\t0,000000\r\n5665\t320190133\t1211,500000\t0,000000\t0,000000\r\n5666\t320191638\t1212,000000\t0,000000\t0,000000\r\n5667\t320193210\t1211,000000\t0,000000\t0,000000\r\n5668\t320194783\t1215,000000\t0,000000\t0,000000\r\n5669\t320196397\t1215,000000\t0,000000\t0,000000\r\n5670\t320197969\t1216,000000\t0,000000\t0,000000\r\n5671\t320199575\t1214,500000\t0,000000\t0,000000\r\n5672\t320201256\t1214,500000\t0,000000\t0,000000\r\n5673\t320202951\t1215,000000\t0,000000\t0,000000\r\n5674\t320204645\t1218,500000\t0,000000\t0,000000\r\n5675\t320206331\t1216,000000\t0,000000\t0,000000\r\n5676\t320207924\t1217,500000\t0,000000\t0,000000\r\n5677\t320209600\t1219,000000\t0,000000\t0,000000\r\n5678\t320211242\t1214,900000\t0,000000\t0,000000\r\n5679\t320212896\t1220,500000\t0,000000\t0,000000\r\n5680\t320214375\t1220,000000\t0,000000\t0,000000\r\n5681\t320215906\t1218,500000\t0,000000\t0,000000\r\n5682\t320217511\t1220,500000\t0,000000\t0,000000\r\n5683\t320219076\t1221,500000\t0,000000\t0,000000\r\n5684\t320220637\t1220,000000\t0,000000\t0,000000\r\n5685\t320222205\t1220,000000\t0,000000\t0,000000\r\n5686\t320223742\t1220,500000\t0,000000\t0,000000\r\n5687\t320225298\t1224,000000\t0,000000\t0,000000\r\n5688\t320226877\t1223,000000\t0,000000\t0,000000\r\n5689\t320228391\t1224,000000\t0,000000\t0,000000\r\n5690\t320229933\t1223,000000\t0,000000\t0,000000\r\n5691\t320231516\t1224,000000\t0,000000\t0,000000\r\n5692\t320233046\t1225,000000\t0,000000\t0,000000\r\n5693\t320234593\t1224,000000\t0,000000\t0,000000\r\n5694\t320236152\t1225,500000\t0,000000\t0,000000\r\n5695\t320237710\t1221,000000\t0,000000\t0,000000\r\n5696\t320239295\t1224,500000\t0,000000\t0,000000\r\n5697\t320240892\t1225,500000\t0,000000\t0,000000\r\n5698\t320242483\t1225,500000\t0,000000\t0,000000\r\n5699\t320244089\t1225,000000\t0,000000\t0,000000\r\n5700\t320245695\t1223,500000\t0,000000\t0,000000\r\n5701\t320247218\t1226,000000\t0,000000\t0,000000\r\n5702\t320248756\t1229,100000\t0,000000\t0,000000\r\n5703\t320250305\t1228,000000\t0,000000\t0,000000\r\n5704\t320251835\t1227,000000\t0,000000\t0,000000\r\n5705\t320253455\t1227,500000\t0,000000\t0,000000\r\n5706\t320255038\t1229,500000\t0,000000\t0,000000\r\n5707\t320256628\t1229,500000\t0,000000\t0,000000\r\n5708\t320258182\t1229,500000\t0,000000\t0,000000\r\n5709\t320259786\t1228,500000\t0,000000\t0,000000\r\n5710\t320261375\t1228,500000\t0,000000\t0,000000\r\n5711\t320262939\t1229,500000\t0,000000\t0,000000\r\n5712\t320264525\t1229,500000\t0,000000\t0,000000\r\n5713\t320266045\t1231,600000\t0,000000\t0,000000\r\n5714\t320267601\t1230,000000\t0,000000\t0,000000\r\n5715\t320269110\t1229,500000\t0,000000\t0,000000\r\n5716\t320270736\t1230,500000\t0,000000\t0,000000\r\n5717\t320272296\t1231,500000\t0,000000\t0,000000\r\n5718\t320273857\t1232,000000\t0,000000\t0,000000\r\n5719\t320275437\t1231,000000\t0,000000\t0,000000\r\n5720\t320276989\t1231,000000\t0,000000\t0,000000\r\n5721\t320278561\t1231,500000\t0,000000\t0,000000\r\n5722\t320280057\t1233,500000\t0,000000\t0,000000\r\n5723\t320281567\t1232,000000\t0,000000\t0,000000\r\n5724\t320283092\t1233,500000\t0,000000\t0,000000\r\n5725\t320284575\t1233,000000\t0,000000\t0,000000\r\n5726\t320286095\t1231,500000\t0,000000\t0,000000\r\n5727\t320287635\t1233,600000\t0,000000\t0,000000\r\n5728\t320289210\t1233,500000\t0,000000\t0,000000\r\n5729\t320290752\t1234,000000\t0,000000\t0,000000\r\n5730\t320292294\t1233,000000\t0,000000\t0,000000\r\n5731\t320293929\t1234,600000\t0,000000\t0,000000\r\n5732\t320295521\t1234,000000\t0,000000\t0,000000\r\n5733\t320297092\t1235,200000\t0,000000\t0,000000\r\n5734\t320298648\t1235,200000\t0,000000\t0,000000\r\n5735\t320300221\t1233,600000\t0,000000\t0,000000\r\n5736\t320301841\t1235,200000\t0,000000\t0,000000\r\n5737\t320303393\t1234,600000\t0,000000\t0,000000\r\n5738\t320305002\t1236,200000\t0,000000\t0,000000\r\n5739\t320306599\t1237,500000\t0,000000\t0,000000\r\n5740\t320308233\t1236,900000\t0,000000\t0,000000\r\n5741\t320309857\t1235,700000\t0,000000\t0,000000\r\n5742\t320311463\t1235,800000\t0,000000\t0,000000\r\n5743\t320313066\t1237,500000\t0,000000\t0,000000\r\n5744\t320314618\t1236,500000\t0,000000\t0,000000\r\n5745\t320316180\t1235,100000\t0,000000\t0,000000\r\n5746\t320317727\t1237,300000\t0,000000\t0,000000\r\n5747\t320319423\t1239,100000\t0,000000\t0,000000\r\n5748\t320321109\t1239,400000\t0,000000\t0,000000\r\n5749\t320322822\t1238,600000\t0,000000\t0,000000\r\n5750\t320324529\t1238,700000\t0,000000\t0,000000\r\n5751\t320326236\t1238,600000\t0,000000\t0,000000\r\n5752\t320327940\t1239,700000\t0,000000\t0,000000\r\n5753\t320329647\t1239,800000\t0,000000\t0,000000\r\n5754\t320331356\t1238,800000\t0,000000\t0,000000\r\n5755\t320333066\t1239,800000\t0,000000\t0,000000\r\n5756\t320334766\t1238,600000\t0,000000\t0,000000\r\n5757\t320336472\t1240,200000\t0,000000\t0,000000\r\n5758\t320338180\t1239,200000\t0,000000\t0,000000\r\n5759\t320339893\t1240,300000\t0,000000\t0,000000\r\n5760\t320341602\t1240,900000\t0,000000\t0,000000\r\n5761\t320343305\t1239,200000\t0,000000\t0,000000\r\n5762\t320345008\t1242,000000\t0,000000\t0,000000\r\n5763\t320346709\t1240,200000\t0,000000\t0,000000\r\n5764\t320348406\t1243,000000\t0,000000\t0,000000\r\n5765\t320349981\t1242,400000\t0,000000\t0,000000\r\n5766\t320351523\t1240,400000\t0,000000\t0,000000\r\n5767\t320353072\t1242,500000\t0,000000\t0,000000\r\n5768\t320354691\t1243,500000\t0,000000\t0,000000\r\n5769\t320356299\t1244,500000\t0,000000\t0,000000\r\n5770\t320357959\t1242,900000\t0,000000\t0,000000\r\n5771\t320359554\t1243,500000\t0,000000\t0,000000\r\n5772\t320361083\t1242,000000\t0,000000\t0,000000\r\n5773\t320362596\t1243,000000\t0,000000\t0,000000\r\n5774\t320364169\t1244,500000\t0,000000\t0,000000\r\n5775\t320365772\t1242,400000\t0,000000\t0,000000\r\n5776\t320367294\t1241,900000\t0,000000\t0,000000\r\n5777\t320368752\t1244,500000\t0,000000\t0,000000\r\n5778\t320370325\t1244,000000\t0,000000\t0,000000\r\n5780\t320373148\t1244,500000\t0,000000\t0,000000\r\n5781\t320374456\t1244,400000\t0,000000\t0,000000\r\n5782\t320375587\t1244,000000\t0,000000\t0,000000\r\n"
  out "Waveform Graph Current":dbl[](graph)
  out "Voltage (mV) F":dbl
  out "Current (mA) F":dbl
  in  "CurrentArrayF":dbl[](array[numeric])
  in  "CurrentArray":dbl[](array[numeric])
  in  "VoltageArrayF":dbl[](array[numeric])
  out "Waveform Graph Voltage":dbl[](graph)
  in  "VoltageArray":dbl[](array[numeric])
  out "esdaqErrorOut":errorcluster
  in  "esdaqPortInp":refnum<visa-resource-name>
  in  "SetCurrent":bool
  out "Voltage (mV)":dbl
  out "Current (mA)":dbl
  in  "Set Value (mA)":dbl
  # "PLB Basic Control Interface"
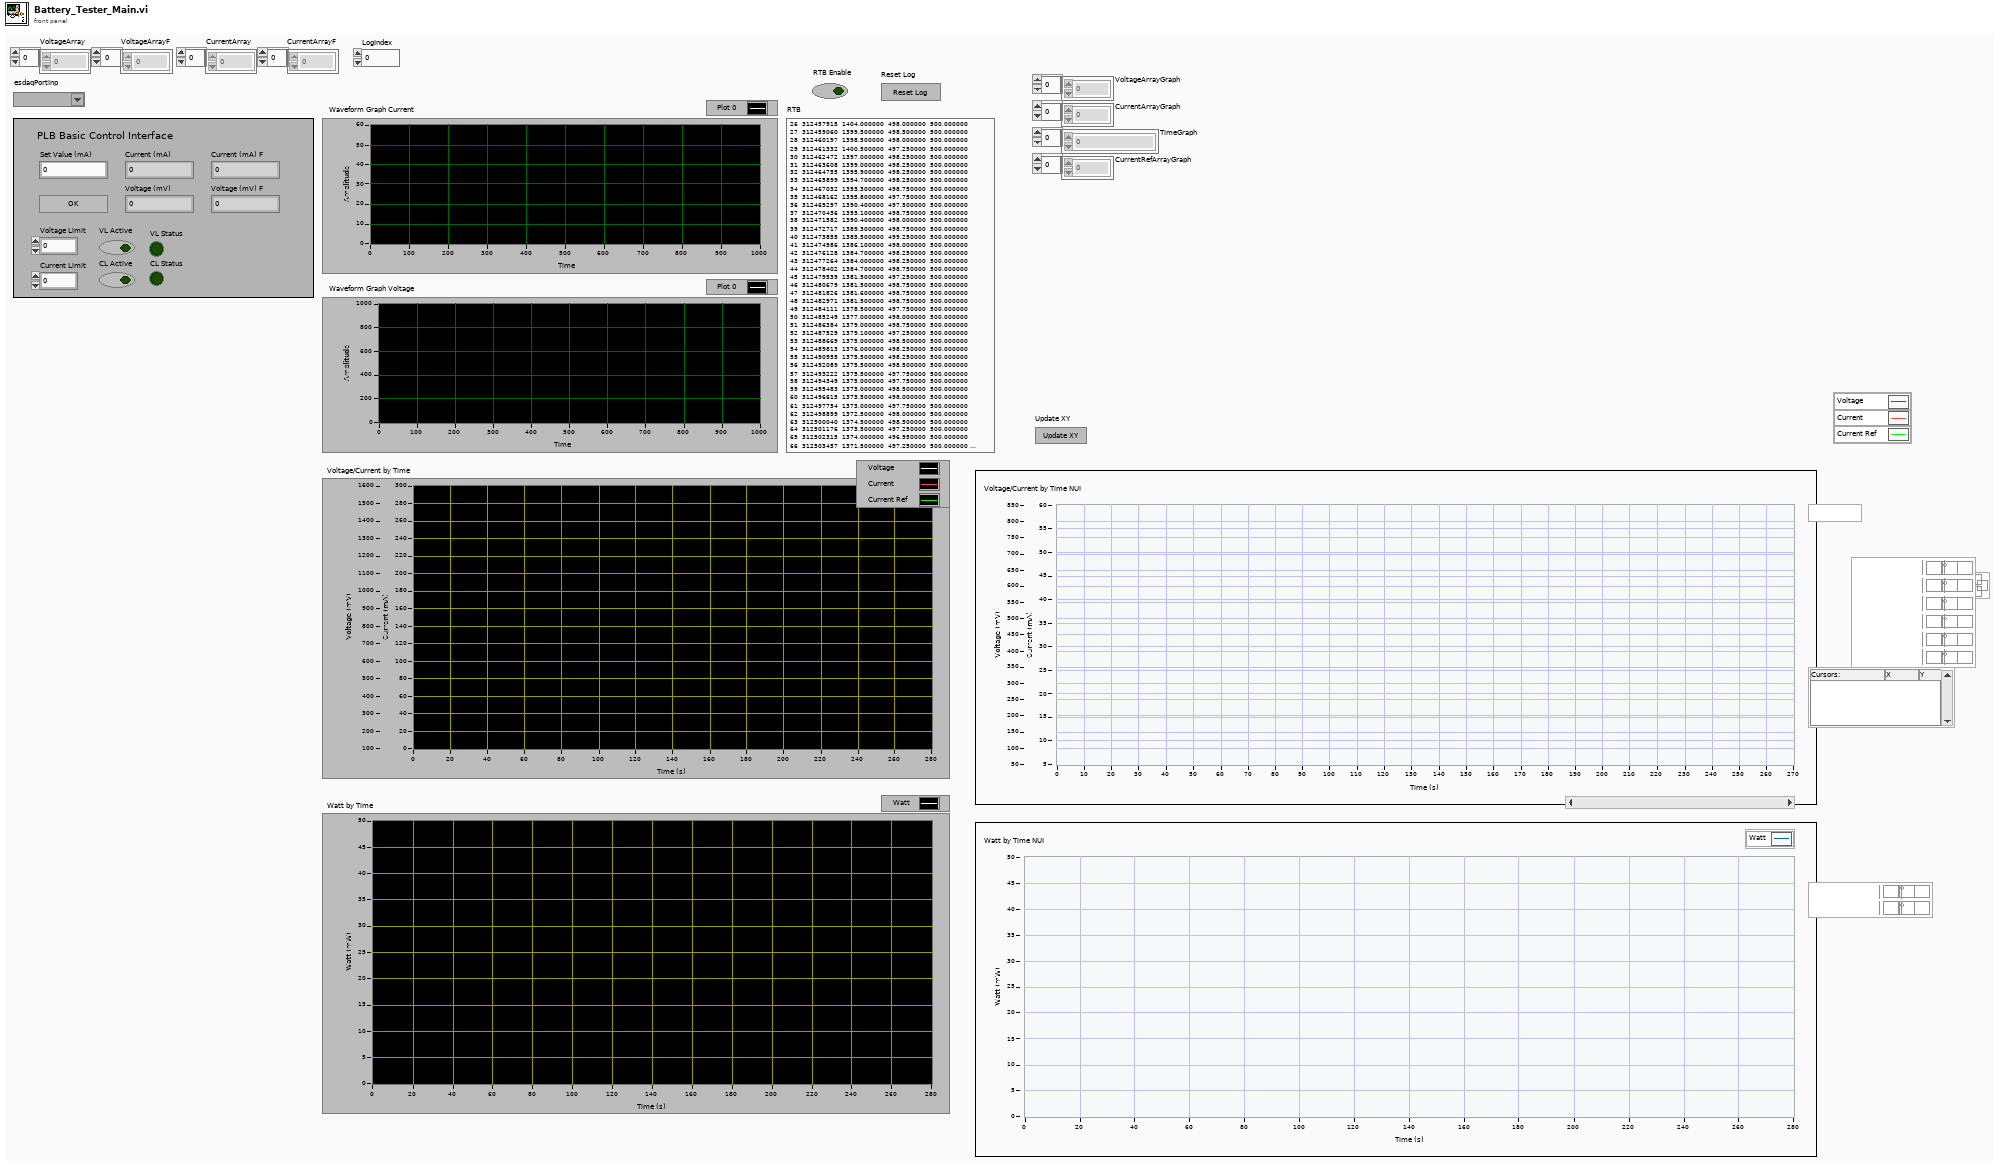
[diagram p1: front panel]
types:
  T1 = cluster{"TimeGraph":dbl[], "CurrentArrayGraph":dbl[]}[]
  T2 = cluster{"TimeGraph":dbl[], "VoltageArrayGraph":dbl[]}
  T3 = cluster{"TimeGraph":dbl[], "CurrentArrayGraph":dbl[]}
  T4 = cluster{"TimeGraph":dbl[], "CurrentRefArrayGraph":dbl[]}
  T5 = cluster{"TimeGraph":dbl[], "CurrentRefArrayGraph":dbl[]}[]
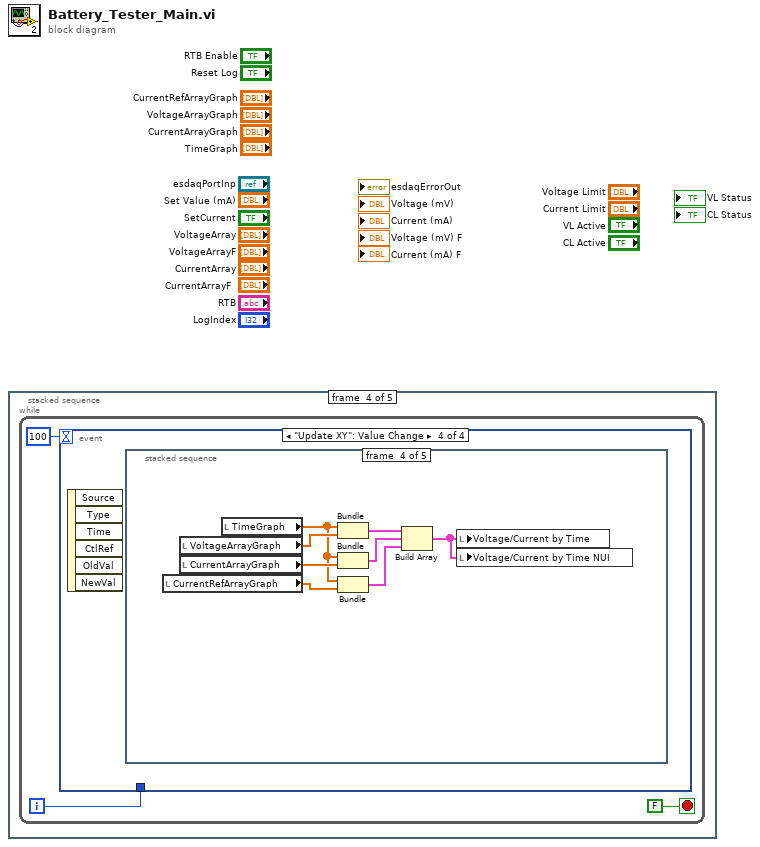
[diagram p0: block diagram]
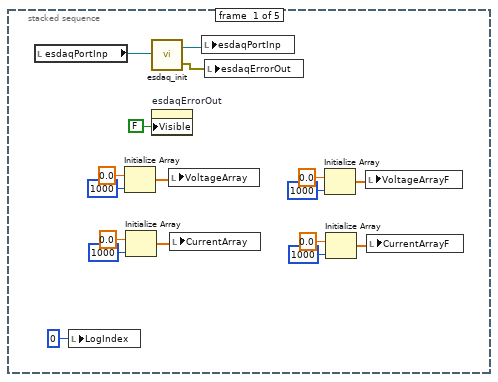
[diagram p2: hidden frame]
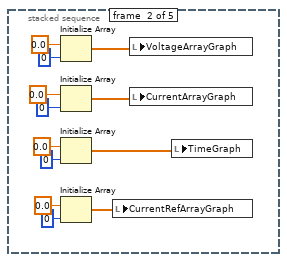
[diagram p3: hidden frame]
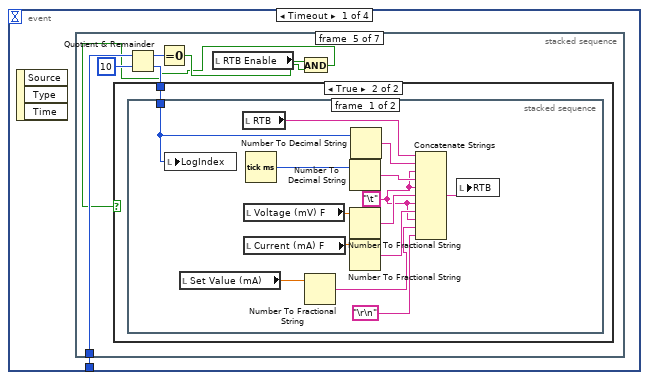
[diagram p5: hidden frame]
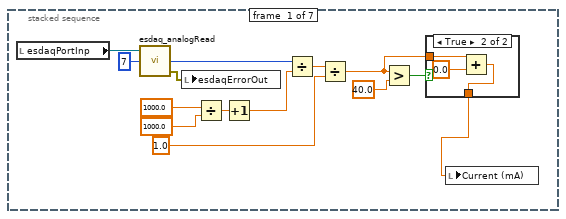
[diagram p6: hidden frame]
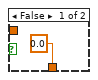
[diagram p7: hidden frame]
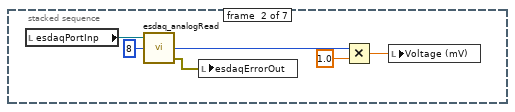
[diagram p8: hidden frame]
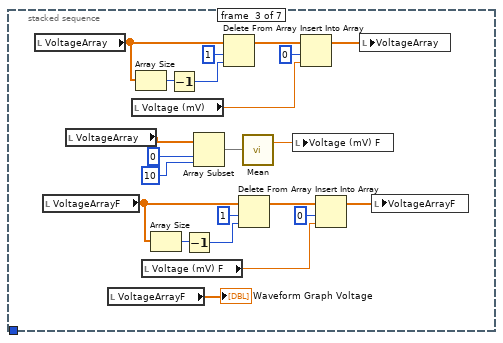
[diagram p9: hidden frame]
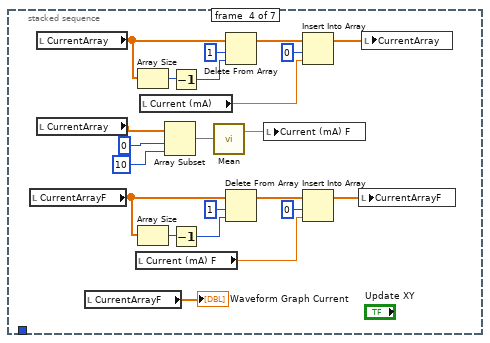
[diagram p10: hidden frame]
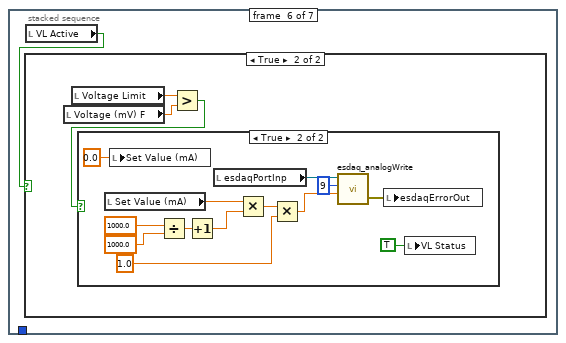
[diagram p13: hidden frame]
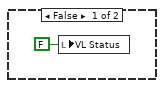
[diagram p14: hidden frame]
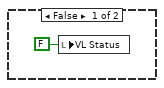
[diagram p15: hidden frame]
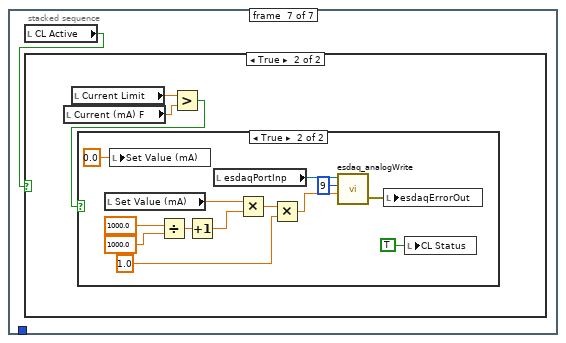
[diagram p16: hidden frame]
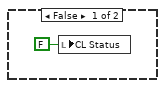
[diagram p17: hidden frame]
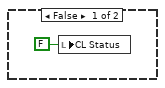
[diagram p18: hidden frame]
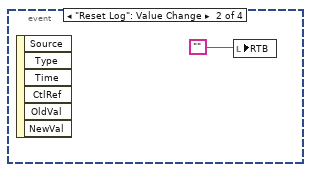
[diagram p19: hidden frame]
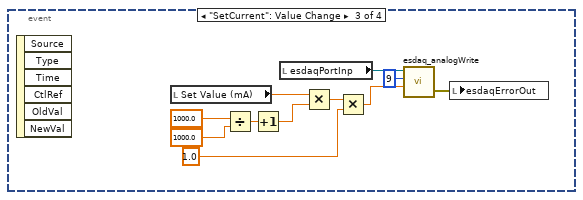
[diagram p20: hidden frame]
diagram:
  n1 = stacked-sequence {
    frame #0 {
      n2 = local read "esdaqPortInp"() -> (w16:refnum<visa-resource-name>)
      n3 = local write "LogIndex"(u32 0 ("LogIndex")) -> ()
      n4 = Initialize Array(0.0 ("element"), 1000 ("dimension size")) -> (w14:dbl[])
      n5 = Initialize Array(0.0 ("element"), 1000 ("dimension size")) -> (w13:dbl[])
      n6 = call "esdaq_init.vi"("esdaqPortInp"=w16) -> ("esdaqPortOut"=w17:refnum<visa-resource-name>, "esdaqErrorOut"=w15:errorcluster)
      n7 = property on="esdaqErrorOut" class="Clust (strict)"("Visible"=FALSE) -> ()  [unwired: 2 in, 2 out]
      n8 = local write "VoltageArray"(w14) -> ()
      n9 = local write "CurrentArray"(w13) -> ()
      n10 = local write "esdaqPortInp"(w17) -> ()
      n11 = local write "esdaqErrorOut"(w15) -> ()
      n12 = Initialize Array(0.0 ("element"), 1000 ("dimension size")) -> (w11:dbl[])
      n13 = Initialize Array(0.0 ("element"), 1000 ("dimension size")) -> (w12:dbl[])
      n14 = local write "VoltageArrayF"(w11) -> ()
      n15 = local write "CurrentArrayF"(w12) -> ()
    }
    frame #1 {
      n16 = Initialize Array(0.0 ("element"), 0 ("dimension size")) -> (w29:dbl[])
      n17 = Initialize Array(0.0 ("element"), 0 ("dimension size")) -> (w24:dbl[])
      n18 = Initialize Array(0.0 ("element"), 0 ("dimension size")) -> (w23:dbl[])
      n19 = Initialize Array(0.0 ("element"), 0 ("dimension size")) -> (w18:dbl[])
      n20 = local write "CurrentRefArrayGraph"(w18) -> ()
      n21 = local write "VoltageArrayGraph"(w29) -> ()
      n22 = local write "CurrentArrayGraph"(w24) -> ()
      n23 = local write "TimeGraph"(w23) -> ()
    }
    frame #2 {
    }
    frame #3 {
      n24 = while {
        i -> [w30]
        stop <- FALSE stop-if-true
        n25 = event shown="[3] \"Update XY\": Value Change" {
          selector: _ -> [_ _ _ _]
          dyn-events: _ -> [_ _ _ _]
          timeout: 100 -> [_ _ _ _]
          tunnel: w30 -> [w33 _ _ _]
          event Timeout {
            n26 = event-data() -> ()  [unwired: 1 in, 3 out]
            n27 = stacked-sequence {
              tunnel: w33 -> [_ _ _ _ w108 _ _]
              frame #0 {
                n28 = local read "esdaqPortInp"() -> (w45:refnum<visa-resource-name>)
                n29 = call "esdaq_analogRead.vi"("Channel"=u8 7, "esdaqPortInp"=w45) -> ("esdaqErrorOut"=w46:errorcluster, "value"=w41:i32)  [unwired: 1 in, 1 out]
                n30 = local write "esdaqErrorOut"(w46) -> ()
                n31 = Divide(x=1000.0, y=1000.0) -> (x/y=w44:dbl)
                n32 = Increment(x=w44) -> (x+1=w40:dbl)
                n33 = Divide(x=w41, y=w40) -> (x/y=w39:dbl)
                n34 = Divide(x=w39, y=1.0) -> (x/y=w34:dbl)
                n35 = Greater?(x=w34, y=40.0) -> (0:w36:bool)
                n36 = case shown="True" w36 {
                  tunnel: w34 -> [_ w51]
                  tunnel: [0.0 ("Current (mA)") w50] -> w35
                  frame False {
                  }
                  frame True {
                    n37 = Add(x=w51, y=0.0) -> (x+y=w50:dbl)
                  }
                }
                n38 = local write "Current (mA)"(w35) -> ()
              }
              frame #1 {
                n39 = local read "esdaqPortInp"() -> (w55:refnum<visa-resource-name>)
                n40 = call "esdaq_analogRead.vi"("Channel"=u8 8, "esdaqPortInp"=w55) -> ("esdaqErrorOut"=w57:errorcluster, "value"=w54:i32)  [unwired: 1 in, 1 out]
                n41 = local write "esdaqErrorOut"(w57) -> ()
                n42 = Multiply(x=w54, y=1.0) -> (x*y=w52:dbl)
                n43 = local write "Voltage (mV)"(w52) -> ()
              }
              frame #2 {
                n44 = local read "VoltageArray"() -> (w79:dbl[])
                n45 = local read "VoltageArrayF"() -> (w60:dbl[])
                n46 = local read "VoltageArray"() -> (w71:dbl[])
                n47 = local read "VoltageArrayF"() -> (→"Waveform Graph Voltage":dbl[])
                n48 = local read "Voltage (mV)"() -> (w73:dbl)
                n49 = Array Size(array=w79) -> (size(s)=w78:i32)
                n50 = local read "Voltage (mV) F"() -> (w66:dbl)
                n51 = Array Size(array=w60) -> (size(s)=w61:i32)
                n52 = Decrement(x=w78) -> (x-1=w77:i32)
                n53 = Decrement(x=w61) -> (x-1=w62:i32)
                n54 = Array Subset(array=w71, index=0, length=10 ("index")) -> (w70:dbl[])
                n55 = Delete From Array(array=w79, length=1, index=w77) -> (array with subset deleted=w75:dbl[])  [unwired: 1 out]
                n56 = Delete From Array(array=w60, length=1, index=w62) -> (array with subset deleted=w64:dbl[])  [unwired: 1 out]
                n57 = call-poly <vilib>:"Mean.vi"("X"=w70) -> ("mean"=w69:dbl)  [unwired: 1 out]
                n58 = local write "Voltage (mV) F"(w69) -> ()
                n59 = Insert Into Array(array=w75, index=0, new element=w73) -> (w72:dbl[])
                n60 = Insert Into Array(array=w64, index=0, new element=w66) -> (w59:dbl[])
                n61 = local write "VoltageArray"(w72) -> ()
                n62 = local write "VoltageArrayF"(w59) -> ()
              }
              frame #3 {
                n63 = local read "CurrentArrayF"() -> (w81:dbl[])
                n64 = local read "CurrentArray"() -> (w101:dbl[])
                n65 = local read "CurrentArray"() -> (w93:dbl[])
                n66 = local read "CurrentArrayF"() -> (→"Waveform Graph Current":dbl[])
                n67 = local read "Current (mA) F"() -> (w85:dbl)
                n68 = Array Size(array=w101) -> (size(s)=w100:i32)
                n69 = Array Size(array=w81) -> (size(s)=w82:i32)
                n70 = local read "Current (mA)"() -> (w97:dbl)
                n71 = Array Subset(array=w93, index=0, length=10 ("index")) -> (w90:dbl[])
                n72 = Decrement(x=w100) -> (x-1=w99:i32)
                n73 = Decrement(x=w82) -> (x-1=w83:i32)
                n74 = call-poly <vilib>:"Mean.vi"("X"=w90) -> ("mean"=w89:dbl)  [unwired: 1 out]
                n75 = Delete From Array(array=w101, length=1, index=w99) -> (array with subset deleted=w98:dbl[])  [unwired: 1 out]
                n76 = Delete From Array(array=w81, length=1, index=w83) -> (array with subset deleted=w84:dbl[])  [unwired: 1 out]
                n77 = local write "Current (mA) F"(w89) -> ()
                n78 = Insert Into Array(array=w98, index=0, new element=w97) -> (w94:dbl[])
                n79 = Insert Into Array(array=w84, index=0, new element=w85) -> (w88:dbl[])
                n80 = local write "CurrentArrayF"(w88) -> ()
                n81 = local write "CurrentArray"(w94) -> ()
              }
              frame #4 {
                n82 = Quotient & Remainder(x=w108, y=10) -> (x-y*floor(x/y)=w106:i32, floor(x/y)=w105:i32)
                n83 = Equal To 0?(x=w106) -> (x = 0?=w103:bool)
                n84 = local read "RTB Enable"() -> (w104:bool)
                n85 = And(x=w104, y=w103) -> (x .and. y?=w102:bool)
                n86 = case shown="True" w102 {
                  tunnel: w105 -> [_ w109]
                  frame False {
                  }
                  frame True {
                    n87 = stacked-sequence {
                      tunnel: w109 -> [w115 _]
                      frame #0 {
                        w112 = "\t"
                        n88 = local write "LogIndex"(w115) -> ()
                        n89 = local read "Set Value (mA)"() -> (w111:dbl)
                        n90 = local read "RTB"() -> (w117:string)
                        n91 = local read "Voltage (mV) F"() -> (w123:dbl)
                        n92 = local read "Current (mA) F"() -> (w122:dbl)
                        n93 = Tick Count (ms)() -> (millisecond timer value=w114:u32)
                        n94 = Number To Fractional String(number=w111) -> (F-format string=w110:string)  [unwired: 3 in]
                        n95 = Number To Decimal String(number=w114) -> (decimal integer string=w121:string)  [unwired: 1 in]
                        n96 = Number To Fractional String(number=w123) -> (F-format string=w120:string)  [unwired: 3 in]
                        n97 = Number To Fractional String(number=w122) -> (F-format string=w119:string)  [unwired: 3 in]
                        n98 = Number To Decimal String(number=w115) -> (decimal integer string=w118:string)  [unwired: 1 in]
                        n99 = Concatenate Strings(w117, w118, w112, w121, w112, w120, w112, w119, w112, w110, "\r\n") -> (w116:string)
                        n100 = local write "RTB"(w116) -> ()
                      }
                      frame #1 {
                      }
                    }
                  }
                }
              }
              frame #5 {
                n101 = local read "VL Active"() -> (w124:bool)
                n102 = case shown="True" w124 {
                  frame False {
                    n103 = local write "VL Status"(FALSE ("VL Status")) -> ()
                  }
                  frame True {
                    n104 = local read "Voltage (mV) F"() -> (w127:dbl)
                    n105 = local read "Voltage Limit"() -> (w128:dbl)
                    n106 = Greater?(x=w128, y=w127) -> (0:w126:bool)
                    n107 = case shown="True" w126 {
                      frame False {
                        n108 = local write "VL Status"(FALSE ("VL Status")) -> ()
                      }
                      frame True {
                        n109 = local read "Set Value (mA)"() -> (w138:dbl)
                        n110 = local write "Set Value (mA)"(0.0 ("Set Value (mA)")) -> ()
                        n111 = Divide(x=1000.0, y=1000.0) -> (x/y=w139:dbl)
                        n112 = Increment(x=w139) -> (x+1=w137:dbl)
                        n113 = local read "esdaqPortInp"() -> (w140:refnum<visa-resource-name>)
                        n114 = Multiply(x=w138, y=w137) -> (x*y=w136:dbl)
                        n115 = Multiply(x=w136, y=1.0) -> (x*y=w135:dbl)
                        n116 = call "esdaq_analogWrite.vi"("Value"=w135, "Channel"=u8 9, "esdaqPortInp"=w140) -> ("esdaqErrorOut"=w141:errorcluster)  [unwired: 1 in, 1 out]
                        n117 = local write "esdaqErrorOut"(w141) -> ()
                        n118 = local write "VL Status"(TRUE ("VL Status")) -> ()
                      }
                    }
                  }
                }
              }
              frame #6 {
                n119 = local read "CL Active"() -> (w143:bool)
                n120 = case shown="True" w143 {
                  frame False {
                    n121 = local write "CL Status"(FALSE ("VL Status")) -> ()
                  }
                  frame True {
                    n122 = local read "Current (mA) F"() -> (w146:dbl)
                    n123 = local read "Current Limit"() -> (w147:dbl)
                    n124 = Greater?(x=w147, y=w146) -> (0:w145:bool)
                    n125 = case shown="True" w145 {
                      frame False {
                        n126 = local write "CL Status"(FALSE ("VL Status")) -> ()
                      }
                      frame True {
                        n127 = local read "Set Value (mA)"() -> (w157:dbl)
                        n128 = local write "Set Value (mA)"(0.0 ("Set Value (mA)")) -> ()
                        n129 = Divide(x=1000.0, y=1000.0) -> (x/y=w158:dbl)
                        n130 = Increment(x=w158) -> (x+1=w156:dbl)
                        n131 = local read "esdaqPortInp"() -> (w159:refnum<visa-resource-name>)
                        n132 = Multiply(x=w157, y=w156) -> (x*y=w155:dbl)
                        n133 = Multiply(x=w155, y=1.0) -> (x*y=w154:dbl)
                        n134 = call "esdaq_analogWrite.vi"("Value"=w154, "Channel"=u8 9, "esdaqPortInp"=w159) -> ("esdaqErrorOut"=w160:errorcluster)  [unwired: 1 in, 1 out]
                        n135 = local write "esdaqErrorOut"(w160) -> ()
                        n136 = local write "CL Status"(TRUE ("VL Status")) -> ()
                      }
                    }
                  }
                }
              }
            }
          }
          event "Reset Log": Value Change {
            n137 = event-data() -> ()  [unwired: 1 in, 6 out]
            n138 = local write "RTB"("") -> ()
          }
          event "SetCurrent": Value Change {
            n139 = event-data() -> ()  [unwired: 1 in, 6 out]
            n140 = local read "Set Value (mA)"() -> (w167:dbl)
            n141 = Divide(x=1000.0, y=1000.0) -> (x/y=w170:dbl)
            n142 = Increment(x=w170) -> (x+1=w166:dbl)
            n143 = local read "esdaqPortInp"() -> (w171:refnum<visa-resource-name>)
            n144 = Multiply(x=w167, y=w166) -> (x*y=w165:dbl)
            n145 = Multiply(x=w165, y=1.0) -> (x*y=w163:dbl)
            n146 = call "esdaq_analogWrite.vi"("Value"=w163, "Channel"=u8 9, "esdaqPortInp"=w171) -> ("esdaqErrorOut"=w172:errorcluster)  [unwired: 1 in, 1 out]
            n147 = local write "esdaqErrorOut"(w172) -> ()
          }
          event "Update XY": Value Change {
            n148 = event-data() -> ()  [unwired: 1 in, 6 out]
            n149 = stacked-sequence {
              frame #0 {
                n150 = local read "RTB"() -> (w178:string)
                n151 = call "RTB2Data.vi"("inp"=w178) -> ("out1"=w177:dbl[], "out2"=w176:dbl[], "out3"=w175:dbl[], "out4"=w174:dbl[])
                n152 = local write "CurrentRefArrayGraph"(w174) -> ()
                n153 = local write "VoltageArrayGraph"(w176) -> ()
                n154 = local write "CurrentArrayGraph"(w175) -> ()
                n155 = local write "TimeGraph"(w177) -> ()
              }
              frame #1 {
                n156 = local read "TimeGraph"() -> (w180:dbl[])
                n157 = Index Array(array=w180, index=0) -> (element=w181:dbl)
                n158 = for {
                  tunnel: w181 -> [w186]
                  tunnel: w180 -> [w187] mode=indexing
                  tunnel: [w183] -> w179 mode=indexing
                  n159 = Subtract(x=w187, y=w186) -> (x-y=w185:dbl)
                  n160 = Divide(x=w185, y=1000.0) -> (x/y=w183:dbl)
                }
                n161 = local write "TimeGraph"(w179) -> ()
              }
              frame #2 {
                w190 = 1 ("length")
                n162 = local read "VoltageArrayGraph"() -> (w193:dbl[])
                n163 = local read "CurrentArrayGraph"() -> (w192:dbl[])
                n164 = local read "TimeGraph"() -> (w196:dbl[])
                n165 = Array Size(array=w192) -> (size(s)=w195:i32)
                n166 = Decrement(x=w195) -> (x-1=w191:i32)
                n167 = Delete From Array(array=w196, length=w190, index=w191) -> (array with subset deleted=w194:dbl[])  [unwired: 1 out]
                n168 = Delete From Array(array=w193, length=w190, index=w191) -> (array with subset deleted=w189:dbl[])  [unwired: 1 out]
                n169 = Delete From Array(array=w192, length=w190, index=w191) -> (array with subset deleted=w188:dbl[])  [unwired: 1 out]
                n170 = local write "VoltageArrayGraph"(w189) -> ()
                n171 = local write "CurrentArrayGraph"(w188) -> ()
                n172 = local write "TimeGraph"(w194) -> ()
              }
              frame #3 {
                n173 = local read "CurrentRefArrayGraph"() -> (w197:dbl[])
                n174 = local read "VoltageArrayGraph"() -> (w204:dbl[])
                n175 = local read "CurrentArrayGraph"() -> (w203:dbl[])
                n176 = local read "TimeGraph"() -> (w198:dbl[])
                n177 = Bundle("TimeGraph"=w198, "VoltageArrayGraph"=w204) -> (w202:T2)  [unwired: 1 in]
                n178 = Bundle("TimeGraph"=w198, "CurrentArrayGraph"=w203) -> (w200:T3)  [unwired: 1 in]
                n179 = Bundle("TimeGraph"=w198, "CurrentRefArrayGraph"=w197) -> (w199:T4)  [unwired: 1 in]
                n180 = Build Array(w202, w200, w199) -> (w201:T5)
                n181 = local write "Voltage/Current by Time"(w201) -> ()
                n182 = local write "Voltage/Current by Time NUI"(w201) -> ()
              }
              frame #4 {
                n183 = local read "VoltageArrayGraph"() -> (w209:dbl[])
                n184 = local read "CurrentArrayGraph"() -> (w210:dbl[])
                n185 = local read "TimeGraph"() -> (w211:dbl[])
                n186 = Multiply(x=w209, y=w210) -> (x*y=w208:dbl[])
                n187 = Divide(x=w208, y=1000.0) -> (x/y=w207:dbl[])
                n188 = Bundle("TimeGraph"=w211, w207) -> (w205:cluster{"TimeGraph":dbl[], dbl[]})  [unwired: 1 in]
                n189 = local write "Watt by Time"(w205) -> ()
                n190 = local write "Watt by Time NUI"(w205) -> ()
              }
            }
          }
        }
      }
    }
    frame #4 {
      n191 = stacked-sequence {
        frame #0 {
          n192 = local read "RTB"() -> (w215:string)
          n193 = call "RTB2Data.vi"("inp"=w215) -> ("out1"=w214:dbl[], "out2"=w213:dbl[], "out3"=w212:dbl[])  [unwired: 1 out]
          n194 = local write "VoltageArrayGraph"(w213) -> ()
          n195 = local write "CurrentArrayGraph"(w212) -> ()
          n196 = local write "TimeGraph"(w214) -> ()
        }
        frame #1 {
          n197 = local read "TimeGraph"() -> (w217:dbl[])
          n198 = Index Array(array=w217, index=0) -> (element=w218:dbl)
          n199 = for {
            tunnel: w218 -> [w223]
            tunnel: w217 -> [w224] mode=indexing
            tunnel: [w220] -> w216 mode=indexing
            n200 = Subtract(x=w224, y=w223) -> (x-y=w222:dbl)
            n201 = Divide(x=w222, y=1000.0) -> (x/y=w220:dbl)
          }
          n202 = local write "TimeGraph"(w216) -> ()
        }
        frame #2 {
          w227 = 1 ("length")
          n203 = local read "VoltageArrayGraph"() -> (w230:dbl[])
          n204 = local read "CurrentArrayGraph"() -> (w229:dbl[])
          n205 = local read "TimeGraph"() -> (w233:dbl[])
          n206 = Array Size(array=w229) -> (size(s)=w232:i32)
          n207 = Decrement(x=w232) -> (x-1=w228:i32)
          n208 = Delete From Array(array=w233, length=w227, index=w228) -> (array with subset deleted=w231:dbl[])  [unwired: 1 out]
          n209 = Delete From Array(array=w230, length=w227, index=w228) -> (array with subset deleted=w226:dbl[])  [unwired: 1 out]
          n210 = Delete From Array(array=w229, length=w227, index=w228) -> (array with subset deleted=w225:dbl[])  [unwired: 1 out]
          n211 = local write "VoltageArrayGraph"(w226) -> ()
          n212 = local write "CurrentArrayGraph"(w225) -> ()
          n213 = local write "TimeGraph"(w231) -> ()
        }
        frame #3 {
          n214 = local read "VoltageArrayGraph"() -> (w238:dbl[])
          n215 = local read "CurrentArrayGraph"() -> (w237:dbl[])
          n216 = local read "TimeGraph"() -> (w239:dbl[])
          n217 = Bundle("TimeGraph"=w239, "VoltageArrayGraph"=w238) -> (w236:T2)  [unwired: 1 in]
          n218 = Bundle("TimeGraph"=w239, "CurrentArrayGraph"=w237) -> (w235:T3)  [unwired: 1 in]
          n219 = Build Array(w236, w235) -> (→"Voltage/Current by Time" →"Voltage/Current by Time NUI":T1)
        }
        frame #4 {
          n220 = local read "VoltageArrayGraph"() -> (w244:dbl[])
          n221 = local read "CurrentArrayGraph"() -> (w245:dbl[])
          n222 = local read "TimeGraph"() -> (w246:dbl[])
          n223 = Multiply(x=w244, y=w245) -> (x*y=w243:dbl[])
          n224 = Divide(x=w243, y=1000.0) -> (x/y=w242:dbl[])
          n225 = Bundle("TimeGraph"=w246, w242) -> (→"Watt by Time" →"Watt by Time NUI":cluster{"TimeGraph":dbl[], dbl[]})  [unwired: 1 in]
        }
      }
    }
  }
